vi "Main.vi"() -> ()   [LabVIEW 2023]
uses:
  SubVIs/Control 1.ctl
  SubVIs/CorrelationSwitchControlType.ctl
  C:/Users/nanometa/Documents/TCSPC_Git_Repo/Source/Thorlabs.MotionControl.Controls.dll
  Thorlabs.MotionControl.Controls.dll
  Drivers/BH TCSPC/Examples/Example_Controls/UserInput.ctl
  Drivers/BH TCSPC/SPC_Wrappers/SPC_Controls/ADCResolution.ctl
  <vilib>/Utility/error.llb/DialogType.ctl
  SubVIs/MeasurementType.ctl
  <vilib>/DAQmx/read.llb/DAQmx Read (Counter DBL 1Chan 1Samp).vi
  <vilib>/DAQmx/write.llb/DAQmx Write (Digital 1D Bool 1Chan 1Samp).vi
  <vilib>/DAQmx/create/channels.llb/DAQmx Create Channel (CI-Count Edges).vi
  <vilib>/DAQmx/miscellaneous.llb/DAQmx Fill In Error Info.vi
  <vilib>/DAQmx/create/channels.llb/DAQmx Create Channel (DO-Digital Output).vi
  <vilib>/Utility/file.llb/Write Delimited Spreadsheet (I64).vi
  C:/Users/nanometa/Documents/TCSPC_Git_Repo/Source/ThorLabs.MotionControl.KCube.DCServoCLI.dll
  ThorLabs.MotionControl.KCube.DCServoCLI.dll
  C:/Users/nanometa/Documents/TCSPC_Git_Repo/Source/Thorlabs.MotionControl.FilterFlipperCLI.dll
  Thorlabs.MotionControl.FilterFlipperCLI.dll
  <instrlib>/Thorlabs_FWxC/Thorlabs_FWxC.lvlib
  <vilib>/Analysis/NI_AALBase.lvlib
panel:
  out "lifetime output":u16[][](array[numeric])=[[0], [0], [0], [0], [0], [0], [0], [0], [0], [0], [0], [0], [0], [0], [0], [0], [0], [0], [0], [0], [0], [0], [0], [0], [0], [0], [0], [0], [0], [0], [0], [0], [0], [0], [0], [0], [0], [0], [0], [0], [0], [0], [0], [0], [0], [0], [0], [0], [0], [0], [0], [0], [0], [0], [0], [0], [0], [0], [0], [0], [0], [0], [0], [0], [0], [0], [0], [0], [0], [0], [0], [0], [0], [0], [0], [0], [0], [0], [0], [0], [0], [0], [0], [0], [0], [0], [0], [0], [0], [0], [0], [0], [0], [0], [0], [0], [0], [0], [0], [0], [0], [0], [0], [0], [0], [0], [0], [0], [0], [0], [0], [0], [0], [0], [0], [0], [0], [0], [0], [0], [0], [0], [0], [0], [0], [0], [0], [0], [6], [5], [5], [6], [7], [4], [3], [7], [7], [9], [3], [3], [6], [7], [4], [4], [3], [5], [3], [4], [7], [7], [6], [4], [8], [4], [3], [4], [3], [3], [3], [6], [3], [2], [8], [5], [6], [3], [4], [2], [2], [5], [7], [5], [8], [4], [6], [1], [2], [3], [3], [4], [6], [7], [5], [1], [4], [4], [4], [6], [3], [8], [7], [1], [5], [4], [4], [1], [6], [5], [1], [4], [1], [5], [6], [6], [3], [7], [2], [6], [1], [2], [5], [3], [5], [5], [3], [3], [3], [4], [9], [5], [5], [8], [6], [6], [7], [4], [4], [5], [6], [1], [6], [4], [8], [5], [5], [2], [4], [7], [6], [3], [3], [6], [1], [5], [6], [5], [2], [6], [3], [1], [4], [5], [6], [6], [5], [6], [7], [6], [5], [4], [6], [4], [5], [9], [3], [5], [4], [6], [4], [4], [3], [6], [10], [6], [3], [5], [7], [6], [3], [3], [7], [1], [5], [2], [0], [4], [6], [6], [3], [5], [3], [4], [4], [5], [1], [5], [4], [2], [3], [4], [6], [9], [7], [2], [4], [8], [1], [6], [2], [6], [4], [2], [4], [3], [5], [2], [3], [4], [3], [4], [3], [4], [3], [6], [4], [7], [1], [2], [3], [11], [8], [5], [6], [4], [3], [4], [6], [7], [6], [16], [19], [29], [35], [23], [43], [50], [62], [82], [82], [87], [123], [147], [191], [268], [319], [471], [763], [954], [1441], [2098], [2594], [3370], [3864], [4458], [4550], [4405], [3863], [3514], [2773], [2350], [1769], [1507], [1267], [1044], [879], [868], [787], [694], [634], [605], [569], [567], [565], [551], [457], [504], [464], [486], [476], [461], [401], [443], [420], [400], [382], [384], [415], [405], [363], [352], [334], [352], [325], [329], [353], [331], [311], [338], [327], [313], [310], [308], [282], [295], [277], [271], [298], [259], [267], [277], [303], [249], [241], [270], [246], [264], [284], [247], [270], [220], [214], [241], [221], [257], [232], [225], [222], [260], [202], [215], [211], [184], [197], [183], [188], [198], [203], [201], [199], [187], [174], [177], [172], [184], [172], [172], [184], [186], [160], [174], [161], [182], [140], [153], [175], [141], [151], [140], [151], [142], [136], [130], [152], [125], [138], [122], [151], [131], [117], [134], [110], [140], [114], [122], [127], [126], [116], [112], [129], [113], [111], [107], [117], [116], [114], [140], [117], [117], [99], [110], [117], [82], [109], [95], [92], [90], [99], [105], [96], [72], [102], [101], [97], [88], [95], [83], [90], [97], [77], [102], [72], [96], [76], [101], [82], [96], [83], [71], [80], [83], [96], [81], [72], [81], [64], [75], [81], [68], [67], [82], [62], [72], [68], [72], [79], [53], [65], [69], [53], [66], [74], [54], [60], [69], [56], [52], [58], [52], [57], [72], [45], [59], [62], [48], [51], [64], [57], [45], [45], [46], [55], [44], [43], [42], [51], [44], [42], [44], [53], [52], [44], [52], [52], [45], [53], [35], [38], [31], [44], [41], [47], [41], [36], [49], [43], [35], [40], [45], [35], [39], [47], [36], [44], [36], [38], [38], [40], [48], [38], [28], [36], [36], [32], [34], [32], [50], [35], [27], [43], [42], [35], [36], [38], [49], [28], [37], [34], [33], [27], [31], [36], [20], [28], [33], [32], [29], [40], [33], [31], [37], [42], [22], [29], [32], [34], [30], [29], [25], [27], [33], [25], [34], [35], [30], [36], [17], [22], [22], [16], [28], [25], [24], [24], [29], [19], [18], [28], [35], [17], [23], [18], [28], [23], [23], [23], [30], [28], [13], [26], [18], [26], [26], [28], [24], [22], [27], [18], [29], [20], [26], [29], [31], [25], [28], [21], [23], [11], [15], [19], [15], [23], [12], [16], [18], [23], [26], [18], [12], [17], [25], [21], [24], [18], [31], [13], [18], [25], [13], [23], [18], [15], [23], [15], [16], [18], [20], [10], [22], [12], [23], [22], [21], [14], [15], [17], [11], [20], [14], [19], [13], [6], [14], [14], [13], [17], [8], [7], [8], [23], [21], [12], [18], [14], [17], [10], [15], [13], [13], [18], [17], [10], [13], [14], [24], [18], [16], [21], [13], [13], [13], [11], [10], [13], [15], [11], [11], [8], [13], [12], [6], [13], [9], [12], [9], [18], [14], [11], [19], [17], [19], [9], [12], [16], [13], [11], [8], [12], [10], [16], [13], [18], [10], [15], [9], [15], [14], [14], [11], [11], [14], [15], [11], [14], [8], [9], [15], [10], [11], [11], [3], [6], [6], [8], [13], [13], [11], [11], [11], [14], [9], [15], [2], [15], [15], [7], [8], [8], [12], [6], [9], [11], [9], [12], [8], [9], [16], [8], [16], [6], [8], [14], [14], [9], [4], [16], [11], [14], [10], [16], [13], [8], [12], [3], [16], [9], [6], [10], [14], [6], [8], [8], [13], [8], [9], [15], [5], [8], [8], [12], [6], [8], [10], [9], [13], [9], [6], [7], [11], [9], [7], [9], [10], [8], [6], [8], [14], [8], [7], [15], [8], [10], [8], [5], [8], [7], [8], [5], [4], [14], [10], [8], [9], [3], [5], [9], [10], [6], [2], [10], [5], [6], [12], [9], [8], [14], [4], [3], [10], [9], [10], [6], [13], [6], [11], [8], [4], [6], [4], [5], [14], [9], [5], [5], [7], [12], [7], [10], [9], [7], [11], [4], [5], [8], [5], [7], [14], [9], [3], [4], [4], [5], [7], [2], [6], [4], [2], [13], [9], [10], [6], [11], [7], [6], [5], [7], [14], [8], [5], [6], [12], [11], [6], [5], [7], [7], [5], [8], [6], [10], [3], [6], [10], [8], [6], [10], [8], [6], [6], [7], [8], [5], [4], [9], [8], [4], [9], [5], [8], [7], [5], [6], [4], [6], [8], [5], [8], [13], [6], [10], [7], [6], [9], [8], [8], [3], [7], [8], [9], [7], [4], [8], [4], [6], [8], [13], [4], [8], [8], [9], [1], [4], [11], [9], [5], [5], [9], [6], [5], [8], [8], [3], [10], [3], [9], [3], [5], [4], [2], [9], [6], [12], [5], [14], [11], [3], [8], [7], [4], [6], [5], [8], [8], [7], [3], [9], [3], [6], [8], [6], [3], [6], [6], [5], [11], [6], [7], [6], [5], [4], [3], [8], [4], [1], [3], [11], [7], [3], [4], [4], [8], [8], [4], [4], [4], [3], [7], [5], [3], [8], [5], [11], [10], [8], [4], [2], [4], [4], [7], [10], [2], [5], [8], [8], [8], [4], [6], [2], [5], [5], [7], [4], [8], [10], [6], [3], [5], [5], [6], [7], [5], [5], [8], [8], [9], [9], [5], [6], [9], [5], [4], [5], [6], [8], [6], [6], [4], [7], [6], [12], [12], [10], [5], [11], [6], [9], [5], [6], [7], [7], [9], [6], [5], [7], [6], [12], [5], [5], [6], [6], [5], [3], [6], [8], [8], [5], [5], [2], [4], [8], [3], [4], [6], [4], [3], [9], [3], [6], [9], [11], [6], [2], [6], [5], [3], [12], [6], [8], [6], [5], [3], [3], [4], [3], [7], [6], [4], [4], [4], [4], [5], [4], [6], [5], [9], [3], [3], [4], [5], [1], [6], [5], [5], [4], [3], [2], [13], [10], [4], [3], [4], [4], [6], [4], [4], [2], [5], [3], [9], [1], [5], [11], [6], [6], [2], [8], [2], [6], [7], [8], [5], [7], [11], [8], [4], [4], [8], [11], [1], [2], [6], [3], [3], [5], [5], [9], [4], [5], [9], [6], [10], [4], [2], [6], [5], [2], [2], [3], [8], [6], [3], [5], [5], [8], [2], [2], [4], [2], [4], [4], [4], [8], [4], [2], [9], [2], [5], [3], [4], [12], [1], [5], [4], [6], [3], [4], [4], [6], [6], [6], [4], [5], [7], [7], [4], [1], [10], [6], [7], [3], [5], [4], [9], [2], [5], [6], [10], [5], [8], [7], [5], [5], [4], [7], [6], [4], [7], [1], [11], [6], [5], [6], [5], [7], [2], [3], [3], [5], [2], [9], [5], [4], [7], [1], [6], [6], [6], [8], [5], [6], [6], [4], [3], [8], [4], [1], [7], [6], [4], [8], [6], [7], [7], [7], [4], [4], [5], [5], [8], [3], [3], [6], [5], [7], [3], [3], [1], [7], [3], [7], [5], [5], [3], [7], [5], [3], [3], [7], [5], [7], [6], [5], [4], [5], [4], [8], [7], [4], [9], [3], [2], [5], [6], [4], [11], [5], [2], [4], [6], [3], [9], [3], [5], [11], [3], [5], [6], [6], [6], [6], [5], [4], [9], [8], [0], [4], [4], [5], [4], [1], [5], [5], [2], [5], [6], [5], [5], [3], [6], [5], [8], [6], [4], [1], [5], [7], [6], [3], [3], [3], [8], [3], [1], [6], [2], [4], [6], [4], [5], [4], [3], [9], [6], [6], [6], [8], [6], [4], [0], [5], [7], [8], [3], [4], [4], [5], [8], [6], [12], [3], [10], [5], [7], [2], [6], [4], [6], [2], [1], [4], [3], [2], [6], [6], [9], [7], [3], [1], [2], [5], [8], [4], [3], [3], [3], [5], [3], [4], [5], [8], [7], [6], [5], [5], [6], [6], [2], [5], [10], [4], [5], [4], [5], [13], [4], [4], [5], [10], [5], [4], [1], [9], [3], [1], [3], [9], [4], [6], [8], [6], [3], [4], [9], [7], [0], [6], [4], [7], [4], [7], [7], [2], [5], [3], [3], [6], [3], [2], [7], [2], [5], [6], [3], [2], [4], [2], [3], [3], [2], [4], [3], [4], [5], [7], [3], [4], [5], [7], [5], [5], [4], [5], [9], [2], [8], [6], [12], [7], [4], [4], [7], [15], [2], [5], [6], [5], [8], [1], [4], [5], [8], [6], [5], [3], [5], [3], [5], [8], [2], [9], [8], [3], [6], [5], [5], [5], [6], [4], [3], [2], [5], [5], [7], [4], [6], [10], [10], [3], [3], [0], [3], [3], [3], [2], [9], [3], [9], [7], [12], [8], [7], [7], [2], [2], [6], [2], [5], [4], [2], [2], [3], [2], [6], [7], [5], [1], [5], [4], [5], [4], [5], [7], [4], [5], [4], [4], [4], [6], [4], [1], [4], [3], [5], [5], [4], [8], [1], [5], [4], [3], [4], [6], [8], [7], [11], [6], [4], [4], [5], [5], [13], [5], [2], [5], [9], [3], [2], [3], [6], [2], [2], [6], [5], [4], [1], [8], [6], [2], [0], [5], [4], [5], [2], [5], [2], [6], [7], [0], [2], [5], [2], [6], [2], [4], [4], [7], [6], [8], [2], [7], [2], [4], [3], [5], [3], [7], [5], [7], [6], [5], [10], [5], [3], [6], [6], [6], [3], [7], [3], [9], [8], [3], [5], [6], [3], [4], [4], [5], [3], [4], [6], [6], [3], [6], [5], [9], [5], [5], [2], [5], [4], [4], [4], [6], [4], [1], [3], [3], [4], [7], [6], [0], [3], [5], [5], [3], [4], [7], [2], [3], [8], [5], [5], [1], [4], [5], [7], [4], [5], [3], [4], [4], [7], [7], [6], [3], [8], [8], [3], [4], [6], [1], [6], [4], [8], [5], [2], [6], [6], [8], [5], [5], [6], [1], [3], [5], [2], [5], [4], [5], [5], [2], [4], [5], [3], [4], [5], [8], [6], [3], [5], [7], [5], [5], [3], [5], [5], [9], [3], [9], [5], [11], [3], [9], [9], [3], [2], [5], [4], [2], [5], [5], [7], [2], [2], [2], [10], [6], [4], [3], [4], [5], [6], [3], [10], [6], [2], [7], [3], [9], [7], [5], [2], [5], [5], [3], [3], [6], [4], [1], [4], [4], [6], [4], [4], [4], [2], [8], [5], [5], [7], [6], [2], [4], [1], [4], [4], [6], [7], [4], [2], [4], [7], [4], [2], [4], [6], [4], [1], [3], [4], [2], [4], [3], [4], [5], [6], [5], [4], [2], [7], [5], [4], [4], [2], [6], [2], [5], [4], [4], [5], [6], [5], [6], [6], [5], [1], [6], [7], [6], [4], [10], [6], [4], [5], [7], [7], [6], [4], [3], [6], [1], [5], [5], [3], [2], [5], [4], [5], [6], [4], [3], [5], [4], [5], [5], [7], [4], [4], [5], [4], [7], [5], [8], [10], [4], [7], [3], [4], [3], [2], [7], [6], [3], [3], [5], [2], [4], [6], [6], [3], [3], [5], [5], [3], [3], [5], [5], [4], [2], [6], [3], [5], [5], [5], [3], [1], [5], [3], [3], [7], [5], [8], [5], [3], [3], [6], [5], [11], [6], [7], [9], [3], [8], [3], [9], [8], [3], [7], [7], [3], [6], [6], [6], [6], [6], [3], [5], [5], [6], [10], [9], [4], [6], [4], [7], [3], [2], [2], [8], [4], [5], [1], [4], [3], [6], [6], [2], [7], [3], [8], [5], [7], [5], [6], [4], [9], [5], [3], [7], [5], [1], [0], [6], [6], [7], [5], [1], [3], [8], [4], [4], [6], [8], [3], [5], [4], [5], [2], [7], [6], [4], [4], [5], [3], [3], [4], [3], [4], [6], [5], [1], [1], [9], [7], [3], [5], [4], [3], [3], [7], [6], [6], [1], [2], [3], [6], [4], [4], [4], [2], [4], [5], [7], [1], [6], [3], [8], [7], [5], [2], [3], [4], [6], [6], [5], [4], [9], [5], [5], [4], [8], [5], [6], [2], [1], [10], [5], [3], [5], [2], [5], [2], [2], [4], [6], [2], [7], [3], [1], [8], [8], [4], [7], [5], [9], [3], [8], [3], [3], [6], [6], [4], [4], [2], [3], [4], [5], [9], [12], [2], [2], [5], [11], [8], [5], [4], [3], [2], [4], [8], [7], [3], [2], [3], [4], [1], [2], [4], [3], [3], [3], [6], [2], [2], [4], [5], [4], [11], [5], [3], [1], [4], [6], [5], [4], [6], [7], [6], [10], [5], [7], [1], [8], [2], [7], [3], [7], [5], [6], [5], [5], [7], [3], [7], [3], [8], [2], [7], [4], [5], [6], [8], [3], [5], [5], [2], [6], [2], [2], [4], [1], [4], [7], [5], [4], [5], [1], [7], [3], [4], [7], [6], [3], [5], [4], [9], [4], [6], [3], [0], [3], [9], [3], [4], [3], [3], [3], [2], [4], [5], [3], [3], [5], [2], [1], [7], [4], [8], [2], [5], [2], [5], [4], [4], [4], [4], [7], [5], [5], [5], [4], [3], [6], [2], [3], [9], [6], [7], [6], [2], [2], [1], [8], [2], [3], [4], [3], [2], [4], [1], [2], [5], [2], [2], [9], [2], [6], [6], [4], [5], [6], [4], [4], [3], [4], [4], [2], [1], [2], [3], [2], [2], [8], [6], [2], [5], [3], [4], [5], [3], [4], [7], [3], [8], [5], [6], [4], [5], [2], [5], [5], [5], [5], [4], [5], [5], [6], [3], [7], [5], [5], [7], [7], [7], [4], [3], [2], [6], [7], [4], [1], [8], [2], [1], [5], [5], [4], [7], [9], [4], [4], [5], [6], [1], [5], [4], [3], [7], [7], [7], [5], [6], [4], [3], [9], [7], [6], [7], [4], [5], [6], [0], [5], [4], [2], [3], [4], [0], [4], [3], [7], [6], [6], [3], [8], [3], [9], [2], [2], [5], [5], [3], [6], [3], [5], [5], [6], [7], [4], [4], [1], [2], [6], [7], [4], [3], [4], [4], [3], [11], [1], [3], [5], [5], [8], [7], [5], [5], [4], [3], [3], [6], [2], [4], [4], [7], [1], [3], [6], [3], [5], [4], [1], [6], [3], [1], [4], [5], [6], [2], [3], [5], [3], [7], [6], [5], [3], [3], [2], [5], [5], [0], [2], [2], [5], [5], [3], [6], [3], [4], [8], [4], [3], [3], [0], [4], [6], [2], [2], [5], [2], [6], [5], [6], [6], [4], [7], [5], [4], [2], [6], [6], [3], [4], [4], [2], [4], [3], [2], [3], [6], [5], [2], [4], [6], [3], [5], [5], [1], [3], [3], [5], [3], [3], [4], [4], [7], [7], [6], [7], [4], [8], [3], [3], [2], [5], [7], [8], [4], [2], [5], [9], [6], [9], [4], [7], [6], [5], [5], [4], [2], [6], [6], [4], [2], [3], [5], [9], [9], [3], [6], [3], [2], [1], [8], [5], [0], [6], [3], [5], [5], [4], [4], [5], [7], [5], [5], [2], [5], [2], [8], [6], [5], [3], [3], [4], [2], [3], [7], [6], [4], [5], [2], [3], [2], [7], [4], [5], [7], [8], [4], [5], [6], [4], [3], [4], [4], [7], [6], [1], [3], [4], [3], [4], [3], [6], [2], [7], [6], [3], [3], [4], [6], [5], [3], [8], [4], [3], [3], [4], [4], [6], [0], [3], [9], [4], [1], [2], [4], [4], [5], [8], [4], [3], [7], [3], [7], [6], [4], [6], [6], [6], [4], [10], [5], [6], [4], [5], [9], [4], [4], [10], [5], [3], [4], [6], [1], [5], [9], [4], [4], [5], [3], [3], [5], [6], [4], [7], [4], [6], [2], [3], [4], [2], [2], [3], [6], [3], [6], [5], [8], [3], [4], [5], [1], [5], [5], [3], [2], [3], [1], [7], [1], [3], [7], [6], [7], [8], [6], [6], [3], [4], [3], [5], [4], [8], [3], [2], [3], [0], [5], [7], [1], [2], [2], [3], [3], [4], [2], [7], [5], [7], [6], [4], [4], [5], [5], [7], [3], [5], [4], [4], [5], [3], [3], [5], [3], [7], [3], [6], [2], [4], [8], [7], [8], [2], [7], [4], [5], [2], [7], [1], [5], [6], [2], [5], [6], [4], [9], [6], [6], [5], [6], [2], [1], [5], [9], [5], [7], [1], [6], [2], [1], [6], [2], [7], [5], [3], [3], [5], [5], [1], [5], [9], [4], [3], [5], [3], [6], [5], [2], [2], [4], [3], [4], [6], [5], [2], [5], [9], [6], [4], [9], [5], [6], [4], [3], [6], [5], [3], [4], [5], [4], [3], [3], [6], [4], [5], [4], [5], [5], [4], [7], [7], [2], [4], [1], [4], [3], [2], [7], [4], [6], [5], [3], [8], [1], [2], [7], [3], [4], [4], [7], [4], [4], [5], [6], [3], [5], [3], [4], [3], [2], [5], [2], [7], [7], [4], [7], [4], [3], [4], [4], [7], [3], [5], [2], [4], [3], [8], [2], [6], [3], [3], [5], [6], [3], [5], [0], [4], [4], [4], [3], [6], [8], [4], [2], [6], [6], [1], [3], [4], [1], [4], [6], [6], [6], [2], [4], [4], [8], [8], [2], [5], [3], [3], [2], [3], [3], [1], [2], [1], [2], [4], [5], [7], [6], [8], [3], [4], [5], [1], [5], [2], [7], [2], [2], [7], [5], [9], [2], [4], [2], [7], [6], [4], [3], [4], [4], [4], [6], [5], [1], [1], [3], [4], [7], [6], [9], [7], [3], [4], [1], [5], [7], [7], [5], [6], [3], [6], [6], [6], [6], [3], [3], [3], [4], [3], [4], [6], [6], [5], [5], [3], [6], [7], [4], [5], [5], [4], [3], [5], [5], [2], [1], [4], [2], [2], [4], [5], [5], [3], [4], [4], [3], [2], [6], [1], [4], [5], [6], [2], [5], [4], [9], [7], [3], [6], [7], [5], [4], [4], [4], [1], [7], [1], [3], [5], [3], [2], [3], [3], [7], [4], [3], [5], [8], [0], [3], [3], [9], [8], [7], [4], [7], [8], [4], [6], [6], [2], [5], [3], [3], [6], [2], [6], [7], [7], [2], [6], [4], [5], [2], [8], [3], [5], [3], [5], [3], [2], [4], [5], [6], [2], [3], [4], [1], [1], [6], [5], [3], [6], [10], [5], [4], [5], [3], [8], [6], [4], [1], [2], [4], [3], [4], [4], [3], [5], [6], [6], [2], [5], [6], [3], [8], [5], [4], [6], [5], [5], [4], [5], [4], [2], [3], [7], [2], [6], [5], [7], [6], [3], [6], [8], [6], [5], [8], [6], [5], [7], [5], [3], [2], [2], [4], [2], [6], [7], [5], [3], [3], [4], [6], [7], [7], [5], [7], [5], [6], [4], [4], [3], [5], [7], [2], [2], [3], [1], [3], [8], [1], [5], [7], [6], [2], [5], [4], [7], [4], [2], [1], [3], [6], [4], [5], [7], [2], [7], [7], [2], [4], [5], [7], [7], [5], [2], [2], [5], [6], [4], [6], [2], [5], [0], [2], [9], [2], [2], [5], [3], [5], [7], [2], [4], [1], [3], [5], [4], [4], [7], [4], [3], [3], [4], [3], [4], [3], [5], [3], [1], [9], [5], [14], [2], [3], [5], [8], [5], [2], [3], [6], [4], [4], [7], [6], [2], [5], [3], [5], [6], [3], [7], [3], [4], [1], [4], [8], [4], [4], [4], [7], [4], [3], [5], [5], [5], [3], [5], [4], [4], [6], [3], [3], [6], [7], [6], [4], [2], [7], [6], [4], [6], [3], [2], [4], [5], [3], [3], [3], [9], [4], [6], [5], [3], [4], [5], [6], [5], [3], [4], [3], [6], [5], [5], [4], [3], [6], [5], [5], [5], [5], [2], [4], [9], [5], [7], [9], [6], [4], [4], [5], [6], [5], [8], [7], [5], [10], [2], [3], [3], [1], [6], [5], [3], [2], [1], [4], [5], [5], [4], [6], [7], [3], [4], [7], [6], [4], [2], [5], [5], [5], [9], [4], [6], [2], [4], [6], [4], [7], [4], [4], [3], [3], [7], [6], [4], [1], [1], [6], [6], [5], [5], [5], [6], [4], [7], [4], [5], [4], [5], [5], [5], [3], [3], [5], [3], [4], [7], [7], [4], [5], [0], [1], [4], [5], [4], [5], [8], [1], [5], [5], [9], [3], [5], [5], [4], [4], [4], [4], [7], [4], [8], [2], [1], [4], [2], [3], [8], [2], [5], [2], [7], [5], [5], [1], [4], [1], [5], [5], [4], [10], [4], [5], [5], [8], [5], [3], [5], [2], [2], [7], [3], [3], [3], [2], [5], [8], [3], [5], [5], [4], [5], [3], [5], [2], [4], [7], [3], [4], [6], [4], [3], [6], [7], [9], [3], [4], [6], [4], [4], [1], [10], [4], [3], [6], [10], [4], [5], [5], [4], [6], [6], [6], [4], [4], [4], [6], [7], [8], [3], [4], [6], [5], [5], [1], [2], [3], [5], [3], [4], [3], [4], [5], [11], [8], [7], [7], [6], [3], [4], [9], [3], [4], [4], [1], [4], [2], [3], [2], [2], [7], [4], [3], [6], [6], [2], [6], [5], [3], [6], [5], [4], [3], [5], [2], [6], [3], [3], [2], [6], [2], [6], [6], [2], [1], [1], [2], [4], [6], [8], [5], [3], [4], [7], [4], [12], [3], [4], [3], [3], [3], [5], [4], [5], [1], [6], [7], [7], [5], [3], [3], [6], [6], [3], [6], [4], [6], [2], [4], [5], [8], [3], [5], [7], [4], [2], [3], [2], [4], [2], [6], [4], [7], [3], [3], [3], [2], [2], [5], [4], [6], [2], [4], [3], [4], [7], [6], [5], [6], [5], [5], [3], [5], [5], [4], [7], [7], [6], [3], [4], [5], [2], [6], [2], [7], [2], [5], [7], [2], [1], [7], [2], [6], [9], [0], [3], [4], [6], [6], [4], [4], [7], [4], [4], [6], [8], [7], [4], [5], [3], [4], [6], [3], [5], [5], [5], [3], [5], [6], [5], [4], [6], [3], [4], [4], [3], [6], [6], [10], [4], [3], [3], [4], [5], [6], [4], [4], [5], [6], [13], [6], [6], [6], [7], [4], [4], [6], [5], [4], [1], [5], [8], [1], [4], [8], [4], [4], [2], [5], [3], [3], [7], [1], [6], [6], [1], [4], [6], [3], [4], [2], [4], [6], [4], [4], [2], [7], [7], [5], [5], [6], [5], [6], [5], [7], [6], [5], [5], [4], [6], [7], [7], [7], [2], [5], [4], [2], [5], [5], [5], [6], [8], [2], [4], [1], [8], [7], [7], [2], [8], [4], [5], [6], [3], [4], [5], [2], [5], [1], [3], [4], [5], [3], [3], [4], [9], [4], [5], [5], [4], [2], [5], [3], [6], [3], [4], [7], [3], [6], [6], [6], [1], [6], [4], [3], [6], [9], [2], [4], [7], [2], [8], [4], [2], [8], [5], [4], [1], [5], [1], [5], [6], [7], [4], [5], [5], [5], [4], [4], [4], [3], [1], [5], [4], [3], [5], [5], [2], [4], [7], [1], [3], [4], [0], [1], [6], [6], [5], [9], [4], [5], [2], [2], [7], [3], [5], [3], [3], [3], [4], [7], [7], [5], [11], [3], [5], [3], [5], [3], [4], [3], [4], [7], [5], [2], [6], [7], [3], [3], [2], [6], [6], [7], [5], [1], [10], [4], [7], [3], [2], [4], [4], [7], [5], [5], [3], [7], [3], [4], [4], [1], [8], [5], [6], [5], [2], [5], [6], [5], [3], [5], [5], [4], [4], [8], [4], [2], [4], [7], [5], [4], [2], [4], [5], [5], [6], [3], [6], [7], [7], [5], [8], [3], [5], [5], [7], [11], [5], [1], [10], [3], [3], [4], [7], [5], [8], [9], [7], [0], [0], [0], [0], [0], [0], [0], [0], [0], [0], [0], [0], [0], [0], [0], [0], [0], [0], [0], [0], [0], [0], [0], [0], [0], [0], [0], [0], [0], [0], [0], [0], [0], [0], [0], [0], [0], [0], [0], [0], [0], [0], [0], [0], [0], [0], [0], [0], [0], [0], [0], [0], [0], [0], [0], [0], [0], [0], [0], [0], [0], [0], [0], [0], [0], [0], [0], [0], [0], [0], [0], [0], [0], [0], [0], [0], [0], [0], [0], [0], [0], [0], [0], [0], [0], [0], [0], [0], [0], [0], [0], [0], [0], [0], [0], [0], [0], [0], [0], [0], [0], [0], [0], [0], [0], [0], [0], [0], [0], [0], [0], [0], [0], [0], [0], [0], [0], [0], [0], [0], [0], [0], [0], [0], [0], [0], [0], [0]] caption="Output Array"
  out "Filter Wheel Init Error":errorcluster
  in  "SLOC Laser":bool
  in  "Rotating Laser Power Filter":refnum<k24>(container)
  in  "FilterFlipperControl 2":refnum<k24>(container)
  in  "FilterFlipperControl":refnum<k24>(container)
  out "Xstored":dbl=51.85
  out "Ystored":dbl=45.85
  out "drift vect.":dbl[](array[numeric])
  out "Zstored":dbl=48.40147356000009 format="%.3g"
  out "Saturation Init":dbl[][](array[numeric])
  out "Scriptable Controls (label text)":string="# of bins\n# of Steps\n3D Line Graph\nA-frequency\nA-velocity\nAbs. Move\nActual Coincidences\nAlign Scan\nAlign XY Mesh\nAlign XY range\nAlignment Graph\nAlignment limits\nAnalog Input\nArea #\nAS Duration (msec)\nAUTO XY SCAN\nBoxcar Width\nBS \nBuffered MapCorr\nBuffered Map\nBuffering\ncent\nChoose QC Config\nClear emitters\nCoincidences\nControls\nCorrect map\nCorrection type\nCorrelation measurement\nCount Direction 2\nCount Direction\nCounters 2\nCounters\nCurent DLL mode\nCurrent MapCorr\nCurrent Map\nCurrent mode value\nCW g2 Cutoff\nCW g2\nDisplay time (s)\nDLL_path\ndown\nDraw emitters\ndrift vect.\neast\nEDC Enable\nEdge\nEdge 2\nEmitter #\nEMITTER REPORT\nEMITTER RUNTHROUGH\nEmpty memory\nenable\nError MG17 Spectrometer\nError MG17\nerror out\nExtension\nFine Align\nFirgelli Position (mm)\nFirgelliSetupOutput\ng2 Button\ng2 config 2\ng2 config pulsed\nGetNewLoc\nGS Frequency\nHelp me find emitters!\nIdentification\nIni file name\nInitial Count\nInitSLOCLaserCluster\nInt. Time (microsec)\nIntegration time (ms)\nIntensities\nIntensity Graph\nIntensity\nIntensity limits\nlampOn\nlampOn 2\nLaser power\nlifetime Button\nlifetime config long\nlifetime config short\nLogging mode\nLower thr\nlowerbright\nMap centers\nMap Switch\nMax Radius\nMax velocity\nMax. dir. changes\nMeasure On PDMs\nMesh\nMG17MotorSpectrometer\nMG17Motor\nMin Radius\nMirror Movement\nMirror Movement 2\nML\nMotion\nN Integrations\nNano AS Data\nNanoCube tracking\nNemitters\nNext emitter\nNLC Enable\nnorth\nNumber of used modules\nOutput Array lifetime 2\nOutput Array lifetime\nOutput Array pulsed 2\nOutput Array pulsed to file\nOutput Array pulsed\nOutput Array\nPath to conf file\nPDM 1 on/off\nPDM 2 on/off\nPDM1 counts\nPDM1 trace\nPDM1+PDM2\nPDM2 counts\nPDM2 trace\nPick candidates\nPosition\npulsed g2 Cutoff\nPulsed on/off\nQC error out\nRabi Contrast\nReceived String\nRecord stab\nRerun g2/lifetim/Sat.\nRMS Cutoff\nRun Lifetime\nRun Pulsed g2\nRun Saturation\nRun T1\nS/N\nSatOutput Array\nSaturation Array 2\nSaturation Array\nScan Frequency\nScan Termination\nScan Type\nScan Velocity\nScans to Average\nScriptable Controls (label text)\nSerial Number:\nSLOC Laser\nsouth\nSPC error\nSPC module info\nSPC_rates\nSPCdata\nSPCM counts\nSPCM trace\nSpectrometer Name:\nSpectrum Array\nSpectrum Button\nSpectrum\nSpeed factor\nStabilityRMS\nstart path\nstaturation Button\nstop\nString To Send\nT1 Array\nT1 Button\nT1 Firgell Position\nT1 Measure Cluster\nTable rate\nTAC range\nTCSPCcluster\nTraceData\nTraceDataStab\nTracking\nTrigger Period (s) 2\nUpper thr\nupperbright\nup\nVISA resource name\nVISA resource name out \nWaveform Graph 2\nWaveform Graph\nwest\nWrite Alignment map to file\nWrite g2 to file\nWrite lifetime to file\nWrite PL map to file\nWrite sat. to file\nWrite spectrum to file\nWrite T1 to file\nWrite to file\nWvlgth\nX Scan Center\nX Scan Range\nX-frequency\nXstored\nXY Graph\nX\nXY Scan\nY Scan Center\nY Scan Range\nY-velocity\nYstored\nY\nZ Mesh\nZ range\nZ-frequency\nZ-velocity\nZstored\nZX range\nZ\n\r\n"
  in  "N Integrations":i32=1 min=1 max=65000000
  in  "enable":i16 min=0 max=1 step=1
  in  "lampOn 2":i32 min=0 max=1 step=1
  in  "lampOn":i32 min=0 max=1 step=1
  in  "NLC Enable":i32 min=0 max=1 step=1
  in  "EDC Enable":i32 min=0 max=1 step=1
  out "Spectrometer Name:":string="QE65000"
  out "Serial Number:":string="QEB1140"
  in  "Scans to Average":i32=1 min=1 max=50 step=1
  in  "Boxcar Width":i32=1 min=0 max=50 step=1
  out "NanoCube tracking":cluster{dbl[], dbl[]}(graph)={[49.99295798, 50.00121664, 50.00152345, 49.99750134, 49.99873124, 50.008933, 49.9950786, 49.99353926, 49.9973082, 50.00564734, 50.00756751], [49.99961646, 49.99920959, 50.00021441, 49.99994716, 49.99854077, 50.00032286, 49.99990099, 49.99988771, 50.00065782, 49.99944116, 49.99927217]} caption="Input XY bulls-eye"
  out "Alignment Graph":dbl[][](graph)
  in  "Alignment limits":dbl[](array[numeric])=[0.0, 0.1]
  out "spectrum output":dbl[][](array[numeric])=[[298.5515419, 2193.0], [299.3478420176174, 2191.6666666666665], [300.14408067453877, 2182.6666666666665], [300.94025784086847, 2177.0], [301.7363734867104, 2171.3333333333335], [302.5324275821688, 2170.6666666666665], [303.32842009734765, 2173.6666666666665], [304.1243510023511, 2174.0], [304.92022026728324, 2177.3333333333335], [305.7160278622481, 2180.3333333333335], [306.51177375735, 2181.3333333333335], [307.3074579226929, 2190.0], [308.10308032838077, 2190.6666666666665], [308.8986409445179, 2196.3333333333335], [309.6941397412084, 2191.6666666666665], [310.48957668855627, 2194.6666666666665], [311.2849517566656, 2203.3333333333335], [312.08026491564056, 2191.6666666666665], [312.87551613558526, 2185.0], [313.67070538660363, 2178.3333333333335], [314.46583263880007, 2190.0], [315.2608978622784, 2195.3333333333335], [316.0559010271428, 2189.6666666666665], [316.8508421034975, 2183.3333333333335], [317.6457210614464, 2179.0], [318.4405378710938, 2180.0], [319.2352925025436, 2188.6666666666665], [320.02998492590007, 2194.0], [320.82461511126724, 2192.6666666666665], [321.61918302874915, 2191.0], [322.41368864845003, 2186.6666666666665], [323.2081319404739, 2189.0], [324.00251287492483, 2189.0], [324.796831421907, 2193.0], [325.5910875515244, 2194.6666666666665], [326.38528123388124, 2197.0], [327.1794124390816, 2199.3333333333335], [327.97348113722956, 2195.0], [328.7674872984293, 2192.6666666666665], [329.56143089278464, 2191.0], [330.3553118904, 2192.3333333333335], [331.1491302613794, 2194.3333333333335], [331.9428859758268, 2192.0], [332.73657900384643, 2213.0], [333.53020931554244, 2214.3333333333335], [334.32377688101883, 2201.6666666666665], [335.1172816703796, 2183.3333333333335], [335.91072365372906, 2194.3333333333335], [336.7041028011712, 2208.0], [337.49741908281015, 2199.6666666666665], [338.29067246875, 2190.3333333333335], [339.0838629290949, 2182.0], [339.87699043394883, 2188.0], [340.67005495341596, 2182.3333333333335], [341.46305645760043, 2188.3333333333335], [342.2559949166062, 2186.3333333333335], [343.0488703005376, 2189.6666666666665], [343.8416825794986, 2193.3333333333335], [344.63443172359325, 2205.6666666666665], [345.42711770292567, 2198.0], [346.2197404876, 2200.0], [347.0123000477204, 2181.3333333333335], [347.80479635339077, 2179.3333333333335], [348.5972293747154, 2179.3333333333335], [349.3895990817984, 2181.0], [350.1819054447438, 2191.0], [350.9741484336556, 2178.3333333333335], [351.7663280186381, 2178.6666666666665], [352.5584441697952, 2171.3333333333335], [353.3504968572311, 2175.6666666666665], [354.14248605105007, 2179.6666666666665], [354.93441172135584, 2179.6666666666665], [355.72627383825284, 2184.3333333333335], [356.51807237184494, 2182.6666666666665], [357.3098072922364, 2181.3333333333335], [358.10147856953125, 2190.6666666666665], [358.8930861738336, 2195.3333333333335], [359.6846300752476, 2199.3333333333335], [360.47611024387726, 2194.3333333333335], [361.26752664982666, 2195.3333333333335], [362.0588792632, 2193.6666666666665], [362.8501680541014, 2185.0], [363.64139299263485, 2177.6666666666665], [364.4325540489045, 2176.6666666666665], [365.22365119301446, 2171.6666666666665], [366.0146843950688, 2180.6666666666665], [366.8056536251716, 2184.6666666666665], [367.59655885342704, 2191.3333333333335], [368.3874000499392, 2185.6666666666665], [369.17817718481217, 2192.0], [369.96889022815003, 2195.0], [370.7595391500569, 2203.6666666666665], [371.55012392063685, 2198.6666666666665], [372.3406445099939, 2197.6666666666665], [373.1311008882325, 2191.0], [373.92149302545624, 2184.3333333333335], [374.7118208917696, 2180.6666666666665], [375.5020844572766, 2182.0], [376.29228369208124, 2187.3333333333335], [377.0824185662877, 2185.6666666666665], [377.87248905, 2183.0], [378.66249511332234, 2183.6666666666665], [379.4524367263588, 2184.6666666666665], [380.2423138592135, 2187.3333333333335], [381.0321264819905, 2185.6666666666665], [381.8218745647938, 2192.0], [382.61155807772764, 2192.6666666666665], [383.4011769908961, 2198.3333333333335], [384.1907312744032, 2185.3333333333335], [384.98022089835314, 2186.6666666666665], [385.76964583285, 2183.0], [386.5590060479979, 2196.6666666666665], [387.3483015139008, 2191.6666666666665], [388.137532200663, 2197.0], [388.9266980783884, 2202.0], [389.71579911718123, 2208.0], [390.5048352871456, 2196.0], [391.2938065583856, 2189.0], [392.08271290100527, 2191.0], [392.8715542851087, 2198.3333333333335], [393.66033068080003, 2195.0], [394.44904205818335, 2192.6666666666665], [395.2376883873628, 2196.6666666666665], [396.0262696384425, 2196.3333333333335], [396.81478578152644, 2188.0], [397.6032367867188, 2176.3333333333335], [398.3916226241236, 2185.3333333333335], [399.1799432638451, 2189.3333333333335], [399.9681986759872, 2196.6666666666665], [400.75638883065415, 2184.3333333333335], [401.54451369795004, 2184.6666666666665], [402.33257324797887, 2180.0], [403.1205674508448, 2179.6666666666665], [403.90849627665193, 2181.3333333333335], [404.69635969550444, 2182.3333333333335], [405.4841576775063, 2190.0], [406.27189019276165, 2189.0], [407.05955721137457, 2192.6666666666665], [407.8471587034492, 2190.0], [408.6346946390897, 2196.0], [409.4221649884, 2204.0], [410.20956972148434, 2213.3333333333335], [410.9969088084468, 2206.3333333333335], [411.7841822193915, 2203.3333333333335], [412.5713899244225, 2191.6666666666665], [413.35853189364383, 2193.0], [414.1456080971596, 2185.3333333333335], [414.93261850507406, 2187.6666666666665], [415.7195630874912, 2188.3333333333335], [416.5064418145152, 2193.3333333333335], [417.29325465625004, 2192.0], [418.08000158279987, 2188.3333333333335], [418.8666825642688, 2185.6666666666665], [419.65329757076097, 2198.0], [420.4398465723804, 2201.6666666666665], [421.2263295392313, 2207.0], [422.0127464414176, 2192.3333333333335], [422.7990972490436, 2186.3333333333335], [423.58538193221324, 2177.3333333333335], [424.37160046103065, 2183.0], [425.1577528056, 2191.6666666666665], [425.9438389360253, 2193.3333333333335], [426.7298588224108, 2201.6666666666665], [427.5158124348605, 2203.3333333333335], [428.3016997434784, 2203.0], [429.0875207183688, 2197.3333333333335], [429.8732753296356, 2187.6666666666665], [430.6589635473831, 2187.6666666666665], [431.4445853417152, 2182.0], [432.23014068273613, 2191.3333333333335], [433.01562954055004, 2195.6666666666665], [433.8010518852609, 2195.3333333333335], [434.58640768697285, 2195.3333333333335], [435.37169691579, 2201.3333333333335], [436.15691954181636, 2207.6666666666665], [436.9420755351562, 2200.6666666666665], [437.7271648659136, 2185.6666666666665], [438.5121875041926, 2183.6666666666665], [439.29714342009726, 2185.0], [440.0820325837317, 2193.0], [440.86685496520005, 2190.3333333333335], [441.65161053460633, 2192.3333333333335], [442.43629926205483, 2187.6666666666665], [443.2209211176495, 2186.3333333333335], [444.00547607149446, 2181.3333333333335], [444.7899640936938, 2179.3333333333335], [445.5743851543516, 2178.0], [446.35873922357206, 2190.3333333333335], [447.1430262714592, 2195.6666666666665], [447.92724626811713, 2196.3333333333335], [448.7113991836501, 2190.6666666666665], [449.4954849881619, 2195.6666666666665], [450.27950365175684, 2196.6666666666665], [451.063455144539, 2194.0], [451.84733943661234, 2198.6666666666665], [452.6311564980812, 2204.3333333333335], [453.4149062990496, 2204.0], [454.1985888096216, 2190.6666666666665], [454.9822039999013, 2179.3333333333335], [455.7657518399927, 2176.6666666666665], [456.5492323, 2193.0], [457.33264535002735, 2195.3333333333335], [458.1159909601788, 2204.6666666666665], [458.89926910055846, 2194.6666666666665], [459.6824797412704, 2195.6666666666665], [460.46562285241885, 2186.6666666666665], [461.24869840410764, 2186.0], [462.03170636644103, 2193.6666666666665], [462.8146467095232, 2200.0], [463.59751940345814, 2199.3333333333335], [464.38032441835, 2198.3333333333335], [465.1630617243029, 2191.3333333333335], [465.94573129142077, 2201.6666666666665], [466.72833308980796, 2201.3333333333335], [467.5108670895684, 2202.6666666666665], [468.2933332608062, 2197.3333333333335], [469.07573157362566, 2225.6666666666665], [469.8580619981306, 2230.0], [470.6403245044252, 2221.0], [471.4225190626136, 2193.0], [472.2046456428, 2194.0], [472.9867042150883, 2205.0], [473.76869474958283, 2200.6666666666665], [474.5506172163875, 2200.3333333333335], [475.33247158560647, 2192.6666666666665], [476.1142578273438, 2203.3333333333335], [476.8959759117036, 2206.3333333333335], [477.6776258087901, 2211.3333333333335], [478.45920748870725, 2202.6666666666665], [479.24072092155916, 2196.0], [480.02216607745004, 2186.6666666666665], [480.80354292648394, 2193.6666666666665], [481.5848514387648, 2194.6666666666665], [482.366091584397, 2198.6666666666665], [483.14726333348443, 2185.0], [483.9283666561313, 2183.3333333333335], [484.7094015224416, 2179.3333333333335], [485.4903679025196, 2188.0], [486.27126576646924, 2196.6666666666665], [487.0520950843947, 2203.0], [487.8328558264, 2205.6666666666665], [488.61354796258934, 2204.3333333333335], [489.3941714630668, 2205.6666666666665], [490.1747262979365, 2201.6666666666665], [490.95521243730246, 2191.3333333333335], [491.7356298512688, 2234.0], [492.51597850993966, 2278.6666666666665], [493.29625838341906, 2286.6666666666665], [494.07646944181124, 2237.0], [494.85661165522015, 2193.6666666666665], [495.63668499375, 2191.6666666666665], [496.4166894275049, 2197.6666666666665], [497.1966249265888, 2198.6666666666665], [497.976491461106, 2203.6666666666665], [498.7562890011604, 2209.0], [499.5360175168563, 2204.0], [500.31567697829763, 2203.6666666666665], [501.09526735558865, 2202.0], [501.8747886188333, 2202.6666666666665], [502.6542407381357, 2205.0], [503.43362368360005, 2194.3333333333335], [504.2129374253304, 2192.0], [504.9921819334308, 2180.6666666666665], [505.7713571780055, 2192.3333333333335], [506.55046312915846, 2195.0], [507.3294997569938, 2204.0], [508.1084670316156, 2195.6666666666665], [508.887364923128, 2197.0], [509.6661934016352, 2201.3333333333335], [510.44495243724117, 2199.0], [511.22364200005006, 2198.0], [512.0022620601659, 2193.6666666666665], [512.7808125876928, 2191.3333333333335], [513.5592935527351, 2196.3333333333335], [514.3377049253965, 2187.6666666666665], [515.1160466757813, 2197.3333333333335], [515.8943187739936, 2197.3333333333335], [516.6725211901376, 2285.3333333333335], [517.4506538943173, 2281.3333333333335], [518.2287168566367, 2278.6666666666665], [519.0067100472002, 2204.0], [519.7846334361113, 2205.0], [520.5624869934747, 2201.3333333333335], [521.3402706893945, 2200.3333333333335], [522.1179844939745, 2199.0], [522.8956283773188, 2202.6666666666665], [523.6732023095316, 2205.3333333333335], [524.450706260717, 2210.0], [525.2281402009792, 2209.6666666666665], [526.0055041004222, 2212.0], [526.7827979291501, 2211.3333333333335], [527.5600216572669, 2211.0], [528.3371752548769, 2197.6666666666665], [529.1142586920839, 2201.6666666666665], [529.8912719389924, 2198.6666666666665], [530.6682149657063, 2200.6666666666665], [531.4450877423296, 2199.0], [532.2218902389666, 2201.0], [532.9986224257212, 2196.6666666666665], [533.7752842726977, 2193.6666666666665], [534.55187575, 2192.0], [535.3283968277323, 2193.0], [536.1048474759988, 2196.0], [536.8812276649035, 2201.0], [537.6575373645504, 2201.0], [538.4337765450438, 2198.0], [539.2099451764877, 2206.0], [539.986043228986, 2212.0], [540.7620706726432, 2211.3333333333335], [541.5380274775631, 2201.0], [542.31391361385, 2197.3333333333335], [543.089729051608, 2195.6666666666665], [543.8654737609407, 2198.3333333333335], [544.6411477119531, 2198.0], [545.4167508747485, 2197.3333333333335], [546.1922832194313, 2197.3333333333335], [546.9677447161057, 2200.0], [547.7431353348757, 2199.6666666666665], [548.5184550458453, 2203.6666666666665], [549.2937038191186, 2198.6666666666665], [550.0688816248002, 2207.0], [550.8439884329933, 2199.6666666666665], [551.6190242138028, 2196.3333333333335], [552.3939889373326, 2194.3333333333335], [553.1688825736865, 2201.0], [553.9437050929689, 2209.0], [554.7184564652836, 2202.6666666666665], [555.4931366607352, 2193.3333333333335], [556.2677456494272, 2192.6666666666665], [557.0422834014643, 2193.6666666666665], [557.8167498869501, 2200.0], [558.5911450759888, 2203.0], [559.3654689386848, 2204.6666666666665], [560.139721445142, 2200.0], [560.9139025654645, 2193.3333333333335], [561.6880122697563, 2192.0], [562.4620505281216, 2192.6666666666665], [563.2360173106646, 2200.6666666666665], [564.0099125874892, 2198.0], [564.7837363286998, 2203.6666666666665], [565.5574885044, 2207.0], [566.3311690846944, 2211.0], [567.1047780396868, 2208.6666666666665], [567.8783153394814, 2202.3333333333335], [568.6517809541824, 2211.6666666666665], [569.4251748538937, 2208.3333333333335], [570.1984970087196, 2205.6666666666665], [570.971747388764, 2199.3333333333335], [571.7449259641312, 2202.3333333333335], [572.5180327049252, 2212.3333333333335], [573.2910675812501, 2218.0], [574.0640305632099, 2216.6666666666665], [574.8369216209087, 2204.3333333333335], [575.6097407244511, 2190.0], [576.3824878439405, 2195.0], [577.1551629494812, 2195.6666666666665], [577.9277660111777, 2199.6666666666665], [578.7002969991337, 2195.0], [579.4727558834533, 2202.0], [580.2451426342407, 2198.3333333333335], [581.0174572216001, 2197.3333333333335], [581.7896996156353, 2193.6666666666665], [582.5618697864509, 2206.0], [583.3339677041505, 2209.0], [584.1059933388384, 2207.3333333333335], [584.8779466606188, 2194.3333333333335], [585.6498276395955, 2190.6666666666665], [586.4216362458732, 2193.0], [587.1933724495552, 2202.6666666666665], [587.9650362207462, 2205.6666666666665], [588.7366275295501, 2203.3333333333335], [589.5081463460708, 2198.6666666666665], [590.279592640413, 2198.0], [591.0509663826799, 2193.3333333333335], [591.8222675429765, 2192.6666666666665], [592.5934960914062, 2183.3333333333335], [593.3646519980737, 2185.0], [594.1357352330825, 2180.0], [594.9067457665371, 2187.6666666666665], [595.6776835685417, 2182.0], [596.4485486092, 2184.0], [597.2193408586164, 2185.6666666666665], [597.9900602868948, 2192.0], [598.7607068641395, 2191.6666666666665], [599.5312805604545, 2197.0], [600.3017813459437, 2200.3333333333335], [601.0722091907118, 2205.3333333333335], [601.8425640648621, 2197.6666666666665], [602.6128459384993, 2198.6666666666665], [603.3830547817272, 2196.6666666666665], [604.1531905646501, 2200.3333333333335], [604.9232532573719, 2196.3333333333335], [605.6932428299967, 2197.3333333333335], [606.4631592526291, 2197.3333333333335], [607.2330024953724, 2205.6666666666665], [608.0027725283313, 2210.3333333333335], [608.7724693216097, 2197.6666666666665], [609.5420928453116, 2185.6666666666665], [610.3116430695412, 2177.3333333333335], [611.0811199644025, 2188.3333333333335], [611.8505235000001, 2185.0], [612.6198536464374, 2193.3333333333335], [613.3891103738188, 2195.3333333333335], [614.1582936522485, 2207.3333333333335], [614.9274034518304, 2205.0], [615.6964397426689, 2199.6666666666665], [616.4654024948676, 2188.3333333333335], [617.2342916785311, 2187.0], [618.0031072637632, 2184.3333333333335], [618.7718492206682, 2184.0], [619.5405175193501, 2184.6666666666665], [620.3091121299128, 2187.6666666666665], [621.077633022461, 2196.0], [621.846080167098, 2187.6666666666665], [622.6144535339284, 2184.3333333333335], [623.3827530930562, 2181.6666666666665], [624.1509788145856, 2188.0], [624.9191306686206, 2190.0], [625.6872086252652, 2187.3333333333335], [626.4552126546238, 2189.3333333333335], [627.2231427268, 2191.3333333333335], [627.9909988118984, 2199.3333333333335], [628.7587808800229, 2199.6666666666665], [629.5264889012775, 2198.0], [630.2941228457665, 2187.3333333333335], [631.0616826835937, 2183.0], [631.8291683848637, 2180.6666666666665], [632.59657991968, 2185.3333333333335], [633.3639172581472, 2185.0], [634.1311803703693, 2188.6666666666665], [634.8983692264501, 2189.0], [635.665483796494, 2187.6666666666665], [636.4325240506048, 2188.0], [637.199489958887, 2206.0], [637.9663814914444, 2201.6666666666665], [638.7331986183813, 2196.6666666666665], [639.4999413098017, 2173.6666666666665], [640.2666095358096, 2181.0], [641.0332032665093, 2178.0], [641.7997224720046, 2185.0], [642.5661671224001, 2187.0], [643.3325371877994, 2191.6666666666665], [644.0988326383069, 2196.0], [644.8650534440266, 2204.3333333333335], [645.6311995750624, 2209.0], [646.3972710015189, 2204.6666666666665], [647.1632676934995, 2190.0], [647.9291896211092, 2186.3333333333335], [648.6950367544512, 2177.0], [649.4608090636302, 2178.3333333333335], [650.22650651875, 2181.6666666666665], [650.9921290899148, 2184.6666666666665], [651.7576767472289, 2181.3333333333335], [652.5231494607959, 2183.6666666666665], [653.2885472007204, 2191.3333333333335], [654.0538699371062, 2199.3333333333335], [654.8191176400576, 2197.6666666666665], [655.5842902796786, 2188.0], [656.3493878260731, 2179.6666666666665], [657.1144102493457, 2170.6666666666665], [657.8793575195999, 2173.6666666666665], [658.6442296069403, 2182.0], [659.4090264814707, 2183.6666666666665], [660.1737481132955, 2185.0], [660.9383944725186, 2191.6666666666665], [661.7029655292437, 2202.0], [662.4674612535757, 2200.0], [663.231881615618, 2192.6666666666665], [663.9962265854753, 2191.3333333333335], [664.7604961332512, 2243.3333333333335], [665.5246902290501, 2235.3333333333335], [666.288808842976, 2228.6666666666665], [667.0528519451328, 2181.0], [667.8168195056251, 2184.3333333333335], [668.5807114945563, 2186.3333333333335], [669.3445278820312, 2184.3333333333335], [670.1082686381536, 2179.0], [670.8719337330276, 2181.6666666666665], [671.6355231367572, 2185.0], [672.3990368194467, 2194.0], [673.1624747512001, 2188.6666666666665], [673.9258369021214, 2186.3333333333335], [674.6891232423148, 2190.0], [675.4523337418844, 2200.0], [676.2154683709343, 2208.6666666666665], [676.9785270995689, 2203.6666666666665], [677.7415098978915, 2196.6666666666665], [678.5044167360072, 2188.0], [679.2672475840193, 2186.6666666666665], [680.0300024120321, 2188.0], [680.7926811901501, 2202.6666666666665], [681.5552838884768, 2209.3333333333335], [682.3178104771168, 2203.6666666666665], [683.0802609261739, 2193.6666666666665], [683.8426352057525, 2185.0], [684.6049332859562, 2189.3333333333335], [685.3671551368897, 2181.6666666666665], [686.1293007286566, 2191.0], [686.8913700313611, 2194.6666666666665], [687.6533630151077, 2197.6666666666665], [688.41527965, 2185.0], [689.1771199061424, 2183.0], [689.9388837536388, 2189.3333333333335], [690.7005711625935, 2197.6666666666665], [691.4621821031104, 2191.6666666666665], [692.2237165452938, 2194.6666666666665], [692.9851744592477, 2188.0], [693.7465558150761, 2190.3333333333335], [694.5078605828832, 2181.0], [695.2690887327732, 2182.6666666666665], [696.03024023485, 2180.0], [696.7913150592179, 2180.3333333333335], [697.5523131759808, 2190.6666666666665], [698.3132345552431, 2196.0], [699.0740791671084, 2196.0], [699.8348469816813, 2194.6666666666665], [700.5955379690657, 2193.6666666666665], [701.3561520993655, 2195.6666666666665], [702.1166893426853, 2189.3333333333335], [702.8771496691286, 2191.3333333333335], [703.6375330488002, 2192.6666666666665], [704.3978394518033, 2192.6666666666665], [705.1580688482429, 2194.0], [705.9182212082226, 2188.6666666666665], [706.6782965018463, 2190.0], [707.4382946992189, 2180.3333333333335], [708.1982157704435, 2183.0], [708.958059685625, 2187.6666666666665], [709.7178264148672, 2204.6666666666665], [710.4775159282742, 2201.3333333333335], [711.23712819595, 2199.6666666666665], [711.9966631879988, 2191.6666666666665], [712.756120874525, 2198.6666666666665], [713.515501225632, 2193.0], [714.2748042114245, 2194.0], [715.0340298020063, 2194.6666666666665], [715.7931779674816, 2199.6666666666665], [716.5522486779546, 2208.3333333333335], [717.3112419035292, 2205.6666666666665], [718.0701576143098, 2210.3333333333335], [718.8289957804, 2199.0], [719.5877563719043, 2197.3333333333335], [720.3464393589269, 2187.3333333333335], [721.1050447115715, 2188.3333333333335], [721.8635723999424, 2184.3333333333335], [722.6220223941436, 2191.3333333333335], [723.3803946642797, 2188.3333333333335], [724.1386891804541, 2193.0], [724.8969059127712, 2189.0], [725.6550448313352, 2196.6666666666665], [726.41310590625, 2202.6666666666665], [727.17108910762, 2199.3333333333335], [727.9289944055488, 2200.6666666666665], [728.686821770141, 2192.0], [729.4445711715005, 2198.6666666666665], [730.2022425797313, 2198.3333333333335], [730.9598359649376, 2197.3333333333335], [731.7173512972234, 2186.0], [732.4747885466933, 2179.0], [733.2321476834506, 2182.6666666666665], [733.9894286776001, 2192.0], [734.7466314992454, 2201.6666666666665], [735.5037561184909, 2194.0], [736.2608025054404, 2194.0], [737.0177706301984, 2189.3333333333335], [737.7746604628688, 2202.6666666666665], [738.5314719735555, 2201.0], [739.288205132363, 2199.0], [740.0448599093952, 2198.6666666666665], [740.8014362747563, 2204.6666666666665], [741.55793419855, 2201.6666666666665], [742.3143536508808, 2196.6666666666665], [743.0706946018529, 2191.3333333333335], [743.8269570215699, 2186.3333333333335], [744.5831408801364, 2189.0], [745.3392461476562, 2185.0], [746.0952727942337, 2182.3333333333335], [746.8512207899727, 2184.6666666666665], [747.6070901049771, 2190.6666666666665], [748.3628807093518, 2188.6666666666665], [749.1185925732, 2184.0], [749.8742256666263, 2181.0], [750.6297799597348, 2188.3333333333335], [751.3852554226295, 2189.6666666666665], [752.1406520254145, 2193.3333333333335], [752.8959697381938, 2196.3333333333335], [753.6512085310717, 2192.6666666666665], [754.4063683741521, 2193.0], [755.1614492375393, 2196.6666666666665], [755.9164510913372, 2201.3333333333335], [756.6713739056502, 2199.6666666666665], [757.426217650582, 2196.6666666666665], [758.1809822962367, 2190.0], [758.9356678127191, 2184.3333333333335], [759.6902741701324, 2176.6666666666665], [760.4448013385813, 2187.0], [761.1992492881697, 2201.6666666666665], [761.9536179890015, 2207.3333333333335], [762.7079074111813, 2194.3333333333335], [763.4621175248127, 2188.0], [764.2162483000001, 2184.0], [764.9702997068473, 2196.3333333333335], [765.7242717154588, 2192.3333333333335], [766.4781642959385, 2193.3333333333335], [767.2319774183903, 2189.6666666666665], [767.9857110529189, 2190.0], [768.7393651696276, 2199.0], [769.4929397386211, 2192.6666666666665], [770.2464347300032, 2198.6666666666665], [770.9998501138782, 2191.3333333333335], [771.7531858603501, 2196.0], [772.5064419395229, 2185.0], [773.2596183215009, 2189.6666666666665], [774.012714976388, 2186.0], [774.7657318742885, 2188.3333333333335], [775.5186689853062, 2184.0], [776.2715262795457, 2186.6666666666665], [777.0243037271106, 2195.3333333333335], [777.7770012981052, 2190.3333333333335], [778.5296189626338, 2193.6666666666665], [779.2821566908, 2189.6666666666665], [780.0346144527084, 2198.6666666666665], [780.7869922184628, 2204.3333333333335], [781.5392899581675, 2203.0], [782.2915076419265, 2207.0], [783.0436452398437, 2191.3333333333335], [783.7957027220237, 2185.6666666666665], [784.5476800585701, 2183.3333333333335], [785.2995772195873, 2187.6666666666665], [786.0513941751792, 2192.0], [786.8031308954501, 2191.6666666666665], [787.554787350504, 2197.3333333333335], [788.3063635104448, 2192.6666666666665], [789.0578593453771, 2184.6666666666665], [789.8092748254044, 2189.0], [790.5606099206314, 2200.6666666666665], [791.3118646011617, 2200.6666666666665], [792.0630388370995, 2187.0], [792.8141325985493, 2176.0], [793.5651458556147, 2183.0], [794.3160785784, 2189.6666666666665], [795.0669307370093, 2192.0], [795.8177023015468, 2185.3333333333335], [796.5683932421165, 2176.3333333333335], [797.3190035288223, 2177.3333333333335], [798.0695331317688, 2186.6666666666665], [798.8199820210596, 2205.3333333333335], [799.5703501667992, 2203.0], [800.3206375390912, 2200.0], [801.0708441080401, 2195.3333333333335], [801.8209698437502, 2192.3333333333335], [802.5710147163248, 2188.6666666666665], [803.3209786958689, 2199.0], [804.0708617524859, 2208.3333333333335], [804.8206638562805, 2200.6666666666665], [805.5703849773563, 2183.6666666666665], [806.3200250858176, 2184.3333333333335], [807.0695841517686, 2198.0], [807.8190621453132, 2204.3333333333335], [808.5684590365557, 2204.6666666666665], [809.3177747956, 2203.0], [810.0670093925504, 2193.0], [810.8161627975109, 2189.0], [811.5652349805855, 2181.0], [812.3142259118785, 2185.3333333333335], [813.0631355614937, 2191.6666666666665], [813.8119638995357, 2191.6666666666665], [814.560710896108, 2196.3333333333335], [815.3093765213154, 2181.3333333333335], [816.0579607452612, 2189.0], [816.8064635380499, 2191.3333333333335], [817.554884869786, 2204.3333333333335], [818.3032247105727, 2196.6666666666665], [819.0514830305151, 2191.0], [819.7996597997164, 2187.6666666666665], [820.5477549882812, 2192.0], [821.2957685663137, 2194.0], [822.0437005039175, 2197.0], [822.7915507711972, 2202.0], [823.5393193382566, 2205.3333333333335], [824.2870061752002, 2197.3333333333335], [825.0346112521314, 2191.6666666666665], [825.7821345391546, 2180.0], [826.5295760063746, 2186.3333333333335], [827.2769356238944, 2190.0], [828.0242133618189, 2211.0], [828.7714091902516, 2203.0], [829.5185230792971, 2205.6666666666665], [830.2655549990593, 2185.0], [831.0125049196421, 2195.0], [831.7593728111501, 2189.6666666666665], [832.5061586436868, 2199.6666666666665], [833.2528623873569, 2201.3333333333335], [833.999484012264, 2202.0], [834.7460234885126, 2197.6666666666665], [835.4924807862062, 2186.6666666666665], [836.2388558754495, 2183.3333333333335], [836.9851487263467, 2181.6666666666665], [837.7313593090012, 2181.6666666666665], [838.4774875935178, 2182.0], [839.22353355, 2180.3333333333335], [839.9694971485525, 2186.0], [840.7153783592788, 2186.6666666666665], [841.4611771522834, 2186.6666666666665], [842.2068934976704, 2191.6666666666665], [842.9525273655438, 2190.3333333333335], [843.6980787260077, 2193.0], [844.443547549166, 2183.3333333333335], [845.1889338051234, 2190.3333333333335], [845.9342374639832, 2247.3333333333335], [846.6794584958499, 2249.3333333333335], [847.424596870828, 2255.0], [848.1696525590207, 2206.6666666666665], [848.914625530533, 2204.6666666666665], [849.6595157554684, 2194.6666666666665], [850.4043232039312, 2186.6666666666665], [851.1490478460256, 2182.3333333333335], [851.8936896518555, 2185.3333333333335], [852.6382485915252, 2180.0], [853.3827246351387, 2205.0], [854.1271177528001, 2203.3333333333335], [854.8714279146134, 2221.3333333333335], [855.6156550906827, 2206.3333333333335], [856.3597992511125, 2205.3333333333335], [857.1038603660063, 2212.6666666666665], [857.8478384054689, 2215.6666666666665], [858.5917333396037, 2220.6666666666665], [859.3355451385152, 2209.0], [860.0792737723073, 2205.6666666666665], [860.8229192110841, 2194.6666666666665], [861.5664814249501, 2182.0], [862.3099603840088, 2177.6666666666665], [863.053356058365, 2180.6666666666665], [863.7966684181221, 2183.3333333333335], [864.5398974333846, 2183.6666666666665], [865.2830430742563, 2264.0], [866.0261053108416, 2294.6666666666665], [866.7690841132446, 2293.0], [867.5119794515691, 2213.3333333333335], [868.2547912959197, 2188.3333333333335], [868.9975196164, 2198.3333333333335], [869.7401643831145, 2198.6666666666665], [870.4827255661668, 2195.6666666666665], [871.2252031356614, 2190.0], [871.9675970617026, 2191.0], [872.7099073143937, 2184.0], [873.4521338638398, 2186.3333333333335], [874.1942766801441, 2181.3333333333335], [874.9363357334113, 2183.3333333333335], [875.6783109937453, 2190.3333333333335], [876.42020243125, 2197.6666666666665], [877.16201001603, 2209.6666666666665], [877.9037337181887, 2199.6666666666665], [878.6453735078311, 2192.3333333333335], [879.3869293550605, 2185.3333333333335], [880.1284012299813, 2192.6666666666665], [880.8697891026977, 2200.3333333333335], [881.6110929433135, 2194.3333333333335], [882.3523127219332, 2193.3333333333335], [883.0934484086607, 2190.6666666666665], [883.8344999736001, 2193.3333333333335], [884.5754673868554, 2190.6666666666665], [885.3163506185307, 2191.0], [886.0571496387305, 2202.0], [886.7978644175583, 2196.6666666666665], [887.5384949251188, 2199.3333333333335], [888.2790411315157, 2191.0], [889.0195030068533, 2195.3333333333335], [889.7598805212352, 2190.6666666666665], [890.5001736447662, 2192.0], [891.24038234755, 2195.6666666666665], [891.9805065996908, 2197.6666666666665], [892.7205463712929, 2203.3333333333335], [893.4605016324599, 2191.6666666666665], [894.2003723532965, 2186.6666666666665], [894.9401585039062, 2184.0], [895.6798600543935, 2191.3333333333335], [896.4194769748627, 2202.3333333333335], [897.1590092354171, 2197.3333333333335], [897.8984568061618, 2191.0], [898.6378196572, 2189.3333333333335], [899.3770977586365, 2188.0], [900.1162910805749, 2186.0], [900.8553995931195, 2179.6666666666665], [901.5944232663745, 2183.0], [902.3333620704437, 2191.0], [903.0722159754317, 2199.6666666666665], [903.8109849514422, 2201.0], [904.5496689685791, 2195.6666666666665], [905.2882679969472, 2197.3333333333335], [906.0267820066499, 2194.6666666666665], [906.765210967792, 2200.3333333333335], [907.5035548504768, 2184.0], [908.2418136248091, 2188.3333333333335], [908.9799872608925, 2188.6666666666665], [909.7180757288312, 2196.0], [910.4560789987297, 2188.3333333333335], [911.1939970406916, 2185.6666666666665], [911.9318298248213, 2179.3333333333335], [912.6695773212227, 2179.6666666666665], [913.4072395000001, 2184.0], [914.1448163312574, 2187.0], [914.8823077850988, 2195.0], [915.6197138316285, 2187.0], [916.3570344409504, 2194.0], [917.0942695831689, 2189.0], [917.8314192283876, 2189.0], [918.5684833467112, 2184.0], [919.3054619082433, 2189.0], [920.042354883088, 2207.3333333333335], [920.7791622413501, 2207.0], [921.5158839531329, 2199.0], [922.2525199885409, 2186.3333333333335], [922.989070317678, 2178.6666666666665], [923.7255349106485, 2170.6666666666665], [924.4619137375563, 2173.6666666666665], [925.1982067685055, 2185.3333333333335], [925.9344139736006, 2198.0], [926.6705353229453, 2191.6666666666665], [927.4065707866438, 2193.6666666666665], [928.1425203348, 2192.0], [928.8783839375185, 2192.0], [929.6141615649029, 2192.3333333333335], [930.3498531870574, 2185.6666666666665], [931.0854587740864, 2191.3333333333335], [931.8209782960937, 2185.6666666666665], [932.5564117231837, 2194.3333333333335], [933.2917590254601, 2192.0], [934.0270201730272, 2192.0], [934.7621951359893, 2185.0], [935.49728388445, 2186.0], [936.2322863885139, 2191.6666666666665], [936.9672026182849, 2204.6666666666665], [937.7020325438671, 2200.6666666666665], [938.4367761353644, 2195.3333333333335], [939.1714333628812, 2187.3333333333335], [939.9060041965217, 2189.6666666666665], [940.6404886063896, 2189.3333333333335], [941.3748865625893, 2188.3333333333335], [942.1091980352247, 2189.0], [942.8434229944, 2189.0], [943.5775614102195, 2188.3333333333335], [944.3116132527867, 2184.6666666666665], [945.0455784922066, 2185.0], [945.7794570985824, 2185.3333333333335], [946.5132490420189, 2189.0], [947.2469542926196, 2188.0], [947.9805728204892, 2189.6666666666665], [948.7141045957313, 2185.6666666666665], [949.4475495884501, 2189.0], [950.1809077687501, 2185.0], [950.9141791067348, 2194.6666666666665], [951.6473635725089, 2191.3333333333335], [952.380461136176, 2192.3333333333335], [953.1134717678406, 2190.0], [953.8463954376062, 2193.6666666666665], [954.5792321155776, 2197.6666666666665], [955.3119817718587, 2197.0], [956.0446443765532, 2185.6666666666665], [956.7772198997658, 2183.6666666666665], [957.5097083116, 2187.6666666666665], [958.2421095821605, 2190.0], [958.9744236815509, 2191.3333333333335], [959.7066505798755, 2183.6666666666665], [960.4387902472386, 2196.0], [961.1708426537438, 2188.6666666666665], [961.9028077694957, 2186.6666666666665], [962.6346855645982, 2182.6666666666665], [963.3664760091551, 2186.6666666666665], [964.0981790732712, 2183.3333333333335], [964.82979472705, 2184.6666666666665], [965.561322940596, 2189.0], [966.2927636840128, 2192.0], [967.0241169274051, 2193.0], [967.7553826408764, 2192.0], [968.4865607945311, 2189.6666666666665], [969.2176513584737, 2186.3333333333335], [969.9486543028075, 2181.6666666666665], [970.6795695976374, 2183.3333333333335], [971.4103972130666, 2187.6666666666665], [972.1411371192002, 2192.6666666666665], [972.8717892861414, 2194.6666666666665], [973.6023536839948, 2191.3333333333335], [974.3328302828646, 2192.0], [975.0632190528544, 2190.0], [975.7935199640689, 2192.6666666666665], [976.5237329866115, 2197.6666666666665], [977.2538580905872, 2205.0], [977.9838952460993, 2199.3333333333335], [978.7138444232521, 2197.0], [979.4437055921501, 2194.3333333333335], [980.1734787228969, 2195.6666666666665], [980.9031637855969, 2192.3333333333335], [981.632760750354, 2191.3333333333335], [982.3622695872725, 2200.3333333333335], [983.0916902664563, 2195.0], [983.8210227580096, 2196.0], [984.5502670320366, 2195.0], [985.2794230586412, 2203.6666666666665], [986.0084908079278, 2210.3333333333335], [986.7374702500001, 2203.0], [987.4663613549623, 2201.0], [988.195164092919, 2188.6666666666665], [988.9238784339734, 2186.6666666666665], [989.6525043482305, 2176.3333333333335], [990.3810418057938, 2178.6666666666665], [991.1094907767678, 2181.3333333333335], [991.8378512312561, 2192.0], [992.5661231393632, 2201.6666666666665], [993.2943064711933, 2196.3333333333335], [994.02240119685, 2191.0], [994.750407286438, 2183.6666666666665], [995.4783247100609, 2192.6666666666665], [996.2061534378231, 2206.3333333333335], [996.9338934398285, 2211.0], [997.6615446861813, 2206.0], [998.3891071469857, 2196.6666666666665], [999.1165807923455, 2193.3333333333335], [999.8439655923653, 2207.6666666666665], [1000.5712615171487, 2204.3333333333335], [1001.2984685368001, 2203.0], [1002.0255866214234, 2188.3333333333335], [1002.7526157411228, 2187.6666666666665], [1003.4795558660026, 2193.3333333333335], [1004.2064069661665, 2191.3333333333335], [1004.9331690117189, 2196.6666666666665], [1005.6598419727636, 2200.3333333333335], [1006.3864258194052, 2203.3333333333335], [1007.1129205217472, 2198.6666666666665], [1007.8393260498941, 2189.6666666666665], [1008.5656423739501, 2194.3333333333335], [1009.2918694640189, 2199.0], [1010.0180072902049, 2198.0], [1010.744055822612, 2201.3333333333335], [1011.4700150313446, 2200.3333333333335], [1012.1958848865063, 2205.0], [1012.9216653582016, 2198.3333333333335], [1013.6473564165346, 2194.0], [1014.3729580316093, 2187.0], [1015.0984701735298, 2189.0], [1015.8238928124, 2196.0], [1016.5492259183244, 2207.3333333333335], [1017.2744694614069, 2211.0], [1017.9996234117515, 2209.3333333333335], [1018.7246877394625, 2202.0], [1019.4496624146437, 2197.0], [1020.1745474073997, 2201.6666666666665], [1020.8993426878341, 2200.6666666666665], [1021.6240482260512, 2207.3333333333335], [1022.3486639921551, 2201.0], [1023.0731899562501, 2227.3333333333335], [1023.7976260884399, 2220.3333333333335], [1024.5219723588289, 2223.0], [1025.2462287375213, 2189.3333333333335], [1025.9703951946203, 2188.6666666666665], [1026.6944717002311, 2179.3333333333335], [1027.4184582244577, 2189.6666666666665], [1028.1423547374036, 2187.3333333333335], [1028.8661612091732, 2198.3333333333335], [1029.5898776098707, 2194.0], [1030.3135039096003, 2201.6666666666665], [1031.0370400784655, 2197.6666666666665], [1031.7604860865708, 2200.6666666666665], [1032.4838419040204, 2195.0], [1033.2071075009185, 2194.0], [1033.930282847369, 2192.3333333333335], [1034.6533679134757, 2200.0], [1035.3763626693433, 2204.3333333333335], [1036.0992670850753, 2199.3333333333335], [1036.8220811307763, 2187.3333333333335], [1037.54480477655, 2181.6666666666665], [1038.2674379925008, 2187.3333333333335], [1038.989980748733, 2190.6666666666665], [1039.7124330153501, 2189.3333333333335], [1040.4347947624565, 2188.6666666666665], [1041.1570659601564, 2227.6666666666665], [1041.8792465785536, 2235.0], [1042.6013365877527, 2241.6666666666665], [1043.3233359578574, 2204.3333333333335], [1044.0452446589718, 2196.0], [1044.7670626612, 2202.0], [1045.4887899346463, 2202.3333333333335], [1046.210426449415, 2204.3333333333335], [1046.9319721756096, 2190.6666666666665], [1047.6534270833345, 2184.6666666666665], [1048.374791142694, 2178.6666666666665], [1049.0960643237918, 2182.3333333333335], [1049.817246596732, 2193.6666666666665], [1050.5383379316193, 2197.6666666666665], [1051.2593382985572, 2199.0], [1051.98024766765, 2189.0], [1052.701066009002, 2192.6666666666665], [1053.4217932927168, 2192.3333333333335], [1054.142429488899, 2198.0], [1054.8629745676524, 2196.6666666666665], [1055.5834284990813, 2191.6666666666665], [1056.3037912532898, 2184.3333333333335], [1057.0240628003817, 2177.3333333333335], [1057.7442431104614, 2177.0], [1058.4643321536328, 2184.6666666666665], [1059.1843299000002, 2187.6666666666665], [1059.9042363196675, 2194.3333333333335], [1060.6240513827388, 2197.3333333333335], [1061.3437750593187, 2199.3333333333335], [1062.0634073195104, 2195.6666666666665], [1062.7829481334188, 2191.0], [1063.5023974711476, 2190.6666666666665], [1064.221755302801, 2195.3333333333335], [1064.9410215984833, 2198.6666666666665], [1065.660196328298, 2206.3333333333335], [1066.37927946235, 2201.0], [1067.0982709707428, 2199.3333333333335], [1067.817170823581, 2194.3333333333335], [1068.535978990968, 2190.0], [1069.2546954430086, 2188.6666666666665], [1069.9733201498063, 2190.3333333333335], [1070.6918530814655, 2193.3333333333335], [1071.4102942080906, 2190.0], [1072.1286434997853, 2185.6666666666665], [1072.846900926654, 2184.0], [1073.5650664588002, 2186.3333333333335], [1074.2831400663283, 2193.6666666666665], [1075.0011217193428, 2197.0], [1075.7190113879476, 2190.3333333333335], [1076.4368090422465, 2178.3333333333335], [1077.1545146523438, 2162.6666666666665], [1077.8721281883438, 2158.0], [1078.5896496203502, 2169.6666666666665], [1079.3070789184671, 2182.6666666666665], [1080.0244160527993, 2200.3333333333335], [1080.74166099345, 2197.3333333333335], [1081.4588137105238, 2200.6666666666665], [1082.1758741741248, 2195.6666666666665], [1082.892842354357, 2197.6666666666665], [1083.6097182213246, 2199.0], [1084.3265017451313, 2194.6666666666665], [1085.0431928958817, 2183.0], [1085.7597916436796, 2183.6666666666665], [1086.4762979586292, 2190.6666666666665], [1087.1927118108347, 2184.3333333333335], [1087.9090331704003, 2165.6666666666665], [1088.6252620074295, 2146.3333333333335], [1089.341398292027, 2147.3333333333335], [1090.0574419942966, 2151.0]]
  out "pulsed g2 output":u16[][](array[numeric])=[[0], [0], [0], [0], [0], [0], [0], [0], [0], [0], [0], [0], [0], [0], [0], [0], [0], [0], [0], [0], [0], [0], [0], [0], [0], [0], [0], [0], [0], [0], [0], [0], [1], [0], [0], [1], [0], [0], [1], [0], [1], [1], [5], [23], [4], [4], [2], [0], [1], [0], [0], [0], [0], [0], [1], [0], [1], [0], [0], [0], [0], [0], [0], [0], [1], [0], [1], [0], [0], [0], [0], [0], [0], [1], [0], [1], [0], [0], [0], [0], [0], [0], [1], [2], [12], [28], [8], [2], [0], [0], [1], [0], [0], [0], [0], [0], [0], [0], [0], [0], [0], [0], [1], [0], [1], [0], [0], [0], [0], [0], [0], [0], [0], [0], [0], [1], [0], [0], [0], [0], [0], [0], [3], [0], [0], [4], [16], [19], [6], [3], [0], [0], [0], [0], [0], [0], [1], [1], [1], [0], [0], [0], [0], [0], [0], [0], [1], [0], [1], [0], [0], [0], [0], [0], [0], [0], [0], [0], [1], [0], [0], [0], [0], [0], [2], [3], [1], [7], [22], [4], [0], [1], [1], [0], [1], [0], [0], [0], [0], [1], [1], [0], [0], [0], [0], [0], [0], [0], [0], [0], [0], [1], [2], [0], [0], [0], [1], [0], [0], [0], [0], [0], [0], [0], [0], [0], [1], [0], [0], [14], [19], [7], [4], [0], [0], [0], [0], [1], [0], [1], [0], [0], [0], [0], [0], [0], [0], [0], [0], [0], [0], [0], [0], [0], [0], [0], [1], [1], [0], [0], [1], [0], [0], [0], [0], [0], [0], [1], [1], [1], [3], [18], [14], [4], [2], [0], [1], [0], [0], [0], [1], [0], [0], [0], [0], [1], [0], [0], [0], [0], [0], [0], [0], [0], [0], [0], [0], [0], [1], [0], [0], [0], [0], [0], [0], [0], [0], [0], [0], [0], [1], [0], [5], [23], [11], [2], [0], [0], [0], [0], [0], [0], [0], [0], [0], [1], [0], [1], [0], [0], [0], [1], [0], [0], [1], [0], [0], [0], [0], [0], [0], [0], [0], [0], [0], [0], [0], [0], [0], [0], [0], [0], [1], [1], [14], [13], [5], [1], [0], [1], [0], [0], [0], [0], [0], [0], [0], [0], [0], [0], [0], [0], [0], [0], [0], [0], [0], [0], [0], [0], [0], [0], [0], [0], [0], [0], [0], [0], [2], [1], [1], [0], [0], [1], [2], [4], [21], [11], [4], [3], [0], [0], [0], [0], [0], [0], [0], [0], [0], [0], [0], [0], [0], [0], [0], [1], [1], [0], [0], [0], [2], [0], [0], [0], [1], [0], [0], [0], [0], [1], [0], [0], [0], [0], [0], [0], [1], [5], [26], [8], [5], [0], [2], [0], [0], [1], [0], [0], [0], [0], [0], [0], [0], [0], [0], [0], [0], [0], [1], [0], [1], [0], [0], [0], [0], [0], [0], [0], [0], [0], [2], [0], [0], [0], [1], [0], [0], [1], [1], [11], [23], [8], [1], [0], [1], [0], [0], [0], [0], [1], [0], [0], [0], [0], [0], [0], [0], [0], [0], [0], [0], [1], [1], [1], [0], [0], [3], [0], [1], [1], [1], [0], [0], [0], [1], [1], [0], [0], [0], [1], [1], [9], [18], [5], [3], [0], [0], [0], [0], [0], [0], [0], [0], [0], [0], [0], [0], [1], [0], [0], [2], [2], [0], [0], [2], [0], [0], [0], [0], [0], [0], [0], [0], [0], [0], [0], [0], [0], [0], [0], [3], [3], [3], [17], [12], [4], [0], [1], [0], [0], [0], [0], [0], [0], [0], [0], [0], [0], [0], [0], [0], [1], [0], [0], [0], [0], [0], [0], [0], [0], [0], [1], [0], [0], [0], [0], [0], [0], [0], [0], [0], [0], [0], [1], [10], [23], [3], [2], [0], [0], [0], [1], [0], [0], [1], [1], [0], [0], [1], [0], [1], [0], [0], [0], [1], [0], [0], [0], [1], [1], [0], [0], [0], [0], [0], [0], [0], [0], [0], [0], [0], [0], [0], [1], [2], [2], [17], [20], [4], [3], [3], [0], [0], [0], [0], [0], [1], [0], [0], [0], [0], [0], [0], [0], [0], [0], [0], [0], [0], [0], [0], [0], [0], [1], [0], [0], [0], [1], [0], [0], [1], [1], [0], [0], [0], [2], [0], [3], [15], [15], [3], [0], [0], [0], [0], [0], [0], [0], [0], [0], [1], [0], [1], [0], [0], [1], [0], [0], [0], [0], [0], [1], [0], [0], [0], [0], [0], [0], [0], [0], [0], [0], [0], [1], [0], [0], [0], [0], [2], [4], [25], [10], [2], [0], [0], [0], [0], [0], [0], [0], [0], [0], [0], [0], [0], [0], [0], [1], [2], [0], [0], [0], [0], [0], [1], [0], [0], [0], [0], [0], [0], [0], [0], [0], [1], [0], [0], [0], [0], [1], [2], [9], [21], [6], [1], [0], [0], [0], [0], [0], [0], [0], [0], [0], [0], [0], [0], [2], [0], [0], [0], [0], [0], [0], [0], [0], [0], [0], [0], [0], [0], [0], [1], [0], [0], [0], [0], [0], [0], [1], [1], [2], [2], [17], [16], [7], [0], [0], [0], [1], [0], [0], [0], [0], [0], [0], [0], [0], [0], [0], [0], [0], [0], [0], [0], [0], [0], [0], [0], [0], [0], [0], [0], [0], [0], [0], [0], [0], [0], [0], [1], [0], [1], [0], [5], [15], [12], [5], [1], [0], [1], [1], [0], [0], [0], [1], [0], [0], [0], [0], [0], [0], [0], [0], [0], [0], [0], [1], [0], [0], [0], [1], [0], [1], [0], [0], [0], [0], [0], [0], [0], [0], [0], [0], [0], [2], [1], [18], [19], [3], [0], [1], [1], [0], [0], [0], [0], [0], [1], [0], [1], [0], [0], [0], [0], [0], [0], [0], [0], [0], [0], [1], [0], [0], [0], [0], [0], [0], [0], [0], [0], [0], [0], [0], [0], [0], [0], [2], [5], [20], [5], [3], [2], [1], [0], [0], [1], [0], [0], [0], [0], [0], [0], [0], [1], [0], [0], [0], [0], [0], [0], [0], [0], [1], [0], [0], [0], [0], [0], [0], [0], [0], [0], [0], [0], [1], [0], [1], [0], [3], [5], [17], [11], [2], [0], [0], [0], [0], [1], [1], [0], [0], [0], [0], [0], [1], [0], [0], [0], [0], [0], [0], [0], [0], [0], [0], [0], [0], [1], [0], [0], [0], [0], [0], [0], [0], [0], [0], [0], [0], [0], [0], [0], [0], [0], [0], [0], [0], [0], [0], [0], [0], [0], [0], [0], [0], [0], [0], [0], [0], [0], [0], [0], [0], [3], [0], [1], [4], [3], [0], [1], [3], [1], [0], [0], [1], [2], [2], [4], [4], [1], [2], [2], [1], [1], [3], [1], [3], [2], [3], [3], [2], [4], [0], [4], [1], [3], [0], [3], [0], [2], [1], [1], [1], [0], [1], [0], [1], [3], [2], [0], [2], [3], [1], [1], [2], [2], [4], [3], [3], [3], [3], [3], [4], [3], [2], [0], [0], [3], [2], [2], [1], [0], [3], [1], [1], [1], [0], [2], [0], [2], [1], [2], [3], [2], [2], [1], [1], [1], [1], [2], [1], [1], [1], [3], [0], [1], [0], [3], [2], [0], [5], [0], [0], [1], [0], [3], [1], [2], [4], [0], [2], [5], [0], [1], [3], [1], [0], [0], [1], [2], [2], [1], [2], [2], [0], [1], [1], [1], [1], [0], [0], [2], [2], [0], [1], [1], [1], [2], [3], [1], [1], [1], [0], [0], [1], [1], [3], [1], [0], [1], [1], [2], [5], [2], [0], [2], [2], [0], [3], [1], [0], [0], [0], [0], [0], [1], [4], [0], [3], [1], [0], [1], [1], [1], [1], [1], [1], [0], [0], [1], [1], [2], [0], [1], [2], [0], [1], [0], [0], [3], [1], [1], [1], [0], [1], [2], [2], [1], [0], [2], [1], [3], [0], [3], [2], [0], [1], [1], [3], [0], [3], [3], [1], [2], [3], [0], [0], [1], [2], [0], [2], [0], [2], [1], [0], [0], [0], [0], [0], [4], [3], [2], [1], [0], [1], [1], [4], [1], [0], [0], [1], [0], [2], [4], [0], [0], [3], [1], [1], [2], [1], [1], [2], [2], [4], [0], [2], [2], [2], [3], [0], [1], [2], [0], [4], [1], [0], [0], [2], [2], [4], [1], [0], [2], [0], [1], [0], [0], [3], [3], [1], [0], [1], [0], [2], [0], [1], [0], [2], [0], [2], [2], [0], [2], [0], [5], [1], [2], [2], [0], [0], [0], [0], [2], [1], [3], [1], [0], [0], [0], [0], [1], [1], [1], [0], [1], [3], [3], [0], [2], [1], [1], [1], [1], [2], [5], [0], [1], [1], [2], [3], [2], [0], [3], [0], [2], [3], [1], [0], [1], [1], [3], [2], [0], [0], [4], [1], [0], [1], [1], [0], [0], [2], [0], [0], [0], [4], [2], [0], [1], [0], [1], [1], [1], [2], [1], [2], [1], [0], [1], [1], [1], [0], [0], [1], [0], [1], [0], [2], [2], [1], [1], [3], [2], [0], [1], [2], [1], [5], [1], [0], [1], [1], [1], [0], [0], [1], [1], [2], [1], [1], [2], [3], [2], [4], [4], [0], [0], [0], [1], [1], [2], [3], [2], [1], [1], [1], [2], [1], [1], [0], [1], [3], [1], [1], [1], [0], [0], [0], [0], [2], [0], [1], [3], [0], [0], [1], [0], [3], [0], [1], [1], [1], [2], [0], [0], [1], [1], [1], [0], [3], [0], [0], [1], [2], [2], [0], [0], [0], [2], [0], [2], [6], [0], [1], [1], [0], [0], [2], [1], [2], [2], [0], [1], [3], [2], [2], [0], [1], [1], [0], [2], [2], [1], [0], [0], [0], [0], [4], [2], [2], [2], [2], [1], [1], [4], [1], [1], [2], [2], [0], [2], [1], [3], [1], [1], [1], [0], [1], [0], [0], [3], [1], [2], [1], [0], [1], [1], [0], [1], [2], [1], [1], [1], [1], [0], [1], [0], [1], [0], [1], [3], [2], [1], [0], [2], [2], [0], [0], [1], [2], [2], [3], [1], [2], [3], [1], [1], [5], [0], [0], [1], [0], [1], [0], [1], [1], [0], [0], [3], [2], [2], [0], [1], [1], [2], [0], [1], [2], [2], [0], [2], [1], [3], [1], [0], [2], [1], [0], [0], [2], [0], [0], [0], [0], [0], [0], [1], [3], [0], [2], [2], [1], [1], [2], [0], [1], [1], [1], [1], [1], [2], [0], [1], [2], [2], [1], [1], [2], [0], [1], [1], [1], [2], [0], [1], [0], [0], [1], [2], [1], [4], [0], [1], [0], [0], [2], [1], [2], [0], [0], [1], [1], [3], [1], [0], [1], [1], [3], [2], [0], [0], [0], [0], [6], [0], [1], [1], [0], [0], [1], [1], [0], [1], [1], [1], [0], [0], [0], [2], [1], [1], [1], [1], [1], [3], [0], [1], [0], [1], [3], [2], [1], [1], [1], [1], [1], [1], [2], [0], [1], [0], [0], [0], [0], [1], [1], [0], [0], [1], [3], [1], [2], [2], [1], [1], [1], [1], [1], [2], [1], [2], [0], [2], [2], [2], [2], [2], [2], [0], [0], [4], [0], [0], [2], [0], [3], [0], [1], [1], [0], [1], [2], [1], [2], [0], [0], [0], [1], [2], [0], [0], [1], [1], [1], [0], [1], [3], [2], [2], [0], [2], [0], [1], [1], [2], [0], [0], [2], [1], [1], [1], [0], [2], [1], [0], [4], [0], [0], [1], [3], [1], [0], [1], [0], [0], [2], [1], [1], [0], [2], [1], [1], [0], [1], [1], [0], [1], [1], [1], [0], [0], [1], [0], [1], [0], [0], [1], [0], [1], [0], [1], [1], [3], [4], [0], [1], [2], [2], [0], [0], [0], [2], [1], [2], [1], [1], [3], [2], [1], [0], [1], [2], [1], [2], [2], [1], [1], [4], [3], [1], [1], [0], [0], [1], [0], [2], [0], [1], [3], [3], [1], [2], [2], [2], [0], [0], [0], [2], [1], [0], [1], [2], [1], [2], [2], [3], [0], [1], [1], [3], [2], [0], [0], [0], [0], [2], [0], [3], [0], [2], [0], [0], [3], [0], [0], [1], [2], [1], [0], [0], [3], [0], [0], [1], [1], [1], [1], [0], [0], [4], [0], [2], [0], [0], [0], [1], [0], [0], [1], [2], [1], [0], [0], [0], [2], [1], [0], [0], [0], [0], [0], [0], [0], [0], [0], [1], [2], [0], [0], [0], [0], [1], [1], [1], [1], [2], [1], [0], [0], [1], [1], [3], [0], [0], [1], [1], [0], [3], [0], [1], [0], [3], [1], [2], [1], [2], [0], [1], [1], [0], [1], [1], [0], [2], [1], [1], [0], [2], [0], [1], [0], [1], [1], [1], [1], [0], [1], [0], [1], [0], [2], [1], [0], [1], [1], [0], [1], [0], [0], [2], [2], [2], [0], [2], [2], [1], [0], [2], [1], [0], [2], [2], [1], [0], [2], [0], [1], [1], [0], [0], [2], [0], [1], [1], [0], [1], [0], [0], [1], [2], [2], [1], [2], [1], [0], [1], [0], [0], [2], [0], [1], [2], [1], [0], [0], [0], [2], [2], [1], [1], [1], [1], [2], [2], [1], [1], [1], [0], [0], [2], [0], [0], [1], [0], [1], [1], [0], [0], [0], [1], [1], [2], [0], [1], [2], [0], [3], [2], [2], [0], [0], [2], [1], [2], [0], [0], [1], [2], [2], [1], [2], [0], [0], [0], [0], [1], [2], [1], [0], [2], [1], [0], [1], [3], [1], [2], [2], [0], [0], [1], [1], [1], [1], [1], [2], [1], [0], [1], [4], [0], [3], [0], [0], [3], [0], [1], [0], [2], [1], [1], [0], [0], [1], [1], [1], [2], [0], [1], [1], [0], [1], [1], [0], [1], [1], [2], [0], [2], [1], [0], [1], [1], [0], [1], [0], [1], [1], [0], [4], [0], [1], [1], [1], [0], [2], [1], [0], [1], [2], [2], [0], [1], [1], [1], [1], [1], [1], [0], [0], [2], [0], [0], [0], [1], [1], [1], [0], [0], [0], [0], [3], [0], [1], [1], [0], [2], [3], [2], [1], [2], [1], [0], [1], [2], [0], [0], [1], [2], [1], [1], [0], [1], [3], [2], [1], [0], [1], [2], [2], [1], [1], [0], [2], [0], [0], [2], [3], [3], [3], [3], [0], [0], [0], [2], [0], [0], [1], [1], [0], [2], [0], [0], [3], [2], [0], [0], [4], [4], [0], [0], [4], [1], [2], [0], [2], [2], [0], [0], [0], [0], [0], [2], [0], [3], [1], [0], [1], [3], [1], [0], [1], [1], [0], [0], [0], [2], [0], [0], [2], [0], [1], [1], [1], [2], [1], [3], [4], [2], [0], [1], [1], [0], [1], [0], [2], [3], [1], [1], [1], [3], [2], [0], [0], [0], [1], [1], [2], [2], [2], [2], [0], [1], [2], [0], [0], [0], [1], [2], [0], [0], [0], [1], [1], [0], [0], [3], [0], [4], [1], [2], [0], [2], [1], [2], [1], [0], [0], [1], [0], [1], [2], [2], [1], [2], [0], [0], [1], [0], [0], [0], [0], [0], [0], [1], [1], [1], [0], [3], [1], [1], [1], [1], [1], [1], [1], [0], [0], [0], [0], [1], [0], [1], [0], [0], [1], [2], [0], [1], [2], [0], [2], [0], [1], [0], [0], [2], [0], [1], [0], [0], [0], [0], [0], [0], [0], [1], [0], [0], [0], [3], [2], [6], [0], [2], [1], [0], [1], [0], [3], [0], [2], [0], [1], [2], [1], [0], [2], [2], [1], [0], [0], [1], [1], [1], [1], [0], [2], [2], [0], [0], [2], [1], [2], [1], [0], [1], [0], [0], [2], [1], [1], [2], [1], [3], [0], [0], [0], [1], [0], [0], [0], [2], [2], [1], [1], [3], [1], [0], [0], [1], [1], [2], [1], [1], [0], [0], [1], [0], [0], [2], [0], [1], [0], [0], [0], [2], [1], [0], [0], [1], [3], [1], [1], [1], [0], [0], [1], [0], [0], [1], [1], [0], [0], [1], [0], [1], [1], [2], [0], [0], [3], [2], [2], [0], [1], [0], [3], [1], [2], [0], [0], [0], [1], [0], [1], [0], [1], [1], [0], [2], [0], [2], [1], [0], [1], [0], [1], [2], [1], [1], [2], [0], [0], [2], [0], [0], [0], [0], [3], [2], [1], [1], [1], [0], [0], [1], [2], [0], [1], [2], [0], [1], [2], [0], [3], [2], [1], [2], [1], [0], [1], [0], [0], [1], [0], [1], [1], [0], [1], [0], [1], [0], [1], [0], [0], [1], [0], [1], [1], [2], [1], [0], [1], [0], [1], [0], [0], [6], [0], [0], [0], [1], [0], [1], [1], [1], [1], [0], [1], [1], [0], [0], [1], [0], [2], [0], [1], [0], [2], [0], [0], [0], [1], [1], [2], [2], [1], [1], [0], [2], [0], [1], [2], [0], [0], [1], [1], [0], [0], [0], [1], [1], [1], [1], [0], [1], [0], [1], [0], [0], [0], [1], [0], [0], [1], [0], [2], [2], [1], [1], [2], [1], [1], [0], [3], [1], [2], [2], [1], [0], [0], [3], [0], [1], [3], [4], [1], [0], [1], [0], [1], [1], [0], [0], [3], [1], [0], [5], [1], [2], [1], [1], [2], [1], [0], [0], [1], [1], [0], [1], [1], [1], [1], [1], [0], [3], [1], [1], [0], [0], [0], [1], [3], [0], [2], [0], [0], [1], [0], [1], [0], [3], [0], [1], [3], [0], [1], [1], [4], [2], [0], [1], [1], [3], [3], [0], [0], [1], [2], [1], [2], [0], [2], [0], [0], [1], [2], [1], [3], [1], [1], [2], [3], [1], [0], [2], [1], [1], [4], [1], [0], [2], [0], [0], [0], [1], [3], [1], [0], [0], [0], [0], [0], [1], [2], [1], [1], [1], [1], [1], [1], [1], [0], [1], [1], [3], [1], [3], [0], [0], [1], [0], [1], [1], [1], [3], [1], [3], [0], [2], [1], [1], [0], [0], [0], [0], [0], [1], [1], [2], [2], [1], [1], [0], [1], [1], [0], [1], [1], [1], [0], [2], [1], [0], [0], [0], [1], [1], [1], [0], [1], [0], [0], [1], [0], [3], [3], [0], [1], [0], [0], [0], [1], [2], [1], [1], [1], [1], [1], [1], [2], [0], [0], [3], [0], [2], [2], [1], [1], [2], [5], [1], [1], [2], [0], [1], [2], [2], [1], [0], [0], [2], [2], [1], [0], [0], [1], [1], [0], [0], [4], [1], [2], [0], [2], [1], [3], [1], [1], [0], [0], [0], [1], [2], [1], [2], [4], [0], [2], [1], [0], [3], [1], [1], [0], [3], [1], [1], [0], [1], [0], [1], [0], [0], [2], [0], [1], [0], [0], [1], [0], [0], [3], [0], [0], [0], [0], [1], [1], [0], [0], [4], [2], [0], [1], [0], [2], [1], [1], [1], [1], [1], [1], [1], [2], [0], [0], [0], [3], [2], [0], [1], [0], [0], [1], [1], [0], [2], [0], [1], [1], [2], [1], [1], [2], [4], [0], [0], [2], [0], [1], [4], [0], [1], [0], [1], [1], [1], [1], [1], [0], [2], [0], [2], [0], [0], [0], [1], [0], [1], [0], [1], [0], [0], [0], [0], [0], [1], [0], [1], [1], [0], [0], [1], [2], [1], [0], [0], [1], [1], [2], [0], [0], [2], [3], [1], [0], [1], [0], [0], [3], [1], [0], [1], [3], [0], [1], [1], [1], [0], [0], [0], [0], [2], [1], [1], [0], [0], [0], [1], [0], [2], [2], [0], [1], [1], [1], [1], [2], [0], [1], [0], [0], [0], [0], [1], [0], [3], [2], [2], [0], [1], [1], [0], [0], [0], [2], [1], [1], [2], [1], [2], [0], [2], [0], [0], [3], [1], [1], [1], [2], [1], [0], [1], [2], [0], [0], [0], [0], [0], [1], [2], [0], [0], [0], [0], [1], [0], [0], [2], [0], [0], [0], [0], [1], [0], [2], [3], [1], [1], [1], [2], [1], [5], [1], [2], [1], [0], [0], [1], [0], [2], [2], [0], [1], [0], [1], [0], [0], [1], [0], [0], [1], [0], [1], [1], [3], [0], [0], [2], [2], [0], [0], [1], [0], [0], [1], [1], [0], [1], [1], [2], [1], [0], [0], [1], [2], [1], [0], [0], [1], [1], [2], [0], [2], [0], [1], [1], [1], [0], [2], [0], [2], [0], [0], [0], [1], [0], [0], [1], [0], [0], [1], [2], [0], [0], [0], [0], [2], [0], [2], [0], [0], [0], [0], [1], [1], [0], [1], [2], [0], [2], [1], [1], [1], [0], [2], [0], [0], [1], [1], [1], [0], [1], [0], [2], [1], [1], [1], [1], [1], [3], [2], [2], [2], [0], [0], [0], [2], [0], [2], [2], [0], [1], [0], [2], [1], [0], [2], [0], [3], [0], [3], [0], [0], [1], [1], [1], [0], [1], [2], [1], [0], [1], [0], [1], [0], [1], [3], [0], [0], [0], [0], [0], [2], [2], [1], [0], [0], [0], [2], [0], [0], [0], [1], [1], [0], [2], [1], [2], [1], [2], [1], [2], [0], [1], [1], [0], [0], [0], [0], [1], [2], [0], [1], [1], [1], [0], [0], [2], [1], [1], [1], [0], [0], [2], [0], [0], [1], [1], [1], [1], [0], [1], [0], [1], [1], [0], [1], [0], [0], [0], [2], [0], [0], [2], [0], [0], [0], [0], [1], [0], [1], [0], [2], [0], [0], [0], [2], [0], [2], [0], [0], [1], [0], [0], [2], [3], [1], [0], [0], [0], [1], [1], [0], [0], [0], [0], [3], [2], [0], [1], [0], [1], [0], [0], [1], [0], [1], [2], [0], [0], [0], [0], [3], [0], [1], [0], [0], [0], [1], [0], [0], [1], [2], [1], [0], [0], [0], [0], [1], [1], [3], [1], [0], [0], [2], [2], [1], [1], [0], [1], [4], [1], [0], [2], [0], [1], [0], [1], [0], [0], [1], [0], [1], [0], [0], [1], [0], [1], [0], [2], [3], [0], [0], [1], [1], [1], [0], [1], [0], [0], [2], [0], [1], [0], [0], [1], [0], [0], [0], [0], [1], [1], [0], [1], [1], [0], [2], [3], [0], [0], [3], [2], [1], [0], [1], [1], [2], [1], [1], [0], [2], [1], [4], [0], [1], [1], [0], [0], [2], [0], [1], [0], [1], [1], [1], [1], [0], [1], [0], [1], [0], [0], [4], [1], [3], [2], [0], [0], [0], [0], [0], [2], [0], [1], [1], [1], [3], [0], [2], [0], [2], [1], [1], [3], [1], [2], [0], [2], [3], [1], [1], [2], [0], [1], [0], [0], [2], [0], [1], [0], [1], [0], [0], [0], [1], [1], [2], [0], [0], [3], [3], [2], [0], [2], [1], [0], [0], [2], [0], [1], [3], [1], [0], [2], [0], [2], [0], [1], [1], [2], [0], [1], [3], [0], [1], [0], [2], [0], [1], [1], [1], [1], [2], [1], [0], [3], [1], [2], [5], [2], [0], [1], [1], [0], [0], [0], [0], [0], [1], [0], [0], [0], [2], [0], [0], [1], [2], [2], [1], [2], [1], [0], [2], [0], [1], [0], [0], [3], [2], [0], [1], [0], [2], [0], [3], [1], [1], [0], [0], [1], [1], [1], [2], [2], [1], [2], [3], [1], [2], [3], [1], [0], [3], [1], [2], [1], [1], [1], [1], [0], [1], [1], [1], [0], [0], [2], [1], [0], [0], [2], [1], [1], [0], [0], [0], [1], [1], [3], [0], [2], [0], [0], [2], [3], [0], [2], [1], [1], [2], [2], [0], [0], [0], [0], [2], [0], [0], [0], [0], [0], [2], [2], [0], [0], [1], [0], [2], [3], [0], [2], [1], [1], [1], [1], [2], [0], [1], [1], [2], [1], [0], [1], [2], [1], [1], [2], [1], [3], [1], [1], [2], [0], [1], [1], [2], [0], [1], [1], [0], [1], [2], [0], [0], [1], [0], [0], [0], [0], [0], [1], [0], [2], [2], [2], [1], [0], [0], [1], [0], [1], [1], [2], [1], [0], [1], [0], [2], [0], [1], [3], [2], [3], [0], [2], [0], [2], [1], [1], [1], [2], [1], [0], [0], [0], [2], [3], [0], [0], [0], [0], [0], [1], [2], [0], [0], [2], [2], [2], [2], [1], [0], [0], [0], [2], [1], [2], [1], [1], [0], [0], [2], [1], [0], [3], [2], [0], [0], [0], [0], [1], [0], [3], [0], [1], [2], [0], [0], [0], [1], [2], [0], [1], [2], [0], [0], [2], [1], [1], [1], [1], [2], [0], [1], [4], [1], [1], [0], [0], [0], [0], [2], [0], [1], [0], [2], [1], [2], [0], [1], [2], [1], [0], [0], [1], [0], [0], [1], [0], [0], [2], [2], [1], [2], [2], [0], [0], [0], [0], [0], [2], [2], [0], [1], [2], [1], [0], [1], [1], [0], [1], [2], [2], [1], [2], [1], [3], [0], [2], [1], [1], [1], [1], [1], [0], [0], [2], [0], [1], [0], [2], [1], [0], [1], [3], [1], [1], [1], [1], [3], [1], [0], [0], [1], [2], [1], [2], [1], [1], [1], [0], [3], [1], [0], [1], [0], [2], [1], [2], [0], [1], [0], [2], [1], [0], [1], [0], [2], [2], [0], [2], [0], [2], [0], [3], [0], [2], [1], [0], [1], [0], [1], [1], [2], [0], [0], [0], [2], [0], [1], [2], [2], [1], [1], [0], [0], [0], [3], [0], [3], [0], [1], [0], [1], [2], [1], [1], [0], [0], [1], [3], [1], [0], [1], [0], [0], [1], [2], [0], [1], [1], [1], [0], [2], [2], [1], [1], [1], [1], [0], [1], [1], [2], [1], [0], [0], [0], [0], [0], [0], [0], [0], [0], [0], [0], [0], [0], [0], [0], [0], [0], [0], [0], [0], [0], [0], [0], [0], [0], [0], [0], [0], [0], [0], [0], [0], [0], [0], [0], [0], [0], [0], [0], [0], [0], [0], [0], [0], [0], [0], [0], [0], [0], [0], [0], [0], [0], [0], [0], [0], [0], [0], [0], [0], [0], [0], [0], [0], [0], [0], [0], [0], [0], [0], [0], [0], [0], [0], [0], [0], [0], [0], [0], [0], [0], [0], [0], [0], [0], [0], [0], [0], [0], [0], [0], [0], [0], [0], [0], [0], [0], [0], [0], [0], [0], [0], [0], [0], [0], [0], [0], [0], [0], [0], [0], [0], [0], [0], [0], [0], [0], [0], [0], [0], [0], [0], [0], [0], [0], [0], [0], [0], [0]] caption="Output Array"
  out "TraceDataStab":dbl[][](array[numeric])
  out "# of Steps":i64=5
  out "TraceData":dbl[][](array[numeric])
  in  "Controls":enum32{"Operation", "Parameters", "Setup"}(tab)
  in  "Clear Last Select Point":bool
  in  "Clear Last Filter Position":bool
  out "ADC Resolution [exponent]":T1=10 items=["-1"=-1, "1"=0, "4"=2, "16"=4, "64"=6, "256"=8, "1024"=10, "4096"=12]
  in  "Counter Int time (ms)":T2=100
  in  "Power Meter Int Time (ms)":u32=300
  in  "ctr2":tag="Dev3/ctr2"
  in  "ctr1":tag="Dev3/ctr1"
  out "NI USB-6341 ctr1 Initalization Error":errorcluster
  out "NI USB-6341 ct2 Initalization Error":errorcluster
  in  "ctr0":tag="Dev3/ctr0"
  out "Attenuator Error Out":errorcluster
  out "Filter wheel ID":string
  out "Power Meter COM Ports":string[](array[string])
  out "Flip Motor (Spectrometer) Initialization Error":errorcluster
  out "Flip Motor (Det) Initialization Error":errorcluster
  out "Power Meter Initalization Error":errorcluster caption="error out" {"code" format="%.0x"}
  out "NI USB-6341 ctr0 Initalization Error":errorcluster
  out "Rotation attenuator Initialization Error":errorcluster
  out "NI-USB 6526 Initialization Error":errorcluster
  in  "Filter Configuraton":u16(ring) items=["550 LP", "590 LP", "633 LP", "750 BP (missing)", "850 LP", "None"]
  in  "Min power":bool
  in  "Mirror Configuraton":u16(ring) items=["Spectrometer", "SPCM", "PDMS"]
  in  "Wavelength":dbl=532.0
  out "Saturation Array":dbl[][](array[numeric])=[[1455.9916, 234680.0], [1472.1560000000002, 280400.0], [1132.38475, 190980.0], [37.0804763, 116460.0], [16.538525500000002, 9010.0], [7.547880900000001, 4680.0], [4.952824799999999, 2870.0], [2.5077224900000004, 2140.0], [1.22270078, 1120.0], [0.656095286, 880.0], [9.517986800000001, 750.0], [6741.6808200000005, 185850.0], [6797.00042, 560640.0], [6740.60352, 585290.0], [6833.27274, 536370.0], [6759.937239999999, 530110.0], [6659.60911, 587330.0], [6633.4184, 584510.0], [6605.0009199999995, 596330.0], [6648.2028199999995, 589580.0], [6185.36891, 571350.0], [0.511186732, 550.0], [0.511247814, 1730.0], [0.515731195, 390.0], [0.515676182, 430.0], [0.515566261, 500.0], [0.51405144, 550.0], [0.5262248669999999, 480.0], [0.593377323, 500.0], [0.647287389, 490.0], [0.665856023, 560.0], [0.677583543, 800.0], [0.68986694, 540.0], [0.70512498, 700.0], [0.71768935, 610.0], [0.7217329, 680.0], [0.73452323, 1310.0], [0.76364057, 940.0], [0.77294931, 570.0], [0.77351127, 750.0], [0.8590612799999999, 720.0], [1.03936623, 720.0], [1.1000684799999998, 1070.0], [1.1943714300000001, 740.0], [1.22601136, 1000.0], [1.24475106, 870.0], [1.2496863399999998, 1050.0], [1.2436821599999999, 840.0], [1.59823279, 1240.0], [1.9418438199999999, 1600.0], [2.53862945, 1330.0], [2.96582986, 1840.0], [3.1734563700000002, 2110.0], [3.2214781900000005, 2070.0], [3.33114929, 1940.0], [3.38079595, 2370.0], [3.50932246, 1960.0], [3.81024406, 2460.0], [3.8589376000000004, 2140.0], [3.8588218199999993, 2700.0], [3.8309442500000004, 2080.0], [4.07525608, 2290.0], [5.31388046, 2630.0], [5.76290512, 3340.0], [7.0907816, 3680.0], [10.0290582, 4840.0], [10.7187472, 4760.0], [11.0151188, 4680.0], [11.7129446, 4710.0], [12.222438899999998, 5340.0], [12.519934, 5120.0], [13.1213803, 5710.0], [13.359242400000001, 6260.0], [14.860863499999999, 6460.0], [18.877713399999998, 6510.0], [20.0740939, 7160.0], [21.085736, 6680.0], [21.9301502, 7450.0], [22.400882, 7650.0], [24.0245733, 8250.0], [25.5491376, 9570.0], [25.2947289, 7920.0], [24.9260375, 9220.0], [25.1921733, 8850.0], [38.3423824, 12110.0], [39.1157739, 11160.0], [38.389618399999996, 12720.0], [37.3949702, 12050.0], [37.8927416, 12080.0], [37.8671069, 10420.0], [38.7255988, 12410.0], [40.878367600000004, 10750.0], [41.9340005, 11860.0], [45.9134277, 14570.0], [46.150556200000004, 19850.0], [46.48418110000001, 13180.0], [47.70362659999999, 17520.0], [59.7791768, 15840.0], [68.7891225, 18630.0], [83.33834599999999, 22550.0], [117.08323899999999, 26850.0], [138.106087, 30950.0], [133.954317, 29490.0], [140.860909, 30080.0], [145.44810700000002, 32830.0], [151.565834, 32660.0], [158.99844099999999, 33000.0], [162.066408, 36420.0], [162.044358, 36310.0], [169.234667, 37130.0], [204.94297600000002, 39610.0], [265.021337, 47580.0], [260.20314600000006, 52650.0], [257.091807, 47950.0], [261.115792, 48880.0], [274.047655, 50510.0], [288.012466, 53270.0], [289.892659, 55110.0], [293.272056, 53670.0], [310.369423, 60220.0], [400.66583199999997, 68110.0], [447.878375, 88820.0], [439.00912999999997, 95160.0], [449.24273100000005, 80120.0], [472.442019, 78470.0], [494.045419, 81180.0], [495.132092, 80950.0], [497.648375, 83630.0], [508.320554, 80790.0], [654.6428559999999, 96220.0], [728.5613300000001, 113430.0], [744.19163, 110310.0], [787.1007900000001, 117120.0], [820.62869, 118930.0], [808.22532, 120770.0], [819.27692, 124080.0], [836.5707699999999, 119940.0], [897.07702, 123640.0], [1102.58666, 142160.0], [1205.79368, 155130.0], [1284.67248, 164870.0], [1290.66448, 171850.0], [1406.65224, 194870.0], [1480.35825, 191940.0], [1722.38759, 213440.0], [1865.8108, 227240.0], [1893.08987, 221870.0], [1909.7304800000002, 218510.0], [2068.2971399999997, 233260.0], [2582.28194, 277970.0], [3436.9528200000004, 328380.0], [3897.95196, 381120.0], [4513.89267, 434570.0], [4742.28839, 443470.0], [5117.27118, 465350.0], [5362.627130000001, 510830.0], [5443.36982, 490160.0], [5423.272959999999, 500930.0], [5326.58546, 503620.0], [5317.36149, 503680.0], [5295.75543, 515460.0], [5323.308690000001, 509020.0], [5349.63303, 497140.0], [5362.144759999999, 497440.0], [5363.18335, 486120.0], [5344.46612, 489250.0], [5404.26929, 490350.0], [5417.96507, 508820.0], [5360.72026, 503630.0], [5316.52541, 490470.0], [5417.673309999999, 480340.0], [5431.53121, 492440.0], [5371.67792, 498730.0], [5445.159720000001, 504820.0], [5431.78384, 525340.0], [5480.051219999999, 526270.0], [5426.330489999999, 512170.0], [5385.468620000001, 502900.0], [5402.68148, 519290.0], [5462.21004, 494820.0], [5520.24571, 485030.0], [5545.59418, 484040.0], [5500.2947300000005, 480560.0], [5459.9825, 476810.0], [5486.5321699999995, 505330.0], [5465.16691, 500580.0], [5463.38268, 503450.0], [5483.597699999999, 500210.0], [5512.71105, 509410.0]]
  in  "Restore center":bool
  in  "Last Scan Y":dbl=50.0 format="%.3g"
  in  "Last Scan X":dbl=50.0 format="%.3g"
  in  "HOME":bool
  in  "Tab Control":T3(tab)=enum."Lifetime"
  in  "Stop Auto Spectrum":bool
  out "Spectrum":cluster{"Y":dbl[], "Y":dbl[]}[](graph)
  in  "Measure spectrum":bool
  in  "Write spectrum to file":bool caption="Write to file"
  in  "Auto Spectrum":bool
  in  "Spectrum Integration Time (s)":i32=10 min=10 max=240000000
  out "g2 time remaining":sgl(knob) caption="Time Remaining" scale=0.0..10.0
  in  "Auto g2":bool
  in  "Measure g2":bool
  in  "Write g2 to file":bool caption="Write to file"
  in  "g2 abort":bool
  in  "g2 settings":T4={"tac_range"=50.0, "tac_gain"=1, "tac_offset"=10.0, "tac_limit_high"=97.0, "tac_limit_low"=3.0, "collect_time"=5.0, "sync_threshold"=-50.980392, "sync_zc_level"=-5.2913384, "sync_freq_div"=1, "cfd_limit_low"=-50.980392, "cfd_zc_level"=-5.2999988} {"sync_freq_div" items=["1"=1, "2"=2, "4"=4]; "cfd_zc_level" min=-96 max=96 step=0.1 format="%#_3g"; "cfd_limit_low" min=-500 max=0 step=0.1 format="%#_3g"; "sync_zc_level" min=-96 max=96 step=0.1 format="%#_3g"; "sync_threshold" min=-500 max=-20 step=0.1 format="%#_3g"; "tac_limit_low" format="%.3g"; "tac_limit_high" min=0 max=100 step=0.1 format="%.3g"; "collect_time" min=1e-07 max=100000 step=0.001; "tac_offset" min=0 max=100 step=0.1 format="%.4g"; "tac_gain" min=1 max=15 step=1; "tac_range" format="%^#_6g"}
  out "g2 data":u16[](graph)=[0, 0, 0, 0, 0, 0, 0, 0, 0, 0, 0, 0, 0, 0, 0, 0, 0, 0, 0, 0, 0, 0, 0, 0, 0, 0, 0, 0, 0, 0, 0, 0, 188, 173, 204, 201, 179, 193, 203, 205, 169, 197, 158, 200, 219, 211, 198, 192, 189, 216, 199, 199, 200, 193, 198, 203, 194, 190, 180, 188, 209, 176, 189, 198, 215, 185, 173, 178, 215, 209, 193, 225, 210, 196, 196, 188, 211, 212, 193, 184, 208, 191, 198, 199, 187, 189, 179, 214, 192, 195, 194, 197, 168, 197, 179, 200, 175, 174, 189, 185, 191, 190, 174, 190, 210, 192, 201, 193, 192, 201, 170, 198, 198, 174, 171, 183, 195, 204, 172, 188, 206, 189, 197, 226, 200, 179, 218, 199, 189, 208, 194, 186, 176, 176, 205, 189, 205, 201, 189, 185, 196, 176, 169, 182, 215, 195, 194, 218, 194, 190, 213, 222, 184, 205, 202, 186, 193, 189, 191, 221, 184, 199, 191, 215, 194, 192, 207, 182, 188, 182, 198, 174, 173, 177, 190, 218, 205, 218, 154, 185, 174, 180, 191, 184, 188, 184, 173, 183, 195, 199, 179, 206, 192, 171, 206, 179, 208, 172, 194, 182, 185, 203, 167, 198, 180, 204, 197, 178, 194, 181, 182, 195, 181, 196, 185, 174, 205, 204, 193, 195, 215, 213, 194, 204, 178, 182, 190, 178, 196, 181, 201, 192, 180, 194, 214, 174, 194, 189, 185, 222, 195, 198, 209, 187, 209, 200, 196, 201, 229, 191, 202, 191, 212, 200, 185, 196, 203, 222, 209, 160, 178, 177, 198, 197, 192, 207, 188, 194, 182, 201, 190, 190, 200, 184, 216, 184, 193, 163, 173, 195, 176, 196, 194, 221, 176, 196, 215, 185, 207, 181, 177, 192, 219, 189, 195, 205, 197, 191, 187, 199, 202, 181, 200, 202, 204, 177, 179, 195, 208, 194, 184, 180, 188, 211, 183, 221, 198, 181, 179, 178, 166, 203, 181, 172, 171, 181, 184, 198, 175, 215, 191, 190, 193, 187, 190, 163, 192, 194, 207, 206, 221, 184, 184, 155, 176, 182, 176, 182, 200, 178, 181, 186, 201, 204, 178, 196, 184, 215, 178, 200, 181, 192, 177, 183, 188, 171, 169, 189, 195, 199, 188, 187, 183, 171, 197, 188, 176, 189, 209, 203, 181, 183, 185, 164, 186, 214, 187, 182, 199, 187, 213, 190, 202, 170, 172, 201, 189, 168, 170, 206, 175, 176, 185, 191, 165, 205, 173, 198, 177, 171, 183, 176, 173, 164, 189, 187, 187, 164, 195, 166, 158, 157, 190, 162, 163, 181, 157, 174, 170, 142, 177, 180, 150, 173, 170, 163, 151, 175, 168, 164, 154, 157, 180, 168, 172, 161, 154, 147, 142, 175, 178, 169, 181, 133, 157, 160, 151, 154, 160, 158, 142, 154, 166, 160, 166, 154, 149, 137, 131, 143, 161, 158, 132, 150, 134, 164, 163, 133, 143, 131, 148, 140, 157, 147, 122, 126, 152, 141, 131, 150, 144, 146, 122, 128, 125, 145, 133, 109, 138, 136, 117, 122, 100, 101, 112, 111, 120, 112, 106, 106, 99, 129, 97, 111, 101, 99, 90, 78, 94, 91, 105, 88, 98, 100, 102, 96, 85, 58, 81, 82, 74, 80, 76, 80, 65, 85, 70, 96, 84, 102, 88, 90, 88, 85, 96, 94, 89, 101, 112, 98, 107, 92, 98, 123, 112, 115, 116, 105, 118, 94, 106, 115, 106, 99, 108, 128, 130, 119, 129, 118, 131, 134, 140, 119, 133, 145, 124, 123, 143, 139, 119, 159, 144, 133, 134, 145, 162, 141, 160, 142, 138, 140, 143, 131, 162, 153, 167, 155, 152, 157, 155, 138, 150, 174, 184, 158, 128, 163, 176, 167, 156, 161, 161, 166, 165, 171, 176, 182, 172, 148, 157, 167, 157, 177, 183, 146, 163, 162, 174, 165, 168, 161, 149, 174, 152, 178, 174, 191, 177, 164, 172, 177, 180, 164, 173, 171, 188, 203, 193, 174, 177, 164, 179, 196, 187, 169, 204, 172, 182, 177, 181, 159, 180, 191, 194, 203, 180, 156, 161, 187, 179, 182, 188, 212, 184, 185, 161, 163, 205, 199, 192, 177, 164, 201, 202, 181, 179, 170, 185, 185, 186, 180, 183, 207, 167, 195, 188, 187, 177, 172, 178, 204, 172, 196, 169, 182, 193, 193, 195, 193, 189, 181, 187, 191, 182, 178, 184, 195, 181, 192, 176, 149, 189, 197, 165, 184, 199, 169, 177, 173, 202, 183, 169, 197, 203, 184, 191, 166, 157, 176, 188, 183, 172, 217, 211, 188, 183, 178, 178, 182, 179, 175, 172, 184, 197, 187, 162, 172, 192, 178, 184, 180, 187, 177, 206, 174, 190, 208, 195, 188, 201, 187, 176, 197, 203, 207, 191, 224, 194, 198, 193, 191, 199, 192, 189, 192, 177, 204, 208, 192, 213, 193, 198, 185, 155, 202, 190, 200, 193, 171, 170, 165, 171, 202, 191, 170, 192, 190, 226, 231, 183, 192, 189, 197, 192, 180, 183, 199, 188, 169, 158, 199, 189, 182, 168, 175, 214, 184, 173, 182, 194, 180, 190, 195, 186, 170, 171, 206, 199, 190, 188, 174, 188, 185, 208, 200, 203, 184, 184, 192, 176, 193, 165, 189, 178, 163, 199, 191, 181, 188, 195, 175, 203, 202, 186, 198, 182, 207, 191, 213, 194, 183, 186, 182, 204, 196, 193, 190, 209, 187, 179, 225, 174, 221, 193, 189, 199, 209, 210, 190, 218, 202, 192, 207, 185, 199, 210, 209, 202, 190, 203, 197, 216, 180, 208, 217, 186, 190, 183, 200, 181, 194, 218, 184, 178, 188, 150, 202, 200, 169, 162, 185, 204, 186, 204, 192, 176, 187, 211, 217, 208, 190, 195, 167, 206, 173, 215, 198, 172, 208, 182, 191, 178, 195, 196, 186, 171, 195, 188, 182, 179, 197, 186, 200, 208, 176, 195, 180, 192, 214, 206, 192, 207, 201, 172, 205, 219, 197, 176, 202, 177, 164, 189, 204, 206, 169, 191, 188, 179, 193, 198, 181, 179, 236, 188, 193, 215, 203, 209, 198, 199, 182, 0, 0, 0, 0, 0, 0, 0, 0, 0, 0, 0, 0, 0, 0, 0, 0, 0, 0, 0, 0, 0, 0, 0, 0, 0, 0, 0, 0, 0, 0, 0, 0]
  in  "Auto lifetime":bool
  in  "Write lifetime to file":bool caption="Write to file"
  in  "Meaure lifetime":bool
  out "lifetime data":u16[](graph)=[0, 0, 0, 0, 0, 0, 0, 0, 0, 0, 0, 0, 0, 0, 0, 0, 0, 0, 0, 0, 0, 0, 0, 0, 0, 0, 0, 0, 0, 0, 0, 0, 64, 48, 63, 72, 64, 56, 55, 57, 57, 67, 49, 49, 59, 60, 56, 58, 63, 54, 59, 43, 55, 53, 61, 58, 69, 59, 69, 55, 56, 67, 54, 59, 55, 57, 51, 53, 57, 64, 67, 69, 38, 65, 66, 48, 64, 49, 42, 39, 55, 60, 71, 59, 58, 60, 56, 57, 47, 54, 66, 53, 73, 68, 63, 45, 55, 53, 58, 57, 53, 60, 53, 47, 76, 45, 54, 58, 58, 57, 57, 71, 63, 51, 58, 52, 55, 65, 64, 51, 66, 57, 59, 64, 53, 65, 49, 61, 60, 54, 52, 73, 57, 48, 68, 97, 214, 796, 1523, 2126, 2428, 2565, 2617, 2716, 2678, 2807, 2743, 2712, 2789, 2747, 2850, 2684, 2717, 2570, 2508, 2600, 2497, 2458, 2349, 2456, 2292, 2281, 2247, 2241, 2223, 2139, 2199, 2178, 2147, 2048, 2072, 2090, 1991, 1912, 1880, 1814, 1870, 1914, 1861, 1750, 1765, 1773, 1656, 1700, 1710, 1637, 1589, 1633, 1606, 1640, 1585, 1528, 1510, 1532, 1475, 1448, 1479, 1428, 1432, 1449, 1336, 1328, 1344, 1289, 1253, 1291, 1273, 1296, 1213, 1223, 1192, 1180, 1162, 1159, 1112, 1157, 1120, 1093, 1075, 1070, 1077, 1066, 1068, 1062, 1013, 983, 942, 1015, 956, 930, 969, 952, 857, 920, 929, 887, 874, 839, 832, 859, 866, 889, 839, 785, 758, 790, 795, 789, 724, 770, 787, 737, 693, 711, 752, 746, 771, 697, 671, 618, 725, 680, 628, 627, 657, 644, 602, 622, 611, 585, 588, 581, 569, 602, 613, 577, 527, 563, 555, 564, 529, 515, 555, 530, 533, 522, 460, 483, 532, 507, 531, 528, 479, 536, 475, 461, 458, 468, 420, 434, 444, 433, 373, 441, 448, 432, 405, 429, 391, 388, 390, 371, 400, 410, 383, 383, 359, 364, 378, 366, 398, 357, 341, 346, 336, 328, 341, 343, 322, 315, 329, 325, 304, 310, 279, 336, 304, 300, 301, 295, 303, 298, 305, 280, 296, 251, 289, 284, 272, 274, 276, 242, 252, 274, 286, 259, 275, 256, 261, 279, 242, 267, 236, 234, 211, 268, 248, 226, 218, 210, 214, 216, 222, 218, 217, 224, 205, 218, 223, 216, 219, 194, 207, 199, 225, 204, 206, 201, 176, 188, 193, 172, 215, 209, 177, 189, 195, 201, 198, 189, 171, 169, 175, 163, 192, 176, 179, 166, 174, 179, 172, 165, 151, 166, 157, 168, 158, 171, 116, 149, 151, 158, 204, 167, 166, 128, 151, 170, 151, 116, 148, 149, 161, 126, 147, 137, 134, 160, 134, 153, 140, 138, 140, 128, 140, 122, 120, 127, 139, 113, 122, 125, 143, 126, 120, 131, 116, 141, 137, 121, 139, 116, 130, 106, 132, 111, 136, 119, 108, 128, 133, 137, 108, 123, 126, 110, 112, 122, 106, 123, 131, 126, 121, 114, 128, 104, 122, 108, 110, 107, 97, 113, 99, 85, 113, 124, 98, 102, 124, 103, 98, 96, 101, 97, 107, 94, 103, 88, 82, 95, 102, 78, 99, 104, 92, 89, 99, 89, 117, 97, 90, 108, 89, 104, 89, 109, 104, 90, 79, 80, 84, 112, 92, 91, 107, 86, 91, 84, 95, 110, 79, 87, 103, 86, 98, 103, 94, 79, 88, 94, 95, 93, 101, 76, 76, 74, 83, 84, 68, 77, 82, 86, 82, 81, 77, 82, 98, 82, 99, 83, 88, 87, 57, 75, 70, 77, 79, 81, 77, 85, 105, 73, 90, 90, 89, 92, 84, 76, 90, 85, 80, 74, 78, 81, 85, 86, 77, 69, 78, 80, 70, 84, 81, 78, 81, 89, 89, 76, 69, 75, 75, 87, 76, 78, 80, 65, 72, 85, 79, 70, 75, 86, 75, 67, 73, 77, 67, 81, 67, 81, 76, 65, 61, 63, 62, 92, 87, 79, 76, 68, 69, 84, 63, 74, 66, 66, 75, 83, 62, 76, 72, 73, 71, 69, 62, 71, 78, 75, 66, 61, 65, 64, 73, 67, 73, 54, 72, 77, 66, 79, 61, 72, 86, 75, 72, 88, 62, 91, 70, 71, 64, 80, 72, 75, 69, 66, 78, 65, 68, 57, 65, 73, 55, 61, 55, 65, 74, 81, 64, 62, 76, 41, 71, 64, 72, 76, 69, 69, 63, 63, 72, 79, 63, 70, 77, 83, 58, 67, 69, 54, 63, 63, 63, 56, 77, 66, 75, 59, 70, 53, 72, 60, 65, 62, 67, 69, 65, 70, 74, 59, 71, 62, 58, 75, 65, 63, 54, 70, 62, 60, 51, 55, 61, 64, 72, 62, 65, 68, 63, 52, 64, 50, 78, 56, 71, 76, 62, 68, 58, 67, 66, 53, 62, 65, 47, 59, 61, 74, 76, 60, 74, 61, 63, 74, 76, 65, 58, 67, 69, 60, 63, 78, 59, 56, 69, 69, 66, 65, 71, 63, 49, 68, 54, 65, 63, 65, 63, 64, 53, 57, 67, 72, 44, 45, 67, 73, 72, 65, 55, 65, 55, 64, 70, 59, 54, 77, 55, 52, 70, 65, 61, 69, 55, 68, 67, 62, 52, 63, 56, 61, 58, 58, 67, 46, 60, 71, 72, 58, 58, 53, 63, 69, 56, 64, 68, 64, 69, 49, 62, 67, 78, 52, 58, 70, 57, 60, 72, 55, 66, 62, 54, 49, 64, 68, 60, 64, 72, 56, 63, 64, 58, 48, 63, 58, 54, 66, 70, 57, 63, 57, 61, 47, 57, 68, 62, 60, 63, 57, 66, 70, 62, 59, 58, 48, 47, 61, 69, 61, 54, 50, 55, 71, 51, 58, 60, 60, 51, 72, 56, 72, 67, 62, 56, 53, 52, 62, 65, 63, 62, 66, 57, 63, 58, 68, 74, 57, 66, 63, 66, 60, 49, 60, 74, 49, 43, 56, 64, 48, 60, 42, 64, 81, 63, 62, 59, 50, 67, 63, 65, 65, 55, 49, 67, 57, 56, 64, 70, 53, 53, 61, 56, 56, 61, 64, 64, 59, 51, 63, 55, 57, 68, 41, 57, 58, 63, 55, 69, 53, 52, 62, 51, 65, 0, 0, 0, 0, 0, 0, 0, 0, 0, 0, 0, 0, 0, 0, 0, 0, 0, 0, 0, 0, 0, 0, 0, 0, 0, 0, 0, 0, 0, 0, 0, 0]
  in  "Lifetime settings":T4={"tac_range"=50.033573, "tac_gain"=4, "tac_offset"=6.0, "tac_limit_high"=97.0, "tac_limit_low"=3.0, "collect_time"=5.0, "sync_threshold"=-50.980392, "sync_zc_level"=-5.2913384, "sync_freq_div"=1, "cfd_limit_low"=-50.980392, "cfd_zc_level"=-5.2999988} {"sync_freq_div" items=["1"=1, "2"=2, "4"=4]; "cfd_zc_level" min=-96 max=96 step=0.1 format="%#_3g"; "cfd_limit_low" min=-500 max=0 step=0.1 format="%#_3g"; "sync_zc_level" min=-96 max=96 step=0.1 format="%#_3g"; "sync_threshold" min=-500 max=-20 step=0.1 format="%#_3g"; "tac_limit_low" format="%.3g"; "tac_limit_high" min=0 max=100 step=0.1 format="%.3g"; "collect_time" min=1e-07 max=100000 step=0.001; "tac_offset" min=0 max=100 step=0.1 format="%.4g"; "tac_gain" min=1 max=15 step=1; "tac_range" format="%^#_6g"}
  in  "Lifetime abort":bool
  out "Lifetime time remaining":sgl(knob) caption="Time Remaining" scale=0.0..30.000001907348633
  in  "Auto Saturation":bool
  in  "Measure saturation":bool
  out "All Detector Counts":dbl[][](graph)
  in  "Record counts":bool
  in  "Write stability to file":bool caption="Write to file"
  in  "Empty memory":bool
  in  "Saturation Start Angle":dbl=10.0
  in  "Saturation Sweep Speed (deg/s)":dbl=10.0
  in  "Saturation End Angle":dbl=210.0
  in  "Measure counts on PDMs?":bool=TRUE
  in  "Scan area override":bool
  in  "Autoscan Spectrum Time (s)":i32=30 min=10 max=240000000
  in  "lifetime window":bool
  in  "Stop Autoscan":bool
  in  "g2":bool
  in  "Spectrum":bool
  in  "Lifetime Auto Scan Settings":T4={"tac_range"=50.0, "tac_gain"=4, "tac_offset"=6.0, "tac_limit_high"=97.0, "tac_limit_low"=3.0, "collect_time"=5.0, "sync_threshold"=-51.0, "sync_zc_level"=-5.2913384, "sync_freq_div"=1, "cfd_limit_low"=-51.0, "cfd_zc_level"=-5.2999988} {"sync_freq_div" items=["1"=1, "2"=2, "4"=4]; "cfd_zc_level" min=-96 max=96 step=0.1 format="%#_3g"; "cfd_limit_low" min=-500 max=0 step=0.1 format="%#_3g"; "sync_zc_level" min=-96 max=96 step=0.1 format="%#_3g"; "sync_threshold" min=-500 max=-20 step=0.1 format="%#_3g"; "tac_limit_low" format="%.3g"; "tac_limit_high" min=0 max=100 step=0.1 format="%.3g"; "collect_time" min=1e-07 max=100000 step=0.001; "tac_offset" min=0 max=100 step=0.1 format="%.4g"; "tac_gain" min=1 max=15 step=1; "tac_range" format="%^#_6g"}
  in  "g2 Auto Scan Settings":T4={"tac_range"=50.0, "tac_gain"=1, "tac_offset"=6.0, "tac_limit_high"=97.0, "tac_limit_low"=3.0, "collect_time"=30.000002, "sync_threshold"=-51.0, "sync_zc_level"=-5.2913384, "sync_freq_div"=1, "cfd_limit_low"=-51.0, "cfd_zc_level"=-5.2999988} {"sync_freq_div" items=["1"=1, "2"=2, "4"=4]; "cfd_zc_level" min=-96 max=96 step=0.1 format="%#_3g"; "cfd_limit_low" min=-500 max=0 step=0.1 format="%#_3g"; "sync_zc_level" min=-96 max=96 step=0.1 format="%#_3g"; "sync_threshold" min=-500 max=-20 step=0.1 format="%#_3g"; "tac_limit_low" format="%.3g"; "tac_limit_high" min=0 max=100 step=0.1 format="%.3g"; "collect_time" min=1e-07 max=100000 step=0.001; "tac_offset" min=0 max=100 step=0.1 format="%.4g"; "tac_gain" min=1 max=15 step=1; "tac_range" format="%^#_6g"}
  in  "g2 window":bool=TRUE
  out "StabilityRMS":dbl=0.4585852277827532
  in  "Tracking":bool
  in  "Align Scan":bool
  in  "Z range":dbl=1.0
  in  "Z Mesh":dbl=0.003
  in  "ZX range":dbl=0.006
  in  "Z-velocity":dbl=0.5 format="%#_13g"
  in  "Z-frequency":dbl=0.5 format="%#_13g"
  in  "A-velocity":dbl=2.0 format="%#_13g"
  in  "A-frequency":dbl=2.0 format="%#_13g"
  in  "Emitter #":i32
  in  "Next emitter":bool
  in  "Align XY range":dbl=1.0
  in  "Align XY Mesh":dbl=0.01
  in  "EMITTER RUNTHROUGH":bool
  out "# of Emitters":i32=47
  out "Area #":i16=5050
  in  "AUTO XY SCAN":bool
  in  "RMS Cutoff":dbl=10000.0
  in  "Fine Align":bool
  out "Autoscan Status":string
  in  "Upper Counts Theshold":dbl=8000000.0
  in  "Lower Counts Threshold":dbl=40000.0
  in  "Autoscan Stability Time (s)":dbl=10.0 caption="Delay Time (s)"
  in  "Lifetime":bool
  in  "Saturation":bool
  in  "GetNewLoc":bool
  in  "Lower contrast threshold":dbl=0.2
  in  "Correct map":bool=TRUE
  in  "Correction type":i16(slide) scale=0.0..1.0
  in  "Upper contrast threshold":dbl=1000000.0
  in  "Write Alignment map to file":bool
  in  "Map Switch":bool=TRUE
  in  "Draw emitters":bool
  in  "Help me find emitters!":bool=TRUE
  in  "Pick candidates":bool
  in  "Laser Shutter":bool
  in  "Correlation measurement":T5 items=["Lifetime (80 MHz, 12.5 ns)", "Lifetime (20 MHz, 50 ns)", "g2 (50 ns)", "g2 (300 ns)"]
  in  "Multiplier":dbl=3.2
  out "Laser power (uW)":dbl=0.32650840600000003 format="%#_5g"
  out "PDM2 counts":i32=730
  out "SPCM trace":dbl(graph)
  out "PDM1 trace":dbl(graph)=20.0
  out "PDM2 trace":dbl(graph)
  in  "Y-velocity":dbl=1.0 format="%#_13g"
  in  "X-frequency":dbl=1.0 format="%#_13g"
  in  "Buffering":bool
  in  "Clear emitters":bool
  in  "PL scan contrast limits":dbl[](array[numeric])=[0.0, 0.001]
  in  "Write PL map to file":bool
  in  "down":bool
  in  "up":bool
  in  "north":bool
  in  "south":bool
  in  "west":bool
  in  "east":bool
  out "Intensity":dbl=52.84858823
  in  "Y Range":dbl=10.0
  in  "XY Scan":bool
  in  "Y Center":dbl=50.0 format="%.3g"
  in  "X Center":dbl=50.0 format="%.3g"
  in  "Abs. Move":bool
  in  "Z":dbl=50.00135028 format="%.3g"
  in  "Y":dbl=49.98837873 format="%.3g"
  in  "X":dbl=50.00616648 format="%.3g"
  out "Position":dbl[](array[numeric])=[49.99295798, 49.99961646, 48.40159384] format="%.6f"
  out "Motion":bool=TRUE
  in  "X Range":dbl=10.0
  out "Intensity Graph":dbl[][](graph)
  in  "Mesh":dbl=0.2
  in  "stop":bool
  out "PDM1 counts":i32=20
  out "SPCM counts":i32
  in  "PDM 2 on/off":bool=TRUE
  in  "PDM 1 on/off":bool=TRUE
  in  "Clear auto spectra positions":bool
  in  "Filter Positions":dbl[](array[numeric])
  in  "Measurement Save Path":path
  in  "Filename Note":string
  out "User Selected Measurement Points":dbl[][](array[numeric])
  out "Current Angle":sgl
  in  "Set power":bool
  in  "Move to":dbl
  out "Filter wheel position":i32
  out "Resource Name":string
  out "Serial Number":string
  out "Laser Pwr Save Var":dbl
  in  "Default 70x70um scan":dbl[][](array[numeric])=[[50.0, 50.0], [50.0, 40.0], [60.0, 40.0], [60.0, 50.0], [60.0, 60.0], [50.0, 60.0], [40.0, 60.0], [40.0, 50.0], [40.0, 40.0], [40.0, 30.0], [50.0, 30.0], [60.0, 30.0], [70.0, 30.0], [70.0, 40.0], [70.0, 50.0], [70.0, 60.0], [70.0, 70.0], [60.0, 70.0], [50.0, 70.0], [40.0, 70.0], [30.0, 70.0], [30.0, 60.0], [30.0, 50.0], [30.0, 40.0], [30.0, 30.0], [30.0, 20.0], [40.0, 20.0], [50.0, 20.0], [60.0, 20.0], [70.0, 20.0], [80.0, 20.0], [80.0, 30.0], [80.0, 40.0], [80.0, 50.0], [80.0, 60.0], [80.0, 70.0], [80.0, 80.0], [70.0, 80.0], [60.0, 80.0], [50.0, 80.0], [40.0, 80.0], [30.0, 80.0], [20.0, 80.0]]
  out "cent":i32[][](array[numeric])=[[193, 6], [84, 9], [125, 13], [137, 17], [32, 22], [163, 22], [123, 25], [36, 29], [14, 30], [119, 40], [32, 41], [132, 54], [8, 55], [33, 57], [191, 57], [139, 59], [88, 73], [36, 80], [26, 83], [115, 85], [177, 89], [22, 90], [141, 105], [132, 109], [161, 109], [180, 116], [39, 125], [63, 126], [153, 129], [173, 129], [26, 136], [162, 136], [73, 139], [134, 140], [127, 153], [96, 155], [145, 155], [79, 157], [29, 163], [96, 164], [50, 166], [119, 169], [150, 176], [22, 184], [182, 185], [189, 188], [75, 190]]
  out "deleted portion":dbl[](array[numeric])
  out "Buffered MapCorr":dbl[][](array[numeric])
  out "Current MapCorr":dbl[][](array[numeric])
  out "Buffered Map":dbl[][](array[numeric])=[[0.40084199999999726, 0.0009999999999976694, 0.0009999999999976694, 0.0009999999999976694, 0.0009999999999976694, 0.0009999999999976694, 0.0009999999999976694, 0.0009999999999976694, 0.0009999999999976694, 0.0009999999999976694, 0.0009999999999976694, 0.0009999999999976694, 0.0009999999999976694, 0.0009999999999976694, 0.0009999999999976694, 0.0009999999999976694, 0.0009999999999976694, 0.0009999999999976694, 0.0009999999999976694, 0.0009999999999976694, 0.0009999999999976694, 0.0009999999999976694, 0.0009999999999976694, 0.0009999999999976694, 0.0009999999999976694, 0.0009999999999976694, 0.0009999999999976694, 0.0009999999999976694, 0.0009999999999976694, 0.0009999999999976694, 0.0009999999999976694, 0.0009999999999976694, 0.0009999999999976694, 0.0009999999999976694, 0.0009999999999976694, 0.0009999999999976694, 0.0009999999999976694, 0.0009999999999976694, 0.0009999999999976694, 0.0009999999999976694, 0.0009999999999976694, 0.0009999999999976694, 0.0009999999999976694, 0.0009999999999976694, 0.0009999999999976694, 0.0009999999999976694, 0.0009999999999976694, 0.0009999999999976694, 0.0009999999999976694, 0.0009999999999976694, 0.0009999999999976694, 0.0009999999999976694, 0.0009999999999976694, 0.0009999999999976694, 0.0009999999999976694, 0.0009999999999976694, 0.0009999999999976694, 0.0009999999999976694, 0.0009999999999976694, 0.0009999999999976694, 0.0009999999999976694, 0.0009999999999976694, 0.0009999999999976694, 0.0009999999999976694, 0.0009999999999976694, 0.0009999999999976694, 0.0009999999999976694, 0.0009999999999976694, 0.0009999999999976694, 0.0009999999999976694, 0.0009999999999976694, 0.0009999999999976694, 0.0009999999999976694, 0.0009999999999976694, 0.0009999999999976694, 0.0009999999999976694, 0.0009999999999976694, 0.0009999999999976694, 0.0009999999999976694, 0.0009999999999976694, 0.0009999999999976694, 0.0009999999999976694, 0.0009999999999976694, 0.0009999999999976694, 0.0009999999999976694, 0.0009999999999976694, 0.0009999999999976694, 0.0009999999999976694, 0.0009999999999976694, 0.0009999999999976694, 0.0009999999999976694, 0.0009999999999976694, 0.0009999999999976694, 0.0009999999999976694, 0.0009999999999976694, 0.0009999999999976694, 0.0009999999999976694, 0.0009999999999976694, 0.0009999999999976694, 0.0009999999999976694], [0.39584799999999376, 0.0009999999999976694, 0.0009999999999976694, 0.0009999999999976694, 0.0009999999999976694, 0.0009999999999976694, 0.0009999999999976694, 0.0009999999999976694, 0.0009999999999976694, 0.0009999999999976694, 0.0009999999999976694, 0.0009999999999976694, 0.0009999999999976694, 0.0009999999999976694, 0.0009999999999976694, 0.0009999999999976694, 0.0009999999999976694, 0.0009999999999976694, 0.0009999999999976694, 0.0009999999999976694, 0.0009999999999976694, 0.0009999999999976694, 0.0009999999999976694, 0.0009999999999976694, 0.0009999999999976694, 0.0009999999999976694, 0.0009999999999976694, 0.0009999999999976694, 0.0009999999999976694, 0.0009999999999976694, 0.0009999999999976694, 0.0009999999999976694, 0.0009999999999976694, 0.0009999999999976694, 0.0009999999999976694, 0.0009999999999976694, 0.0009999999999976694, 0.0009999999999976694, 0.0009999999999976694, 0.0009999999999976694, 0.0009999999999976694, 0.0009999999999976694, 0.0009999999999976694, 0.0009999999999976694, 0.0009999999999976694, 0.0009999999999976694, 0.0009999999999976694, 0.0009999999999976694, 0.0009999999999976694, 0.0009999999999976694, 0.0009999999999976694, 0.0009999999999976694, 0.0009999999999976694, 0.0009999999999976694, 0.0009999999999976694, 0.0009999999999976694, 0.0009999999999976694, 0.0009999999999976694, 0.0009999999999976694, 0.0009999999999976694, 0.0009999999999976694, 0.0009999999999976694, 0.0009999999999976694, 0.0009999999999976694, 0.0009999999999976694, 0.0009999999999976694, 0.0009999999999976694, 0.0009999999999976694, 0.0009999999999976694, 0.0009999999999976694, 0.0009999999999976694, 0.0009999999999976694, 0.0009999999999976694, 0.0009999999999976694, 0.0009999999999976694, 0.0009999999999976694, 0.0009999999999976694, 0.0009999999999976694, 0.0009999999999976694, 0.0009999999999976694, 0.0009999999999976694, 0.0009999999999976694, 0.0009999999999976694, 0.0009999999999976694, 0.0009999999999976694, 0.0009999999999976694, 0.0009999999999976694, 0.0009999999999976694, 0.0009999999999976694, 0.0009999999999976694, 0.0009999999999976694, 0.0009999999999976694, 0.0009999999999976694, 0.0009999999999976694, 0.0009999999999976694, 0.0009999999999976694, 0.0009999999999976694, 0.0009999999999976694, 0.0009999999999976694, 0.0009999999999976694], [0.3941149999999993, 0.0009999999999976694, 0.0009999999999976694, 0.0009999999999976694, 0.0009999999999976694, 0.0009999999999976694, 0.0009999999999976694, 0.0009999999999976694, 0.0009999999999976694, 0.0009999999999976694, 0.0009999999999976694, 0.0009999999999976694, 0.0009999999999976694, 0.0009999999999976694, 0.0009999999999976694, 0.0009999999999976694, 0.0009999999999976694, 0.0009999999999976694, 0.0009999999999976694, 0.0009999999999976694, 0.0009999999999976694, 0.0009999999999976694, 0.0009999999999976694, 0.0009999999999976694, 0.0009999999999976694, 0.0009999999999976694, 0.0009999999999976694, 0.0009999999999976694, 0.0009999999999976694, 0.0009999999999976694, 0.0009999999999976694, 0.0009999999999976694, 0.0009999999999976694, 0.0009999999999976694, 0.0009999999999976694, 0.0009999999999976694, 0.0009999999999976694, 0.0009999999999976694, 0.0009999999999976694, 0.0009999999999976694, 0.0009999999999976694, 0.0009999999999976694, 0.0009999999999976694, 0.0009999999999976694, 0.0009999999999976694, 0.0009999999999976694, 0.0009999999999976694, 0.0009999999999976694, 0.0009999999999976694, 0.0009999999999976694, 0.0009999999999976694, 0.0009999999999976694, 0.0009999999999976694, 0.0009999999999976694, 0.0009999999999976694, 0.0009999999999976694, 0.0009999999999976694, 0.0009999999999976694, 0.0009999999999976694, 0.0009999999999976694, 0.0009999999999976694, 0.0009999999999976694, 0.0009999999999976694, 0.0009999999999976694, 0.0009999999999976694, 0.0009999999999976694, 0.0009999999999976694, 0.0009999999999976694, 0.0009999999999976694, 0.0009999999999976694, 0.0009999999999976694, 0.0009999999999976694, 0.0009999999999976694, 0.0009999999999976694, 0.0009999999999976694, 0.0009999999999976694, 0.0009999999999976694, 0.0009999999999976694, 0.0009999999999976694, 0.0009999999999976694, 0.0009999999999976694, 0.0009999999999976694, 0.0009999999999976694, 0.0009999999999976694, 0.0009999999999976694, 0.0009999999999976694, 0.0009999999999976694, 0.0009999999999976694, 0.0009999999999976694, 0.0009999999999976694, 0.0009999999999976694, 0.0009999999999976694, 0.0009999999999976694, 0.0009999999999976694, 0.0009999999999976694, 0.0009999999999976694, 0.0009999999999976694, 0.0009999999999976694, 0.0009999999999976694, 0.0009999999999976694], [0.40012899999999973, 0.0009999999999976694, 0.0009999999999976694, 0.0009999999999976694, 0.0009999999999976694, 0.0009999999999976694, 0.0009999999999976694, 0.0009999999999976694, 0.0009999999999976694, 0.0009999999999976694, 0.0009999999999976694, 0.0009999999999976694, 0.0009999999999976694, 0.0009999999999976694, 0.0009999999999976694, 0.0009999999999976694, 0.0009999999999976694, 0.0009999999999976694, 0.0009999999999976694, 0.0009999999999976694, 0.0009999999999976694, 0.0009999999999976694, 0.0009999999999976694, 0.0009999999999976694, 0.0009999999999976694, 0.0009999999999976694, 0.0009999999999976694, 0.0009999999999976694, 0.0009999999999976694, 0.0009999999999976694, 0.0009999999999976694, 0.0009999999999976694, 0.0009999999999976694, 0.0009999999999976694, 0.0009999999999976694, 0.0009999999999976694, 0.0009999999999976694, 0.0009999999999976694, 0.0009999999999976694, 0.0009999999999976694, 0.0009999999999976694, 0.0009999999999976694, 0.0009999999999976694, 0.0009999999999976694, 0.0009999999999976694, 0.0009999999999976694, 0.0009999999999976694, 0.0009999999999976694, 0.0009999999999976694, 0.0009999999999976694, 0.0009999999999976694, 0.0009999999999976694, 0.0009999999999976694, 0.0009999999999976694, 0.0009999999999976694, 0.0009999999999976694, 0.0009999999999976694, 0.0009999999999976694, 0.0009999999999976694, 0.0009999999999976694, 0.0009999999999976694, 0.0009999999999976694, 0.0009999999999976694, 0.0009999999999976694, 0.0009999999999976694, 0.0009999999999976694, 0.0009999999999976694, 0.0009999999999976694, 0.0009999999999976694, 0.0009999999999976694, 0.0009999999999976694, 0.0009999999999976694, 0.0009999999999976694, 0.0009999999999976694, 0.0009999999999976694, 0.0009999999999976694, 0.0009999999999976694, 0.0009999999999976694, 0.0009999999999976694, 0.0009999999999976694, 0.0009999999999976694, 0.0009999999999976694, 0.0009999999999976694, 0.0009999999999976694, 0.0009999999999976694, 0.0009999999999976694, 0.0009999999999976694, 0.0009999999999976694, 0.0009999999999976694, 0.0009999999999976694, 0.0009999999999976694, 0.0009999999999976694, 0.0009999999999976694, 0.0009999999999976694, 0.0009999999999976694, 0.0009999999999976694, 0.0009999999999976694, 0.0009999999999976694, 0.0009999999999976694, 0.0009999999999976694], [0.38820399999999466, 0.0009999999999976694, 0.0009999999999976694, 0.0009999999999976694, 0.0009999999999976694, 0.0009999999999976694, 0.0009999999999976694, 0.0009999999999976694, 0.0009999999999976694, 0.0009999999999976694, 0.0009999999999976694, 0.0009999999999976694, 0.0009999999999976694, 0.0009999999999976694, 0.0009999999999976694, 0.0009999999999976694, 0.0009999999999976694, 0.0009999999999976694, 0.0009999999999976694, 0.0009999999999976694, 0.0009999999999976694, 0.0009999999999976694, 0.0009999999999976694, 0.0009999999999976694, 0.0009999999999976694, 0.0009999999999976694, 0.0009999999999976694, 0.0009999999999976694, 0.0009999999999976694, 0.0009999999999976694, 0.0009999999999976694, 0.0009999999999976694, 0.0009999999999976694, 0.0009999999999976694, 0.0009999999999976694, 0.0009999999999976694, 0.0009999999999976694, 0.0009999999999976694, 0.0009999999999976694, 0.0009999999999976694, 0.0009999999999976694, 0.0009999999999976694, 0.0009999999999976694, 0.0009999999999976694, 0.0009999999999976694, 0.0009999999999976694, 0.0009999999999976694, 0.0009999999999976694, 0.0009999999999976694, 0.0009999999999976694, 0.0009999999999976694, 0.0009999999999976694, 0.0009999999999976694, 0.0009999999999976694, 0.0009999999999976694, 0.0009999999999976694, 0.0009999999999976694, 0.0009999999999976694, 0.0009999999999976694, 0.0009999999999976694, 0.0009999999999976694, 0.0009999999999976694, 0.0009999999999976694, 0.0009999999999976694, 0.0009999999999976694, 0.0009999999999976694, 0.0009999999999976694, 0.0009999999999976694, 0.0009999999999976694, 0.0009999999999976694, 0.0009999999999976694, 0.0009999999999976694, 0.0009999999999976694, 0.0009999999999976694, 0.0009999999999976694, 0.0009999999999976694, 0.0009999999999976694, 0.0009999999999976694, 0.0009999999999976694, 0.0009999999999976694, 0.0009999999999976694, 0.0009999999999976694, 0.0009999999999976694, 0.0009999999999976694, 0.0009999999999976694, 0.0009999999999976694, 0.0009999999999976694, 0.0009999999999976694, 0.0009999999999976694, 0.0009999999999976694, 0.0009999999999976694, 0.0009999999999976694, 0.0009999999999976694, 0.0009999999999976694, 0.0009999999999976694, 0.0009999999999976694, 0.0009999999999976694, 0.0009999999999976694, 0.0009999999999976694, 0.0009999999999976694], [0.3995169999999959, 0.0009999999999976694, 0.0009999999999976694, 0.0009999999999976694, 0.0009999999999976694, 0.0009999999999976694, 0.0009999999999976694, 0.0009999999999976694, 0.0009999999999976694, 0.0009999999999976694, 0.0009999999999976694, 0.0009999999999976694, 0.0009999999999976694, 0.0009999999999976694, 0.0009999999999976694, 0.0009999999999976694, 0.0009999999999976694, 0.0009999999999976694, 0.0009999999999976694, 0.0009999999999976694, 0.0009999999999976694, 0.0009999999999976694, 0.0009999999999976694, 0.0009999999999976694, 0.0009999999999976694, 0.0009999999999976694, 0.0009999999999976694, 0.0009999999999976694, 0.0009999999999976694, 0.0009999999999976694, 0.0009999999999976694, 0.0009999999999976694, 0.0009999999999976694, 0.0009999999999976694, 0.0009999999999976694, 0.0009999999999976694, 0.0009999999999976694, 0.0009999999999976694, 0.0009999999999976694, 0.0009999999999976694, 0.0009999999999976694, 0.0009999999999976694, 0.0009999999999976694, 0.0009999999999976694, 0.0009999999999976694, 0.0009999999999976694, 0.0009999999999976694, 0.0009999999999976694, 0.0009999999999976694, 0.0009999999999976694, 0.0009999999999976694, 0.0009999999999976694, 0.0009999999999976694, 0.0009999999999976694, 0.0009999999999976694, 0.0009999999999976694, 0.0009999999999976694, 0.0009999999999976694, 0.0009999999999976694, 0.0009999999999976694, 0.0009999999999976694, 0.0009999999999976694, 0.0009999999999976694, 0.0009999999999976694, 0.0009999999999976694, 0.0009999999999976694, 0.0009999999999976694, 0.0009999999999976694, 0.0009999999999976694, 0.0009999999999976694, 0.0009999999999976694, 0.0009999999999976694, 0.0009999999999976694, 0.0009999999999976694, 0.0009999999999976694, 0.0009999999999976694, 0.0009999999999976694, 0.0009999999999976694, 0.0009999999999976694, 0.0009999999999976694, 0.0009999999999976694, 0.0009999999999976694, 0.0009999999999976694, 0.0009999999999976694, 0.0009999999999976694, 0.0009999999999976694, 0.0009999999999976694, 0.0009999999999976694, 0.0009999999999976694, 0.0009999999999976694, 0.0009999999999976694, 0.0009999999999976694, 0.0009999999999976694, 0.0009999999999976694, 0.0009999999999976694, 0.0009999999999976694, 0.0009999999999976694, 0.0009999999999976694, 0.0009999999999976694, 0.0009999999999976694], [0.3968670000000003, 0.39177099999999854, 0.0009999999999976694, 0.0009999999999976694, 0.0009999999999976694, 0.0009999999999976694, 0.0009999999999976694, 0.0009999999999976694, 0.0009999999999976694, 0.3975809999999953, 0.3952369999999945, 0.0009999999999976694, 0.0009999999999976694, 0.40002699999999436, 0.0009999999999976694, 0.0009999999999976694, 0.0009999999999976694, 0.397987999999998, 0.0009999999999976694, 0.0009999999999976694, 0.0009999999999976694, 0.0009999999999976694, 0.38147699999999674, 0.0009999999999976694, 0.0009999999999976694, 0.4033899999999946, 0.0009999999999976694, 0.0009999999999976694, 0.0009999999999976694, 0.0009999999999976694, 0.4291759999999982, 0.0009999999999976694, 0.0009999999999976694, 0.0009999999999976694, 0.0009999999999976694, 0.0009999999999976694, 0.3899369999999962, 0.40237099999999515, 0.0009999999999976694, 0.0009999999999976694, 0.392280999999997, 0.40349199999999996, 0.0009999999999976694, 0.0009999999999976694, 0.0009999999999976694, 0.0009999999999976694, 0.40614199999999556, 0.0009999999999976694, 0.4003329999999963, 0.3972750000000005, 0.0009999999999976694, 0.0009999999999976694, 0.0009999999999976694, 0.0009999999999976694, 0.0009999999999976694, 0.0009999999999976694, 0.3952369999999945, 0.39747899999999703, 0.0009999999999976694, 0.0009999999999976694, 0.0009999999999976694, 0.3926889999999972, 0.0009999999999976694, 0.0009999999999976694, 0.40053599999999534, 0.39972099999999955, 0.0009999999999976694, 0.0009999999999976694, 0.40002699999999436, 0.0009999999999976694, 0.0009999999999976694, 0.3983959999999982, 0.39941499999999763, 0.39859999999999474, 0.0009999999999976694, 0.0009999999999976694, 0.0009999999999976694, 0.0009999999999976694, 0.0009999999999976694, 0.3956439999999972, 0.0009999999999976694, 0.0009999999999976694, 0.0009999999999976694, 0.3983959999999982, 0.3967649999999949, 0.0009999999999976694, 0.3963579999999993, 0.39737699999999876, 0.0009999999999976694, 0.0009999999999976694, 0.0009999999999976694, 0.39788599999999974, 0.0009999999999976694, 0.0009999999999976694, 0.0009999999999976694, 0.0009999999999976694, 0.0009999999999976694, 0.0009999999999976694, 0.3938099999999949, 0.3968670000000003], [0.3952369999999945, 0.3948289999999943, 0.400739999999999, 0.39788599999999974, 0.39747899999999703, 0.39737699999999876, 0.3960519999999974, 0.39513499999999624, 0.39289199999999624, 0.39819199999999455, 0.39707099999999684, 0.39707099999999684, 0.4030839999999998, 0.3982939999999999, 0.4028809999999936, 0.3988039999999984, 0.4057339999999954, 0.3990079999999949, 0.40685599999999766, 0.39788599999999974, 0.400230999999998, 0.40206500000000034, 0.3948289999999943, 0.39554199999999895, 0.40124999999999744, 0.39625599999999395, 0.3968670000000003, 0.3999249999999961, 0.3915669999999949, 0.39972099999999955, 0.3956439999999972, 0.39319799999999816, 0.39859999999999474, 0.39442099999999414, 0.40043399999999707, 0.4030839999999998, 0.3956439999999972, 0.3938099999999949, 0.3929939999999945, 0.42071699999999623, 0.40767100000000056, 0.39890599999999665, 0.36843099999999396, 0.409403999999995, 0.3988039999999984, 0.3960519999999974, 0.3948289999999943, 0.400739999999999, 0.3957459999999955, 0.400739999999999, 0.397987999999998, 0.3957459999999955, 0.3961539999999957, 0.39747899999999703, 0.3969689999999986, 0.3980899999999963, 0.3967649999999949, 0.40012899999999973, 0.3945229999999995, 0.3961539999999957, 0.4021669999999986, 0.3983959999999982, 0.39890599999999665, 0.39594999999999914, 0.4033899999999946, 0.40012899999999973, 0.404408999999994, 0.3967649999999949, 0.389528999999996, 0.401453999999994, 0.39737699999999876, 0.3995169999999959, 0.3967649999999949, 0.3987020000000001, 0.4003329999999963, 0.3960519999999974, 0.3998229999999978, 0.39788599999999974, 0.39656199999999586, 0.39849799999999647, 0.39972099999999955, 0.3868790000000004, 0.39177099999999854, 0.39656199999999586, 0.3954400000000007, 0.3910579999999939, 0.4017589999999984, 0.38259799999999444, 0.400739999999999, 0.4032879999999963, 0.41154399999999924, 0.39890599999999665, 0.3990079999999949, 0.39890599999999665, 0.4025749999999988, 0.3972750000000005, 0.39554199999999895, 0.3976830000000007, 0.39707099999999684, 0.40155599999999936], [0.40053599999999534, 0.4055309999999963, 0.4009439999999955, 0.3998229999999978, 0.40084199999999726, 0.40532699999999977, 0.39584799999999376, 0.41235899999999504, 0.400739999999999, 0.3960519999999974, 0.3919749999999951, 0.39788599999999974, 0.3949309999999997, 0.4074669999999969, 0.4067539999999994, 0.3960519999999974, 0.3972750000000005, 0.39819199999999455, 0.39778499999999894, 0.3945229999999995, 0.4090980000000002, 0.3996189999999942, 0.40695699999999846, 0.40349199999999996, 0.40165799999999763, 0.40155599999999936, 0.3975809999999953, 0.39849799999999647, 0.39442099999999414, 0.40797699999999537, 0.40767100000000056, 0.39737699999999876, 0.39778499999999894, 0.39289199999999624, 0.399210999999994, 0.39207700000000045, 0.39360599999999835, 0.3982939999999999, 0.3980899999999963, 0.3972750000000005, 0.39666299999999666, 0.3925869999999989, 0.39707099999999684, 0.39391200000000026, 0.3976830000000007, 0.3971729999999951, 0.39747899999999703, 0.4033899999999946, 0.3982939999999999, 0.39941499999999763, 0.4345779999999948, 0.3929939999999945, 0.39972099999999955, 0.3972750000000005, 0.3871849999999952, 0.40532699999999977, 0.39584799999999376, 0.4307049999999961, 0.39707099999999684, 0.4048169999999942, 0.397987999999998, 0.39747899999999703, 0.39513499999999624, 0.39747899999999703, 0.39788599999999974, 0.40685599999999766, 0.39503299999999797, 0.3957459999999955, 0.4018609999999967, 0.3918729999999968, 0.39207700000000045, 0.4075689999999952, 0.3998229999999978, 0.4045109999999994, 0.38789799999999985, 0.39401299999999395, 0.39859999999999474, 0.4075689999999952, 0.3968670000000003, 0.3999249999999961, 0.3953379999999953, 0.39594999999999914, 0.399210999999994, 0.3892229999999941, 0.401453999999994, 0.40124999999999744, 0.3952369999999945, 0.3948289999999943, 0.3925869999999989, 0.3996189999999942, 0.3967649999999949, 0.39941499999999763, 0.4057339999999954, 0.40614199999999556, 0.3899369999999962, 0.41184999999999405, 0.3996189999999942, 0.39747899999999703, 0.400230999999998, 0.43518899999999405], [0.3892229999999941, 0.40349199999999996, 0.3988039999999984, 0.40624399999999383, 0.39431899999999587, 0.39666299999999666, 0.39319799999999816, 0.39126199999999756, 0.39319799999999816, 0.401453999999994, 0.39931299999999936, 0.3969689999999986, 0.39931299999999936, 0.3960519999999974, 0.3954400000000007, 0.4052249999999944, 0.3960519999999974, 0.400739999999999, 0.39890599999999665, 0.397987999999998, 0.4003329999999963, 0.392280999999997, 0.40624399999999383, 0.399210999999994, 0.3948289999999943, 0.40002699999999436, 0.3949309999999997, 0.39941499999999763, 0.40155599999999936, 0.3960519999999974, 0.3995169999999959, 0.43202999999999747, 0.39584799999999376, 0.3964599999999976, 0.4009439999999955, 0.3967649999999949, 0.39431899999999587, 0.39972099999999955, 0.4013519999999957, 0.40124999999999744, 0.4009439999999955, 0.3941149999999993, 0.39584799999999376, 0.40043399999999707, 0.4083839999999981, 0.3999249999999961, 0.39656199999999586, 0.4009439999999955, 0.40532699999999977, 0.39778499999999894, 0.39747899999999703, 0.4048169999999942, 0.39513499999999624, 0.39941499999999763, 0.39207700000000045, 0.3915669999999949, 0.409912999999996, 0.3935040000000001, 0.4033899999999946, 0.401453999999994, 0.40165799999999763, 0.3914649999999966, 0.3781139999999965, 0.3982939999999999, 0.3991100000000003, 0.40043399999999707, 0.3896309999999943, 0.39656199999999586, 0.40053599999999534, 0.3963579999999993, 0.39472699999999605, 0.3980899999999963, 0.3942169999999976, 0.4040019999999984, 0.4010459999999938, 0.39666299999999666, 0.3903439999999989, 0.40155599999999936, 0.4006379999999936, 0.4017589999999984, 0.39737699999999876, 0.4036959999999965, 0.3982939999999999, 0.4017589999999984, 0.3952369999999945, 0.40542899999999804, 0.3988039999999984, 0.40206500000000034, 0.40379799999999477, 0.3911599999999993, 0.39778499999999894, 0.3971729999999951, 0.39737699999999876, 0.3998229999999978, 0.4052249999999944, 0.3946249999999978, 0.3999249999999961, 0.41032099999999616, 0.41235899999999504, 0.39238299999999526], [0.40155599999999936, 0.3960519999999974, 0.39788599999999974, 0.4028809999999936, 0.39737699999999876, 0.3996189999999942, 0.40542899999999804, 0.4402860000000004, 0.3956439999999972, 0.4154169999999979, 0.39890599999999665, 0.3963579999999993, 0.37444499999999437, 0.40390000000000015, 0.39737699999999876, 0.39503299999999797, 0.4049189999999996, 0.39442099999999414, 0.39849799999999647, 0.39656199999999586, 0.40277899999999534, 0.39849799999999647, 0.4010459999999938, 0.38973299999999966, 0.3964599999999976, 0.3961539999999957, 0.3969689999999986, 0.39584799999999376, 0.40359399999999823, 0.39656199999999586, 0.40797699999999537, 0.40053599999999534, 0.39849799999999647, 0.3972750000000005, 0.38942699999999775, 0.3983959999999982, 0.3884079999999983, 0.3960519999999974, 0.3963579999999993, 0.4009439999999955, 0.3991100000000003, 0.39554199999999895, 0.39747899999999703, 0.3946249999999978, 0.3960519999999974, 0.39890599999999665, 0.4018609999999967, 0.3969689999999986, 0.3971729999999951, 0.4021669999999986, 0.3975809999999953, 0.3926889999999972, 0.39085399999999737, 0.38983499999999793, 0.39177099999999854, 0.39513499999999624, 0.3956439999999972, 0.39554199999999895, 0.40012899999999973, 0.40542899999999804, 0.40084199999999726, 0.39360599999999835, 0.4125629999999987, 0.3960519999999974, 0.39329999999999643, 0.3929939999999945, 0.39941499999999763, 0.3957459999999955, 0.399210999999994, 0.39625599999999395, 0.3957459999999955, 0.3949309999999997, 0.3948289999999943, 0.4116459999999975, 0.40012899999999973, 0.39238299999999526, 0.39707099999999684, 0.39778499999999894, 0.392280999999997, 0.397987999999998, 0.3930959999999999, 0.40084199999999726, 0.40919999999999845, 0.3919749999999951, 0.3915669999999949, 0.3913639999999958, 0.4010459999999938, 0.40114799999999917, 0.392280999999997, 0.3914649999999966, 0.4139899999999983, 0.392280999999997, 0.3971729999999951, 0.3967649999999949, 0.4032879999999963, 0.3968670000000003, 0.40053599999999534, 0.3956439999999972, 0.3957459999999955, 0.3942169999999976], [0.39584799999999376, 0.39360599999999835, 0.40124999999999744, 0.39656199999999586, 0.3975809999999953, 0.39747899999999703, 0.3935040000000001, 0.3899369999999962, 0.39666299999999666, 0.3953379999999953, 0.39737699999999876, 0.3877959999999945, 0.3888159999999985, 0.392280999999997, 0.3988039999999984, 0.40277899999999534, 0.4025749999999988, 0.4074669999999969, 0.397987999999998, 0.39594999999999914, 0.39554199999999895, 0.37954099999999613, 0.3998229999999978, 0.39391200000000026, 0.3988039999999984, 0.39788599999999974, 0.40277899999999534, 0.3956439999999972, 0.40277899999999534, 0.4006379999999936, 0.3957459999999955, 0.3942169999999976, 0.4021669999999986, 0.3896309999999943, 0.39931299999999936, 0.40430699999999575, 0.39656199999999586, 0.4013519999999957, 0.3975809999999953, 0.39941499999999763, 0.3906499999999937, 0.3957459999999955, 0.397987999999998, 0.3869809999999987, 0.3968670000000003, 0.40124999999999744, 0.39472699999999605, 0.39859999999999474, 0.39054799999999545, 0.39931299999999936, 0.39625599999999395, 0.39747899999999703, 0.39819199999999455, 0.3941149999999993, 0.4067539999999994, 0.4036959999999965, 0.3968670000000003, 0.3995169999999959, 0.38647100000000023, 0.4009439999999955, 0.39329999999999643, 0.39126199999999756, 0.3996189999999942, 0.41307299999999714, 0.3988039999999984, 0.39513499999999624, 0.39177099999999854, 0.399210999999994, 0.3980899999999963, 0.39401299999999395, 0.3980899999999963, 0.4025749999999988, 0.400230999999998, 0.40053599999999534, 0.3991100000000003, 0.3896309999999943, 0.3990079999999949, 0.40084199999999726, 0.3983959999999982, 0.399210999999994, 0.3942169999999976, 0.3964599999999976, 0.3963579999999993, 0.4040019999999984, 0.40318599999999805, 0.4018609999999967, 0.3961539999999957, 0.4006379999999936, 0.3982939999999999, 0.3926889999999972, 0.3968670000000003, 0.40053599999999534, 0.3900389999999945, 0.3949309999999997, 0.3968670000000003, 0.3980899999999963, 0.39625599999999395, 0.3937079999999966, 0.39859999999999474, 0.38749099999999714], [0.3964599999999976, 0.3982939999999999, 0.39594999999999914, 0.39442099999999414, 0.41562099999999447, 0.4030839999999998, 0.39819199999999455, 0.3987020000000001, 0.39289199999999624, 0.41643599999999736, 0.3967649999999949, 0.399210999999994, 0.4040019999999984, 0.3824959999999962, 0.3998229999999978, 0.3980899999999963, 0.399210999999994, 0.3835160000000002, 0.4055309999999963, 0.4006379999999936, 0.3980899999999963, 0.3969689999999986, 0.4022689999999969, 0.3957459999999955, 0.3876939999999962, 0.397987999999998, 0.3961539999999957, 0.3914649999999966, 0.4049189999999996, 0.40084199999999726, 0.40002699999999436, 0.39778499999999894, 0.39625599999999395, 0.400230999999998, 0.40084199999999726, 0.3980899999999963, 0.3987020000000001, 0.39013999999999527, 0.3904459999999972, 0.3969689999999986, 0.39166900000000027, 0.39788599999999974, 0.39819199999999455, 0.3971729999999951, 0.39859999999999474, 0.3904459999999972, 0.3949309999999997, 0.400230999999998, 0.4010459999999938, 0.40084199999999726, 0.39737699999999876, 0.40817999999999444, 0.3996189999999942, 0.4022689999999969, 0.39625599999999395, 0.3935040000000001, 0.3996189999999942, 0.3980899999999963, 0.39431899999999587, 0.3972750000000005, 0.39972099999999955, 0.40124999999999744, 0.3913639999999958, 0.4083839999999981, 0.39085399999999737, 0.4060399999999973, 0.39472699999999605, 0.3967649999999949, 0.40206500000000034, 0.40705899999999673, 0.4028809999999936, 0.39238299999999526, 0.40359399999999823, 0.3926889999999972, 0.3995169999999959, 0.40053599999999534, 0.3995169999999959, 0.3946249999999978, 0.39707099999999684, 0.3826999999999998, 0.40206500000000034, 0.39594999999999914, 0.3969689999999986, 0.3952369999999945, 0.40124999999999744, 0.3954400000000007, 0.3967649999999949, 0.39931299999999936, 0.3960519999999974, 0.3968670000000003, 0.4056319999999971, 0.38942699999999775, 0.3941149999999993, 0.40124999999999744, 0.3980899999999963, 0.3930959999999999, 0.3982939999999999, 0.39737699999999876, 0.3942169999999976, 0.400230999999998], [0.3946249999999978, 0.4024730000000005, 0.39849799999999647, 0.3999249999999961, 0.400230999999998, 0.44395499999999544, 0.39594999999999914, 0.3956439999999972, 0.3995169999999959, 0.39972099999999955, 0.3982939999999999, 0.4013519999999957, 0.4018609999999967, 0.3988039999999984, 0.3961539999999957, 0.3983959999999982, 0.3889169999999993, 0.3960519999999974, 0.40614199999999556, 0.3980899999999963, 0.3949309999999997, 0.4105249999999998, 0.4017589999999984, 0.39329999999999643, 0.3941149999999993, 0.39707099999999684, 0.4003329999999963, 0.3935040000000001, 0.39024200000000064, 0.39329999999999643, 0.3942169999999976, 0.4036959999999965, 0.39329999999999643, 0.4028809999999936, 0.39941499999999763, 0.42214399999999586, 0.39859999999999474, 0.400230999999998, 0.40165799999999763, 0.4018609999999967, 0.4028809999999936, 0.39248500000000064, 0.40043399999999707, 0.40237099999999515, 0.40390000000000015, 0.400230999999998, 0.4036959999999965, 0.4209209999999999, 0.39819199999999455, 0.3926889999999972, 0.4060399999999973, 0.40084199999999726, 0.3934019999999947, 0.39391200000000026, 0.3892229999999941, 0.3949309999999997, 0.40654999999999575, 0.3998229999999978, 0.3968670000000003, 0.3963579999999993, 0.40053599999999534, 0.39747899999999703, 0.3930959999999999, 0.405937999999999, 0.40155599999999936, 0.3910579999999939, 0.39126199999999756, 0.3889169999999993, 0.4003329999999963, 0.392789999999998, 0.40807899999999364, 0.38942699999999775, 0.40012899999999973, 0.4006379999999936, 0.3971729999999951, 0.4208189999999945, 0.4018609999999967, 0.3968670000000003, 0.40084199999999726, 0.39166900000000027, 0.4021669999999986, 0.40043399999999707, 0.4030839999999998, 0.4045109999999994, 0.40002699999999436, 0.3963579999999993, 0.39707099999999684, 0.3911599999999993, 0.39472699999999605, 0.39788599999999974, 0.39554199999999895, 0.3972750000000005, 0.3918729999999968, 0.44589099999999604, 0.39166900000000027, 0.400230999999998, 0.40420599999999496, 0.40012899999999973, 0.40114799999999917, 0.3957459999999955], [0.0009999999999976694, 0.40736499999999864, 0.40430699999999575, 0.0009999999999976694, 0.0009999999999976694, 0.0009999999999976694, 0.0009999999999976694, 0.4013519999999957, 0.0009999999999976694, 0.0009999999999976694, 0.40502099999999785, 0.3910579999999939, 0.39442099999999414, 0.0009999999999976694, 0.0009999999999976694, 0.4399799999999985, 0.39778499999999894, 0.3945229999999995, 0.3948289999999943, 0.0009999999999976694, 0.0009999999999976694, 0.0009999999999976694, 0.0009999999999976694, 0.397987999999998, 0.39238299999999526, 0.0009999999999976694, 0.39656199999999586, 0.3995169999999959, 0.0009999999999976694, 0.0009999999999976694, 0.3956439999999972, 0.3990079999999949, 0.0009999999999976694, 0.0009999999999976694, 0.4033899999999946, 0.0009999999999976694, 0.0009999999999976694, 0.0009999999999976694, 0.40461299999999767, 0.3948289999999943, 0.3982939999999999, 0.0009999999999976694, 0.39503299999999797, 0.3953379999999953, 0.0009999999999976694, 0.0009999999999976694, 0.3996189999999942, 0.40043399999999707, 0.0009999999999976694, 0.39972099999999955, 0.397987999999998, 0.41001499999999425, 0.3982939999999999, 0.3964599999999976, 0.3946249999999978, 0.40237099999999515, 0.4067539999999994, 0.39941499999999763, 0.0009999999999976694, 0.0009999999999976694, 0.0009999999999976694, 0.3987020000000001, 0.3935040000000001, 0.0009999999999976694, 0.0009999999999976694, 0.4021669999999986, 0.4366159999999937, 0.3982939999999999, 0.0009999999999976694, 0.3998229999999978, 0.0009999999999976694, 0.3976830000000007, 0.4022689999999969, 0.3968670000000003, 0.0009999999999976694, 0.0009999999999976694, 0.0009999999999976694, 0.4006379999999936, 0.40277899999999534, 0.38066199999999384, 0.39238299999999526, 0.39360599999999835, 0.0009999999999976694, 0.0009999999999976694, 0.3942169999999976, 0.0009999999999976694, 0.0009999999999976694, 0.0009999999999976694, 0.0009999999999976694, 0.39289199999999624, 0.0009999999999976694, 0.40053599999999534, 0.3930959999999999, 0.39941499999999763, 0.0009999999999976694, 0.39166900000000027, 0.39931299999999936, 0.3982939999999999, 0.0009999999999976694, 0.3893249999999995], [0.0009999999999976694, 0.0009999999999976694, 0.0009999999999976694, 0.0009999999999976694, 0.0009999999999976694, 0.0009999999999976694, 0.0009999999999976694, 0.0009999999999976694, 0.0009999999999976694, 0.0009999999999976694, 0.0009999999999976694, 0.0009999999999976694, 0.0009999999999976694, 0.0009999999999976694, 0.0009999999999976694, 0.0009999999999976694, 0.0009999999999976694, 0.0009999999999976694, 0.0009999999999976694, 0.0009999999999976694, 0.0009999999999976694, 0.0009999999999976694, 0.0009999999999976694, 0.0009999999999976694, 0.0009999999999976694, 0.0009999999999976694, 0.0009999999999976694, 0.0009999999999976694, 0.0009999999999976694, 0.0009999999999976694, 0.0009999999999976694, 0.0009999999999976694, 0.0009999999999976694, 0.0009999999999976694, 0.0009999999999976694, 0.0009999999999976694, 0.0009999999999976694, 0.0009999999999976694, 0.0009999999999976694, 0.0009999999999976694, 0.0009999999999976694, 0.0009999999999976694, 0.0009999999999976694, 0.0009999999999976694, 0.0009999999999976694, 0.0009999999999976694, 0.0009999999999976694, 0.0009999999999976694, 0.0009999999999976694, 0.0009999999999976694, 0.0009999999999976694, 0.0009999999999976694, 0.0009999999999976694, 0.0009999999999976694, 0.0009999999999976694, 0.0009999999999976694, 0.0009999999999976694, 0.0009999999999976694, 0.0009999999999976694, 0.0009999999999976694, 0.0009999999999976694, 0.0009999999999976694, 0.0009999999999976694, 0.0009999999999976694, 0.0009999999999976694, 0.0009999999999976694, 0.0009999999999976694, 0.0009999999999976694, 0.0009999999999976694, 0.0009999999999976694, 0.0009999999999976694, 0.0009999999999976694, 0.0009999999999976694, 0.0009999999999976694, 0.0009999999999976694, 0.0009999999999976694, 0.0009999999999976694, 0.0009999999999976694, 0.0009999999999976694, 0.0009999999999976694, 0.0009999999999976694, 0.0009999999999976694, 0.0009999999999976694, 0.0009999999999976694, 0.0009999999999976694, 0.0009999999999976694, 0.0009999999999976694, 0.0009999999999976694, 0.0009999999999976694, 0.0009999999999976694, 0.0009999999999976694, 0.0009999999999976694, 0.0009999999999976694, 0.0009999999999976694, 0.0009999999999976694, 0.0009999999999976694, 0.0009999999999976694, 0.0009999999999976694, 0.0009999999999976694, 0.0009999999999976694], [0.0009999999999976694, 0.0009999999999976694, 0.0009999999999976694, 0.0009999999999976694, 0.0009999999999976694, 0.0009999999999976694, 0.0009999999999976694, 0.0009999999999976694, 0.0009999999999976694, 0.0009999999999976694, 0.0009999999999976694, 0.0009999999999976694, 0.0009999999999976694, 0.0009999999999976694, 0.0009999999999976694, 0.0009999999999976694, 0.0009999999999976694, 0.0009999999999976694, 0.0009999999999976694, 0.0009999999999976694, 0.0009999999999976694, 0.0009999999999976694, 0.0009999999999976694, 0.0009999999999976694, 0.0009999999999976694, 0.0009999999999976694, 0.0009999999999976694, 0.0009999999999976694, 0.0009999999999976694, 0.0009999999999976694, 0.0009999999999976694, 0.0009999999999976694, 0.0009999999999976694, 0.0009999999999976694, 0.0009999999999976694, 0.0009999999999976694, 0.0009999999999976694, 0.0009999999999976694, 0.0009999999999976694, 0.0009999999999976694, 0.0009999999999976694, 0.0009999999999976694, 0.0009999999999976694, 0.0009999999999976694, 0.0009999999999976694, 0.0009999999999976694, 0.0009999999999976694, 0.0009999999999976694, 0.0009999999999976694, 0.0009999999999976694, 0.0009999999999976694, 0.0009999999999976694, 0.0009999999999976694, 0.0009999999999976694, 0.0009999999999976694, 0.0009999999999976694, 0.0009999999999976694, 0.0009999999999976694, 0.0009999999999976694, 0.0009999999999976694, 0.0009999999999976694, 0.0009999999999976694, 0.0009999999999976694, 0.0009999999999976694, 0.0009999999999976694, 0.0009999999999976694, 0.0009999999999976694, 0.0009999999999976694, 0.0009999999999976694, 0.0009999999999976694, 0.0009999999999976694, 0.0009999999999976694, 0.0009999999999976694, 0.0009999999999976694, 0.0009999999999976694, 0.0009999999999976694, 0.0009999999999976694, 0.0009999999999976694, 0.0009999999999976694, 0.0009999999999976694, 0.0009999999999976694, 0.0009999999999976694, 0.0009999999999976694, 0.0009999999999976694, 0.0009999999999976694, 0.0009999999999976694, 0.0009999999999976694, 0.0009999999999976694, 0.0009999999999976694, 0.0009999999999976694, 0.0009999999999976694, 0.0009999999999976694, 0.0009999999999976694, 0.0009999999999976694, 0.0009999999999976694, 0.0009999999999976694, 0.0009999999999976694, 0.0009999999999976694, 0.0009999999999976694, 0.0009999999999976694], [0.0009999999999976694, 0.0009999999999976694, 0.0009999999999976694, 0.0009999999999976694, 0.0009999999999976694, 0.0009999999999976694, 0.0009999999999976694, 0.0009999999999976694, 0.0009999999999976694, 0.0009999999999976694, 0.0009999999999976694, 0.0009999999999976694, 0.0009999999999976694, 0.0009999999999976694, 0.0009999999999976694, 0.0009999999999976694, 0.0009999999999976694, 0.0009999999999976694, 0.0009999999999976694, 0.0009999999999976694, 0.0009999999999976694, 0.0009999999999976694, 0.0009999999999976694, 0.0009999999999976694, 0.0009999999999976694, 0.0009999999999976694, 0.0009999999999976694, 0.0009999999999976694, 0.0009999999999976694, 0.0009999999999976694, 0.0009999999999976694, 0.0009999999999976694, 0.0009999999999976694, 0.0009999999999976694, 0.0009999999999976694, 0.0009999999999976694, 0.0009999999999976694, 0.0009999999999976694, 0.0009999999999976694, 0.0009999999999976694, 0.0009999999999976694, 0.0009999999999976694, 0.0009999999999976694, 0.0009999999999976694, 0.0009999999999976694, 0.0009999999999976694, 0.0009999999999976694, 0.0009999999999976694, 0.0009999999999976694, 0.0009999999999976694, 0.0009999999999976694, 0.0009999999999976694, 0.0009999999999976694, 0.0009999999999976694, 0.0009999999999976694, 0.0009999999999976694, 0.0009999999999976694, 0.0009999999999976694, 0.0009999999999976694, 0.0009999999999976694, 0.0009999999999976694, 0.0009999999999976694, 0.0009999999999976694, 0.0009999999999976694, 0.0009999999999976694, 0.0009999999999976694, 0.0009999999999976694, 0.0009999999999976694, 0.0009999999999976694, 0.0009999999999976694, 0.0009999999999976694, 0.0009999999999976694, 0.0009999999999976694, 0.0009999999999976694, 0.0009999999999976694, 0.0009999999999976694, 0.0009999999999976694, 0.0009999999999976694, 0.0009999999999976694, 0.0009999999999976694, 0.0009999999999976694, 0.0009999999999976694, 0.0009999999999976694, 0.0009999999999976694, 0.0009999999999976694, 0.0009999999999976694, 0.0009999999999976694, 0.0009999999999976694, 0.0009999999999976694, 0.0009999999999976694, 0.0009999999999976694, 0.0009999999999976694, 0.0009999999999976694, 0.0009999999999976694, 0.0009999999999976694, 0.0009999999999976694, 0.0009999999999976694, 0.0009999999999976694, 0.0009999999999976694, 0.0009999999999976694], [0.0009999999999976694, 0.0009999999999976694, 0.0009999999999976694, 0.0009999999999976694, 0.0009999999999976694, 0.0009999999999976694, 0.0009999999999976694, 0.0009999999999976694, 0.0009999999999976694, 0.0009999999999976694, 0.0009999999999976694, 0.0009999999999976694, 0.0009999999999976694, 0.0009999999999976694, 0.0009999999999976694, 0.0009999999999976694, 0.0009999999999976694, 0.0009999999999976694, 0.0009999999999976694, 0.0009999999999976694, 0.0009999999999976694, 0.0009999999999976694, 0.0009999999999976694, 0.0009999999999976694, 0.0009999999999976694, 0.0009999999999976694, 0.0009999999999976694, 0.0009999999999976694, 0.0009999999999976694, 0.0009999999999976694, 0.0009999999999976694, 0.0009999999999976694, 0.0009999999999976694, 0.0009999999999976694, 0.0009999999999976694, 0.0009999999999976694, 0.0009999999999976694, 0.0009999999999976694, 0.0009999999999976694, 0.0009999999999976694, 0.0009999999999976694, 0.0009999999999976694, 0.0009999999999976694, 0.0009999999999976694, 0.0009999999999976694, 0.0009999999999976694, 0.0009999999999976694, 0.0009999999999976694, 0.0009999999999976694, 0.0009999999999976694, 0.0009999999999976694, 0.0009999999999976694, 0.0009999999999976694, 0.0009999999999976694, 0.0009999999999976694, 0.0009999999999976694, 0.0009999999999976694, 0.0009999999999976694, 0.0009999999999976694, 0.0009999999999976694, 0.0009999999999976694, 0.0009999999999976694, 0.0009999999999976694, 0.0009999999999976694, 0.0009999999999976694, 0.0009999999999976694, 0.0009999999999976694, 0.0009999999999976694, 0.0009999999999976694, 0.0009999999999976694, 0.0009999999999976694, 0.0009999999999976694, 0.0009999999999976694, 0.0009999999999976694, 0.0009999999999976694, 0.0009999999999976694, 0.0009999999999976694, 0.0009999999999976694, 0.0009999999999976694, 0.0009999999999976694, 0.0009999999999976694, 0.0009999999999976694, 0.0009999999999976694, 0.0009999999999976694, 0.0009999999999976694, 0.0009999999999976694, 0.0009999999999976694, 0.0009999999999976694, 0.0009999999999976694, 0.0009999999999976694, 0.0009999999999976694, 0.0009999999999976694, 0.0009999999999976694, 0.0009999999999976694, 0.0009999999999976694, 0.0009999999999976694, 0.0009999999999976694, 0.0009999999999976694, 0.0009999999999976694, 0.0009999999999976694], [0.0009999999999976694, 0.0009999999999976694, 0.0009999999999976694, 0.0009999999999976694, 0.0009999999999976694, 0.0009999999999976694, 0.0009999999999976694, 0.0009999999999976694, 0.0009999999999976694, 0.0009999999999976694, 0.0009999999999976694, 0.0009999999999976694, 0.0009999999999976694, 0.0009999999999976694, 0.0009999999999976694, 0.0009999999999976694, 0.0009999999999976694, 0.0009999999999976694, 0.0009999999999976694, 0.0009999999999976694, 0.0009999999999976694, 0.0009999999999976694, 0.0009999999999976694, 0.0009999999999976694, 0.0009999999999976694, 0.0009999999999976694, 0.0009999999999976694, 0.0009999999999976694, 0.0009999999999976694, 0.0009999999999976694, 0.0009999999999976694, 0.0009999999999976694, 0.0009999999999976694, 0.0009999999999976694, 0.0009999999999976694, 0.0009999999999976694, 0.0009999999999976694, 0.0009999999999976694, 0.0009999999999976694, 0.0009999999999976694, 0.0009999999999976694, 0.0009999999999976694, 0.0009999999999976694, 0.0009999999999976694, 0.0009999999999976694, 0.0009999999999976694, 0.0009999999999976694, 0.0009999999999976694, 0.0009999999999976694, 0.0009999999999976694, 0.0009999999999976694, 0.0009999999999976694, 0.0009999999999976694, 0.0009999999999976694, 0.0009999999999976694, 0.0009999999999976694, 0.0009999999999976694, 0.0009999999999976694, 0.0009999999999976694, 0.0009999999999976694, 0.0009999999999976694, 0.0009999999999976694, 0.0009999999999976694, 0.0009999999999976694, 0.0009999999999976694, 0.0009999999999976694, 0.0009999999999976694, 0.0009999999999976694, 0.0009999999999976694, 0.0009999999999976694, 0.0009999999999976694, 0.0009999999999976694, 0.0009999999999976694, 0.0009999999999976694, 0.0009999999999976694, 0.0009999999999976694, 0.0009999999999976694, 0.0009999999999976694, 0.0009999999999976694, 0.0009999999999976694, 0.0009999999999976694, 0.0009999999999976694, 0.0009999999999976694, 0.0009999999999976694, 0.0009999999999976694, 0.0009999999999976694, 0.0009999999999976694, 0.0009999999999976694, 0.0009999999999976694, 0.0009999999999976694, 0.0009999999999976694, 0.0009999999999976694, 0.0009999999999976694, 0.0009999999999976694, 0.0009999999999976694, 0.0009999999999976694, 0.0009999999999976694, 0.0009999999999976694, 0.0009999999999976694, 0.0009999999999976694]]
  out "Current Map":dbl[][](array[numeric])
  in  "Scan Termination":T6(ring)=enum."Center of scan"
  in  "Scan Type":enum16{"Sinusoidal", "Spiral"}(ring)
  in  "Scan Velocity":dbl=0.1910828025477707
  in  "Analog Input":i32=4 min=1 max=5 step=1
  in  "Scan Frequency":dbl=0.9554140127388535
  in  "Table rate":i32=5
  out "Nano AS Data":dbl[][](array[numeric])
  in  "Speed factor":dbl=1.0
  in  "Max velocity":dbl=3.0
  in  "Min Radius":dbl=0.1
  in  "Max Radius":dbl=1.0
  in  "GS Frequency":dbl=2.5
  in  "Max. dir. changes":i32=50
  in  "ML":dbl=0.1
  out "AS Duration (msec)":u32=62855
  out "Received String":string=">>SPA? 1 0x0E000200\r\n1 0xe000200=4.999999874e-005"
  in  "String To Send":string
  out "Identification":string="(c)2015-2018 Physik Instrumente (PI) GmbH & Co. KG, E-712.3CDA, 117006756, 14.10.12.05"
  out "S/N":string="117006756"
  in  "Logging mode":bool
  out "Path to conf file":path=path "C:/Users/brk1273pc1/PI QC Workstation_Brandon_v4.vi"
  # "PHOTON COUNTING"
  # "Quantum Emitter Measurement Station"
  # "Stage Position"
  # "X\nY\nZ"
  # "Scanning"
  # "on"
  # "off"
  # "Mirror Configuration"
  # "Laser Power"
  # "Filter Configuration"
  # "Initialization Errors"
  # "TAC / Time Range"
  # "CFD"
  # "(start)"
  # "SYNC"
  # "(stop)"
  # "range"
  # "gain"
  # "threshold(LL)"
  # "offset"
  # "limit high"
  # "limit low"
  # "zero cross(ZC)"
  # "Collection Time"
  # "TAC / Time Range"
  # "CFD"
  # "(start)"
  # "SYNC"
  # "(stop)"
  # "range"
  # "gain"
  # "threshold(LL)"
  # "offset"
  # "limit high"
  # "limit low"
  # "zero cross(ZC)"
  # "Collection Time"
  # "Saturation Set saturation start angle as an angle that corresponds to a very low laser power. Set end angle as maximum power you wish to measure. Select end angle such that it's greater than start angle because the rotation direction is fixed. Press \"measure saturation\" to begin the measurement. Saturation will prompt you to save it automatically.\n\nAutosaturation will take saturation measurements at the selected points saved in memory (right column) and save them automatically. Be sure to set your save path (top right). \n\nStability is measured by pressing \"record counts\", you can pause/resume the measurment with this button. \"Write to file\" will save the data displayed. Clear memory is used to clear the data to start another measurment.\n\nThe counts written to memory are from all the detectors summed up, it does not matter if you measure on PDMs or SPCM."
  # "Measurements to run:"
  # "Auto Emitter Analysis"
  # "Alignment Scan"
  # "MAP CONTROLS"
  # "buffer"
  # "current"
  # "TAC / Time Range"
  # "CFD"
  # "(start)"
  # "SYNC"
  # "(stop)"
  # "range"
  # "gain"
  # "threshold(LL)"
  # "offset"
  # "limit high"
  # "limit low"
  # "zero cross(ZC)"
  # "Collection Time"
  # "TAC / Time Range"
  # "CFD"
  # "(start)"
  # "SYNC"
  # "(stop)"
  # "range"
  # "gain"
  # "threshold(LL)"
  # "offset"
  # "limit high"
  # "limit low"
  # "zero cross(ZC)"
  # "Collection Time"
  # "Areal Scan Parameters"
  # "Gradient Search Parameters"
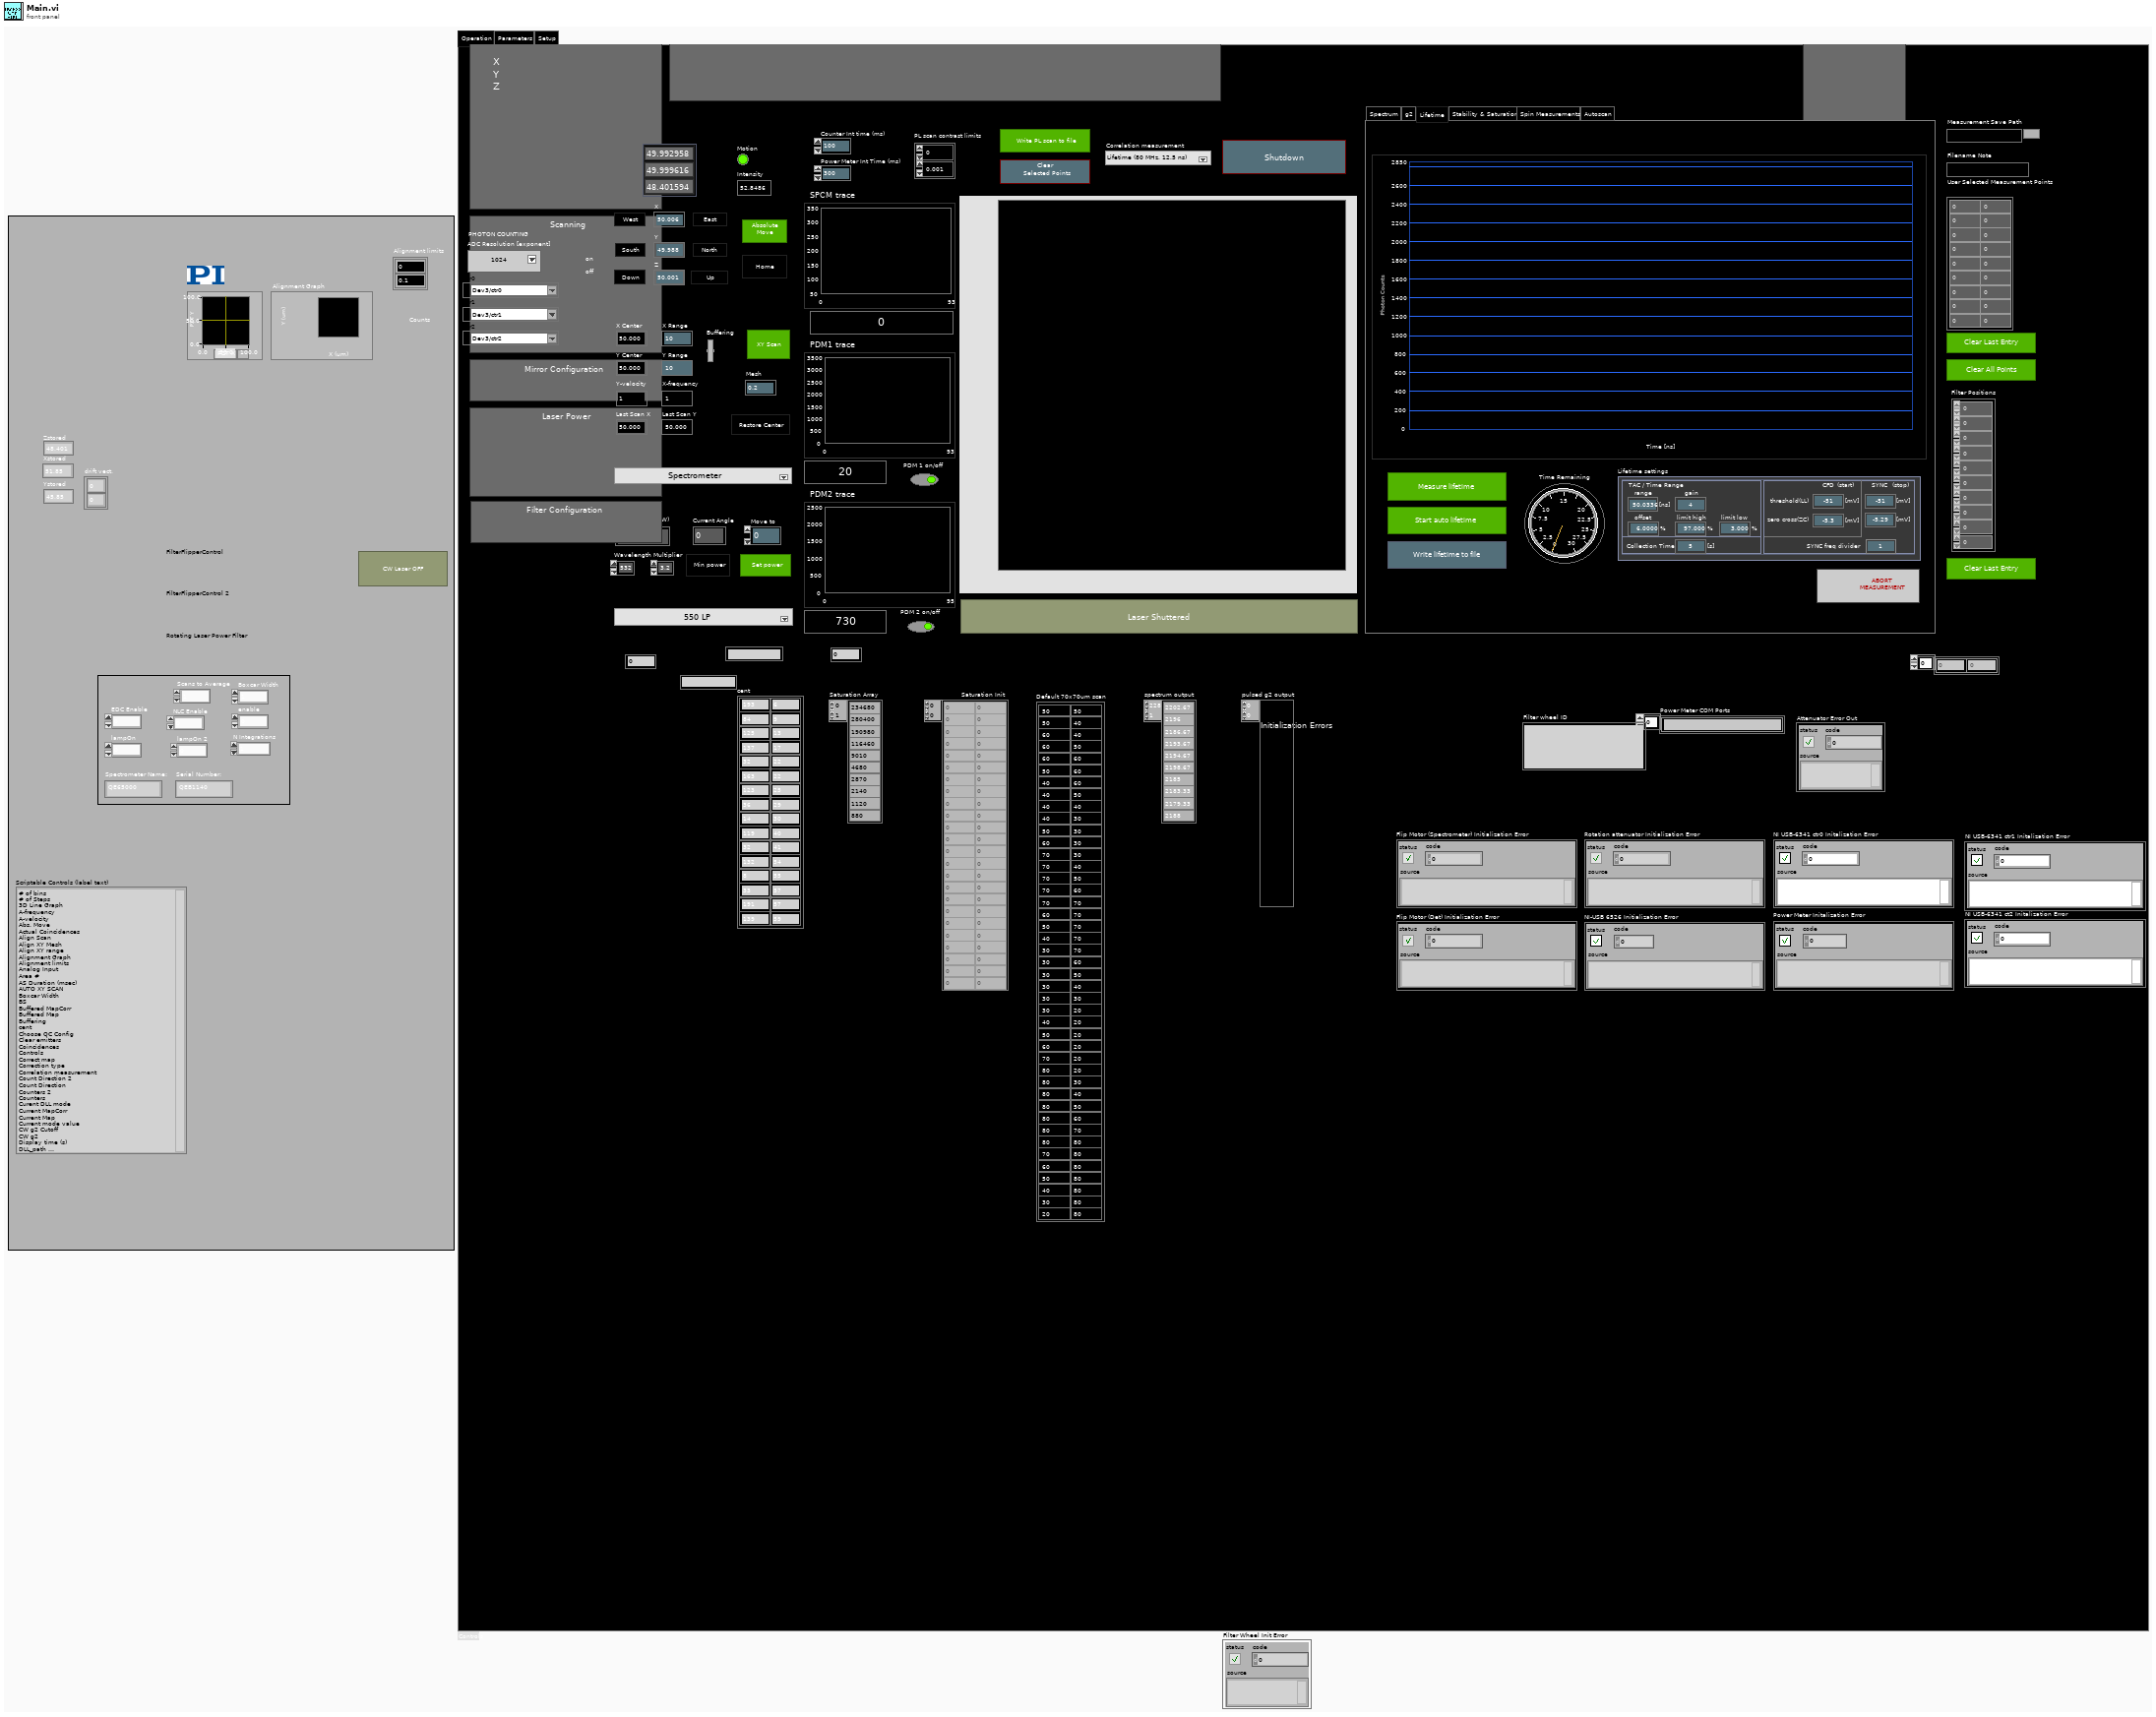
[diagram p1: front panel]
types:
  T1 = typedef "ADCResolution.ctl" = i16
  T2 = typedef "Control 1.ctl" = u32
  T3 = enum32{"Spectrum", "g2", "Lifetime", "Stability & Saturation", "Spin Measurements", "Autoscan"}
  T4 = typedef "UserInput.ctl" = cluster{"tac_range":sgl, "tac_gain":i16, "tac_offset":sgl, "tac_limit_high":sgl, "tac_limit_low":sgl, "collect_time":sgl, "sync_threshold":sgl, "sync_zc_level":sgl, "sync_freq_div":i16, "cfd_limit_low":sgl, "cfd_zc_level":sgl}
  T5 = typedef "CorrelationSwitchControlType.ctl" = u16
  T6 = enum16{"Maximum", "End Position", "Center of scan"}
  T7 = typedef "DialogType.ctl" = u16
  T8 = enum8{"Enabled", "Disabled", "Disabled and Grayed Out"}
  T9 = enum16{"Turn off when wheel is idle to eliminate stray light", "Remain active"}
  T10 = typedef "ConfigMem.ctl" = cluster{"Max Block No":i32, "Blocks Per Frame":i32, "Frames Per Page":i32, "Maxpage":i32, "Block Length":i32}
  T11 = cluster{"SPCMemConfig":T10, "DLL Path":path, "Module No":i16, "Page":i32}
  T12 = typedef "MeasurementType.ctl" = enum16{"PL Map", "Spectrum", "Lifetime", "g2", "Stability", "Saturation"}
  T13 = cluster{"Width":u16, "Style":enum32{"Solid", "Dash", "Dot", "DashDot", "DashDotDot"}}
  T14 = enum16{"Maximum", "End Position", "Center of scan", ""}
  T15 = cluster{"System no.":i32, "Xoffset":dbl, "Yoffset":dbl, "Array":dbl[][], "Mesh":dbl, "cent":i32[][], "Numeric":i32}
  T16 = cluster{"Measurement Save Path":path, "Autoscan Emitter Position":dbl[], "Current Angle":sgl, "Filename Note":string}
  T17 = typedef "imagedata.ctl" = cluster{"image type":i32, "image depth":i32, "image":u8[], "mask":u8[], "colors":u32[], "Rectangle":cluster{"left":i16, "top":i16, "right":i16, "bottom":i16}}
  T18 = typedef "LVPoint32TypeDef.ctl" = cluster{"Horizontal":i32, "Vertical":i32}
  T19 = typedef "LVRectTypeDef.ctl" = cluster{"Left":i16, "Top":i16, "Right":i16, "Bottom":i16}
  T20 = cluster{"task out":refnum<k21>, "task out":refnum<k21>, "task out":refnum<k21>}
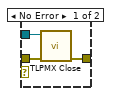
[diagram p2: hidden frame]
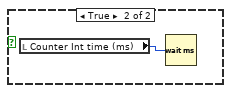
[diagram p3: hidden frame]
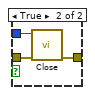
[diagram p4: hidden frame]
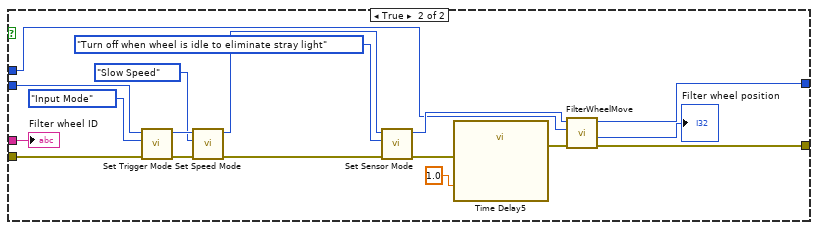
[diagram p5: hidden frame]
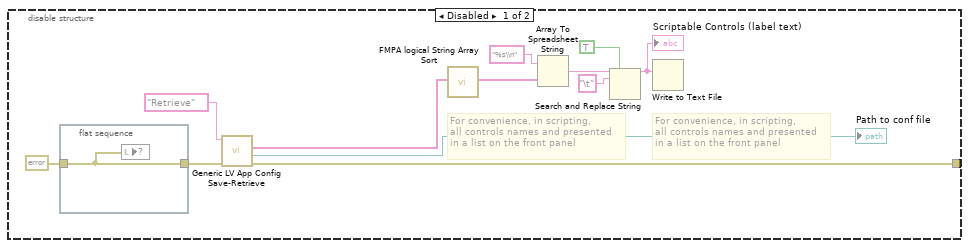
[diagram p6: hidden frame]
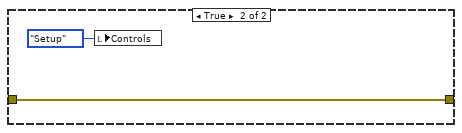
[diagram p7: hidden frame]
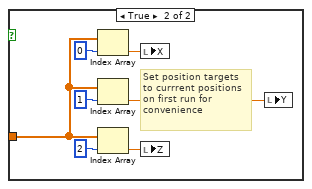
[diagram p11: hidden frame]
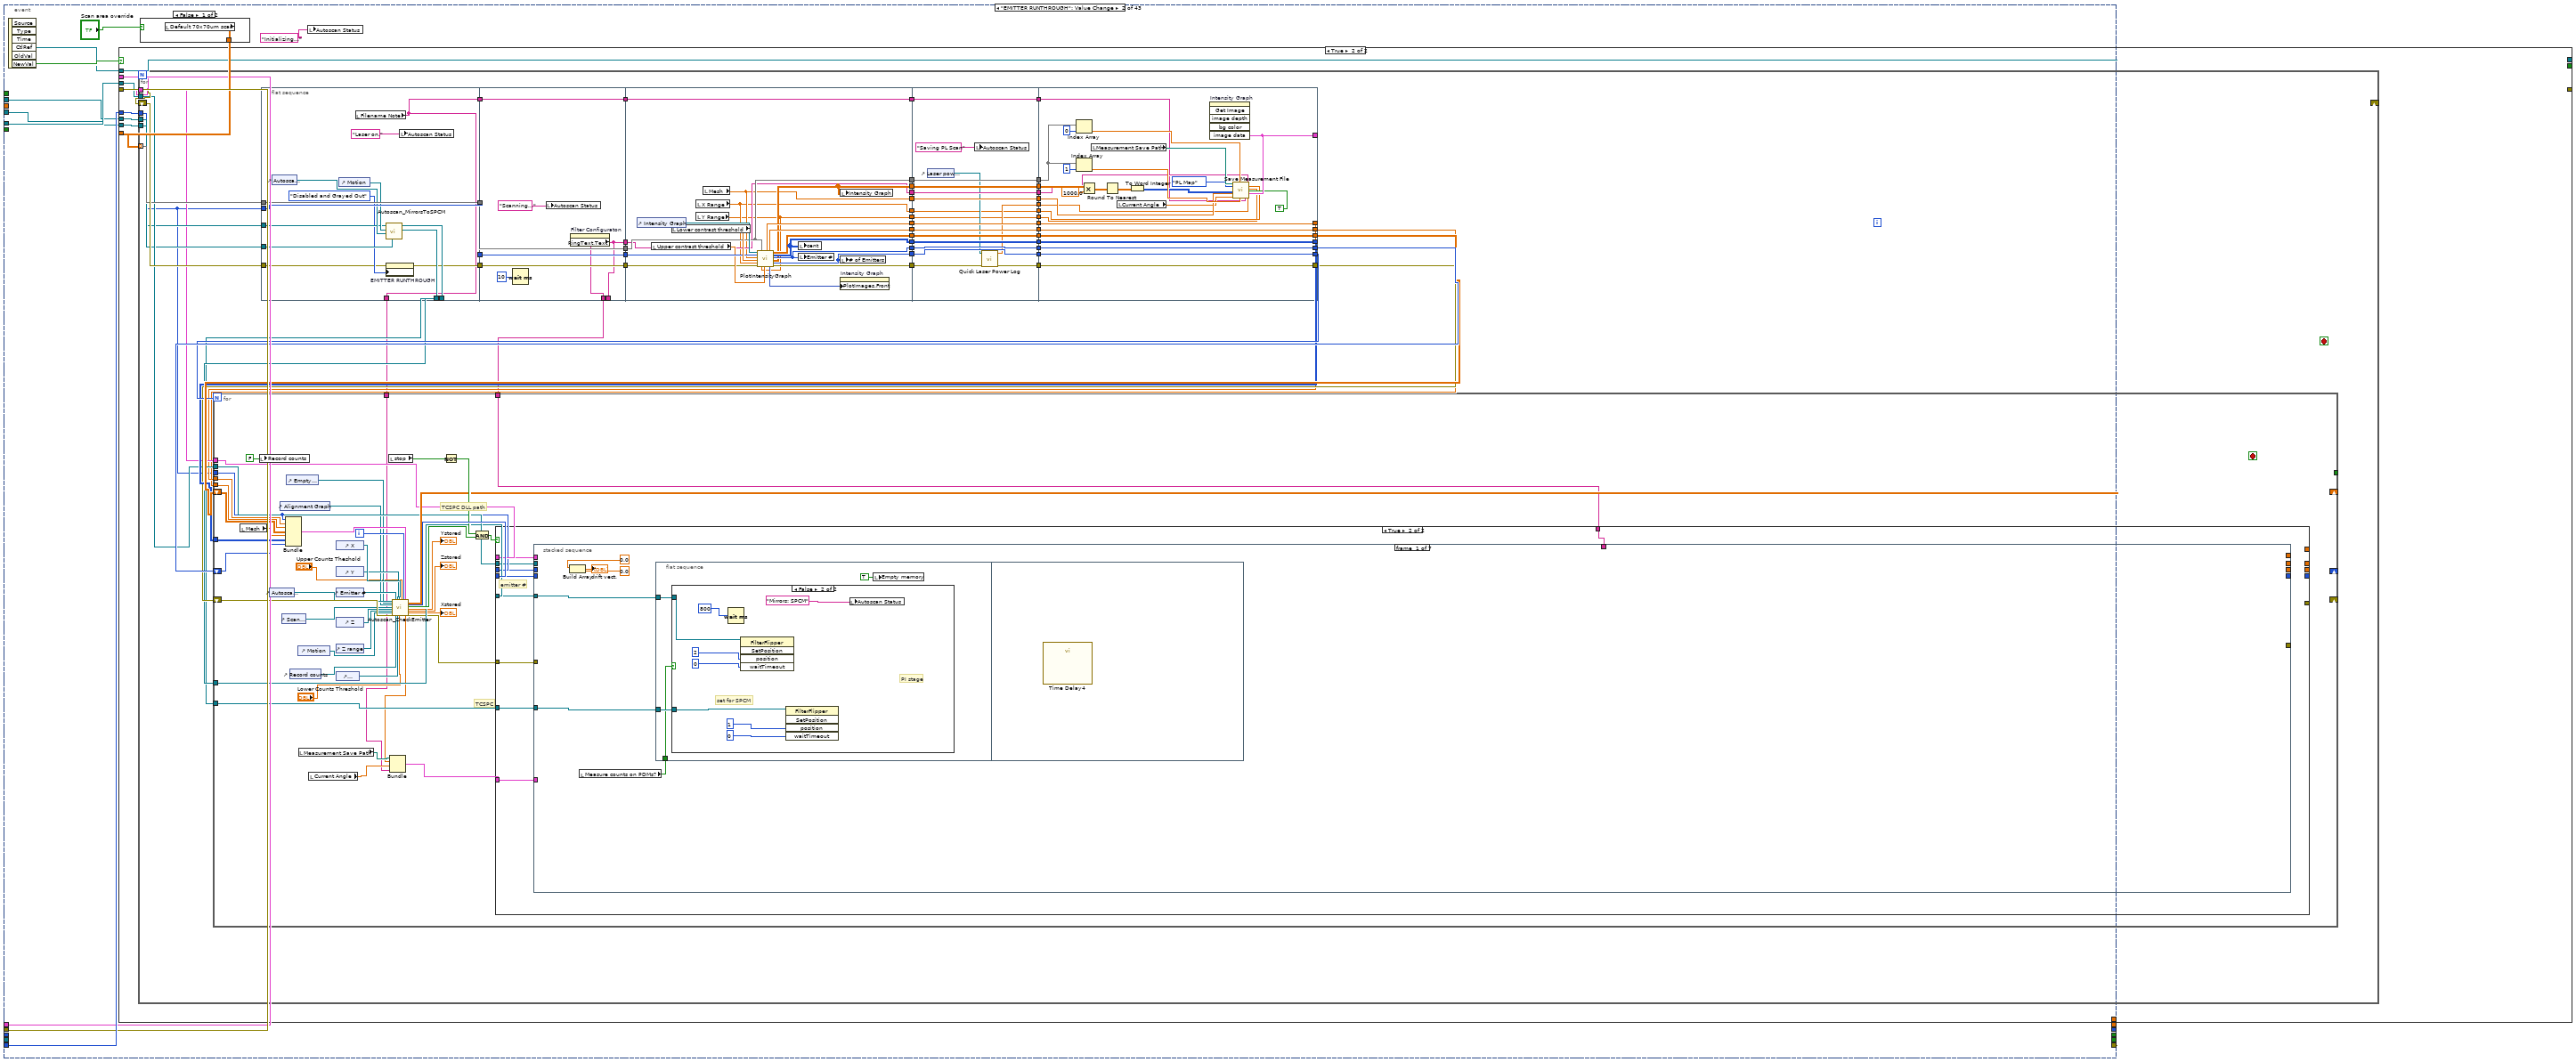
[diagram p12: hidden frame]
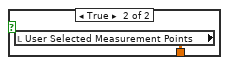
[diagram p13: hidden frame]
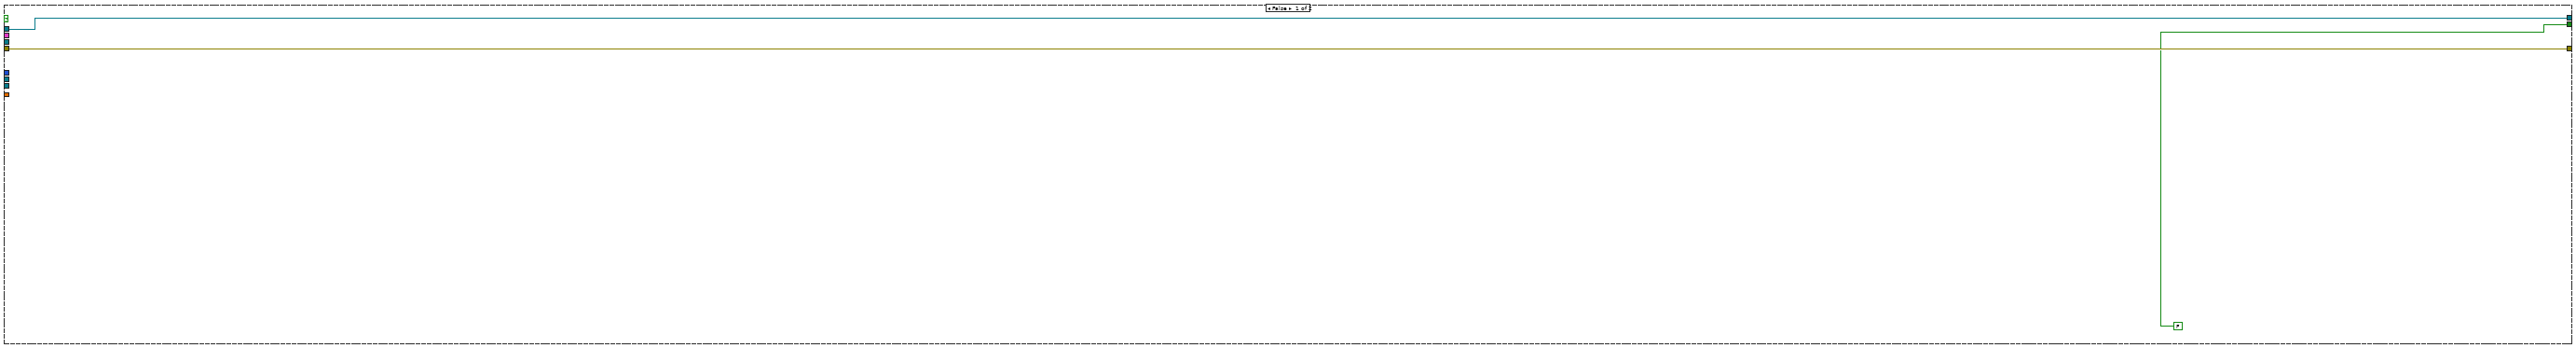
[diagram p14: hidden frame]
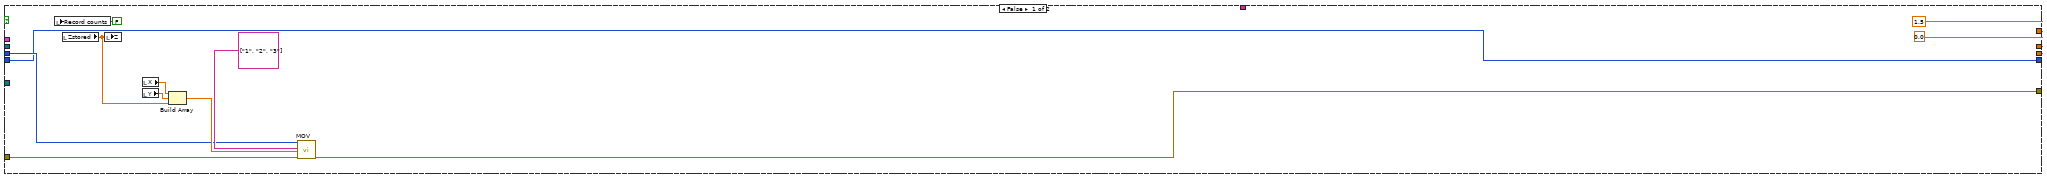
[diagram p15: hidden frame]
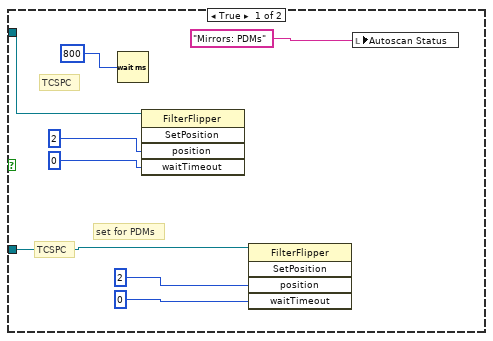
[diagram p16: hidden frame]
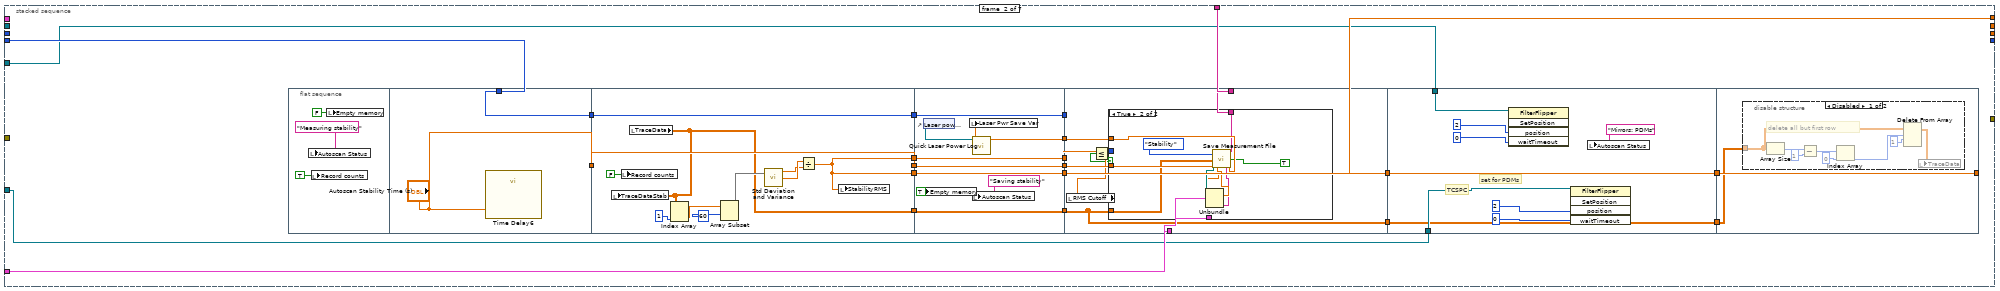
[diagram p17: hidden frame]
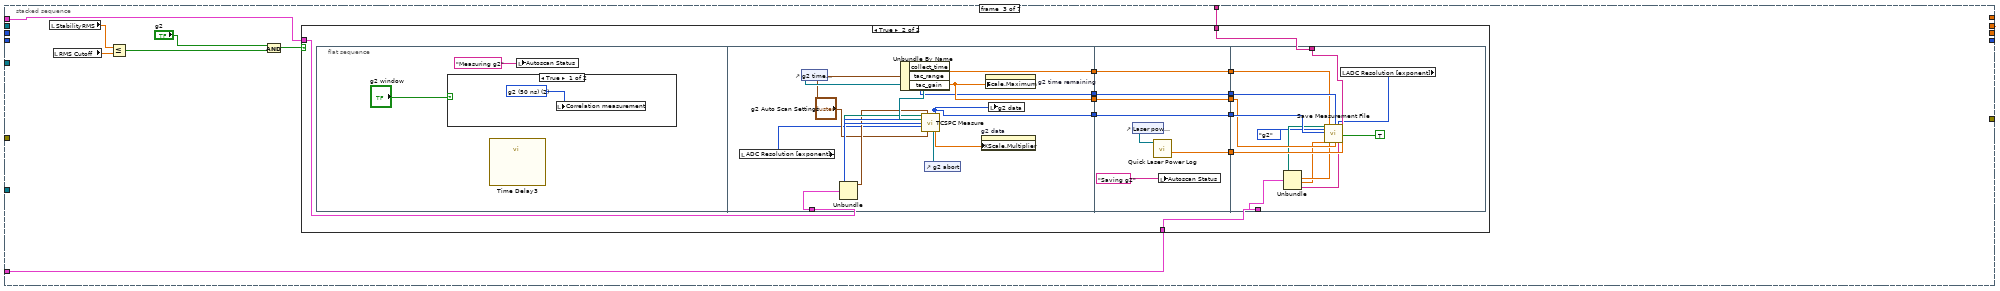
[diagram p20: hidden frame]
diagram:
  w42 = T7 3 items=["no dialog", "OK message", "continue or stop message", "OK message + warnings", "continue/stop + warnings"] ("type of dialog (OK msg:1)")
  (unwired) FALSE  # Nano GS active?
  w60 = T7 0 items=["no dialog", "OK message", "continue or stop message", "OK message + warnings", "continue/stop + warnings"] ("type of dialog (OK msg:1)")
  # "check this"
  # "If the device doesn't initialize then ignore"
  # "On termination, stop logging (if it's on), stop\nall fast alignment processes, and if there's an\nerror situation, show the Setup pane with\nits error indicator."
  n1 = disable-structure shown="Enabled" {
    disable-tunnel: [w69 _] -> w12
    frame Disabled {
      # "For convenience, in scripting,\nall controls names and presented\nin a list on the front panel"
      # "For convenience, in scripting,\nall controls names and presented\nin a list on the front panel"
      n2 = flat-sequence {
        tunnel: errorcluster {"status"=FALSE, "code"=0, "source"=""} ("error in") -> [w79]
        tunnel: [w79] -> w70
        frame #0 {
          n3 = local write item#-1(w79) -> ()
        }
      }
      n4 = call "Generic LV App Config Save-Retrieve.vi"("error in"=w70, "Save/Retrieve"="Retrieve") -> ("error out"=w69:errorcluster, "Path to conf file"=→"Path to conf file":path, "Calling VI's Controls"=w76:string[])  [unwired: 5 in, 2 out]
      n5 = call "FMPA logical String Array Sort.vi"("Unsorted List"=w76) -> ("Sorted List"=w71:string[])  [unwired: 18 in]
      n6 = Array To Spreadsheet String(array=w71, 3:"%s\\n" ("format string")) -> (spreadsheet string=w74:string)  [unwired: 1 in]
      n7 = Search and Replace String(replace all?=TRUE ("replace all? (F)"), input string=w74, search string="\t") -> (result string=w67:string)  [unwired: 5 in, 3 out]
      "Scriptable Controls (label text)" <- w67
      n8 = Write to Text File(text=w67) -> ()  [unwired: 3 in, 3 out]
    }
    frame Enabled {
      # "Retrieve all  control settings from the .conf file if it exists.\n\nThe .conf file is created in the user's home directory on\nevery non-error conclusion of this VI.  It is not written\nif an error condition exists or if the LabVIEW halt button\nis pressed."
    }
  }
  n9 = flat-sequence {
    tunnel: w12 -> [w80]
    tunnel: [w80] -> w11
    frame #0 {
      w81 = FALSE ("Abs. Move")
      # "Variable Initialiation"
      n10 = flat-sequence {
        frame #0 {
          # "Brandon's Auto Measurements"
        }
      }
      n11 = flat-sequence {
        frame #0 {
          # "Scan variables"
        }
      }
      n12 = flat-sequence {
        frame #0 {
          # "Alignment variables"
        }
      }
      n13 = flat-sequence {
        frame #0 {
          n14 = Initialize Array(0.0 ("element"), 1 ("dimension size"), 2 ("dimension size")) -> (→"TraceData" →"TraceDataStab":dbl[][])
          n15 = local write "Empty memory"(FALSE ("Empty memory")) -> ()
          n16 = local write "EMITTER RUNTHROUGH"(FALSE ("EMITTER RUNTHROUGH")) -> ()
        }
      }
      n17 = local write "Controls"(enum32{"Operation", "Parameters", "Setup"}."Operation" ("Controls")) -> ()
      n18 = flat-sequence {
        frame #0 {
        }
      }
      n19 = flat-sequence {
        frame #0 {
          w91 = T8."Enabled" ("Disabled")
          n20 = property on="stop" class="Bool (strict)"("Value"=FALSE ("stop")) -> (error out=w95:errorcluster)  [unwired: 2 in, 1 out]
          n21 = property on="Meaure lifetime" class="Bool (strict)"(error in=w95, "DisabledEnum"=w91) -> (error out=w94:errorcluster)  [unwired: 1 in, 1 out]
          n22 = property on="Measure g2" class="Bool (strict)"(error in=w94, "DisabledEnum"=w91) -> (error out=w93:errorcluster)  [unwired: 1 in, 1 out]
          n23 = property on="Measure spectrum" class="Bool (strict)"(error in=w93, "DisabledEnum"=w91) -> (error out=w92:errorcluster)  [unwired: 1 in, 1 out]
          n24 = property on="Measure saturation" class="Bool (strict)"(error in=w92, "DisabledEnum"=w91) -> (error out=w90:errorcluster)  [unwired: 1 in, 1 out]
          n25 = property on="EMITTER RUNTHROUGH" class="Bool (strict)"(error in=w90, "DisabledEnum"=w91) -> (error out=w89:errorcluster)  [unwired: 1 in, 1 out]
          n26 = property on="Stop Autoscan" class="Bool (strict)"(error in=w89, "DisabledEnum"=w91) -> ()  [unwired: 1 in, 2 out]
        }
      }
      n27 = local write "XY Scan"(w81) -> ()
      n28 = local write "stop"(w81) -> ()
      n29 = local write "Write PL map to file"(w81) -> ()
      n30 = local write "Write Alignment map to file"(w81) -> ()
      n31 = local write "Laser Shutter"(w81) -> ()
      n32 = local write "Abs. Move"(w81) -> ()
      n33 = flat-sequence {
        frame #0 {
          # "Spectrometer Variables"
        }
      }
      n34 = Build Array("west", "east", "south", "north", "down", "up") -> ()  [unwired: 1 out]
    }
  }
  n35 = flat-sequence {
    tunnel: [w105] -> w51
    tunnel: [w106] -> w38
    tunnel: [w103] -> w49
    frame #0 {
      # "Filter Wheel Initalization"
      n36 = call <instrlib>:"List COM port.vi"() -> ("error out"=w110:errorcluster, "COM Ports"=w113:string[])  [unwired: 10 in]
      "Power Meter COM Ports" <- w113
      n37 = Reverse 1D Array(array=w113) -> (reversed array=w112:string[])
      n38 = Index Array(array=w112) -> (element=w111:string)  [unwired: 1 in]
      n39 = call <instrlib>:"Open.vi"("error in (no error)"=w110, "Serial Port"=w111) -> ("error out"=w114:errorcluster, "hdl out"=w115:i32, "Connected?"=w103:bool)  [unwired: 7 in]
      n40 = call <instrlib>:"Get ID.vi"("error in (no error)"=w114, "hdl in"=w115) -> ("error out"=w107:errorcluster, "ID"=w109:string, "hdl out"=w108:i32)  [unwired: 7 in]
      n41 = case shown="False" w103 {
        tunnel: w109 -> [_ w135]
        tunnel: w108 -> [w117 w128]
        tunnel: w107 -> [w116 w127]
        tunnel: [w116 w125] -> w106
        tunnel: [w117 w124] -> w105
        tunnel: "Filter Configuraton" -> [_ w123]
        frame False {
          # "If the device never connects just ignore it"
        }
        frame True {
          n42 = call <instrlib>:"Set Trigger Mode.vi"("error in (no error)"=w127, "Set Trigger Mode"=enum16{"Input Mode", "Output Mode"}."Input Mode", "hdl in"=w128) -> ("error out"=w132:errorcluster, "hdl out"=w134:i32)  [unwired: 7 in]
          n43 = call <instrlib>:"Set Speed Mode.vi"("error in (no error)"=w132, "Set Speed Mode"=enum16{"Slow Speed", "High Speed"}."Slow Speed", "hdl in"=w134) -> ("error out"=w131:errorcluster, "hdl out"=w133:i32)  [unwired: 7 in]
          n44 = call <instrlib>:"Set Sensor Mode.vi"("error in (no error)"=w131, "Set Sensor Mode"=T9."Turn off when wheel is idle to eliminate stray light", "hdl in"=w133) -> ("error out"=w122:errorcluster, "hdl out"=w126:i32)  [unwired: 7 in]
          n45 = call "Time Delay5"("error in (no error)"=w122, "Delay Time (s)"=1.0) -> ("error out"=w121:errorcluster)  [unwired: 9 in]
          n46 = call "FilterWheelMove.vi"("error in (no error)"=w121, "Filter Configuraton"=w123, "hdl in"=w126) -> ("error out"=w125:errorcluster, "Get Position"=→"Filter wheel position":i32, "hdl out"=w124:i32)  [unwired: 6 in]
          "Filter wheel ID" <- w135
        }
      }
    }
  }
  n47 = flat-sequence {
    tunnel: [w136] -> w47
    frame #0 {
      # "DAQmx is NI 6525 device"
      # "NI USB-6525 (I/O Relay device) Initialization"
      n48 = Build Array(tag "Dev2/port0/line0" ("lines"), tag "Dev2/port0/line2" ("lines"), tag "Dev2/port0/line3" ("element"), tag "Dev2/port0/line4" ("element"), tag "Dev2/port0/line5" ("element"), tag "Dev2/port0/line7" ("lines"), tag "Dev2/port0/line6" ("lines")) -> (w145:tag[])
      n49 = call <vilib>:"DAQmx Flatten Channel String.vi"("names in"=w145) -> ("names out"=w143:string, "error out"=w147:errorcluster)  [unwired: 13 in]
      n50 = call-poly <vilib>:"DAQmx Create Virtual Channel.vi"("lines"=w143, "error in"=w147) -> ("task out"=w149:refnum<k21>, "error out"=w148:errorcluster)  [unwired: 12 in]
      n51 = call <vilib>:"DAQmx Start Task.vi"("task/channels in"=w149, "error in"=w148) -> ("task out"=w136:refnum<k21>, "error out"=→"NI-USB 6526 Initialization Error":errorcluster)  [unwired: 12 in]
    }
  }
  n52 = flat-sequence {
    tunnel: [w152] -> w56
    tunnel: [w152] -> w15
    tunnel: [w151] -> w14
    tunnel: w11 -> [w150]
    frame #0 {
      w154 = TRUE  # Parameter no. format  (Decimal: FALSE)
      w161 = TRUE  # Stop wave generator output (if any)
      w160 = FALSE  # Move to middle?
      w162 = 20000  # Timeout
      w164 = FALSE  # Perform autozero?
      w165 = TRUE  # Change servo status to ON?
      w152 = 1  # System no.
      w163 = u16 2 items=["RS232", "TCP/IP", "USB"] ("Interface")
      w174 = string[] ["1", "2", "3"] ("Routinename")
      # "Re-enable"
      # "PI Piezo Stage Initialization"
      n53 = call "Set logging mode.vi"("Logging mode"="Logging mode", "File dialog?"=TRUE, "error in"=w150) -> ("error out"=w171:errorcluster)  [unwired: 16 in]
      n54 = call "E712_Configuration_Setup.vi"("System no."=w152, "USB settings"=cluster{"S/N":string, "USB Search?":bool} {"S/N"="117006756", "USB Search?"=FALSE}, "Change servo status to ON?"=w165, "Perform autozero?"=w164, "error in"=w171, "Interface"=w163, "Timeout"=w162, "Stop wave generator\noutput (if any)"=w161, "Move to middle?"=w160) -> ("Identification"=→"Identification":string, "USB: S/N out"=→"S/N":string, "error out"=w169:errorcluster)  [unwired: 6 in, 2 out]
      n55 = call "CCL.vi"("System no."=w152, "Command level"=1, "Password"="advanced", "error in"=w169) -> ("error out"=w170:errorcluster)  [unwired: 14 in, 1 out]
      n56 = call "SPA.vi"("System no."=w152, "Axis to set"=string[] ["1"], "Parameter value"=dbl[] [3.0], "error in"=w170, "Parameter no. format \n(Decimal: FALSE)"=w154, "Parameter number (hex)"=u32[] [369099520]) -> ("error out"=w151:errorcluster)  [unwired: 12 in, 1 out]
      n57 = call "FRP?.vi"("System no."=w152, "Routines to query"=w174, "error in"=w151) -> ("error out"=w173:errorcluster)  [unwired: 15 in, 1 out]
      n58 = call "FRP.vi"("System no."=w152, "Routinename"=w174, "Option"=i32[] [0, 0], "error in"=w173) -> ("error out"=w176:errorcluster)  [unwired: 15 in]
      n59 = call "ERR?.vi"("System no."=w152, "error in"=w176) -> ()  [unwired: 16 in, 2 out]
    }
  }
  n60 = flat-sequence {
    tunnel: [w178] -> w18
    frame #0 {
      w177 = T1 10 items=["-1"=-1, "1"=0, "4"=2, "16"=4, "64"=6, "256"=8, "1024"=10, "4096"=12] ("ADC Resolution [exponent]")
      # "B&H TCSPC Initialization"
      n61 = call "TCSPC Initialize.vi"("ADC Resolution [exponent]"=w177) -> ("Page"=w179:i32, "Module No"=w180:i16, "DLL Path"=w181:path, "SPCMemConfig"=w182:T10)  [unwired: 5 in, 2 out]
      n62 = Bundle "B&H"("SPCMemConfig"=w182, "DLL Path"=w181, "Module No"=w180, "Page"=w179) -> (w178:T11)  [unwired: 1 in]
      "ADC Resolution [exponent]" <- w177
    }
  }
  n63 = call "FDG.vi"("System no."=w15, "Routinename"="2" ("String"), "Axis settings"=cluster{"Scan axis":string, "Step axis":string} {"Scan axis"="1", "Step axis"="2"}, "error in"=w14) -> ("error out"=w13:errorcluster)  [unwired: 15 in]
  n64 = Initialize Array(FALSE, 6) -> (w52:bool[])
  n65 = while {
    shift-right: [w200] -> _
    shift-left: _ -> [w198]
    tunnel: w56 -> [w199]
    shift-right: [w189] -> w22
    shift-left: w13 -> [w197]
    tunnel: w4 -> [w196]
    tunnel: w54 -> [w195]
    tunnel: w53 -> [w194]
    shift-right: [w191] -> _
    shift-left: w52 -> [w192]
    tunnel: w51 -> [w190]
    tunnel: [w187] -> w50
    tunnel: w49 -> [w186]
    tunnel: w47 -> [w185]
    tunnel: w18 -> [w183]
    stop <- w188 stop-if-true
    # "Attenuator ref"
    # "State Machine"
    n66 = Wait (ms)(milliseconds to wait=u32 100) -> ()  [unwired: 1 out]
    n67 = event shown="[19] \"Min power\": Mouse Down" {
      selector: _ -> [_ _ _ _ _ _ _ _ _ _ _ _ _ _ _ _ _ _ _ _ _ _ _ _ _ _ _ _ _ _ _ _ _ _ _ _ _ _ _ _ _ _ _]
      dyn-events: _ -> [_ _ _ _ _ _ _ _ _ _ _ _ _ _ _ _ _ _ _ _ _ _ _ _ _ _ _ _ _ _ _ _ _ _ _ _ _ _ _ _ _ _ _]
      timeout: 0 -> [_ _ _ _ _ _ _ _ _ _ _ _ _ _ _ _ _ _ _ _ _ _ _ _ _ _ _ _ _ _ _ _ _ _ _ _ _ _ _ _ _ _ _]
      tunnel: [w203 _ _ _ _ _ _ _ _ _ _ _ _ _ _ _ _ _ _ _ _ _ _ _ _ _ _ _ _ _ _ _ _ _ _ _ _ _ _ _ _ _ _] -> w200
      tunnel: w199 -> [w209 w249 w923 _ _ _ _ _ _ _ _ _ _ w1325 w1417 w1509 w1630 _ _ _ _ _ _ _ _ _ _ _ w1854 _ w1916 w2013 _ _ w2040 _ _ _ w2116 w2134 w2150 w2177 _]
      tunnel: w198 -> [_ _ _ _ _ _ _ _ _ _ _ _ _ _ _ _ _ _ _ _ _ _ _ _ w1819 _ _ _ _ _ _ _ _ _ _ _ _ _ _ _ _ _ _]
      tunnel: [_ _ _ _ _ _ _ _ _ _ _ _ _ _ _ _ _ _ _ _ _ _ _ _ w1819 _ _ _ _ _ _ _ _ _ _ _ _ _ _ _ _ _ _] -> _
      tunnel: w197 -> [w202 w248 w925 w951 w1049 w1091 w1124 w1153 w1200 w1271 w1287 w1297 w1320 w1326 w1418 w1510 w1631 w1724 w1747 w1761 w1764 w1768 w1795 w1798 w1814 w1840 _ _ w1857 w1909 w1915 w2015 w2028 w2031 w2047 w2084 w2095 w2098 w2118 w2136 w2152 w2176 w2269]
      tunnel: [w205 w244 w924 w952 w1050 w1088 w1121 w1156 w1199 w1271 w1287 w1297 w1320 w1327 w1419 w1511 w1632 w1724 w1746 w1761 w1764 w1769 w1795 w1798 w1805 w1840 _ _ w1856 w1909 w1912 w2014 w2028 w2031 w2047 w2084 w2095 w2096 w2117 w2135 w2151 w2172 w2269] -> w189
      tunnel: w196 -> [_ w242 _ _ _ _ _ _ w1197 _ _ _ _ w1323 w1415 w1506 w1629 _ _ w1763 w1767 _ _ _ _ _ _ _ _ _ _ _ _ _ _ _ _ _ _ _ _ _ _]
      tunnel: w195 -> [_ w240 _ _ _ _ _ w1154 _ _ _ _ _ _ _ w1508 _ w1727 _ _ _ _ _ _ _ _ _ _ _ _ _ _ _ _ _ _ _ _ _ _ _ _ _]
      tunnel: w194 -> [_ w241 _ _ _ _ _ w1155 _ _ _ _ _ _ _ w1507 _ w1726 _ _ _ _ _ _ _ _ _ _ _ _ _ _ _ _ _ _ _ _ _ _ _ _ _]
      tunnel: w185 -> [_ _ _ w956 w1054 _ _ _ _ _ _ _ _ _ _ _ _ _ _ _ _ _ _ _ _ _ _ _ _ _ _ _ _ _ _ _ _ _ _ _ _ _ _]
      tunnel: w192 -> [_ _ _ w954 w1052 _ _ _ _ _ _ _ _ _ _ _ _ _ _ _ _ _ _ _ _ _ _ _ _ _ _ _ _ _ _ _ _ _ _ _ _ _ _]
      tunnel: [_ _ _ w953 w1051 _ _ _ _ _ _ _ _ _ _ _ _ _ _ _ _ _ _ _ _ _ _ _ _ _ _ _ _ _ _ _ _ _ _ _ _ _ _] -> w191
      tunnel: w190 -> [_ _ _ _ _ _ _ _ _ _ _ _ _ _ _ _ _ _ w1751 _ _ _ _ _ _ _ _ _ _ _ _ _ _ _ _ _ _ _ _ _ _ _ _]
      tunnel: [_ _ _ _ _ _ _ _ _ _ _ _ _ _ _ _ _ _ w1749 _ _ _ _ _ _ _ _ _ _ _ _ _ _ _ _ _ _ _ _ _ _ _ _] -> w187
      tunnel: w186 -> [_ _ _ _ _ _ _ _ _ _ _ _ _ _ _ _ _ _ w1748 _ _ _ _ _ _ _ _ _ _ _ _ _ _ _ _ _ _ _ _ _ _ _ _]
      tunnel: [_ _ _ _ _ _ _ _ _ _ _ _ _ _ _ _ _ _ _ _ _ _ _ _ _ _ _ _ _ _ _ _ _ _ _ _ _ _ _ _ _ _ "stop"] -> w184
      tunnel: w183 -> [_ w237 _ _ _ w1090 w1123 _ _ _ _ _ _ w1324 w1416 _ _ _ _ _ _ _ _ _ _ _ _ _ _ _ _ _ _ _ _ _ _ _ _ _ _ _ _]
      event Timeout {
        # "Update positions and\npower indicators on the\nfront panel."
        # "This subVI provides a \"contrail\" for the dither bulls-eye"
        # "Check if piezo motion is underway,\neither from a commanded move\nor the gradient search."
        n68 = event-data() -> ()  [unwired: 1 in, 3 out]
        n69 = call "POS?.vi"("System no."=w209, "All axes?"=TRUE, "error in"=w202) -> ("Position"=w203:dbl[], "error out"=w210:errorcluster)  [unwired: 2 in, 13 out]
        n70 = local read "Analog Input"() -> (w208:i32)
        n71 = call "TCI?.vi"("System no."=w209, "Board"=w208, "error in"=w210) -> ("Calculated analog value"=→"Intensity":dbl, "error out"=w207:errorcluster)  [unwired: 15 in]
        n72 = First Call?() -> (First Call?: T/F=w214:bool)
        n73 = local write "Position"(w203) -> ()
        n74 = Index Array(array=w203, index=0) -> (element=w217:dbl)
        n75 = Index Array(array=w203, index=1) -> (element=w216:dbl)
        n76 = call "#5.vi"("System no."=w209, "error in"=w207) -> ("Axis moving?"=w228:bool[], "error out"=w223:errorcluster)  [unwired: 16 out]
        n77 = call "FRP?.vi"("System no."=w209, "Routines to query"=string[] ["2"], "error in"=w223) -> ("Status"=w224:i32[], "error out"=w205:errorcluster)  [unwired: 15 in]
        n78 = Equal?(x=w224, y=2) -> (x = y?=w226:bool[])
        n79 = case shown="False" w214 {
          tunnel: w203 -> [_ w232]
          frame False {
          }
          frame True {
            # "Set position targets\nto currrent positions\non first run for \nconvenience"
            n80 = Index Array(array=w232, index=0) -> (element=w230:dbl)
            n81 = Index Array(array=w232, index=1) -> (element=w229:dbl)
            n82 = Index Array(array=w232, index=2) -> (element=w231:dbl)
            n83 = local write "X"(w230) -> ()
            n84 = local write "Z"(w231) -> ()
            n85 = local write "Y"(w229) -> ()
          }
        }
        n86 = Build Array(w217, w216) -> (w215:dbl[])
        n87 = Or Array Elements(Boolean array=w226) -> (logical OR=w204:bool)
        n88 = Or Array Elements(Boolean array=w228) -> (logical OR=w221:bool)
        n89 = call "FMPA Feed Bullseye.vi"("Perfect circle XY bulls-eye"=cluster{dbl[], dbl[]} {[], []}, "Perfect circle?"=FALSE, "Init?"=w214, "POS array"=w215) -> ("Input XY bulls-eye"=w211:cluster{dbl[], dbl[]})  [unwired: 7 in]
        n90 = local write "NanoCube tracking"(w211) -> ()
        n91 = Or(x=w221, y=w204) -> (x .or. y?=→"Motion":bool)
      }
      event "EMITTER RUNTHROUGH": Value Change {
        n92 = event-data() -> ("CtlRef"=w246:refnum<vi>, "NewVal"=w247:bool)  [unwired: 1 in, 4 out]
        n93 = case shown="False" "Scan area override" {
          tunnel: [w250 w251] -> w245
          frame False {
            n94 = local read "Default 70x70um scan"() -> (w250:dbl[][])
          }
          frame True {
            n95 = local read "User Selected Measurement Points"() -> (w251:dbl[][])
          }
        }
        n96 = case shown="True" w247 {
          tunnel: [w254 w256] -> w244
          tunnel: w248 -> [w254 w264]
          tunnel: w249 -> [_ w263]
          tunnel: w246 -> [w253 w265]
          tunnel: [w253 w265] -> w243
          tunnel: w245 -> [_ w257]
          tunnel: w242 -> [_ w262]
          tunnel: w241 -> [_ w261]
          tunnel: w240 -> [_ w260]
          tunnel: [FALSE ("Value") FALSE ("Value")] -> w238
          tunnel: w237 -> [_ w258]
          frame False {
          }
          frame True {
            n97 = for {
              tunnel: w263 -> [w305]
              tunnel: w257 -> [w321] mode=indexing
              shift-right: [w303] -> w255
              shift-left: w264 -> [w323]
              tunnel: w262 -> [w320]
              tunnel: w261 -> [w319]
              tunnel: w260 -> [w318]
              tunnel: w258 -> [w309]
              stop <- w308 stop-if-true
              n98 = for {
                N: w325 -> [_]
                tunnel: w324 -> [w441]
                tunnel: w305 -> [w446]
                shift-right: [w460] -> _
                shift-left: w327 -> [w419]
                shift-right: [w417] -> w303
                shift-left: w322 -> [w450]
                shift-right: [w454] -> _
                shift-left: w326 -> [w443]
                tunnel: w307 -> [w445]
                tunnel: w306 -> [w444]
                tunnel: w320 -> [w453]
                tunnel: w313 -> [w452]
                tunnel: w310 -> [w451]
                tunnel: w309 -> [w448]
                tunnel: ["Stop Autoscan"] -> w308
                tunnel: w304 -> [w421]
                tunnel: w270 -> [w414]
                i -> [w440]
                stop <- "Stop Autoscan" stop-if-true
                # "TCSPC"
                # "TCSPC DLL path"
                n99 = local read "Mesh"() -> (w442:dbl)
                n100 = local write "Record counts"(FALSE ("Record stab")) -> ()
                n101 = control-ref of="Autoscan Status"() -> (w438:refnum<vi>)
                n102 = control-ref of="Alignment Graph"() -> (w433:refnum<vi>)
                n103 = control-ref of="Scan Termination"() -> (w432:refnum<vi>)
                n104 = Bundle("System no."=w446, "Xoffset"=w445, "Yoffset"=w444, "Array"=w443, "Mesh"=w442, "cent"=w441, "Numeric"=w419) -> (w439:T15)  [unwired: 1 in]
                n105 = control-ref of="Empty memory"() -> (w434:refnum<vi>)
                n106 = control-ref of="Record counts"() -> (w428:refnum<vi>)
                n107 = control-ref of="Motion"() -> (w429:refnum<vi>)
                n108 = local read "Measurement Save Path"() -> (w420:path)
                n109 = local read "Current Angle"() -> (w415:sgl)
                n110 = control-ref of="X"() -> (w437:refnum<vi>)
                n111 = control-ref of="Y"() -> (w436:refnum<vi>)
                n112 = control-ref of="Emitter #"() -> (w435:refnum<vi>)
                n113 = control-ref of="Z"() -> (w431:refnum<vi>)
                n114 = control-ref of="Z range"() -> (w430:refnum<vi>)
                n115 = control-ref of="TraceData"() -> (w425:refnum<vi>)
                n116 = local read "stop"() -> (w458:bool)
                n117 = call "Autoscan_CheckEmitter.vi"("String in"=w438, "reference 5"=w434, "IntGraph Refnum"=w433, "reference 6"=w432, "reference 7"=w431, "reference 8"=w430, "reference 9"=w429, "error in (no error)"=w450, "reference 4"=w435, "reference 10"=w428, "reference 3"=w436, "reference 11"=w425, "reference in"=w437, "lowerbright"="Lower Counts Threshold", "upperbright"="Upper Counts Theshold", "Numeric in"=w440, "Cluster"=w439) -> ("Autoscan Emitter Position"=w418:dbl[], "Array"=w454:dbl[][], "Emitter # out"=w459:i32, "Boolean"=w457:bool, "Ystored"=→"Ystored":dbl, "Zstored"=→"Zstored":dbl, "Xstored"=→"Xstored":dbl, "error out"=w449:errorcluster)  [unwired: 2 in, 1 out]
                n118 = Bundle("Measurement Save Path"=w420, "Autoscan Emitter Position"=w418, "Current Angle"=w415, "Filename Note"=w414) -> (w416:T16)  [unwired: 1 in]
                n119 = Not(x=w458) -> (.not. x?=w456:bool)
                n120 = And(x=w456, y=w457) -> (x .and. y?=w455:bool)
                n121 = case shown="True" w455 {
                  tunnel: w449 -> [w472 w486]
                  tunnel: w446 -> [w471 w485]
                  tunnel: w459 -> [w467 w488]
                  tunnel: [w467 w487] -> w461
                  tunnel: w453 -> [_ w484]
                  tunnel: w452 -> [_ w475]
                  tunnel: w451 -> [_ w483]
                  tunnel: [w465 w482] -> w417
                  tunnel: [0.0 w479] -> _
                  tunnel: [w463 w480] -> _
                  tunnel: [w463 w481] -> _
                  tunnel: w448 -> [_ w478]
                  tunnel: w421 -> [_ w477]
                  tunnel: w416 -> [_ w476]
                  frame False {
                    w463 = 1.5
                    n122 = local write "Record counts"(FALSE ("Record stab")) -> ()
                    n123 = local read "Zstored"() -> (w468:dbl)
                    n124 = local write "Z"(w468) -> ()
                    n125 = local read "X"() -> (w470:dbl)
                    n126 = local read "Y"() -> (w469:dbl)
                    n127 = Build Array(w470, w469, w468) -> (w473:dbl[])
                    n128 = call "MOV.vi"("System no."=w471, "Axes to move"=string[] ["1", "2", "3"], "Position values"=w473, "error in"=w472) -> ("error out"=w465:errorcluster)  [unwired: 1 in, 14 out]
                  }
                  frame True {
                    # "emitter #"
                    n129 = stacked-sequence {
                      seq-local: [w491 _ _ _ _ _ _] -> [_ _ _ _ _ w811 w909]
                      tunnel: w486 -> [w491 _ _ _ _ _ _]
                      tunnel: w488 -> [_ w528 _ _ _ _ w910]
                      tunnel: [_ _ _ _ _ _ w910] -> w487
                      tunnel: w485 -> [_ _ _ _ _ w821 _]
                      tunnel: w484 -> [_ _ _ _ _ w814 _]
                      tunnel: w475 -> [w493 w521 _ _ w728 w813 w906]
                      tunnel: w483 -> [w492 w520 _ _ w727 w812 w905]
                      tunnel: [_ _ _ _ _ w808 _] -> w482
                      tunnel: [0.0 _ _ _ _ _ _] -> w481
                      tunnel: [_ _ 0.0 ("CW g2") _ _ _ _] -> w480
                      tunnel: [_ w539 _ _ _ _ _] -> w479
                      tunnel: w478 -> [_ _ w612 w667 _ _ _]
                      tunnel: w477 -> [_ w524 w605 w665 _ w809 w907]
                      tunnel: w476 -> [_ w523 w606 w666 w723 w810 w908]
                      tunnel: [_ _ _ _ _ _ w908] -> _
                      tunnel: [_ _ _ _ _ _ w907] -> _
                      frame #0 {
                        (unwired) 0.0 ("element")
                        # "PI stage"
                        n130 = Build Array(0.0 ("element"), 0.0 ("element")) -> (→"drift vect.":dbl[])
                        n131 = local read "Measure counts on PDMs?"() -> (w489:bool)
                        n132 = flat-sequence {
                          tunnel: w493 -> [w500]
                          tunnel: w492 -> [w499]
                          tunnel: w489 -> [w498]
                          frame #0 {
                            # "PI stage"
                            n133 = case shown="False" w498 {
                              tunnel: w500 -> [w503 w511]
                              tunnel: w499 -> [w502 w510]
                              frame True {
                                # "TCSPC"
                                # "TCSPC"
                                # "set for PDMs"
                                n134 = Wait (ms)(milliseconds to wait=u32 800) -> ()  [unwired: 1 out]
                                n135 = invoke class="FilterFlipper" method="SetPosition"(reference=w503, "position"=u32 2, "waitTimeout"=0) -> ()  [unwired: 2 in, 5 out]
                                n136 = invoke class="FilterFlipper" method="SetPosition"(reference=w502, "position"=u32 2, "waitTimeout"=0) -> ()  [unwired: 2 in, 5 out]
                                n137 = local write "Autoscan Status"("Mirrors: PDMs") -> ()
                              }
                              frame False {
                                # "set for SPCM"
                                n138 = Wait (ms)(milliseconds to wait=u32 800) -> ()  [unwired: 1 out]
                                n139 = invoke class="FilterFlipper" method="SetPosition"(reference=w511, "position"=u32 2, "waitTimeout"=0) -> ()  [unwired: 2 in, 5 out]
                                n140 = invoke class="FilterFlipper" method="SetPosition"(reference=w510, "position"=u32 1, "waitTimeout"=0) -> ()  [unwired: 2 in, 5 out]
                                n141 = local write "Autoscan Status"("Mirrors: SPCM") -> ()
                              }
                            }
                            n142 = local write "Empty memory"(TRUE ("Empty memory")) -> ()
                          }
                          frame #1 {
                            n143 = call "Time Delay4"() -> ()  [unwired: 11 in, 1 out]
                          }
                        }
                      }
                      frame #1 {
                        n144 = flat-sequence {
                          tunnel: ["Autoscan Stability Time (s)"] -> w538
                          tunnel: w528 -> [w543]
                          tunnel: [w543] -> w527
                          tunnel: [w547] -> w537
                          tunnel: w538 -> [w548]
                          tunnel: [w548] -> w535
                          tunnel: [w547] -> w532
                          tunnel: [w546] -> w530
                          tunnel: w527 -> [w545]
                          tunnel: [w545] -> w526
                          tunnel: w537 -> [w564]
                          tunnel: [w564] -> w536
                          tunnel: w535 -> [w563]
                          tunnel: [w563] -> w534
                          tunnel: [w561] -> w533
                          tunnel: w532 -> [w560]
                          tunnel: [w560] -> w531
                          tunnel: w530 -> [w559]
                          tunnel: [w559] -> w529
                          tunnel: w526 -> [w558]
                          tunnel: [w558] -> w525
                          tunnel: w536 -> [w574]
                          tunnel: w534 -> [w573]
                          tunnel: w533 -> [w572]
                          tunnel: w531 -> [w571]
                          tunnel: w529 -> [w565]
                          tunnel: w525 -> [w568]
                          tunnel: w524 -> [w567]
                          tunnel: w523 -> [w566]
                          tunnel: [w574] -> w522
                          tunnel: [w565] -> w517
                          tunnel: w522 -> [w594]
                          tunnel: w521 -> [w589]
                          tunnel: w520 -> [w588]
                          tunnel: [w594] -> w519
                          tunnel: [w586] -> w518
                          tunnel: w517 -> [w586]
                          tunnel: [w596] -> w539
                          tunnel: w519 -> [w596]
                          tunnel: w518 -> [w595]
                          frame #0 {
                            n145 = local write "Autoscan Status"("Measuring stability" ("Autoscan Status")) -> ()
                            n146 = local write "Record counts"(TRUE ("Record stab")) -> ()
                            n147 = local write "Empty memory"(FALSE ("Empty memory")) -> ()
                          }
                          frame #1 {
                            n148 = call "Time Delay6"("Delay Time (s)"="Autoscan Stability Time (s)") -> ()  [unwired: 10 in, 1 out]
                          }
                          frame #2 {
                            n149 = local write "Record counts"(FALSE ("Record stab")) -> ()
                            n150 = local read "TraceData"() -> (w546:dbl[][])
                            n151 = local write "TraceDataStab"(w546) -> ()
                            n152 = Index Array(array=w546, index (col)=1) -> (element=w552:dbl[])  [unwired: 1 in]
                            n153 = Array Subset(array=w552, index=60) -> (w553:dbl[])  [unwired: 1 in]
                            n154 = call <vilib>:"Std Deviation and Variance.vi"("X"=w553) -> ("mean"=w554:dbl, "standard deviation"=w555:dbl)  [unwired: 1 in, 1 out]
                            n155 = Divide(x=w555, y=w554) -> (x/y=w547:dbl)
                            n156 = local write "StabilityRMS"(w547) -> ()
                          }
                          frame #3 {
                            n157 = local write "Empty memory"(TRUE ("Empty memory")) -> ()
                            n158 = control-ref of="Laser power (uW)"() -> (w562:refnum<vi>)
                            n159 = call "Quick Laser Power Log.vi"("Digital in"=w562) -> ("Numeric"=w561:dbl)  [unwired: 9 in, 1 out]
                            n160 = local write "Laser Pwr Save Var"(w561) -> ()
                            n161 = local write "Autoscan Status"("Saving stability" ("Current Measurement")) -> ()
                          }
                          frame #4 {
                            n162 = local read "RMS Cutoff"() -> (w570:dbl)
                            n163 = Less Or Equal?(x=w571, y=w570) -> (x <= y?=w569:bool)
                            n164 = case shown="True" w569 {
                              tunnel: w573 -> [_ w585]
                              tunnel: w572 -> [_ w584]
                              tunnel: w565 -> [_ w583]
                              tunnel: w568 -> [_ _]
                              tunnel: w567 -> [_ w581]
                              tunnel: w566 -> [_ w579]
                              frame False {
                              }
                              frame True {
                                n165 = Unbundle(w579) -> ("Measurement Save Path"=w578:path, "Autoscan Emitter Position"=w577:dbl[], "Current Angle"=w576:sgl, "Filename Note"=w575:string)
                                n166 = call "Save Measurement File.vi"("Measurement Save Path"=w578, "Measurement Type"=MeasurementType."Stability", "Data in (if 2D)"=w583, "ND angle"=w576, "Position"=w577, "integration time"=w585, "Filename Note"=w575, "Filter"=w581, "Prevent Save Dialog Prompt?"=TRUE, "laser power"=w584) -> ()  [unwired: 10 in]
                              }
                            }
                          }
                          frame #5 {
                            # "TCSPC"
                            # "set for PDMs"
                            n167 = invoke class="FilterFlipper" method="SetPosition"(reference=w589, "position"=u32 2, "waitTimeout"=0) -> ()  [unwired: 2 in, 5 out]
                            n168 = invoke class="FilterFlipper" method="SetPosition"(reference=w588, "position"=u32 2, "waitTimeout"=0) -> ()  [unwired: 2 in, 5 out]
                            n169 = local write "Autoscan Status"("Mirrors: PDMs" ("Current Measurement")) -> ()
                          }
                          frame #6 {
                            n170 = disable-structure shown="Disabled" {
                              disable-tunnel: w595 -> [w598 _]
                              frame Disabled {
                                # "delete all but first row"
                                n171 = Array Size(array=w598) -> (size(s)=w604:i32[])
                                n172 = Subtract(x=w604, y=1) -> (x-y=w602:i32[])
                                n173 = Index Array(array=w602, index=0) -> (element=w600:i32)
                                n174 = Delete From Array(array=w598, length=w600, index (row)=1) -> (array with subset deleted=w597:dbl[][])  [unwired: 1 in, 1 out]
                                n175 = local write "TraceData"(w597) -> ()
                              }
                              frame Enabled {
                              }
                            }
                          }
                        }
                      }
                      frame #2 {
                        # "PI Stage"
                        # "TCSPC"
                        n176 = local read "StabilityRMS"() -> (w609:dbl)
                        n177 = local read "RMS Cutoff"() -> (w608:dbl)
                        n178 = Less Or Equal?(x=w609, y=w608) -> (x <= y?=w610:bool)
                        n179 = And(x="g2", y=w610) -> (x .and. y?=w607:bool)
                        n180 = case shown="True" w607 {
                          tunnel: w612 -> [_ w625]
                          tunnel: w606 -> [_ w624]
                          tunnel: w605 -> [_ w623]
                          frame False {
                          }
                          frame True {
                            n181 = flat-sequence {
                              tunnel: w625 -> [w637]
                              tunnel: [w633] -> w622
                              tunnel: [w632] -> w620
                              tunnel: [w631] -> w618
                              tunnel: [w630] -> w616
                              tunnel: w622 -> [w650]
                              tunnel: [w650] -> w621
                              tunnel: w620 -> [w649]
                              tunnel: [w649] -> w619
                              tunnel: w618 -> [w648]
                              tunnel: [w648] -> w617
                              tunnel: w616 -> [w647]
                              tunnel: [w647] -> w615
                              tunnel: [w645] -> w614
                              tunnel: w624 -> [w664]
                              tunnel: w621 -> [w663]
                              tunnel: w619 -> [w662]
                              tunnel: w623 -> [w661]
                              tunnel: w617 -> [w660]
                              tunnel: w615 -> [w659]
                              tunnel: w614 -> [w658]
                              frame #0 {
                                n182 = case shown="True" "g2 window" {
                                frame True {
                                w628 = T5 2 items=["Lifetime (80 MHz, 12.5 ns)", "Lifetime (20 MHz, 50 ns)", "g2 (50 ns)", "g2 (300 ns)"] ("Correlation measurement")
                                n183 = local write "Correlation measurement"(w628) -> ()
                                }
                                frame False {
                                w629 = T5 3 items=["Lifetime (80 MHz, 12.5 ns)", "Lifetime (20 MHz, 50 ns)", "g2 (50 ns)", "g2 (300 ns)"] ("Correlation measurement")
                                # "Adjust shutter here"
                                n184 = local write "Correlation measurement"(w629) -> ()
                                }
                                }
                                n185 = call "Time Delay3"() -> ()  [unwired: 11 in, 1 out]
                                n186 = local write "Autoscan Status"("Measuring g2") -> ()
                              }
                              frame #1 {
                                n187 = local read "ADC Resolution [exponent]"() -> (w634:T1)
                                n188 = control-ref of="g2 time remaining"() -> (w642:refnum<vi>)
                                n189 = Unbundle(w637) -> ("SPCMemConfig"=w638:T10, "DLL Path"=w639:path, "Module No"=w640:i16, "Page"=w641:i32)
                                n190 = Unbundle By Name("g2 Auto Scan Settings") -> ("collect_time"=w632:sgl, "tac_range"=w630:sgl, "tac_gain"=w631:i16)
                                n191 = control-ref of="g2 abort"() -> (w643:refnum<vi>)
                                n192 = call "TCSPC Measure.vi"("DLL Path"=w639, "SPC Memory Config"=w638, "Module No"=w640, "Timer Refnum"=w642, "Page"=w641, "ADC Resolution (exponent)"=w634, "Abort Refnum"=w643, "User Input"="g2 Auto Scan Settings") -> ("Data"=w633:u16[], "x-scale multiplier"=w635:dbl)  [unwired: 4 in, 2 out]
                                n193 = property on="g2 data" class="WFGraph (strict)"("XScale.Multiplier"=w635) -> ()  [unwired: 2 in, 2 out]
                                n194 = property on="g2 time remaining" class="Knob (strict)"("Scale.Maximum"=w632) -> ()  [unwired: 2 in, 2 out]
                                n195 = local write "g2 data"(w633) -> ()
                              }
                              frame #2 {
                                n196 = control-ref of="Laser power (uW)"() -> (w646:refnum<vi>)
                                n197 = call "Quick Laser Power Log.vi"("Digital in"=w646) -> ("Numeric"=w645:dbl)  [unwired: 9 in, 1 out]
                                n198 = local write "Autoscan Status"("Saving g2") -> ()
                              }
                              frame #3 {
                                n199 = Unbundle(w664) -> ("Measurement Save Path"=w657:path, "Autoscan Emitter Position"=w656:dbl[], "Current Angle"=w655:sgl, "Filename Note"=w651:string)
                                n200 = local read "ADC Resolution [exponent]"() -> (w652:T1)
                                n201 = call "Save Measurement File.vi"("Measurement Save Path"=w657, "Measurement Type"=MeasurementType."g2", "Data in (if 1D)"=w663, "ND angle"=w655, "tac"=w659, "Position"=w656, "gain"=w660, "integration time"=w662, "bins"=w652, "Filename Note"=w651, "Filter"=w661, "Prevent Save Dialog Prompt?"=TRUE, "laser power"=w658) -> ()  [unwired: 7 in]
                              }
                            }
                          }
                        }
                      }
                      frame #3 {
                        # "Measure Lifetime"
                        n202 = local read "StabilityRMS"() -> (w671:dbl)
                        n203 = local read "RMS Cutoff"() -> (w670:dbl)
                        n204 = local read "Lifetime"() -> (w668:bool)
                        n205 = Less Or Equal?(x=w671, y=w670) -> (x <= y?=w672:bool)
                        n206 = And(x=w668, y=w672) -> (x .and. y?=w669:bool)
                        n207 = case shown="True" w669 {
                          tunnel: w667 -> [_ w684]
                          tunnel: w666 -> [_ w682]
                          tunnel: w665 -> [_ w681]
                          frame False {
                          }
                          frame True {
                            n208 = flat-sequence {
                              tunnel: w684 -> [w696]
                              tunnel: [w692] -> w679
                              tunnel: [w691] -> w678
                              tunnel: [w690] -> w676
                              tunnel: [w689] -> w674
                              tunnel: [w707] -> w683
                              tunnel: [w706] -> w680
                              tunnel: w679 -> [w706]
                              tunnel: w678 -> [w705]
                              tunnel: [w705] -> w677
                              tunnel: w676 -> [w704]
                              tunnel: [w704] -> w675
                              tunnel: w674 -> [w703]
                              tunnel: [w703] -> w673
                              tunnel: w683 -> [w722]
                              tunnel: w682 -> [w721]
                              tunnel: w681 -> [w717]
                              tunnel: w680 -> [w715]
                              tunnel: w677 -> [w714]
                              tunnel: w675 -> [w712]
                              tunnel: w673 -> [w711]
                              frame #0 {
                                n209 = call "Time Delay8"() -> ()  [unwired: 11 in, 1 out]
                                n210 = case shown="True" "lifetime window" {
                                frame False {
                                w687 = T5 1 items=["Lifetime (80 MHz, 12.5 ns)", "Lifetime (20 MHz, 50 ns)", "g2 (50 ns)", "g2 (300 ns)"] ("Correlation measurement")
                                n211 = local write "Correlation measurement"(w687) -> ()
                                }
                                frame True {
                                w688 = T5 1 items=["Lifetime (80 MHz, 12.5 ns)", "Lifetime (20 MHz, 50 ns)", "g2 (50 ns)", "g2 (300 ns)"] ("Correlation measurement")
                                n212 = local write "Correlation measurement"(w688) -> ()
                                }
                                }
                                n213 = local write "Autoscan Status"("Measuring lifetime") -> ()
                              }
                              frame #1 {
                                n214 = local read "ADC Resolution [exponent]"() -> (w693:T1)
                                n215 = Unbundle By Name(w696) -> ("SPCMemConfig"=w699:T10, "DLL Path"=w700:path, "Module No"=w701:i16, "Page"=w702:i32)
                                n216 = control-ref of="Lifetime time remaining"() -> (w698:refnum<vi>)
                                n217 = Unbundle By Name("Lifetime Auto Scan Settings") -> ("collect_time"=w689:sgl, "tac_range"=w692:sgl, "tac_gain"=w691:i16)
                                n218 = control-ref of="Lifetime abort"() -> (w697:refnum<vi>)
                                n219 = call "TCSPC Measure.vi"("DLL Path"=w700, "SPC Memory Config"=w699, "Module No"=w701, "Timer Refnum"=w698, "Page"=w702, "ADC Resolution (exponent)"=w693, "Abort Refnum"=w697, "User Input"="Lifetime Auto Scan Settings") -> ("Data"=w690:u16[], "x-scale multiplier"=w694:dbl)  [unwired: 4 in, 2 out]
                                n220 = property on="Lifetime time remaining" class="Knob (strict)"("Scale.Maximum"=w689) -> ()  [unwired: 2 in, 2 out]
                                n221 = local write "lifetime data"(w690) -> ()
                                n222 = property on="lifetime data" class="WFGraph (strict)"("XScale.Multiplier"=w694) -> ()  [unwired: 2 in, 2 out]
                              }
                              frame #2 {
                                n223 = control-ref of="Laser power (uW)"() -> (w708:refnum<vi>)
                                n224 = call "Quick Laser Power Log.vi"("Digital in"=w708) -> ("Numeric"=w707:dbl)  [unwired: 9 in, 1 out]
                              }
                              frame #3 {
                                n225 = local read "ADC Resolution [exponent]"() -> (w716:T1)
                                n226 = Unbundle(w721) -> ("Measurement Save Path"=w720:path, "Autoscan Emitter Position"=w719:dbl[], "Current Angle"=w718:sgl, "Filename Note"=w709:string)
                                n227 = call "Save Measurement File.vi"("Measurement Save Path"=w720, "Measurement Type"=MeasurementType."Lifetime", "Data in (if 1D)"=w712, "ND angle"=w718, "tac"=w715, "Position"=w719, "gain"=w714, "integration time"=w711, "bins"=w716, "Filename Note"=w709, "Filter"=w717, "Prevent Save Dialog Prompt?"=TRUE, "laser power"=w722) -> ()  [unwired: 7 in]
                              }
                            }
                          }
                        }
                      }
                      frame #4 {
                        n228 = local read "StabilityRMS"() -> (w730:dbl)
                        n229 = local read "RMS Cutoff"() -> (w729:dbl)
                        n230 = Less Or Equal?(x=w730, y=w729) -> (x <= y?=w725:bool)
                        n231 = And(x="Spectrum", y=w725) -> (x .and. y?=w724:bool)
                        n232 = case shown="True" w724 {
                          tunnel: w728 -> [_ w755]
                          tunnel: w727 -> [_ w754]
                          tunnel: w723 -> [_ w734]
                          frame False {
                          }
                          frame True {
                            n233 = flat-sequence {
                              tunnel: w755 -> [w779]
                              tunnel: w754 -> [w778]
                              tunnel: [w781] -> w753
                              tunnel: [w780] -> w752
                              tunnel: w753 -> [w790]
                              tunnel: w752 -> [w789]
                              tunnel: [w790] -> w751
                              tunnel: [w789] -> w750
                              tunnel: [w806] -> w756
                              tunnel: [w807] -> w757
                              tunnel: w751 -> [w807]
                              tunnel: w750 -> [w806]
                              tunnel: w749 -> [w805]
                              tunnel: w748 -> [w804]
                              tunnel: w747 -> [w803]
                              tunnel: w746 -> [w802]
                              tunnel: w745 -> [w801]
                              tunnel: w744 -> [w800]
                              tunnel: w743 -> [w799]
                              tunnel: w742 -> [w798]
                              tunnel: 0 -> [w797]
                              tunnel: w740 -> [w796]
                              tunnel: [w795] -> w739
                              tunnel: [w794] -> w738
                              tunnel: [w793] -> w737
                              tunnel: [w792] -> w732
                              tunnel: [w791] -> w736
                              frame #0 {
                                # "set for spectrometer"
                                n234 = invoke class="FilterFlipper" method="SetPosition"(reference=w779, "position"=u32 1, "waitTimeout"=0) -> (reference out=w781:refnum<k24>)  [unwired: 2 in, 4 out]
                                n235 = invoke class="FilterFlipper" method="SetPosition"(reference=w778, "position"=u32 1, "waitTimeout"=0) -> (reference out=w780:refnum<k24>)  [unwired: 2 in, 4 out]
                                n236 = Wait (ms)(milliseconds to wait=1500) -> ()  [unwired: 1 out]
                                n237 = local write "Autoscan Status"("Mirrors: Spectrometer") -> ()
                              }
                              frame #1 {
                                n238 = local write "Autoscan Status"("Measuring Spectrum...") -> ()
                                n239 = Wait (ms)(milliseconds to wait=10) -> ()  [unwired: 1 out]
                              }
                              frame #2 {
                                n240 = call "OceanOpticsRecordSpectra.vi"("Boxcar Width"=w805, "Scans to Average"=w804, "EDC Enable"=w803, "NLC Enable"=w802, "lampOn"=w801, "N Integrations"=w800, "Int. Time (microsec)"=w799, "lampOn 2"=w798, "Spectrometer Index"=w797, "enable"=w796) -> ("getName"=w795:string, "getSerialNumber"=w794:string, "XY Graph"=w793:cluster{"Y":dbl[], "Y":dbl[]}[], "Array"=w792:dbl[][], "error out"=w791:errorcluster)  [unwired: 5 in]
                              }
                            }
                            n241 = local read "Scans to Average"() -> (w748:i32)
                            n242 = local read "N Integrations"() -> (w744:i32)
                            n243 = local read "Boxcar Width"() -> (w749:i32)
                            n244 = local read "EDC Enable"() -> (w747:i32)
                            n245 = local read "NLC Enable"() -> (w746:i32)
                            n246 = Multiply(x="Autoscan Spectrum Time (s)", y=1000000) -> (x*y=w743:i32)
                            n247 = local read "lampOn 2"() -> (w742:i32)
                            n248 = local read "lampOn"() -> (w745:i32)
                            n249 = local read "enable"() -> (w740:i16)
                            n250 = flat-sequence {
                              tunnel: w736 -> [w761]
                              tunnel: w757 -> [_]
                              tunnel: w756 -> [_]
                              tunnel: [w760] -> w735
                              tunnel: [w759] -> w731
                              tunnel: [w776] -> _
                              tunnel: w735 -> [w776]
                              tunnel: w734 -> [w774]
                              tunnel: "Autoscan Spectrum Time (s)" -> [w775]
                              tunnel: w732 -> [w773]
                              tunnel: w731 -> [w772]
                              frame #0 {
                                # "set for PDMs"
                                n251 = control-ref of="Laser power (uW)"() -> (w762:refnum<vi>)
                                n252 = Wait (ms)(milliseconds to wait=1000) -> ()  [unwired: 1 out]
                                n253 = call "Quick Laser Power Log.vi"("error in (no error)"=w761, "Digital in"=w762) -> ("error out"=w760:errorcluster, "Numeric"=w759:dbl)  [unwired: 8 in]
                              }
                              frame #1 {
                                n254 = local write "Autoscan Status"("Saving spectrum") -> ()
                                n255 = local write "Empty memory"(TRUE ("Empty memory")) -> ()
                                n256 = Unbundle(w774) -> ("Measurement Save Path"=w768:path, "Autoscan Emitter Position"=w771:dbl[], "Current Angle"=w770:sgl, "Filename Note"=w765:string)
                                n257 = call "Save Measurement File.vi"("Measurement Save Path"=w768, "Measurement Type"=MeasurementType."Spectrum", "Data in (if 2D)"=w773, "ND angle"=w770, "Position"=w771, "integration time"=w775, "Filename Note"=w765, "Prevent Save Dialog Prompt?"=TRUE, "laser power"=w772) -> ()  [unwired: 11 in]
                              }
                            }
                            n258 = local write "Spectrometer Name:"(w739) -> ()
                            n259 = local write "Serial Number:"(w738) -> ()
                            n260 = local write "Spectrum"(w737) -> ()
                            n261 = local write "spectrum output"(w732) -> ()
                          }
                        }
                      }
                      frame #5 {
                        n262 = local read "StabilityRMS"() -> (w818:dbl)
                        n263 = local read "RMS Cutoff"() -> (w817:dbl)
                        n264 = local read "Saturation"() -> (w819:bool)
                        n265 = local read "Scan Termination"() -> (w820:T6)
                        n266 = Less Or Equal?(x=w818, y=w817) -> (x <= y?=w816:bool)
                        n267 = And(x=w819, y=w816) -> (x .and. y?=w815:bool)
                        n268 = case shown="True" w815 {
                          tunnel: [w822 w844] -> w808
                          tunnel: w821 -> [_ w829]
                          tunnel: w820 -> [_ w828]
                          tunnel: w814 -> [_ w831]
                          tunnel: w813 -> [_ w827]
                          tunnel: w812 -> [_ w826]
                          tunnel: w811 -> [w822 w825]
                          tunnel: w810 -> [_ w824]
                          tunnel: w809 -> [_ w823]
                          frame False {
                          }
                          frame True {
                            n269 = flat-sequence {
                              tunnel: [w848] -> w830
                              tunnel: w828 -> [_]
                              tunnel: w829 -> [_]
                              tunnel: w825 -> [w848]
                              tunnel: w826 -> [w846]
                              tunnel: w827 -> [w847]
                              tunnel: w830 -> [w865]
                              tunnel: [w870] -> w840
                              tunnel: [w869] -> w838
                              tunnel: [w868] -> w834
                              tunnel: w831 -> [w867]
                              tunnel: [w875] -> w841
                              tunnel: w840 -> [w875]
                              tunnel: [w874] -> w839
                              tunnel: w838 -> [w874]
                              tunnel: [w873] -> w835
                              tunnel: w834 -> [w873]
                              tunnel: [w885] -> w842
                              tunnel: w841 -> [w885]
                              tunnel: w839 -> [w884]
                              tunnel: [w883] -> w836
                              tunnel: w835 -> [w882]
                              tunnel: [w881] -> w832
                              tunnel: [w897] -> w843
                              tunnel: w842 -> [w897]
                              tunnel: [w896] -> w837
                              tunnel: w836 -> [w896]
                              tunnel: [w895] -> w833
                              tunnel: w832 -> [w895]
                              tunnel: w824 -> [w893]
                              tunnel: w823 -> [w888]
                              tunnel: [w899] -> w844
                              tunnel: w843 -> [w901]
                              tunnel: w837 -> [w902]
                              tunnel: w833 -> [w900]
                              frame #0 {
                                n270 = local read "Measure counts on PDMs?"() -> (w845:bool)
                                n271 = case shown="False" w845 {
                                tunnel: w847 -> [w850 w858]
                                tunnel: w846 -> [w849 w857]
                                frame False {
                                n272 = invoke class="FilterFlipper" method="SetPosition"(reference=w850, "position"=u32 2, "waitTimeout"=0) -> ()  [unwired: 2 in, 5 out]
                                n273 = invoke class="FilterFlipper" method="SetPosition"(reference=w849, "position"=u32 1, "waitTimeout"=0) -> ()  [unwired: 2 in, 5 out]
                                n274 = Wait (ms)(milliseconds to wait=u32 550) -> ()  [unwired: 1 out]
                                n275 = local write "Autoscan Status"("Mirrors: SPCM") -> ()
                                }
                                frame True {
                                n276 = invoke class="FilterFlipper" method="SetPosition"(reference=w858, "position"=u32 2, "waitTimeout"=0) -> ()  [unwired: 2 in, 5 out]
                                n277 = invoke class="FilterFlipper" method="SetPosition"(reference=w857, "position"=u32 2, "waitTimeout"=0) -> ()  [unwired: 2 in, 5 out]
                                n278 = Wait (ms)(milliseconds to wait=u32 550) -> ()  [unwired: 1 out]
                                n279 = local write "Autoscan Status"("Mirrors: PDMs") -> ()
                                }
                                }
                              }
                              frame #1 {
                                n280 = local read "Saturation Start Angle"() -> (w871:dbl)
                                n281 = local write "Autoscan Status"("Saturation Initialization") -> ()
                                n282 = call "Saturation Start Sequence.vi"("error in (no error)"=w865, "Saturation Start Angle"=w871, "Rotation stage refnum"=w867) -> ("error out"=w868:errorcluster, "Rotation stage refnum out"=w869:refnum<k24>, "return position"=w870:dbl)
                              }
                              frame #2 {
                                n283 = local write "Empty memory"(FALSE ("Empty memory")) -> ()
                                n284 = local write "Record counts"(TRUE) -> ()
                                n285 = Wait (ms)(milliseconds to wait=200) -> ()  [unwired: 1 out]
                              }
                              frame #3 {
                                n286 = local read "Saturation Sweep Speed (deg/s)"() -> (w879:dbl)
                                n287 = local read "Saturation End Angle"() -> (w880:dbl)
                                n288 = local write "Autoscan Status"("Saturation Measuring...") -> ()
                                n289 = call "Saturation Move Sequence.vi"("error in (no error)"=w882, "Saturation Sweep Speed"=w879, "Saturation End Angle"=w880, ".NET Refnum in"=w884) -> ("error out"=w881:errorcluster, "reference out"=w883:refnum<k24>)
                              }
                              frame #4 {
                                # "save the data"
                                n290 = local read "TraceData"() -> (w886:dbl[][])
                                n291 = Wait (ms)(milliseconds to wait=u32 50) -> ()  [unwired: 1 out]
                                n292 = Unbundle(w893) -> ("Measurement Save Path"=w892:path, "Autoscan Emitter Position"=w891:dbl[], "Filename Note"=w887:string)  [unwired: 1 out]
                                n293 = local write "Saturation Array"(w886) -> ()
                                n294 = call "Save Measurement File.vi"("Measurement Save Path"=w892, "Measurement Type"=MeasurementType."Saturation", "Data in (if 2D)"=w886, "Position"=w891, "Filename Note"=w887, "Filter"=w888, "Prevent Save Dialog Prompt?"=TRUE) -> ()  [unwired: 13 in]
                              }
                              frame #5 {
                                n295 = local write "Record counts"(FALSE ("Record counts")) -> ()
                                n296 = call "Saturation Return or End Sequence.vi"("error in (no error)"=w900, "return position"=w901, ".NET Refnum in"=w902) -> ("error out"=w899:errorcluster)  [unwired: 7 in, 1 out]
                                n297 = local write "Empty memory"(TRUE ("Empty memory")) -> ()
                                n298 = local write "Autoscan Status"("Saturation Done.") -> ()
                              }
                            }
                          }
                        }
                      }
                      frame #6 {
                        n299 = flat-sequence {
                          tunnel: w906 -> [w912]
                          tunnel: w905 -> [w911]
                          frame #0 {
                            # "set for SPCM"
                            n300 = Wait (ms)(milliseconds to wait=u32 1000 ("millisecond timer value")) -> ()  [unwired: 1 out]
                            n301 = local write "Empty memory"(FALSE ("Laser Shutter")) -> ()
                            n302 = local write "Autoscan Status"("Emitter complete. Mirrors to SPCM " ("Current Measurement")) -> ()
                            n303 = invoke class="FilterFlipper" method="SetPosition"(reference=w912, "position"=u32 2, "waitTimeout"=0) -> ()  [unwired: 2 in, 5 out]
                            n304 = invoke class="FilterFlipper" method="SetPosition"(reference=w911, "position"=u32 1, "waitTimeout"=0) -> ()  [unwired: 2 in, 5 out]
                          }
                        }
                        n305 = flat-sequence {
                          tunnel: w909 -> [w922]
                          tunnel: [w922] -> _
                          frame #0 {
                            n306 = Wait (ms)(milliseconds to wait=u32 400) -> ()  [unwired: 1 out]
                            n307 = local write "Autoscan Status"("Data saved.") -> ()
                          }
                        }
                      }
                    }
                  }
                }
                n308 = Increment(x=w461) -> (x+1=w460:i32)
              }
              n309 = flat-sequence {
                tunnel: [w340] -> w315
                tunnel: [w339] -> w314
                tunnel: [w336] -> w310
                tunnel: [w335] -> w313
                tunnel: w305 -> [w340]
                tunnel: w321 -> [w339]
                tunnel: w318 -> [w334]
                tunnel: w319 -> [w333]
                tunnel: w323 -> [w331]
                tunnel: [w330] -> w311
                tunnel: [w328] -> w271
                tunnel: [w328] -> w270
                tunnel: [w347] -> w317
                tunnel: [w346] -> w316
                tunnel: w315 -> [w347]
                tunnel: w314 -> [w346]
                tunnel: [w343] -> w312
                tunnel: w311 -> [w343]
                tunnel: [w342] -> w304
                tunnel: [w342] -> _
                tunnel: [w342] -> w302
                tunnel: [w341] -> w272
                tunnel: w271 -> [w341]
                tunnel: w317 -> [w361]
                tunnel: w316 -> [w354]
                tunnel: w312 -> [w356]
                tunnel: [w367] -> w301
                tunnel: [w366] -> w299
                tunnel: [w364] -> w297
                tunnel: [w355] -> w295
                tunnel: [w363] -> w293
                tunnel: [w362] -> w291
                tunnel: [w360] -> w289
                tunnel: [w354] -> w287
                tunnel: [w353] -> w285
                tunnel: [w352] -> w283
                tunnel: w302 -> [w352]
                tunnel: [w351] -> w281
                tunnel: [w350] -> w277
                tunnel: [w349] -> w275
                tunnel: [w348] -> w273
                tunnel: w272 -> [w348]
                tunnel: w301 -> [w385]
                tunnel: [w385] -> w300
                tunnel: w299 -> [w384]
                tunnel: [w384] -> w298
                tunnel: w297 -> [w383]
                tunnel: [w383] -> w296
                tunnel: w295 -> [w382]
                tunnel: [w382] -> w294
                tunnel: w293 -> [w381]
                tunnel: [w381] -> w292
                tunnel: w291 -> [w380]
                tunnel: [w380] -> w290
                tunnel: w289 -> [w373]
                tunnel: [w372] -> w288
                tunnel: w287 -> [w379]
                tunnel: [w379] -> w286
                tunnel: w285 -> [w378]
                tunnel: [w378] -> w284
                tunnel: w283 -> [w377]
                tunnel: [w377] -> w282
                tunnel: w281 -> [w376]
                tunnel: [w376] -> w280
                tunnel: [w374] -> w279
                tunnel: [w371] -> w278
                tunnel: w277 -> [w371]
                tunnel: [w370] -> w276
                tunnel: w275 -> [w370]
                tunnel: [w368] -> w274
                tunnel: w273 -> [w368]
                tunnel: [w407] -> w322
                tunnel: [w408] -> w306
                tunnel: [w409] -> w307
                tunnel: [w410] -> w324
                tunnel: [w411] -> w325
                tunnel: [w412] -> w326
                tunnel: [w413] -> w327
                tunnel: w300 -> [w413]
                tunnel: w298 -> [w412]
                tunnel: w296 -> [w411]
                tunnel: w294 -> [w410]
                tunnel: w292 -> [w409]
                tunnel: w290 -> [w408]
                tunnel: w288 -> [w407]
                tunnel: w286 -> [w404]
                tunnel: w284 -> [w401]
                tunnel: w282 -> [w387]
                tunnel: w280 -> [w394]
                tunnel: w279 -> [w392]
                tunnel: [w391] -> _
                tunnel: w278 -> [w389]
                tunnel: w276 -> [w388]
                tunnel: w274 -> [w386]
                frame #0 {
                  n310 = control-ref of="Autoscan Status"() -> (w338:refnum<vi>)
                  n311 = control-ref of="Motion"() -> (w337:refnum<vi>)
                  n312 = local read "Filename Note"() -> (w328:string)
                  n313 = call "Autoscan_MirrorsToSPCM.vi"("Device 4"=w333, "reference 3"=w338, "reference 2"=w337, ".NET Refnum in"=w334) -> ("Device"=w336:refnum<k24>, ".NET Refnum out"=w335:refnum<k24>)  [unwired: 6 in]
                  n314 = property on="EMITTER RUNTHROUGH" class="Bool (strict)"(error in=w331, "DisabledEnum"=T8."Disabled and Grayed Out" ("Disabled")) -> (error out=w330:errorcluster)  [unwired: 1 in, 1 out]
                  n315 = local write "Autoscan Status"("Laser on.") -> ()
                }
                frame #1 {
                  n316 = Wait (ms)(milliseconds to wait=u32 10) -> ()  [unwired: 1 out]
                  n317 = local write "Autoscan Status"("Scanning...") -> ()
                  n318 = property on="Filter Configuraton" class="Ring (strict)"() -> ("RingText.Text"=w342:string)  [unwired: 2 in, 2 out]
                }
                frame #2 {
                  n319 = control-ref of="Intensity Graph"() -> (w358:refnum<vi>)
                  n320 = local read "Upper contrast threshold"() -> (w359:dbl)
                  n321 = local read "Lower contrast threshold"() -> (w365:dbl)
                  n322 = local read "X Range"() -> (w350:dbl)
                  n323 = local read "Y Range"() -> (w349:dbl)
                  n324 = local read "Mesh"() -> (w351:dbl)
                  n325 = call "PlotIntensityGraph.vi"("IntensityGraph in"=w358, "System no."=w361, "Mesh"=w351, "Lower thr"=w365, "X Scan Range"=w350, "error in (no error)"=w356, "Map centers"=w354, "Y Scan Range"=w349, "Upper thr"=w359) -> ("Xoffset"=w363:dbl, "Yoffset"=w362:dbl, "Plot Images:Front"=w357:picture, "Array"=w366:dbl[][], "cent"=w355:i32[][], "Numeric"=w367:i32, "Intensity Graph"=w353:dbl[][], "Nemitters"=w364:i32, "error out"=w360:errorcluster)  [unwired: 2 in]
                  n326 = local write "cent"(w355) -> ()
                  n327 = local write "Emitter #"(w367) -> ()
                  n328 = local write "Intensity Graph"(w353) -> ()
                  n329 = local write "# of Emitters"(w364) -> ()
                  n330 = property on="Intensity Graph" class="IntGraph (strict)"("PlotImages.Front"=w357) -> ()  [unwired: 2 in, 2 out]
                }
                frame #3 {
                  n331 = control-ref of="Laser power (uW)"() -> (w375:refnum<vi>)
                  n332 = local write "Autoscan Status"("Saving PL Scan" ("Current Measurement")) -> ()
                  n333 = call "Quick Laser Power Log.vi"("error in (no error)"=w373, "Digital in"=w375) -> ("error out"=w372:errorcluster, "Numeric"=w374:dbl)  [unwired: 8 in]
                }
                frame #4 {
                  n334 = Index Array(array=w404, index=0) -> (element=w402:dbl)
                  n335 = Index Array(array=w404, index=1) -> (element=w403:dbl)
                  n336 = Multiply(x=w401, y=1000.0) -> (x*y=w399:dbl[][])
                  n337 = local read "Measurement Save Path"() -> (w396:path)
                  n338 = Round To Nearest(number=w399) -> (nearest integer value=w398:dbl[][])
                  n339 = local read "Current Angle"() -> (w393:sgl)
                  n340 = To Word Integer(number=w398) -> (16bit integer=w397:i16[][])
                  n341 = invoke on="Intensity Graph" class="IntGraph (strict)" method="Get Image"() -> ("image data"=w391:T17)  [unwired: 6 in, 5 out]
                  n342 = call "Save Measurement File.vi"("Measurement Save Path"=w396, "Measurement Type"=MeasurementType."PL Map", "Data in (if 2D)"=w397, "mesh"=w394, "ND angle"=w393, "x center"=w402, "y center"=w403, "Filename Note"=w386, "Filter"=w387, "x range"=w389, "y range"=w388, "Prevent Save Dialog Prompt?"=TRUE, "image data"=w391, "laser power"=w392) -> ()  [unwired: 6 in]
                }
              }
            }
            n343 = flat-sequence {
              tunnel: [w266] -> w256
              tunnel: w255 -> [w268]
              frame #0 {
                n344 = local write "Autoscan Status"("Autoscan exited." ("Current Measurement")) -> ()
                n345 = property on="EMITTER RUNTHROUGH" class="Bool (strict)"(error in=w268, "DisabledEnum"=T8."Enabled" ("Disabled")) -> (error out=w266:errorcluster)  [unwired: 1 in, 1 out]
              }
            }
          }
        }
        n346 = local write "Autoscan Status"("Initializing...") -> ()
        n347 = property class="Bool (strict)"(reference=w243, "Value"=w238) -> ()  [unwired: 1 in, 2 out]
      }
      event "AUTO XY SCAN": Value Change {
        n348 = event-data() -> ("CtlRef"=w928:refnum<vi>, "NewVal"=w929:bool)  [unwired: 1 in, 4 out]
        n349 = case shown="True" w929 {
          tunnel: w928 -> [w930 w946]
          tunnel: [w930 w946] -> w927
          tunnel: w925 -> [w931 w939]
          tunnel: [w931 w940] -> w924
          tunnel: w923 -> [_ w938]
          frame False {
          }
          frame True {
            n350 = flat-sequence {
              tunnel: w939 -> [w947]
              tunnel: [w947] -> w932
              frame #0 {
                n351 = local write "Motion"(TRUE ("Motion")) -> ()
              }
            }
            n352 = local read "Lower contrast threshold"() -> (w943:dbl)
            n353 = local read "X Range"() -> (w936:dbl)
            n354 = local read "Y Range"() -> (w935:dbl)
            n355 = local read "Mesh"() -> (w934:dbl)
            n356 = call "AUTOFLIM_AutoScan.vi"("X Scan Center"=55.0, "System#"=w938, "Mesh"=w934, "Y Scan Center"=55.0, "Lower Thr"=w943, "error in (no error)"=w932, "X Scan Range"=w936, "Y Scan Range"=w935) -> ("Intensity Graph"=w941:dbl[][], "Nemitters"=w942:i32, "cent"=w933:i32[][], "error out"=w940:errorcluster)  [unwired: 2 in, 2 out]
            n357 = local write "# of Emitters"(w942) -> ()
            n358 = local write "Intensity Graph"(w941) -> ()
            n359 = local write "cent"(w933) -> ()
            n360 = call "AUTOFLIM_Draw_emitters.vi"("Y Scan Range"=w935, "X Scan Range"=w936, "Mesh"=w934, "cent"=w933) -> ("Plot Images:Front"=w937:picture)  [unwired: 6 in, 1 out]
            n361 = property on="Intensity Graph" class="IntGraph (strict)"("PlotImages.Front"=w937) -> ()  [unwired: 2 in, 2 out]
          }
        }
        n362 = property class="Bool (strict)"(reference=w927, "Value"=FALSE) -> ()  [unwired: 1 in, 2 out]
      }
      event Value Change {
        n363 = event-data() -> ()  [unwired: 1 in, 5 out]
        n364 = case shown="0, Default" "Correlation measurement" {
          tunnel: [TRUE FALSE FALSE FALSE] -> w960
          tunnel: [FALSE FALSE FALSE TRUE] -> w961
          tunnel: [FALSE FALSE TRUE FALSE] -> w962
          tunnel: [FALSE TRUE FALSE FALSE] -> w963
          frame 0, Default {
            n365 = Bundle By Name(cluster=T4 {"tac_range"=50.033573, "tac_gain"=4, "tac_offset"=6.0, "tac_limit_high"=97.0, "tac_limit_low"=3.0, "collect_time"=5.0, "sync_threshold"=-50.980392, "sync_zc_level"=-5.2913384, "sync_freq_div"=1, "cfd_limit_low"=-50.980392, "cfd_zc_level"=-5.2999988} ("Lifetime settings"), "tac_range"=sgl 50.0, "tac_gain"=i16 4, "tac_offset"=sgl 6.0, "tac_limit_high"=sgl 97.0, "tac_limit_low"=sgl 3.0, "collect_time"=sgl 5.0, "sync_threshold"=sgl -51.0, "sync_zc_level"=sgl -5.3, "sync_freq_div"=i16 1, "cfd_limit_low"=sgl -51.0, "cfd_zc_level"=sgl -5.3) -> (w978:T4)
            n366 = local write "Lifetime settings"(w978) -> ()
          }
          frame 1 {
            n367 = Bundle By Name(cluster=T4 {"tac_range"=50.033573, "tac_gain"=4, "tac_offset"=6.0, "tac_limit_high"=97.0, "tac_limit_low"=3.0, "collect_time"=5.0, "sync_threshold"=-50.980392, "sync_zc_level"=-5.2913384, "sync_freq_div"=1, "cfd_limit_low"=-50.980392, "cfd_zc_level"=-5.2999988} ("Lifetime settings"), "tac_range"=sgl 50.0, "tac_gain"=i16 1, "tac_offset"=sgl 8.0, "tac_limit_high"=sgl 97.0, "tac_limit_low"=sgl 3.0, "collect_time"=sgl 5.0, "sync_threshold"=sgl -51.0, "sync_zc_level"=sgl -5.3, "sync_freq_div"=i16 1, "cfd_limit_low"=sgl -51.0, "cfd_zc_level"=sgl -5.3) -> (w993:T4)
            n368 = local write "Lifetime settings"(w993) -> ()
          }
          frame 2 {
            n369 = Bundle By Name(cluster=T4 {"tac_range"=50.033573, "tac_gain"=4, "tac_offset"=6.0, "tac_limit_high"=97.0, "tac_limit_low"=3.0, "collect_time"=5.0, "sync_threshold"=-50.980392, "sync_zc_level"=-5.2913384, "sync_freq_div"=1, "cfd_limit_low"=-50.980392, "cfd_zc_level"=-5.2999988} ("Lifetime settings"), "tac_range"=sgl 50.0, "tac_gain"=i16 1, "tac_offset"=sgl 6.0, "tac_limit_high"=sgl 97.0, "tac_limit_low"=sgl 3.0, "collect_time"=sgl 5.0, "sync_threshold"=sgl -51.0, "sync_zc_level"=sgl -5.3, "sync_freq_div"=i16 1, "cfd_limit_low"=sgl -51.0, "cfd_zc_level"=sgl -5.3) -> (w1010:T4)
            n370 = local write "g2 settings"(w1010) -> ()
          }
          frame 3 {
            n371 = Bundle By Name(cluster=T4 {"tac_range"=50.033573, "tac_gain"=4, "tac_offset"=6.0, "tac_limit_high"=97.0, "tac_limit_low"=3.0, "collect_time"=5.0, "sync_threshold"=-50.980392, "sync_zc_level"=-5.2913384, "sync_freq_div"=1, "cfd_limit_low"=-50.980392, "cfd_zc_level"=-5.2999988} ("Lifetime settings"), "tac_range"=sgl 300.0, "tac_gain"=i16 1, "tac_offset"=sgl 6.0, "tac_limit_high"=sgl 97.0, "tac_limit_low"=sgl 3.0, "collect_time"=sgl 5.0, "sync_threshold"=sgl -51.0, "sync_zc_level"=sgl -5.3, "sync_freq_div"=i16 1, "cfd_limit_low"=sgl -51.0, "cfd_zc_level"=sgl -5.3) -> (w1027:T4)
            n372 = local write "g2 settings"(w1027) -> ()
          }
        }
        n373 = local read "Laser Shutter"() -> (w950:bool)
        n374 = local read "Laser Shutter"() -> (w969:bool)
        n375 = Not(x=w969) -> ()  [unwired: 1 out]
        n376 = Not(x=w950) -> (.not. x?=w949:bool)
        n377 = Boolean Array To Number(Boolean array=w954) -> (number=w955:u32)
        n378 = Not(x="PDM 2 on/off") -> (.not. x?=w967:bool)
        n379 = Not(x="PDM 1 on/off") -> (.not. x?=w968:bool)
        n380 = Build Array(w967, w968, w963, w962, w961, w960, w949) -> (w964:bool[])
        n381 = Boolean Array To Number(Boolean array=w964) -> (number=w958:u32)
        n382 = Not Equal?(x=w955, y=w958) -> (x != y?=w959:bool)
        n383 = case shown="True" w959 {
          tunnel: [w971 w973] -> w953
          tunnel: w956 -> [_ w975]
          tunnel: [w970 w974] -> w952
          tunnel: w964 -> [w971 w973]
          tunnel: w951 -> [w970 w972]
          frame False {
          }
          frame True {
            n384 = call-poly <vilib>:"DAQmx Write.vi"("task/channels in"=w975, "data"=w973, "error in"=w972) -> ("error out"=w974:errorcluster)  [unwired: 10 in, 2 out]
          }
        }
      }
      event "PDM 1 on/off", "PDM 2 on/off", "Laser Shutter": Value Change {
        n385 = event-data() -> ()  [unwired: 1 in, 5 out]
        n386 = local read "Correlation measurement"() -> (w1048:T5)
        n387 = case shown="0, Default" w1048 {
          tunnel: [TRUE FALSE FALSE FALSE] -> w1057
          tunnel: [FALSE FALSE FALSE TRUE] -> w1058
          tunnel: [FALSE FALSE TRUE FALSE] -> w1059
          tunnel: [FALSE TRUE FALSE FALSE] -> w1060
          frame 0, Default {
          }
          frame 1 {
          }
          frame 2 {
          }
          frame 3 {
          }
        }
        n388 = local read "Laser Shutter"() -> (w1045:bool)
        n389 = local read "Laser Shutter"() -> (w1064:bool)
        n390 = Not(x=w1064) -> ()  [unwired: 1 out]
        n391 = Not(x=w1045) -> (.not. x?=w1044:bool)
        n392 = local read "PDM 1 on/off"() -> (w1047:bool)
        n393 = local read "PDM 2 on/off"() -> (w1046:bool)
        n394 = Boolean Array To Number(Boolean array=w1052) -> (number=w1053:u32)
        n395 = Not(x=w1047) -> (.not. x?=w1062:bool)
        n396 = Not(x=w1046) -> (.not. x?=w1063:bool)
        n397 = Build Array(w1062, w1063, w1060, w1059, w1058, w1057, w1044) -> (w1061:bool[])
        n398 = Boolean Array To Number(Boolean array=w1061) -> (number=w1055:u32)
        n399 = Not Equal?(x=w1053, y=w1055) -> (x != y?=w1056:bool)
        n400 = case shown="True" w1056 {
          tunnel: [w1066 w1068] -> w1051
          tunnel: w1054 -> [_ w1070]
          tunnel: [w1065 w1069] -> w1050
          tunnel: w1061 -> [w1066 w1068]
          tunnel: w1049 -> [w1065 w1067]
          frame False {
          }
          frame True {
            n401 = call-poly <vilib>:"DAQmx Write.vi"("task/channels in"=w1070, "data"=w1068, "error in"=w1067) -> ("error out"=w1069:errorcluster)  [unwired: 10 in, 2 out]
          }
        }
      }
      event "Measure g2": Value Change {
        n402 = event-data() -> ("NewVal"=w1092:bool)  [unwired: 1 in, 5 out]
        n403 = case shown="True" w1092 {
          tunnel: [w1098 w1112] -> w1089
          tunnel: w1091 -> [w1098 w1108]
          tunnel: w1090 -> [_ w1119]
          frame False {
          }
          frame True {
            n404 = local read "ADC Resolution [exponent]"() -> (w1099:T1)
            n405 = Unbundle By Name("g2 settings") -> ("collect_time"=w1105:sgl)
            n406 = property on="g2 time remaining" class="Knob (strict)"(error in=w1108, "Scale.Maximum"=w1105) -> (error out=w1107:errorcluster)  [unwired: 1 in, 1 out]
            n407 = property on="Measure g2" class="Bool (strict)"(error in=w1107, "DisabledEnum"=T8."Disabled and Grayed Out" ("Disabled")) -> (error out=w1113:errorcluster)  [unwired: 1 in, 1 out]
            n408 = control-ref of="g2 data"() -> (w1104:refnum<vi>)
            n409 = Unbundle(w1119) -> ("SPCMemConfig"=w1118:T10, "DLL Path"=w1117:path, "Module No"=w1116:i16, "Page"=w1115:i32)
            n410 = control-ref of="g2 time remaining"() -> (w1114:refnum<vi>)
            n411 = control-ref of="g2 abort"() -> (w1102:refnum<vi>)
            n412 = call "TCSPC Measure.vi"("DLL Path"=w1117, "SPC Memory Config"=w1118, "Module No"=w1116, "Timer Refnum"=w1114, "Page"=w1115, "ADC Resolution (exponent)"=w1099, "Abort Refnum"=w1102, "Error In"=w1113, "User Input"="g2 settings") -> ("Data"=→"g2 data":u16[], "x-scale multiplier"=w1103:dbl, "Error Out"=w1101:errorcluster)  [unwired: 3 in, 1 out]
            n413 = property class="WFGraph (strict)"(reference=w1104, error in=w1101, "XScale.Multiplier"=w1103) -> (error out=w1100:errorcluster)  [unwired: 1 out]
            n414 = property on="Measure g2" class="Bool (strict)"(error in=w1100, "DisabledEnum"=T8."Enabled" ("Disabled")) -> (error out=w1112:errorcluster)  [unwired: 1 in, 1 out]
          }
        }
        n415 = flat-sequence {
          tunnel: [w1095] -> w1087
          tunnel: w1089 -> [w1095]
          tunnel: [w1097] -> w1088
          tunnel: w1087 -> [w1097]
          frame #0 {
            n416 = control-ref of="Laser power (uW)"() -> (w1094:refnum<vi>)
            n417 = call "Quick Laser Power Log.vi"("Digital in"=w1094) -> ("Numeric"=w1093:dbl)  [unwired: 9 in, 1 out]
            n418 = local write "Laser Pwr Save Var"(w1093) -> ()
          }
          frame #1 {
            n419 = local write "g2 abort"(FALSE ("g2 abort")) -> ()
          }
        }
      }
      event "Meaure lifetime": Value Change {
        # "DAQmx task"
        n420 = event-data() -> ("NewVal"=w1125:bool)  [unwired: 1 in, 5 out]
        n421 = case shown="True" w1125 {
          tunnel: w1124 -> [w1131 w1141]
          tunnel: [w1131 w1146] -> w1122
          tunnel: w1123 -> [_ w1151]
          frame False {
          }
          frame True {
            n422 = local read "ADC Resolution [exponent]"() -> (w1132:T1)
            n423 = Unbundle By Name("Lifetime settings") -> ("collect_time"=w1138:sgl)
            n424 = property on="Lifetime time remaining" class="Knob (strict)"(error in=w1141, "Scale.Maximum"=w1138) -> (error out=w1140:errorcluster)  [unwired: 1 in, 1 out]
            n425 = property on="Meaure lifetime" class="Bool (strict)"(error in=w1140, "DisabledEnum"=T8."Disabled and Grayed Out" ("Disabled")) -> (error out=w1145:errorcluster)  [unwired: 1 in, 1 out]
            n426 = control-ref of="Lifetime time remaining"() -> (w1142:refnum<vi>)
            n427 = Unbundle(w1151) -> ("SPCMemConfig"=w1147:T10, "DLL Path"=w1150:path, "Module No"=w1149:i16, "Page"=w1148:i32)
            n428 = control-ref of="lifetime data"() -> (w1137:refnum<vi>)
            n429 = control-ref of="Lifetime abort"() -> (w1135:refnum<vi>)
            n430 = call "TCSPC Measure.vi"("DLL Path"=w1150, "SPC Memory Config"=w1147, "Module No"=w1149, "Timer Refnum"=w1142, "Page"=w1148, "ADC Resolution (exponent)"=w1132, "Abort Refnum"=w1135, "Error In"=w1145, "User Input"="Lifetime settings") -> ("Data"=→"lifetime data":u16[], "x-scale multiplier"=w1136:dbl, "Error Out"=w1134:errorcluster)  [unwired: 3 in, 1 out]
            n431 = property class="WFGraph (strict)"(reference=w1137, error in=w1134, "XScale.Multiplier"=w1136) -> (error out=w1133:errorcluster)  [unwired: 1 out]
            n432 = property on="Meaure lifetime" class="Bool (strict)"(error in=w1133, "DisabledEnum"=T8."Enabled" ("Disabled")) -> (error out=w1146:errorcluster)  [unwired: 1 in, 1 out]
          }
        }
        n433 = flat-sequence {
          tunnel: w1122 -> [w1128]
          tunnel: [w1128] -> w1120
          tunnel: [w1130] -> w1121
          tunnel: w1120 -> [w1130]
          frame #0 {
            n434 = control-ref of="Laser power (uW)"() -> (w1126:refnum<vi>)
            n435 = call "Quick Laser Power Log.vi"("Digital in"=w1126) -> ("Numeric"=→"Laser Pwr Save Var":dbl)  [unwired: 9 in, 1 out]
          }
          frame #1 {
            n436 = local write "Lifetime abort"(FALSE ("Lifetime abort")) -> ()
          }
        }
      }
      event "Measure spectrum": Value Change {
        n437 = event-data() -> ("NewVal"=w1157:bool)  [unwired: 1 in, 5 out]
        n438 = case shown="True" w1157 {
          tunnel: w1153 -> [w1158 w1172]
          tunnel: [w1158 w1161] -> w1156
          tunnel: w1155 -> [_ w1167]
          tunnel: w1154 -> [_ w1166]
          frame False {
          }
          frame True {
            n439 = flat-sequence {
              tunnel: [w1195] -> w1163
              tunnel: w1172 -> [w1195]
              tunnel: w1167 -> [w1190]
              tunnel: w1166 -> [w1189]
              frame #0 {
                n440 = invoke class="FilterFlipper" method="SetPosition"(reference=w1189, "position"=u32 1, "waitTimeout"=0) -> ()  [unwired: 2 in, 5 out]
                n441 = invoke class="FilterFlipper" method="SetPosition"(reference=w1190, "position"=u32 1, "waitTimeout"=0) -> ()  [unwired: 2 in, 5 out]
                n442 = Wait (ms)(milliseconds to wait=u32 550 ("millisecond timer value")) -> ()  [unwired: 1 out]
              }
            }
            n443 = local read "Spectrum Integration Time (s)"() -> (w1171:i32)
            n444 = property on="Measure spectrum" class="Bool (strict)"(error in=w1163, "DisabledEnum"=T8."Disabled and Grayed Out" ("Disabled")) -> (error out=w1162:errorcluster)  [unwired: 1 in, 1 out]
            n445 = local read "Scans to Average"() -> (w1181:i32)
            n446 = local read "N Integrations"() -> (w1178:i32)
            n447 = local read "Boxcar Width"() -> (w1182:i32)
            n448 = Multiply(x=w1171, y=1000000) -> (x*y=w1170:i32)
            n449 = local read "EDC Enable"() -> (w1175:i32)
            n450 = local read "NLC Enable"() -> (w1180:i32)
            n451 = local read "lampOn 2"() -> (w1179:i32)
            n452 = local read "lampOn"() -> (w1183:i32)
            n453 = Round To Nearest(number=w1170) -> (nearest integer value=w1169:i32)
            n454 = local read "enable"() -> (w1177:i16)
            n455 = call "OceanOpticsRecordSpectra.vi"("Boxcar Width"=w1182, "Scans to Average"=w1181, "EDC Enable"=w1175, "NLC Enable"=w1180, "error in (no error)"=w1162, "lampOn"=w1183, "N Integrations"=w1178, "Int. Time (microsec)"=w1169, "lampOn 2"=w1179, "Spectrometer Index"=0, "enable"=w1177) -> ("getName"=w1173:string, "getSerialNumber"=w1174:string, "XY Graph"=w1185:cluster{"Y":dbl[], "Y":dbl[]}[], "Array"=w1184:dbl[][], "error out"=w1160:errorcluster)  [unwired: 4 in]
            n456 = local write "Spectrometer Name:"(w1173) -> ()
            n457 = local write "Serial Number:"(w1174) -> ()
            n458 = local write "Spectrum"(w1185) -> ()
            n459 = local write "spectrum output"(w1184) -> ()
            n460 = flat-sequence {
              tunnel: w1160 -> [w1188]
              tunnel: [w1188] -> w1159
              frame #0 {
                n461 = control-ref of="Laser power (uW)"() -> (w1186:refnum<vi>)
                n462 = call "Quick Laser Power Log.vi"("Digital in"=w1186) -> ("Numeric"=w1187:dbl)  [unwired: 9 in, 1 out]
                n463 = local write "Laser Pwr Save Var"(w1187) -> ()
              }
            }
            n464 = property on="Measure spectrum" class="Bool (strict)"(error in=w1159, "DisabledEnum"=T8."Enabled" ("Disabled")) -> (error out=w1161:errorcluster)  [unwired: 1 in, 1 out]
          }
        }
      }
      event "Measure saturation": Value Change {
        n465 = event-data() -> ("NewVal"=w1198:bool)  [unwired: 1 in, 5 out]
        n466 = case shown="True" w1198 {
          tunnel: w1200 -> [w1201 w1221]
          tunnel: [w1201 w1219] -> w1199
          tunnel: w1197 -> [_ w1220]
          frame False {
          }
          frame True {
            n467 = flat-sequence {
              tunnel: w1221 -> [w1225]
              tunnel: w1220 -> [w1229]
              tunnel: [w1228] -> w1216
              tunnel: [w1227] -> w1214
              tunnel: [w1226] -> w1212
              tunnel: [w1232] -> w1217
              tunnel: w1216 -> [w1232]
              tunnel: [w1236] -> w1215
              tunnel: w1214 -> [w1236]
              tunnel: [w1235] -> w1213
              tunnel: w1212 -> [w1235]
              tunnel: [w1241] -> w1218
              tunnel: w1217 -> [w1241]
              tunnel: w1215 -> [w1240]
              tunnel: w1213 -> [w1239]
              tunnel: [w1238] -> w1211
              tunnel: [w1237] -> w1210
              tunnel: [w1252] -> w1209
              tunnel: w1218 -> [w1252]
              tunnel: w1211 -> [w1247]
              tunnel: [w1244] -> w1207
              tunnel: w1210 -> [w1244]
              tunnel: [w1247] -> w1204
              tunnel: [w1244] -> w1202
              tunnel: w1209 -> [w1258]
              tunnel: [w1258] -> w1208
              tunnel: w1207 -> [w1257]
              tunnel: [w1257] -> w1206
              tunnel: [w1254] -> w1205
              tunnel: w1204 -> [w1254]
              tunnel: [w1253] -> w1203
              tunnel: w1202 -> [w1253]
              tunnel: [w1262] -> w1219
              tunnel: w1208 -> [w1264]
              tunnel: w1206 -> [_]
              tunnel: w1205 -> [w1260]
              tunnel: w1203 -> [w1259]
              frame #0 {
                n468 = property on="Measure saturation" class="Bool (strict)"(error in=w1225, "DisabledEnum"=T8."Disabled and Grayed Out" ("Disabled")) -> (error out=w1224:errorcluster)  [unwired: 1 in, 1 out]
                n469 = call "Saturation Start Sequence.vi"("error in (no error)"=w1224, "Saturation Start Angle"="Saturation Start Angle", "Rotation stage refnum"=w1229) -> ("error out"=w1226:errorcluster, "Rotation stage refnum out"=w1227:refnum<k24>, "return position"=w1228:dbl)
                n470 = local write "Empty memory"(TRUE ("Empty memory")) -> ()
              }
              frame #1 {
                n471 = local write "Record counts"(TRUE ("Record stab")) -> ()
                n472 = Wait (ms)(milliseconds to wait=u32 200) -> ()  [unwired: 1 out]
                n473 = local write "Empty memory"(FALSE ("Empty memory")) -> ()
              }
              frame #2 {
                n474 = call "Saturation Move Sequence.vi"("error in (no error)"=w1239, "Saturation Sweep Speed"="Saturation Sweep Speed (deg/s)", "Saturation End Angle"="Saturation End Angle", ".NET Refnum in"=w1240) -> ("error out"=w1238:errorcluster, "reference out"=w1237:refnum<k24>)
              }
              frame #3 {
                n475 = local read "Measurement Save Path"() -> (w1251:path)
                n476 = local read "Filename Note"() -> (w1248:string)
                n477 = local read "TraceData"() -> (w1250:dbl[][])
                n478 = local read "Position"() -> (w1249:dbl[])
                n479 = property on="Filter Configuraton" class="Ring (strict)"() -> ("RingText.Text"=w1245:string)  [unwired: 2 in, 2 out]
                n480 = call "Save Measurement File.vi"("Measurement Save Path"=w1251, "Measurement Type"=MeasurementType."Saturation", "Data in (if 2D)"=w1250, "Position"=w1249, "Filename Note"=w1248, "Filter"=w1245) -> ()  [unwired: 14 in]
              }
              frame #4 {
                n481 = local write "Record counts"(FALSE ("Record stab")) -> ()
                n482 = Wait (ms)(milliseconds to wait=u32 200) -> ()  [unwired: 1 out]
              }
              frame #5 {
                n483 = call "Saturation Return or End Sequence.vi"("error in (no error)"=w1260, "return position"=w1264, ".NET Refnum in"=w1259) -> ("error out"=w1263:errorcluster)  [unwired: 7 in, 1 out]
                n484 = property on="Measure saturation" class="Bool (strict)"(error in=w1263, "DisabledEnum"=T8."Enabled" ("Disabled")) -> (error out=w1262:errorcluster)  [unwired: 1 in, 1 out]
              }
            }
          }
        }
      }
      event "Write g2 to file": Mouse Down {
        n485 = event-data() -> ()  [unwired: 1 in, 8 out]
        n486 = local read "g2 settings"() -> (w1276:T4)
        n487 = local read "Measurement Save Path"() -> (w1277:path)
        n488 = local read "Filename Note"() -> (w1272:string)
        n489 = local read "Current Angle"() -> (w1278:sgl)
        n490 = Unbundle By Name(w1276) -> ("tac_range"=w1275:sgl, "tac_gain"=w1274:i16, "collect_time"=w1273:sgl)
        n491 = local read "g2 data"() -> (w1269:u16[])
        n492 = local read "Position"() -> (w1270:dbl[])
        n493 = local read "ADC Resolution [exponent]"() -> (w1265:T1)
        n494 = local read "Laser Pwr Save Var"() -> (w1268:dbl)
        n495 = property on="Filter Configuraton" class="Ring (strict)"() -> ("RingText.Text"=w1267:string)  [unwired: 2 in, 2 out]
        n496 = call "Save Measurement File.vi"("Measurement Save Path"=w1277, "Measurement Type"=MeasurementType."g2", "Data in (if 1D)"=w1269, "ND angle"=w1278, "tac"=w1275, "Position"=w1270, "gain"=w1274, "integration time"=w1273, "bins"=w1265, "Filename Note"=w1272, "Filter"=w1267, "laser power"=w1268) -> ()  [unwired: 8 in]
      }
      event "Write lifetime to file": Mouse Down {
        (unwired) 0 ("laser power")
        n497 = event-data() -> ()  [unwired: 1 in, 8 out]
        n498 = local read "Lifetime settings"() -> (w1290:T4)
        n499 = local read "lifetime data"() -> (w1283:u16[])
        n500 = local read "Measurement Save Path"() -> (w1292:path)
        n501 = local read "Filename Note"() -> (w1291:string)
        n502 = local read "Current Angle"() -> (w1284:sgl)
        n503 = Unbundle By Name(w1290) -> ("tac_range"=w1289:sgl, "tac_gain"=w1288:i16, "collect_time"=w1285:sgl)
        n504 = local read "Position"() -> (w1286:dbl[])
        n505 = local read "ADC Resolution [exponent]"() -> (w1279:T1)
        n506 = local read "Laser Pwr Save Var"() -> (w1282:dbl)
        n507 = property on="Filter Configuraton" class="Ring (strict)"() -> ("RingText.Text"=w1281:string)  [unwired: 2 in, 2 out]
        n508 = call "Save Measurement File.vi"("Measurement Save Path"=w1292, "Measurement Type"=MeasurementType."Lifetime", "Data in (if 1D)"=w1283, "ND angle"=w1284, "tac"=w1289, "Position"=w1286, "gain"=w1288, "integration time"=w1285, "bins"=w1279, "Filename Note"=w1291, "Filter"=w1281, "laser power"=w1282) -> ()  [unwired: 8 in]
      }
      event "Write spectrum to file": Mouse Down {
        (unwired) 0 ("number")
        n509 = event-data() -> ()  [unwired: 1 in, 8 out]
        n510 = local read "Spectrum Integration Time (s)"() -> (w1299:i32)
        n511 = local read "Measurement Save Path"() -> (w1301:path)
        n512 = local read "spectrum output"() -> (w1302:dbl[][])
        n513 = local read "Current Angle"() -> (w1300:sgl)
        n514 = local read "Filename Note"() -> (w1298:string)
        n515 = local read "Position"() -> (w1296:dbl[])
        n516 = local read "Laser Pwr Save Var"() -> (w1295:dbl)
        n517 = property on="Filter Configuraton" class="Ring (strict)"() -> ("RingText.Text"=w1293:string)  [unwired: 2 in, 2 out]
        n518 = call "Save Measurement File.vi"("Measurement Save Path"=w1301, "Measurement Type"=MeasurementType."Spectrum", "Data in (if 2D)"=w1302, "ND angle"=w1300, "Position"=w1296, "integration time"=w1299, "Filename Note"=w1298, "Filter"=w1293, "laser power"=w1295) -> ()  [unwired: 11 in]
      }
      event "Write PL map to file": Mouse Down {
        n519 = event-data() -> ()  [unwired: 1 in, 8 out]
        n520 = local read "Mesh"() -> (w1303:dbl)
        n521 = local read "Intensity Graph"() -> (w1317:dbl[][])
        n522 = flat-sequence {
          tunnel: [w1321] -> w1306
          frame #0 {
            n523 = control-ref of="Laser power (uW)"() -> (w1322:refnum<vi>)
            n524 = call "Quick Laser Power Log.vi"("Digital in"=w1322) -> ("Numeric"=w1321:dbl)  [unwired: 9 in, 1 out]
          }
        }
        n525 = local read "Measurement Save Path"() -> (w1314:path)
        n526 = Multiply(x=w1317, y=1000.0) -> (x*y=w1316:dbl[][])
        n527 = property on="Filter Configuraton" class="Ring (strict)"() -> ("RingText.Text"=w1308:string)  [unwired: 2 in, 2 out]
        n528 = local read "Filename Note"() -> (w1309:string)
        n529 = local read "Current Angle"() -> (w1310:sgl)
        n530 = Round To Nearest(number=w1316) -> (nearest integer value=w1319:dbl[][])
        n531 = local read "X Center"() -> (w1305:dbl)
        n532 = local read "Y Center"() -> (w1304:dbl)
        n533 = To Word Integer(number=w1319) -> (16bit integer=w1313:i16[][])
        n534 = invoke on="Intensity Graph" class="IntGraph (strict)" method="Get Image"() -> ("image data"=w1312:T17)  [unwired: 6 in, 5 out]
        n535 = local read "X Range"() -> (w1311:dbl)
        n536 = local read "Y Range"() -> (w1307:dbl)
        n537 = call "Save Measurement File.vi"("Measurement Save Path"=w1314, "Measurement Type"=MeasurementType."PL Map", "Data in (if 2D)"=w1313, "mesh"=w1303, "ND angle"=w1310, "x center"=w1305, "y center"=w1304, "Filename Note"=w1309, "Filter"=w1308, "x range"=w1311, "y range"=w1307, "image data"=w1312, "laser power"=w1306) -> ()  [unwired: 7 in]
      }
      event "Auto g2": Value Change {
        n538 = event-data() -> ("NewVal"=w1328:bool)  [unwired: 1 in, 5 out]
        n539 = case shown="True" w1328 {
          tunnel: w1326 -> [w1329 w1333]
          tunnel: [w1329 w1334] -> w1327
          tunnel: w1325 -> [_ w1345]
          tunnel: w1324 -> [_ w1337]
          tunnel: w1323 -> [_ w1330]
          frame False {
          }
          frame True {
            n540 = local read "User Selected Measurement Points"() -> (w1340:dbl[][])
            n541 = property on="Auto lifetime" class="Bool (strict)"(error in=w1333, "DisabledEnum"=T8."Disabled and Grayed Out" ("Disabled")) -> (error out=w1332:errorcluster)  [unwired: 1 in, 1 out]
            n542 = local read "Filter Positions"() -> (w1339:dbl[])
            n543 = Array Size(array=w1340) -> (size(s)=w1346:i32[])
            n544 = local read "Measurement Save Path"() -> (w1338:path)
            n545 = Array Size(array=w1339) -> (size(s)=w1344:i32)
            n546 = Index Array(array=w1346, index=0) -> (element=w1343:i32)
            n547 = Round To Nearest(number=w1343) -> (nearest integer value=w1342:i32)
            n548 = Round To Nearest(number=w1344) -> (nearest integer value=w1341:i32)
            n549 = for {
              N: w1342 -> [_]
              shift-right: [w1357] -> w1335
              shift-left: w1332 -> [w1356]
              tunnel: w1340 -> [w1355] mode=indexing
              tunnel: w1339 -> [w1354]
              tunnel: w1345 -> [w1353]
              tunnel: w1341 -> [w1352]
              tunnel: w1338 -> [w1351]
              tunnel: w1337 -> [w1350]
              tunnel: w1330 -> [w1348]
              stop <- w1349 stop-if-true
              n550 = for {
                N: w1352 -> [_]
                tunnel: w1355 -> [w1364]
                tunnel: w1354 -> [w1363] mode=indexing
                tunnel: w1353 -> [w1362]
                shift-right: [w1366] -> w1357
                shift-left: w1356 -> [w1365]
                tunnel: w1351 -> [w1361]
                tunnel: w1350 -> [w1360]
                tunnel: [w1358] -> w1349
                tunnel: w1348 -> [w1359]
                stop <- w1358 stop-if-true
                n551 = stacked-sequence {
                  seq-local: [_ _ w1380 _ _] -> [_ _ _ _ w1414]
                  seq-local: [_ _ w1390 _ _] -> [_ _ _ _ w1410]
                  seq-local: [_ _ _ w1399 _] -> [_ _ _ _ w1406]
                  tunnel: [w1372 _ _ _ _] -> w1366
                  tunnel: w1365 -> [_ w1378 w1385 w1400 _]
                  tunnel: w1364 -> [_ w1373 _ _ w1412]
                  tunnel: w1363 -> [w1369 _ _ _ w1413]
                  tunnel: w1362 -> [_ w1376 _ _ _]
                  tunnel: w1361 -> [_ _ _ _ w1411]
                  tunnel: w1360 -> [_ _ w1397 _ _]
                  tunnel: w1359 -> [w1370 _ _ _ _]
                  frame #0 {
                    # "Move rotation attenuator angle"
                    n552 = invoke class="KCubeDCServo" method="MoveTo"(reference=w1370, "position"=w1369, "waitTimeout"=0) -> (error out=w1368:errorcluster)  [unwired: 2 in, 4 out]
                    n553 = call "Time Delay7"("error in (no error)"=w1368, "Delay Time (s)"=5.0) -> ("error out"=w1372:errorcluster)  [unwired: 9 in]
                  }
                  frame #1 {
                    w1374 = string[] ["1", "2"]
                    n554 = call "MOV.vi"("System no."=w1376, "Axes to move"=w1374, "Position values"=w1373, "error in"=w1378) -> ("error out"=w1377:errorcluster)  [unwired: 1 in, 14 out]
                    n555 = call "General wait for movement to stop.vi"("System no."=w1376, "Axes to wait for"=w1374, "Additional wait time, ms"=u32 200, "error in"=w1377) -> ()  [unwired: 4 in, 12 out]
                  }
                  frame #2 {
                    n556 = local read "ADC Resolution [exponent]"() -> (w1379:T1)
                    n557 = local read "g2 settings"() -> (w1390:T4)
                    n558 = Unbundle By Name(w1390) -> ("collect_time"=w1389:sgl)
                    n559 = property on="g2 time remaining" class="Knob (strict)"(error in=w1385, "Scale.Maximum"=w1389) -> (error out=w1388:errorcluster)  [unwired: 1 in, 1 out]
                    n560 = property on="Measure g2" class="Bool (strict)"(error in=w1388, "DisabledEnum"=T8."Disabled and Grayed Out" ("Disabled")) -> (error out=w1384:errorcluster)  [unwired: 1 in, 1 out]
                    n561 = Unbundle(w1397) -> ("SPCMemConfig"=w1393:T10, "DLL Path"=w1396:path, "Module No"=w1395:i16, "Page"=w1394:i32)
                    n562 = control-ref of="g2 time remaining"() -> (w1392:refnum<vi>)
                    n563 = control-ref of="g2 abort"() -> (w1381:refnum<vi>)
                    n564 = call "TCSPC Measure.vi"("DLL Path"=w1396, "SPC Memory Config"=w1393, "Module No"=w1395, "Timer Refnum"=w1392, "Page"=w1394, "ADC Resolution (exponent)"=w1379, "Abort Refnum"=w1381, "Error In"=w1384, "User Input"=w1390) -> ("Data"=w1380:u16[], "x-scale multiplier"=w1391:dbl, "Error Out"=w1383:errorcluster)  [unwired: 3 in, 1 out]
                    n565 = property on="g2 data" class="WFGraph (strict)"(error in=w1383, "XScale.Multiplier"=w1391) -> (error out=w1382:errorcluster)  [unwired: 1 in, 1 out]
                    n566 = local write "g2 data"(w1380) -> ()
                    n567 = property on="Measure g2" class="Bool (strict)"(error in=w1382, "DisabledEnum"=T8."Enabled" ("Disabled")) -> ()  [unwired: 1 in, 2 out]
                  }
                  frame #3 {
                    n568 = control-ref of="Laser power (uW)"() -> (w1398:refnum<vi>)
                    n569 = call "Quick Laser Power Log.vi"("error in (no error)"=w1400, "Digital in"=w1398) -> ("Numeric"=w1399:dbl)  [unwired: 8 in, 1 out]
                  }
                  frame #4 {
                    n570 = property on="Filter Configuraton" class="Ring (strict)"() -> ("RingText.Text"=w1403:string)  [unwired: 2 in, 2 out]
                    n571 = local read "ADC Resolution [exponent]"() -> (w1404:T1)
                    n572 = local read "Filename Note"() -> (w1407:string)
                    n573 = Unbundle By Name(w1410) -> ("tac_range"=w1409:sgl, "tac_gain"=w1408:i16, "collect_time"=w1402:sgl)
                    n574 = call "Save Measurement File.vi"("Measurement Save Path"=w1411, "Measurement Type"=MeasurementType."g2", "Data in (if 1D)"=w1414, "ND angle"=w1413, "tac"=w1409, "Position"=w1412, "gain"=w1408, "integration time"=w1402, "bins"=w1404, "Filename Note"=w1407, "Filter"=w1403, "Prevent Save Dialog Prompt?"=TRUE, "laser power"=w1406) -> ()  [unwired: 7 in]
                  }
                }
                n575 = local read "g2 abort"() -> (w1358:bool)
              }
            }
            n576 = property on="Auto lifetime" class="Bool (strict)"(error in=w1335, "DisabledEnum"=T8."Enabled" ("Disabled")) -> (error out=w1334:errorcluster)  [unwired: 1 in, 1 out]
          }
        }
      }
      event "Auto lifetime": Value Change {
        n577 = event-data() -> ("NewVal"=w1420:bool)  [unwired: 1 in, 5 out]
        n578 = case shown="True" w1420 {
          tunnel: w1418 -> [w1421 w1425]
          tunnel: [w1421 w1426] -> w1419
          tunnel: w1417 -> [_ w1437]
          tunnel: w1416 -> [_ w1429]
          tunnel: w1415 -> [_ w1422]
          frame False {
          }
          frame True {
            n579 = local read "User Selected Measurement Points"() -> (w1432:dbl[][])
            n580 = property on="Auto lifetime" class="Bool (strict)"(error in=w1425, "DisabledEnum"=T8."Disabled and Grayed Out" ("Disabled")) -> (error out=w1424:errorcluster)  [unwired: 1 in, 1 out]
            n581 = local read "Filter Positions"() -> (w1431:dbl[])
            n582 = Array Size(array=w1432) -> (size(s)=w1438:i32[])
            n583 = local read "Measurement Save Path"() -> (w1430:path)
            n584 = Array Size(array=w1431) -> (size(s)=w1436:i32)
            n585 = Index Array(array=w1438, index=0) -> (element=w1435:i32)
            n586 = Round To Nearest(number=w1435) -> (nearest integer value=w1434:i32)
            n587 = Round To Nearest(number=w1436) -> (nearest integer value=w1433:i32)
            n588 = for {
              N: w1434 -> [_]
              shift-right: [w1449] -> w1427
              shift-left: w1424 -> [w1448]
              tunnel: w1432 -> [w1447] mode=indexing
              tunnel: w1431 -> [w1446]
              tunnel: w1437 -> [w1445]
              tunnel: w1433 -> [w1444]
              tunnel: w1430 -> [w1443]
              tunnel: w1429 -> [w1442]
              tunnel: w1422 -> [w1440]
              stop <- w1441 stop-if-true
              n589 = for {
                N: w1444 -> [_]
                tunnel: w1447 -> [w1456]
                tunnel: w1446 -> [w1455] mode=indexing
                tunnel: w1445 -> [w1454]
                shift-right: [w1458] -> w1449
                shift-left: w1448 -> [w1457]
                tunnel: w1443 -> [w1453]
                tunnel: w1442 -> [w1452]
                tunnel: [w1450] -> w1441
                tunnel: w1440 -> [w1451]
                stop <- w1450 stop-if-true
                n590 = stacked-sequence {
                  seq-local: [_ _ w1472 _ _] -> [_ _ _ _ w1505]
                  seq-local: [_ _ w1481 _ _] -> [_ _ _ _ w1501]
                  seq-local: [_ _ _ w1490 _] -> [_ _ _ _ w1497]
                  tunnel: [w1464 _ _ _ _] -> w1458
                  tunnel: w1457 -> [_ w1470 w1479 _ _]
                  tunnel: w1456 -> [_ w1465 _ _ w1503]
                  tunnel: w1455 -> [w1461 _ _ _ w1504]
                  tunnel: w1454 -> [_ w1468 _ _ _]
                  tunnel: w1453 -> [_ _ _ _ w1502]
                  tunnel: w1452 -> [_ _ w1489 _ _]
                  tunnel: w1451 -> [w1462 _ _ _ _]
                  frame #0 {
                    # "Move rotation attenuator angle"
                    n591 = invoke class="KCubeDCServo" method="MoveTo"(reference=w1462, "position"=w1461, "waitTimeout"=0) -> (error out=w1460:errorcluster)  [unwired: 2 in, 4 out]
                    n592 = call "Time Delay2"("error in (no error)"=w1460, "Delay Time (s)"=5.0) -> ("error out"=w1464:errorcluster)  [unwired: 9 in]
                  }
                  frame #1 {
                    w1466 = string[] ["1", "2"]
                    n593 = call "MOV.vi"("System no."=w1468, "Axes to move"=w1466, "Position values"=w1465, "error in"=w1470) -> ("error out"=w1469:errorcluster)  [unwired: 1 in, 14 out]
                    n594 = call "General wait for movement to stop.vi"("System no."=w1468, "Axes to wait for"=w1466, "Additional wait time, ms"=u32 200, "error in"=w1469) -> ()  [unwired: 4 in, 12 out]
                  }
                  frame #2 {
                    n595 = local read "Lifetime settings"() -> (w1481:T4)
                    n596 = Unbundle By Name(w1481) -> ("collect_time"=w1480:sgl)
                    n597 = local read "ADC Resolution [exponent]"() -> (w1471:T1)
                    n598 = property on="Lifetime time remaining" class="Knob (strict)"(error in=w1479, "Scale.Maximum"=w1480) -> (error out=w1478:errorcluster)  [unwired: 1 in, 1 out]
                    n599 = property on="Meaure lifetime" class="Bool (strict)"(error in=w1478, "DisabledEnum"=T8."Disabled and Grayed Out" ("Disabled")) -> (error out=w1476:errorcluster)  [unwired: 1 in, 1 out]
                    n600 = control-ref of="Lifetime time remaining"() -> (w1483:refnum<vi>)
                    n601 = Unbundle(w1489) -> ("SPCMemConfig"=w1485:T10, "DLL Path"=w1488:path, "Module No"=w1487:i16, "Page"=w1486:i32)
                    n602 = control-ref of="Lifetime abort"() -> (w1484:refnum<vi>)
                    n603 = call "TCSPC Measure.vi"("DLL Path"=w1488, "SPC Memory Config"=w1485, "Module No"=w1487, "Timer Refnum"=w1483, "Page"=w1486, "ADC Resolution (exponent)"=w1471, "Abort Refnum"=w1484, "Error In"=w1476, "User Input"=w1481) -> ("Data"=w1472:u16[], "x-scale multiplier"=w1482:dbl, "Error Out"=w1475:errorcluster)  [unwired: 3 in, 1 out]
                    n604 = property on="lifetime data" class="WFGraph (strict)"(error in=w1475, "XScale.Multiplier"=w1482) -> (error out=w1474:errorcluster)  [unwired: 1 in, 1 out]
                    n605 = local write "lifetime data"(w1472) -> ()
                    n606 = property on="Meaure lifetime" class="Bool (strict)"(error in=w1474, "DisabledEnum"=T8."Enabled" ("Disabled")) -> ()  [unwired: 1 in, 2 out]
                  }
                  frame #3 {
                    n607 = control-ref of="Laser power (uW)"() -> (w1491:refnum<vi>)
                    n608 = call "Quick Laser Power Log.vi"("Digital in"=w1491) -> ("Numeric"=w1490:dbl)  [unwired: 9 in, 1 out]
                  }
                  frame #4 {
                    n609 = property on="Filter Configuraton" class="Ring (strict)"() -> ("RingText.Text"=w1494:string)  [unwired: 2 in, 2 out]
                    n610 = local read "Filename Note"() -> (w1498:string)
                    n611 = Unbundle By Name(w1501) -> ("tac_range"=w1500:sgl, "tac_gain"=w1499:i16, "collect_time"=w1496:sgl)
                    n612 = local read "ADC Resolution [exponent]"() -> (w1493:T1)
                    n613 = call "Save Measurement File.vi"("Measurement Save Path"=w1502, "Measurement Type"=MeasurementType."Lifetime", "Data in (if 1D)"=w1505, "ND angle"=w1504, "tac"=w1500, "Position"=w1503, "gain"=w1499, "integration time"=w1496, "bins"=w1493, "Filename Note"=w1498, "Filter"=w1494, "Prevent Save Dialog Prompt?"=TRUE, "laser power"=w1497) -> ()  [unwired: 7 in]
                  }
                }
                n614 = local read "Lifetime abort"() -> (w1450:bool)
              }
            }
            n615 = property on="Auto lifetime" class="Bool (strict)"(error in=w1427, "DisabledEnum"=T8."Enabled" ("Disabled")) -> (error out=w1426:errorcluster)  [unwired: 1 in, 1 out]
          }
        }
      }
      event "Auto Spectrum": Value Change {
        n616 = event-data() -> ("NewVal"=w1512:bool)  [unwired: 1 in, 5 out]
        n617 = case shown="True" w1512 {
          tunnel: w1510 -> [w1513 w1523]
          tunnel: [w1513 w1515] -> w1511
          tunnel: w1509 -> [_ w1535]
          tunnel: w1508 -> [_ w1521]
          tunnel: w1507 -> [_ w1520]
          tunnel: w1506 -> [_ w1514]
          frame False {
          }
          frame True {
            n618 = flat-sequence {
              tunnel: [w1547] -> w1522
              tunnel: w1523 -> [w1547]
              tunnel: w1521 -> [w1542]
              tunnel: w1520 -> [w1541]
              tunnel: [w1540] -> w1519
              tunnel: [w1539] -> w1518
              frame #0 {
                # "set for spectometer"
                n619 = invoke class="FilterFlipper" method="SetPosition"(reference=w1541, "position"=u32 1, "waitTimeout"=0) -> (reference out=w1540:refnum<k24>)  [unwired: 2 in, 4 out]
                n620 = invoke class="FilterFlipper" method="SetPosition"(reference=w1542, "position"=u32 1, "waitTimeout"=0) -> (reference out=w1539:refnum<k24>)  [unwired: 2 in, 4 out]
                n621 = Wait (ms)(milliseconds to wait=550) -> ()  [unwired: 1 out]
                n622 = property on="Auto Spectrum" class="Bool (strict)"("DisabledEnum"=T8."Disabled and Grayed Out" ("Disabled")) -> ()  [unwired: 2 in, 2 out]
              }
            }
            n623 = local read "User Selected Measurement Points"() -> (w1528:dbl[][])
            n624 = local read "Spectrum Integration Time (s)"() -> (w1526:i32)
            n625 = Array Size(array=w1528) -> (size(s)=w1536:i32[])
            n626 = local read "Filter Positions"() -> (w1525:dbl[])
            n627 = Multiply(x=w1526, y=1000000.0) -> (x*y=w1529:dbl)
            n628 = Array Size(array=w1525) -> (size(s)=w1534:i32)
            n629 = Index Array(array=w1536, index=0) -> (element=w1533:i32)
            n630 = Round To Nearest(number=w1533) -> (nearest integer value=w1532:i32)
            n631 = Round To Nearest(number=w1534) -> (nearest integer value=w1531:i32)
            n632 = Round To Nearest(number=w1529) -> (nearest integer value=w1527:dbl)
            n633 = local read "Measurement Save Path"() -> (w1524:path)
            n634 = for {
              N: w1532 -> [_]
              shift-right: [w1561] -> w1516
              shift-left: w1522 -> [w1560]
              tunnel: w1528 -> [w1559] mode=indexing
              tunnel: w1525 -> [w1558]
              tunnel: w1535 -> [w1557]
              tunnel: w1531 -> [w1556]
              tunnel: w1524 -> [w1555]
              tunnel: w1526 -> [w1554]
              tunnel: w1527 -> [w1553]
              tunnel: w1519 -> [w1551]
              tunnel: w1518 -> [w1550]
              tunnel: w1514 -> [w1549]
              stop <- w1552 stop-if-true
              n635 = for {
                N: w1556 -> [_]
                tunnel: w1559 -> [w1571]
                tunnel: w1558 -> [w1570] mode=indexing
                tunnel: w1557 -> [w1569]
                shift-right: [w1573] -> w1561
                shift-left: w1560 -> [w1572]
                tunnel: w1555 -> [w1568]
                tunnel: w1554 -> [w1567]
                tunnel: w1553 -> [w1566]
                shift-right: ["Stop Auto Spectrum"] -> w1552
                shift-left: _ -> [_]
                tunnel: w1551 -> [w1564]
                tunnel: w1550 -> [w1563]
                tunnel: w1549 -> [w1562]
                stop <- "Stop Auto Spectrum" stop-if-true
                n636 = stacked-sequence {
                  seq-local: [_ _ _ w1616 _] -> [_ _ _ _ w1623]
                  tunnel: [w1580 _ _ _ _] -> w1573
                  tunnel: w1572 -> [w1576 w1587 w1594 w1615 w1622]
                  tunnel: w1571 -> [_ w1581 _ _ w1626]
                  tunnel: w1570 -> [w1577 _ _ _ w1627]
                  tunnel: w1569 -> [_ w1585 _ _ _]
                  tunnel: [_ w1582 _ _ _] -> _
                  tunnel: [_ _ _ _ w1622] -> _
                  tunnel: [_ _ w1591 _ _] -> _
                  tunnel: w1568 -> [_ _ _ _ w1620]
                  tunnel: w1567 -> [_ _ _ _ w1625]
                  tunnel: w1566 -> [_ _ w1590 _ _]
                  tunnel: w1564 -> [_ _ w1589 _ _]
                  tunnel: w1563 -> [_ _ w1588 _ _]
                  tunnel: w1562 -> [w1578 _ _ _ _]
                  frame #0 {
                    # "Add rotation filter to minimum here"
                    n637 = invoke class="KCubeDCServo" method="MoveTo"(reference=w1578, error in=w1576, "position"=w1577, "waitTimeout"=0) -> (error out=w1575:errorcluster)  [unwired: 1 in, 4 out]
                    n638 = call "Time Delay"("error in (no error)"=w1575, "Delay Time (s)"=5.0) -> ("error out"=w1580:errorcluster)  [unwired: 9 in]
                  }
                  frame #1 {
                    w1583 = string[] ["1", "2"]
                    n639 = call "MOV.vi"("System no."=w1585, "Axes to move"=w1583, "Position values"=w1581, "error in"=w1587) -> ("error out"=w1586:errorcluster)  [unwired: 1 in, 14 out]
                    n640 = call "General wait for movement to stop.vi"("System no."=w1585, "Axes to wait for"=w1583, "Additional wait time, ms"=u32 200, "error in"=w1586) -> ("error out"=w1582:errorcluster)  [unwired: 4 in, 11 out]
                  }
                  frame #2 {
                    n641 = flat-sequence {
                      tunnel: [w1613] -> w1593
                      tunnel: w1594 -> [w1613]
                      tunnel: w1589 -> [w1608]
                      tunnel: w1588 -> [w1607]
                      frame #0 {
                        n642 = invoke class="FilterFlipper" method="SetPosition"(reference=w1608, "position"=u32 2, "waitTimeout"=0) -> ()  [unwired: 2 in, 5 out]
                        n643 = invoke class="FilterFlipper" method="SetPosition"(reference=w1607, "position"=u32 2, "waitTimeout"=0) -> ()  [unwired: 2 in, 5 out]
                        n644 = Wait (ms)(milliseconds to wait=u32 550 ("millisecond timer value")) -> ()  [unwired: 1 out]
                      }
                    }
                    n645 = local read "Scans to Average"() -> (w1603:i32)
                    n646 = local read "N Integrations"() -> (w1600:i32)
                    n647 = local read "Boxcar Width"() -> (w1604:i32)
                    n648 = local read "EDC Enable"() -> (w1597:i32)
                    n649 = local read "NLC Enable"() -> (w1602:i32)
                    n650 = local read "lampOn 2"() -> (w1601:i32)
                    n651 = local read "lampOn"() -> (w1605:i32)
                    n652 = local read "enable"() -> (w1599:i16)
                    n653 = call "OceanOpticsRecordSpectra.vi"("Boxcar Width"=w1604, "Scans to Average"=w1603, "EDC Enable"=w1597, "NLC Enable"=w1602, "error in (no error)"=w1593, "lampOn"=w1605, "N Integrations"=w1600, "Int. Time (microsec)"=w1590, "lampOn 2"=w1601, "Spectrometer Index"=0, "enable"=w1599) -> ("getName"=w1595:string, "getSerialNumber"=w1596:string, "XY Graph"=w1606:cluster{"Y":dbl[], "Y":dbl[]}[], "Array"=w1592:dbl[][], "error out"=w1591:errorcluster)  [unwired: 4 in]
                    n654 = local write "Spectrometer Name:"(w1595) -> ()
                    n655 = local write "Spectrum"(w1606) -> ()
                    n656 = local write "spectrum output"(w1592) -> ()
                    n657 = local write "Serial Number:"(w1596) -> ()
                  }
                  frame #3 {
                    n658 = control-ref of="Laser power (uW)"() -> (w1617:refnum<vi>)
                    n659 = call "Quick Laser Power Log.vi"("error in (no error)"=w1615, "Digital in"=w1617) -> ("Numeric"=w1616:dbl)  [unwired: 8 in, 1 out]
                  }
                  frame #4 {
                    n660 = property on="Filter Configuraton" class="Ring (strict)"() -> ("RingText.Text"=w1619:string)  [unwired: 2 in, 2 out]
                    n661 = local read "spectrum output"() -> (w1628:dbl[][])
                    n662 = local read "Filename Note"() -> (w1624:string)
                    n663 = call "Save Measurement File.vi"("Measurement Save Path"=w1620, "Measurement Type"=MeasurementType."Spectrum", "Data in (if 2D)"=w1628, "ND angle"=w1627, "Position"=w1626, "integration time"=w1625, "Filename Note"=w1624, "Filter"=w1619, "Prevent Save Dialog Prompt?"=TRUE, "laser power"=w1623) -> ()  [unwired: 10 in]
                  }
                }
              }
            }
            n664 = property on="Auto Spectrum" class="Bool (strict)"(error in=w1516, "DisabledEnum"=T8."Enabled" ("Disabled")) -> (error out=w1515:errorcluster)  [unwired: 1 in, 1 out]
          }
        }
      }
      event "Auto Saturation": Value Change {
        n665 = event-data() -> ("NewVal"=w1633:bool)  [unwired: 1 in, 5 out]
        n666 = case shown="True" w1633 {
          tunnel: w1631 -> [w1634 w1641]
          tunnel: [w1634 w1635] -> w1632
          tunnel: w1630 -> [_ w1647]
          tunnel: w1629 -> [_ w1640]
          frame False {
          }
          frame True {
            n667 = local read "User Selected Measurement Points"() -> (w1644:dbl[][])
            n668 = local read "Saturation Sweep Speed (deg/s)"() -> (w1638:dbl)
            n669 = local read "Measurement Save Path"() -> (w1642:path)
            n670 = local read "Saturation Start Angle"() -> (w1636:dbl)
            n671 = Array Size(array=w1644) -> (size(s)=w1648:i32[])
            n672 = local read "Saturation End Angle"() -> (w1639:dbl)
            n673 = local read "Filename Note"() -> (w1637:string)
            n674 = Index Array(array=w1648, index=0) -> (element=w1646:i32)
            n675 = Round To Nearest(number=w1646) -> (nearest integer value=w1645:i32)
            n676 = for {
              N: w1645 -> [_]
              tunnel: w1644 -> [w1660] mode=indexing
              tunnel: w1647 -> [w1659]
              tunnel: w1642 -> [w1658]
              tunnel: 1000000.0 ("y") -> [w1657]
              tunnel: w1641 -> [w1656]
              tunnel: w1640 -> [w1655]
              tunnel: w1636 -> [w1651]
              tunnel: w1639 -> [w1654]
              tunnel: w1638 -> [w1653]
              tunnel: w1637 -> [w1652]
              tunnel: [w1650] -> w1635
              n677 = stacked-sequence {
                tunnel: w1660 -> [w1661 w1677]
                tunnel: w1659 -> [w1667 _]
                tunnel: w1658 -> [_ w1680]
                tunnel: w1657 -> [_ _]
                tunnel: [w1663 _] -> _
                tunnel: w1656 -> [w1662 w1682]
                tunnel: w1655 -> [_ w1681]
                tunnel: w1651 -> [_ w1674]
                tunnel: w1654 -> [_ w1679]
                tunnel: w1653 -> [_ w1678]
                tunnel: w1652 -> [_ w1676]
                tunnel: [_ w1675] -> _
                tunnel: [_ w1673] -> _
                tunnel: w1651 -> [_ w1672]
                tunnel: [_ w1671] -> w1650
                frame #0 {
                  w1665 = string[] ["1", "2"]
                  n678 = call "MOV.vi"("System no."=w1667, "Axes to move"=w1665, "Position values"=w1661, "error in"=w1662) -> ("error out"=w1668:errorcluster)  [unwired: 1 in, 14 out]
                  n679 = call "General wait for movement to stop.vi"("System no."=w1667, "Axes to wait for"=w1665, "Additional wait time, ms"=u32 500, "error in"=w1668) -> ("error out"=w1664:errorcluster)  [unwired: 4 in, 11 out]
                  n680 = flat-sequence {
                    tunnel: w1664 -> [w1669]
                    tunnel: [w1669] -> w1663
                    frame #0 {
                      n681 = local write "SLOC Laser"(TRUE) -> ()
                    }
                  }
                }
                frame #1 {
                  n682 = flat-sequence {
                    tunnel: w1682 -> [w1693]
                    tunnel: w1681 -> [w1696]
                    tunnel: [w1695] -> w1690
                    tunnel: [w1694] -> w1689
                    tunnel: w1674 -> [w1692]
                    tunnel: [w1701] -> w1688
                    tunnel: w1690 -> [w1701]
                    tunnel: [w1700] -> w1687
                    tunnel: w1689 -> [w1700]
                    tunnel: w1688 -> [w1707]
                    tunnel: w1687 -> [w1706]
                    tunnel: [w1705] -> w1686
                    tunnel: [w1704] -> w1685
                    tunnel: w1679 -> [w1703]
                    tunnel: w1678 -> [w1702]
                    tunnel: [w1716] -> w1684
                    tunnel: w1686 -> [w1716]
                    tunnel: [w1717] -> w1683
                    tunnel: w1685 -> [w1717]
                    tunnel: w1680 -> [w1713]
                    tunnel: w1677 -> [w1712]
                    tunnel: w1676 -> [w1711]
                    tunnel: w1684 -> [w1723]
                    tunnel: w1683 -> [w1722]
                    tunnel: [w1723] -> w1675
                    tunnel: [w1722] -> w1673
                    tunnel: w1672 -> [w1719]
                    tunnel: [w1718] -> w1671
                    frame #0 {
                      n683 = call "Saturation Start Sequence.vi"("error in (no error)"=w1693, "Saturation Start Angle"=w1692, "Rotation stage refnum"=w1696) -> ("error out"=w1694:errorcluster, "Rotation stage refnum out"=w1695:refnum<k24>)  [unwired: 1 out]
                      n684 = local write "Empty memory"(TRUE ("Empty memory")) -> ()
                    }
                    frame #1 {
                      n685 = local write "Record counts"(TRUE ("Record stab")) -> ()
                      n686 = Wait (ms)(milliseconds to wait=u32 200) -> ()  [unwired: 1 out]
                      n687 = local write "Empty memory"(FALSE ("Empty memory")) -> ()
                    }
                    frame #2 {
                      n688 = call "Saturation Move Sequence.vi"("error in (no error)"=w1706, "Saturation Sweep Speed"=w1702, "Saturation End Angle"=w1703, ".NET Refnum in"=w1707) -> ("error out"=w1705:errorcluster, "reference out"=w1704:refnum<k24>)
                    }
                    frame #3 {
                      n689 = Wait (ms)(milliseconds to wait=u32 500) -> ()  [unwired: 1 out]
                      n690 = local read "TraceData"() -> (w1714:dbl[][])
                      n691 = property on="Mirror Configuraton" class="Ring (strict)"() -> ("RingText.Text"=w1709:string)  [unwired: 2 in, 2 out]
                      n692 = call "Save Measurement File.vi"("Measurement Save Path"=w1713, "Measurement Type"=MeasurementType."Saturation", "Data in (if 2D)"=w1714, "Position"=w1712, "Filename Note"=w1711, "Filter"=w1709, "Prevent Save Dialog Prompt?"=TRUE) -> ()  [unwired: 13 in]
                    }
                    frame #4 {
                      n693 = local write "Record counts"(FALSE ("Record stab")) -> ()
                      n694 = Wait (ms)(milliseconds to wait=u32 200) -> ()  [unwired: 1 out]
                      n695 = call "Saturation Return or End Sequence.vi"("return position"=w1719) -> ("error out"=w1718:errorcluster)  [unwired: 9 in, 1 out]
                    }
                  }
                }
              }
            }
          }
        }
      }
      event "Mirror Configuraton": Value Change {
        # "This NewVal might work might need to be replaced with the miriror configuration variable"
        n696 = event-data() -> ("NewVal"=w1725:u16)  [unwired: 1 in, 5 out]
        n697 = case shown="0, Default" w1725 {
          tunnel: w1727 -> [w1729 w1735 w1741]
          tunnel: w1726 -> [w1728 w1734 w1740]
          frame 0, Default {
            n698 = invoke class="FilterFlipper" method="SetPosition"(reference=w1728, "position"=u32 1, "waitTimeout"=0) -> ()  [unwired: 2 in, 5 out]
            n699 = invoke class="FilterFlipper" method="SetPosition"(reference=w1729, "position"=u32 1, "waitTimeout"=0) -> ()  [unwired: 2 in, 5 out]
          }
          frame 1 {
            n700 = invoke class="FilterFlipper" method="SetPosition"(reference=w1734, "position"=u32 2, "waitTimeout"=0) -> ()  [unwired: 2 in, 5 out]
            n701 = invoke class="FilterFlipper" method="SetPosition"(reference=w1735, "position"=u32 1, "waitTimeout"=0) -> ()  [unwired: 2 in, 5 out]
          }
          frame 2 {
            n702 = invoke class="FilterFlipper" method="SetPosition"(reference=w1740, "position"=u32 2, "waitTimeout"=0) -> ()  [unwired: 2 in, 5 out]
            n703 = invoke class="FilterFlipper" method="SetPosition"(reference=w1741, "position"=u32 2, "waitTimeout"=0) -> ()  [unwired: 2 in, 5 out]
          }
        }
      }
      event "Filter Configuraton": Value Change {
        # "This NewVal might work might need to be replaced with the miriror configuration variable"
        n704 = event-data() -> ("NewVal"=w1750:u16)  [unwired: 1 in, 5 out]
        n705 = case shown="True" w1748 {
          tunnel: w1751 -> [w1753 w1759]
          tunnel: [w1752 w1758] -> w1746
          tunnel: w1750 -> [_ w1757]
          tunnel: [w1753 w1756] -> w1749
          tunnel: w1747 -> [w1752 w1754]
          frame False {
          }
          frame True {
            n706 = call "FilterWheelMove.vi"("error in (no error)"=w1754, "Filter Configuraton"=w1757, "hdl in"=w1759) -> ("error out"=w1758:errorcluster, "Get Position"=w1755:i32, "hdl out"=w1756:i32)  [unwired: 6 in]
            n707 = local write "Filter wheel position"(w1755) -> ()
          }
        }
      }
      event "Min power": Mouse Down {
        (unwired) 90.0 ("position")
        n708 = event-data() -> ()  [unwired: 1 in, 8 out]
        n709 = invoke class="KCubeDCServo" method="MoveTo"(reference=w1763, "position"=0.0, "waitTimeout"=0) -> ()  [unwired: 2 in, 5 out]
      }
      event "Set power": Mouse Down {
        n710 = event-data() -> ()  [unwired: 1 in, 8 out]
        n711 = invoke class="KCubeDCServo" method="MoveTo"(reference=w1767, "position"="Move to", "waitTimeout"=0) -> ()  [unwired: 2 in, 5 out]
      }
      event "GetNewLoc": Value Change {
        n712 = event-data() -> ("CtlRef"=w1772:refnum<vi>, "NewVal"=w1773:bool)  [unwired: 1 in, 4 out]
        n713 = case shown="True" w1773 {
          tunnel: w1772 -> [w1775 w1787]
          tunnel: [w1775 w1787] -> w1770
          tunnel: w1768 -> [w1774 w1782]
          tunnel: [w1774 w1786] -> w1769
          frame False {
          }
          frame True {
            # "Code rewritten to not use the image processing toolbox 12/30/2025\n\nOld code is below it, commented out"
            n714 = local read "Upper contrast threshold"() -> (w1779:dbl)
            n715 = local read "Lower contrast threshold"() -> (w1778:dbl)
            n716 = disable-structure shown="Disabled" {
              frame Disabled {
                n717 = mathscript code="cent=[];%\n\n%d((d>32.76)&(d<32.80))=0;\n\n%% Level and normalize the map\n\nd = d - min(d(:)) ; \nM = max(d(:));\nd = d / max(d(:)) ;\n\nthres_coeff = thres_coeff/M;\nup_thres_coeff = up_thres_coeff/M;\n\n%% Define smoothing filter for the map\n\nmesh = 0.05;\ndiffracLength = 0.3;\ndiffracPixels = floor(diffracLength/mesh);\n\nsigma = 1; %gaussian low-pass filter\nkernel = zeros(2*diffracPixels + 1, 2*diffracPixels+1);\nW = 0;\nfor i = 1:diffracPixels\n    for j = 1:diffracPixels\n        sq_dist = (i-diffracPixels-1)^2 + (j-diffracPixels-1)^2;\n        kernel(i,j) = exp(-1*(sq_dist)/(2*sigma*sigma));\n        W = W + kernel(i,j);\n    end\nend\nkernel = kernel/W;\n\n%% defaults\n\nif any(any(~floor(d))) %For the case the input image is double, casting to uint16 keeps enough dynamic range while speeds up the code.\n\n    if max(d(:))<=1\n        d =  uint16( d.*2^16./(max(d(:))));\n    else\n        d = uint16(d);\n    end\nend\n\nthres = (max([min(max(d,[],1))  min(max(d,[],2))])) ;\nfilt = kernel; %if needed modify the filter according to the expected peaks sizes\nedg = diffracPixels+1;\nres = 1;\n\n%% Analyze image\n\n\n    \n    % apply threshold\n    if isa(d,'uint8')\n        d=d.*uint8(d>thres);\n    elseif isa(d,'uint16')\n        d=d.*uint16(d>thres);\n    end\n    \n        % smooth image\n        d=conv2(single(d),filt,'same') ;\n        M = max(d(:));\n        thres_coeff = uint16(floor(thres_coeff*M));\n        up_thres_coeff = up_thres_coeff*M;\n        % Apply again threshold (and change if needed according to SNR)\n        d=d.*(d>thres_coeff);\n        bw = (d>thres_coeff);\n        CC = bwconncomp(bw);\n              for i = 1:length(CC.PixelIdxList)\n                      if numel(CC.PixelIdxList{i}) > (2*diffracPixels)^2\n                           d(CC.PixelIdxList{i}) = 0;\n                      end\n               end\n                % switch between local maxima and sub-pixel methods\n            \n                % peak find - using the local maxima approach - 1 pixel resolution\n                \n                % d will be noisy on the edges, and also local maxima looks\n                % for nearest neighbors so edge must be at least 1. We'll skip 'edge' pixels.\n                sd=size(d);\n                [x y]=find(d(edg:sd(1)-edg,edg:sd(2)-edg));\n                \n                % initialize outputs\n \n\n                cent_map=zeros(sd);\n                \n                x=x+edg-1;\n                y=y+edg-1;\n                for j=1:length(y)\n                        if  d(x(j),y(j)) == max(max(d((x(j)- diffracPixels):(x(j)+diffracPixels),(y(j)-diffracPixels):(y(j)+ diffracPixels))))\n\n\n                        if( d(x(j), y(j))< up_thres_coeff)\n                                cent = [cent ;  x(j)  y(j)];\n                        end\n                        %cent_map(x(j),y(j))=cent_map(x(j),y(j))+1; % if a binary matrix output is desired\n                        \n                    end\n                end"() -> ()  [unwired: 4 in, 2 out]
              }
              frame Enabled {
              }
            }
            n718 = local read "Intensity Graph"() -> (w1780:dbl[][])
            n719 = local read "Mesh"() -> (w1776:dbl)
            n720 = script code="cent = [];\n\n%% Level and normalize \nd = d - min(d(:)); \nM = max(d(:));\nd = d / M;\n\nthres_coeff = thres_coeff / M;\nup_thres_coeff = up_thres_coeff / M;\n\n%% Define smoothing filter (Standard MATLAB - No Toolbox)\nmesh = 0.05;\ndiffracLength = 0.3;\ndiffracPixels = floor(diffracLength/mesh);\n\nsigma = 1.50;\n% Create a grid for the Gaussian kernel without loops\n[x_grid, y_grid] = meshgrid(-diffracPixels:diffracPixels, -diffracPixels:diffracPixels);\nkernel = exp(-(x_grid.^2 + y_grid.^2) / (2 * sigma^2));\nkernel = kernel / sum(kernel(:));\n\n%% Image Prep\nif any(any(mod(d, 1) ~= 0)) || max(d(:)) <= 1\n    d = uint16(d .* 65535);\nelse\n    d = uint16(d);\nend\n\n% Base threshold calculation\nthres = max([min(max(d,[],1)) min(max(d,[],2))]);\nedg = diffracPixels + 1;\n\n%% Analyze image\n% Apply initial threshold\nd_filtered = d .* uint16(d > thres);\n\n% Smooth image using standard 2D convolution\nd_smooth = conv2(single(d_filtered), kernel, 'same');\nM_smooth = max(d_smooth(:));\n\n% Adjust thresholds for the smoothed image\nfinal_thres = thres_coeff * M_smooth;\nfinal_up_thres = up_thres_coeff * M_smooth;\n\n% Filter by threshold\nd_smooth = d_smooth .* (d_smooth > final_thres);\n\n%% Local Maxima Search (Toolbox-Free Vectorization)\n% Instead of bwconncomp, we use a sliding window comparison\nsd = size(d_smooth);\n[rows, cols] = find(d_smooth > final_thres);\n\n% Filter coordinates away from edges to prevent indexing errors\nvalid_idx = (rows > edg) & (rows < sd(1)-edg) & (cols > edg) & (cols < sd(2)-edg);\nrows = rows(valid_idx);\ncols = cols(valid_idx);\n\nfor i = 1:length(rows)\n    r = rows(i);\n    c = cols(i);\n    \n    % Extract the local neighborhood\n    local_window = d_smooth(r-diffracPixels:r+diffracPixels, c-diffracPixels:c+diffracPixels);\n    \n    % Check if central pixel is the absolute maximum in its neighborhood\n    if d_smooth(r,c) == max(local_window(:))\n        % Apply the upper intensity bound\n        if d_smooth(r,c) < final_up_thres\n            cent = [cent; r, c];\n        end\n    end\nend\n\n% Remove duplicates (in case of flat-top peaks)\ncent = unique(cent, 'rows');\n\n\n%% OLD CODE BELOW: REQUIRES IMAGE PROCESSING TOOLBOX:\n\n% cent=[];%\n% \n% %d((d>32.76)&(d<32.80))=0;\n% \n% %% Level and normalize the map\n% \n% d = d - min(d(:)) ; \n% M = max(d(:));\n% d = d / max(d(:)) ;\n% \n% thres_coeff = thres_coeff/M;\n% up_thres_coeff = up_thres_coeff/M;\n% \n% %% Define smoothing filter for the map\n% \n% mesh = 0.05;\n% diffracLength = 0.3;\n% diffracPixels = floor(diffracLength/mesh);\n% \n% sigma = 1.50; %gaussian low-pass filter\n% kernel = zeros(2*diffracPixels + 1, 2*diffracPixels+1);\n% W = 0;\n% for i = 1:diffracPixels\n%     for j = 1:diffracPixels\n%         sq_dist = (i-diffracPixels-1)^2 + (j-diffracPixels-1)^2;\n%         kernel(i,j) = exp(-1*(sq_dist)/(2*sigma*sigma));\n%         W = W + kernel(i,j);\n%     end\n% end\n% kernel = kernel/W;\n% \n% %% defaults\n% \n% if any(any(~floor(d))) %For the case the input image is double, casting to uint16 keeps enough dynamic range while speeds up the code.\n% \n%     if max(d(:))<=1\n%         d =  uint16( d.*2^16./(max(d(:))));\n%     else\n%         d = uint16(d);\n%     end\n% end\n% \n% thres = (max([min(max(d,[],1))  min(max(d,[],2))])) ;\n% filt = kernel; %if needed modify the filter according to the expected peaks sizes\n% edg = diffracPixels+1;\n% res = 1;\n% \n% %% Analyze image\n% \n% \n% \n%     % apply threshold\n%     if isa(d,'uint8')\n%         d=d.*uint8(d>thres);\n%     elseif isa(d,'uint16')\n%         d=d.*uint16(d>thres);\n%     end\n% \n%         % smooth image\n%         d=conv2(single(d),filt,'same') ;\n%         M = max(d(:));\n%         thres_coeff = uint16(floor(thres_coeff*M));\n%         up_thres_coeff = up_thres_coeff*M;\n%         % Apply again threshold (and change if needed according to SNR)\n%         d=d.*(d>thres_coeff);\n% \n%          bw1 = (d>thres_coeff);\n%         CC1 = bwconncomp(bw1);\n%               for i = 1:length(CC1.PixelIdxList)\n%                       if numel(CC1.PixelIdxList{i}) > (2.25*diffracPixels)^2\n%                            %d(CC1.PixelIdxList{i}) = 0;\n%                       end\n%                end\n% \n%         bw2 = (d>thres_coeff/2);\n%        CC2 = bwconncomp(bw2);\n%               for i = 1:length(CC2.PixelIdxList)\n%                       if numel(CC2.PixelIdxList{i}) < 2\n%                            %d(CC2.PixelIdxList{i}) = 0;\n%                      end\n% end\n% \n% \n%                 % switch between local maxima and sub-pixel methods\n% \n%                 % peak find - using the local maxima approach - 1 pixel resolution\n% \n%                 % d will be noisy on the edges, and also local maxima looks\n%                 % for nearest neighbors so edge must be at least 1. We'll skip 'edge' pixels.\n%                 sd=size(d);\n%                 [x y]=find(d(edg:sd(1)-edg,edg:sd(2)-edg));\n% \n%                 % initialize outputs\n% \n% \n%                 cent_map=zeros(sd);\n% \n%                 x=x+edg-1;\n%                 y=y+edg-1;\n%                 for j=1:length(y)\n%                         if  d(x(j),y(j)) == max(max(d((x(j)- diffracPixels):(x(j)+diffracPixels),(y(j)-diffracPixels):(y(j)+ diffracPixels))))\n% \n% \n%                         if( d(x(j), y(j))< up_thres_coeff)\n%                                 cent = [cent ;  x(j)  y(j)];\n%                         end\n%                         %cent_map(x(j),y(j))=cent_map(x(j),y(j))+1; % if a binary matrix output is desired\n% \n%                     end\n%                 end"("??"=w1782, "d"=w1780, "up_thres_coeff"=w1779, "thres_coeff"=w1778, "mesh"=w1776) -> ("??"=w1781:errorcluster, "cent"=w1777:dbl[][])
            n721 = local write "cent"(w1777) -> ()
            n722 = flat-sequence {
              tunnel: w1781 -> [w1788]
              tunnel: [w1788] -> w1786
              frame #0 {
                n723 = local write "Emitter #"(0 ("Emitter #")) -> ()
              }
            }
            n724 = Array Size(array=w1777) -> (size(s)=w1785:i32[])
            n725 = Index Array(array=w1785, index=0) -> (element=w1783:i32)
            n726 = local write "# of Emitters"(w1783) -> ()
          }
        }
        n727 = property class="Bool (strict)"(reference=w1770, "Value"=FALSE) -> ()  [unwired: 1 in, 2 out]
      }
      event "Draw emitters": Value Change {
        n728 = event-data() -> ()  [unwired: 1 in, 6 out]
        n729 = local read "X Range"() -> (w1791:dbl)
        n730 = local read "Y Range"() -> (w1790:dbl)
        n731 = local read "Mesh"() -> (w1792:dbl)
        n732 = local read "cent"() -> (w1793:i32[][])
        n733 = call "AUTOFLIM_Draw_emitters.vi"("Y Scan Range"=w1790, "X Scan Range"=w1791, "Mesh"=w1792, "cent"=w1793) -> ("Plot Images:Front"=w1794:picture)  [unwired: 6 in, 1 out]
        n734 = property on="Intensity Graph" class="IntGraph (strict)"("PlotImages.Front"=w1794) -> ()  [unwired: 2 in, 2 out]
      }
      event "Clear emitters": Value Change {
        n735 = event-data() -> ()  [unwired: 1 in, 6 out]
        n736 = property on="Intensity Graph" class="IntGraph (strict)"("PlotImages.Front"=picture data[5B] ("Plot Images:Front")) -> ()  [unwired: 2 in, 2 out]
        n737 = local write "User Selected Measurement Points"(dbl[][] [] ("Autospectra Positions")) -> ()
      }
      event "Intensity Graph": Mouse Down {
        # "Help me find emitters boolean"
        # "If the user clicks on an NV of interest,\nput its coordinates into the position target\ncontrols.  Note this does not start\nthe motion.\n\nAlso, put the current Z position into the\nZ target control, so clicking on the\nGo button doesn't cause any motion\nin Z."
        n738 = event-data() -> ("CtlRef"=w1816:refnum<vi>, "Coords"=w1807:T18)  [unwired: 1 in, 6 out]
        n739 = Index Array(array=w1819, index=2) -> (element=w1817:dbl)
        n740 = local write "Z"(w1817) -> ()
        n741 = local read "Help me find emitters!"() -> (w1799:bool)
        n742 = local read "User Selected Measurement Points"() -> (w1800:dbl[][])
        n743 = local read "Pick candidates"() -> (w1808:bool)
        n744 = property on="Intensity Graph" class="IntGraph (strict)"() -> ("Plot Bounds"=w1812:T19)  [unwired: 2 in, 2 out]
        n745 = Unbundle(w1812) -> ("Left"=w1811:i16, "Top"=w1810:i16)  [unwired: 2 out]
        n746 = invoke class="IntGraph (strict)" method="Map Coords To XY"(reference=w1816, error in=w1814, "Coords"=w1807) -> (error out=w1813:errorcluster, "XY"=w1815:cluster{"X":dbl, "Y":dbl})  [unwired: 4 in, 5 out]
        n747 = Unbundle By Name(w1815) -> ("X"=w1804:dbl, "Y"=w1803:dbl)
        n748 = local write "X"(w1804) -> ()
        n749 = local write "Y"(w1803) -> ()
        n750 = local write "X Center"(w1804) -> ()
        n751 = Build Array(w1804, w1803) -> (w1802:dbl[])
        n752 = Insert Into Array(array=w1800, new element=w1802) -> (→"User Selected Measurement Points":dbl[][])  [unwired: 2 in]
        n753 = local write "Y Center"(w1803) -> ()
        n754 = Bundle("Left"=w1811, "Top"=w1810) -> (w1806:cluster{"Left":i16, "Top":i16})  [unwired: 1 in]
        n755 = case shown="True" w1799 {
          tunnel: w1813 -> [w1830 w1839]
          tunnel: [w1830 w1839] -> w1809
          tunnel: w1807 -> [_ w1833]
          tunnel: w1806 -> [_ w1831]
          frame False {
          }
          frame True {
            n756 = Subtract(x=w1833, y=w1831) -> (x-y=w1832:T18)
            n757 = property on="Intensity Graph" class="IntGraph (strict)"() -> ("PlotImages.Front"=w1838:picture)  [unwired: 2 in, 2 out]
            n758 = call <vilib>:"Draw Circle by Radius.vi"("pen"=T13 {"Width"=1, "Style"=enum."Solid"}, "color(black)"=u32 16716306, "pixel center"=w1832, "radius"=6, "picture"=w1838) -> ("new picture"=w1837:picture)  [unwired: 6 in]
            n759 = property on="Intensity Graph" class="IntGraph (strict)"("PlotImages.Front"=w1837) -> ()  [unwired: 2 in, 2 out]
          }
        }
        n760 = case shown="True" w1808 {
          tunnel: w1809 -> [w1820 w1829]
          tunnel: [w1820 w1829] -> w1805
          tunnel: w1807 -> [_ w1825]
          tunnel: w1806 -> [_ w1823]
          frame False {
          }
          frame True {
            n761 = Subtract(x=w1825, y=w1823) -> (x-y=w1824:T18)
            n762 = property on="Intensity Graph" class="IntGraph (strict)"() -> ("PlotImages.Front"=w1822:picture)  [unwired: 2 in, 2 out]
            n763 = call <vilib>:"Draw Circle by Radius.vi"("pen"=T13 {"Width"=2, "Style"=enum."Solid"}, "color(black)"=u32 4436992, "pixel center"=w1824, "radius"=6, "picture"=w1822) -> ("new picture"=w1821:picture)  [unwired: 6 in]
            n764 = property on="Intensity Graph" class="IntGraph (strict)"("PlotImages.Front"=w1821) -> ()  [unwired: 2 in, 2 out]
          }
        }
      }
      event "Clear auto spectra positions": Value Change {
        n765 = event-data() -> ()  [unwired: 1 in, 6 out]
        n766 = property on="Intensity Graph" class="IntGraph (strict)"("PlotImages.Front"=picture data[5B] ("Plot Images:Front")) -> ()  [unwired: 2 in, 2 out]
        n767 = local write "User Selected Measurement Points"(dbl[][] [] ("Autospectra Positions")) -> ()
      }
      event "Clear Last Select Point": Mouse Down {
        n768 = event-data() -> ()  [unwired: 1 in, 8 out]
        n769 = local read "User Selected Measurement Points"() -> (w1845:dbl[][])
        n770 = disable-structure shown="Disabled" {
          frame Disabled {
            n771 = property on="Intensity Graph" class="IntGraph (strict)"() -> ("PlotImages.Front"=w1847:picture)  [unwired: 2 in, 2 out]
            n772 = call <vilib>:"Draw Circle by Radius.vi"("pen"=T13 {"Width"=1, "Style"=enum."Solid"}, "color(black)"=u32 3684408, "radius"=6, "picture"=w1847) -> ("new picture"=w1851:picture, "pixel center"=w1846:cluster{"horizontal":i16, "vertical":i16})  [unwired: 6 in]
            n773 = property on="Property Node" class="IntGraph (strict)"("PlotImages.Front"=w1851) -> ()  [unwired: 2 in, 2 out]
          }
          frame Enabled {
          }
        }
        n774 = Delete From Array(array=w1845) -> (deleted portion=→"deleted portion":dbl[], array with subset deleted=w1844:dbl[][])  [unwired: 3 in]
        n775 = local write "User Selected Measurement Points"(w1844) -> ()
      }
      event "Clear Last Filter Position": Mouse Down {
        n776 = event-data() -> ()  [unwired: 1 in, 8 out]
        n777 = local read "Filter Positions"() -> (w1853:dbl[])
        n778 = Delete From Array(array=w1853) -> (array with subset deleted=w1852:dbl[])  [unwired: 2 in, 1 out]
        n779 = local write "Filter Positions"(w1852) -> ()
      }
      event "XY Scan": Value Change {
        n780 = event-data() -> ("CtlRef"=w1858:refnum<vi>, "NewVal"=w1855:bool)  [unwired: 1 in, 4 out]
        n781 = case shown="True" w1855 {
          tunnel: w1857 -> [w1861 w1894]
          tunnel: [w1861 w1867] -> w1856
          tunnel: w1858 -> [w1862 w1895]
          tunnel: [w1862 w1895] -> w1860
          tunnel: w1854 -> [_ w1893]
          frame False {
          }
          frame True {
            n782 = flat-sequence {
              tunnel: w1894 -> [w1907]
              tunnel: [w1907] -> w1866
              frame #0 {
                n783 = local write "Emitter #"(0.0 ("Emitter #")) -> ()
                n784 = local write "Motion"(TRUE ("Motion")) -> ()
              }
            }
            n785 = local read "Current Map"() -> (w1891:dbl[][])
            n786 = local read "X-frequency"() -> (w1875:dbl)
            n787 = local read "Table rate"() -> (w1882:i32)
            n788 = local read "Scan Type"() -> (w1880:enum16{"Sinusoidal", "Spiral"})
            n789 = local read "Buffering"() -> (w1892:bool)
            n790 = local read "Y-velocity"() -> (w1874:dbl)
            n791 = local read "X Center"() -> (w1864:dbl)
            n792 = local read "Y Center"() -> (w1863:dbl)
            n793 = local read "Y Range"() -> (w1878:dbl)
            n794 = local read "X Range"() -> (w1877:dbl)
            n795 = local write "Last Scan Y"(w1863) -> ()
            n796 = local write "Last Scan X"(w1864) -> ()
            n797 = Divide(x=w1878, y=2.0) -> (x/y=w1886:dbl)
            n798 = Divide(x=w1877, y=2.0) -> (x/y=w1885:dbl)
            n799 = local read "Scan Termination"() -> (w1872:T6)
            n800 = local read "Buffered Map"() -> (w1889:dbl[][])
            n801 = local read "Analog Input"() -> (w1881:i32)
            n802 = case shown="\"Center of scan\"" w1872 {
              selector: w1872 -> [w1897 w1899 _]
              tunnel: [w1897 w1899 T14."End Position" ("Scan Termination")] -> w1871
              tunnel: [FALSE FALSE TRUE] -> w1870
              frame "Maximum", Default {
              }
              frame "End Position" {
              }
              frame "Center of scan" {
              }
            }
            n803 = Subtract(x=w1863, y=w1886) -> (x-y=w1884:dbl)
            n804 = Subtract(x=w1864, y=w1885) -> (x-y=w1883:dbl)
            n805 = case shown="True" w1892 {
              tunnel: w1891 -> [_ w1905]
              tunnel: [w1903 w1905] -> w1890
              tunnel: w1889 -> [w1903 _]
              tunnel: w1866 -> [w1902 w1904]
              tunnel: [w1902 w1904] -> w1876
              frame False {
              }
              frame True {
              }
            }
            n806 = local write "Buffered Map"(w1890) -> ()
            n807 = local read "Mesh"() -> (w1879:dbl)
            n808 = call "Area_Scan_v12 (SubVI).vi"("Step Axis"="2", "Scan Termination"=w1871, "Center of Scan"=w1870, "Scan Type"=w1880, "Analog Input"=w1881, "Table rate"=w1882, "System no."=w1893, "error in (no error)"=w1876, "Mesh in"=w1879, "X-frequency"=w1875, "X Scan Range"=w1877, "Y-velocity"=w1874, "Y Scan Range"=w1878, "X Scan Center"=w1864, "Y Scan Center"=w1863) -> ("Intensity Graph"=w1865:dbl[][], "Nano AS Data"=w1868:dbl[][], "AS Duration (msec)"=w1869:u32, "error out"=w1867:errorcluster)  [unwired: 8 in, 1 out]
            n809 = local write "Current Map"(w1865) -> ()
            n810 = local write "Intensity Graph"(w1865) -> ()
            n811 = local write "Nano AS Data"(w1868) -> ()
            n812 = local write "AS Duration (msec)"(w1869) -> ()
            n813 = property on="Intensity Graph" class="IntGraph (strict)"(error in=w1867, "XScale.Multiplier"=w1879, "YScale.Multiplier"=w1879, "XScale.Offset"=w1883, "YScale.Offset"=w1884) -> ()  [unwired: 1 in, 2 out]
          }
        }
        n814 = property class="Bool (strict)"(reference=w1860, "Value"=FALSE) -> ()  [unwired: 1 in, 2 out]
      }
      event "Restore center": Mouse Down {
        n815 = event-data() -> ()  [unwired: 1 in, 8 out]
        n816 = local read "Last Scan X"() -> (w1911:dbl)
        n817 = local read "Last Scan Y"() -> (w1910:dbl)
        n818 = local write "X Center"(w1911) -> ()
        n819 = local write "Y Center"(w1910) -> ()
      }
      event "Align Scan": Value Change {
        n820 = event-data() -> ("CtlRef"=w1914:refnum<vi>, "NewVal"=w1913:bool)  [unwired: 1 in, 4 out]
        n821 = case shown="True" w1913 {
          tunnel: w1915 -> [w1920 w1931]
          tunnel: [w1920 w1938] -> w1912
          tunnel: w1914 -> [w1919 w1993]
          tunnel: [w1919 w1993] -> w1918
          tunnel: w1916 -> [_ w1927]
          frame False {
          }
          frame True {
            # "fine XY scan for\naccurate XY alignment"
            # "XZ scan averaged over X\nproduces Z-dependent intensity profile\n\nThen the stage is positioned at Z location\nwith maximum counts"
            # "Gradient search routine\nfor high speed\napproximate XY alignment"
            n822 = flat-sequence {
              tunnel: w1931 -> [w2011]
              tunnel: [w2011] -> w1982
              frame #0 {
                n823 = local write "Emitter #"(0.0 ("Emitter #")) -> ()
                n824 = local write "Motion"(TRUE ("Motion")) -> ()
              }
            }
            n825 = local read "Current Map"() -> (w1991:dbl[][])
            n826 = local read "Speed factor"() -> (w1946:dbl)
            n827 = local read "Z-frequency"() -> (w1954:dbl)
            n828 = local read "Max velocity"() -> (w1947:dbl)
            n829 = local read "A-frequency"() -> (w1961:dbl)
            n830 = local read "Max Radius"() -> (w1950:dbl)
            n831 = local read "Min Radius"() -> (w1949:dbl)
            n832 = local read "Scan Type"() -> (w1978:enum16{"Sinusoidal", "Spiral"})
            n833 = local read "Table rate"() -> (w1976:i32)
            n834 = local read "Scan Type"() -> (w1972:enum16{"Sinusoidal", "Spiral"})
            n835 = local read "Table rate"() -> (w1970:i32)
            n836 = local read "A-velocity"() -> (w1962:dbl)
            n837 = local read "Buffering"() -> (w1992:bool)
            n838 = local read "Z-velocity"() -> (w1955:dbl)
            n839 = local read "ZX range"() -> (w1960:dbl)
            n840 = local read "Tracking"() -> (w1952:bool)
            n841 = local read "Z range"() -> (w1958:dbl)
            n842 = local read "Z range"() -> (w1963:dbl)
            n843 = local read "Z Mesh"() -> (w1959:dbl)
            n844 = local read "Z Mesh"() -> (w1964:dbl)
            n845 = local read "Align XY Mesh"() -> (w1956:dbl)
            n846 = local read "Scan Termination"() -> (w1979:T6)
            n847 = local read "Max. dir. changes"() -> (w1945:i32)
            n848 = local read "Scan Termination"() -> (w1973:T6)
            n849 = local read "Align XY range"() -> (w1935:dbl)
            n850 = local read "Align XY range"() -> (w1968:dbl)
            n851 = local read "Align XY Mesh"() -> (w1942:dbl)
            n852 = local read "GS Frequency"() -> (w1951:dbl)
            n853 = local read "Buffered Map"() -> (w1989:dbl[][])
            n854 = local read "Analog Input"() -> (w1953:i32)
            n855 = local read "Analog Input"() -> (w1977:i32)
            n856 = local read "Analog Input"() -> (w1971:i32)
            n857 = local read "Z"() -> (w1957:dbl)
            n858 = case shown="\"Center of scan\"" w1979 {
              selector: w1979 -> [w2001 w2003 _]
              tunnel: [w2001 w2003 T6."End Position" ("Scan Termination")] -> w1965
              tunnel: [FALSE FALSE TRUE] -> w1981
              frame "Maximum", Default {
              }
              frame "End Position" {
              }
              frame "Center of scan" {
              }
            }
            n859 = case shown="\"Center of scan\"" w1973 {
              selector: w1973 -> [w1995 w1997 _]
              tunnel: [w1995 w1997 T14."End Position" ("Scan Termination")] -> w1975
              tunnel: [FALSE FALSE TRUE] -> w1974
              frame "Maximum", Default {
              }
              frame "End Position" {
              }
              frame "Center of scan" {
              }
            }
            n860 = case shown="False" w1992 {
              tunnel: w1991 -> [_ w2009]
              tunnel: [w2007 w2009] -> w1990
              tunnel: w1989 -> [w2007 _]
              tunnel: w1982 -> [w2006 w2008]
              tunnel: [w2006 w2008] -> w1944
              frame False {
              }
              frame True {
              }
            }
            n861 = Divide(x=w1935, y=2.0) -> (x/y=w1985:dbl)
            n862 = Divide(x=w1935, y=2.0) -> (x/y=w1986:dbl)
            n863 = local write "Buffered Map"(w1990) -> ()
            n864 = local read "ML"() -> (w1948:dbl)
            n865 = call "Gradient_Search_v12 (SubVI).vi"("Speed factor"=w1946, "Max velocity"=w1947, "ML"=w1948, "Min Radius"=w1949, "Max Radius"=w1950, "GS Frequency"=w1951, "Max. dir. changes"=w1945, "error in (no error)"=w1944, "Analog Input"=w1953, "Run?"=TRUE, "System no."=w1927, "Tracking"=w1952) -> ("error out"=w1941:errorcluster)  [unwired: 7 in]
            n866 = call "General wait for movement to stop.vi"("System no."=w1927, "Additional wait time, ms"=3000, "error in"=w1941, "Polling cycle \ntime, ms"=1) -> ("error out"=w1929:errorcluster)  [unwired: 4 in, 11 out]
            n867 = call "POS?.vi"("System no."=w1927, "All axes?"=TRUE, "error in"=w1929) -> ("Position"=w1926:dbl[], "error out"=w1928:errorcluster)  [unwired: 2 in, 13 out]
            n868 = Index Array(array=w1926, index=1) -> (element=w1922:dbl)
            n869 = Index Array(array=w1926, index=0) -> (element=w1921:dbl)
            n870 = Subtract(x=w1922, y=w1986) -> (x-y=w1984:dbl)
            n871 = Subtract(x=w1921, y=w1985) -> (x-y=w1983:dbl)
            n872 = local read "Z"() -> (w1967:dbl)
            n873 = call "Z_Scan_v12 (SubVI).vi"("Scan Axis"="3", "Scan Termination"=w1965, "Center of Scan"=w1981, "Scan Type"=w1978, "Analog Input"=w1977, "Table rate"=w1976, "System no."=w1927, "error in (no error)"=w1928, "Z Mesh"=w1964, "Z-frequency"=w1954, "X Scan Range"=w1960, "Z-velocity"=w1955, "Z Scan Range"=w1963, "X Scan Center"=w1921, "Z Scan Center"=w1967) -> ("Intensity Graph"=w1934:dbl[][], "error out"=w1933:errorcluster)  [unwired: 8 in, 3 out]
            n874 = call "Z_Alignment_v12 (SubVI).vi"("System no."=w1927, "Z range"=w1958, "Intensity Graph"=w1934, "Z Mesh"=w1959, "error in (no error)"=w1933, "Z"=w1957, "Y"=w1922, "X"=w1921) -> ("error out"=w1966:errorcluster, "Zout"=w1923:dbl)  [unwired: 2 in]
            n875 = call "Area_Scan_v12 (SubVI).vi"("Step Axis"="2", "Scan Termination"=w1975, "Center of Scan"=w1974, "Scan Type"=w1972, "Analog Input"=w1971, "Table rate"=w1970, "System no."=w1927, "error in (no error)"=w1966, "Mesh in"=w1942, "X-frequency"=w1961, "X Scan Range"=w1935, "Y-velocity"=w1962, "Y Scan Range"=w1935, "X Scan Center"=w1921, "Y Scan Center"=w1922) -> ("Intensity Graph"=w1936:dbl[][], "error out"=w1932:errorcluster)  [unwired: 8 in, 3 out]
            n876 = property on="Alignment Graph" class="IntGraph (strict)"(error in=w1932, "XScale.Multiplier"=w1942, "YScale.Multiplier"=w1942, "XScale.Offset"=w1983, "YScale.Offset"=w1984) -> ()  [unwired: 1 in, 2 out]
            n877 = call "Smoothing_Alignment_v12 (SubVI).vi"("X center"=w1921, "Intensity Graph"=w1936, "Y center"=w1922, "Mesh"=w1956, "X Scan Range"=w1968, "Y Scan Range"=w1968, "Z"=w1923, "System no."=w1927, "error in (no error)"=w1932) -> ("Alignment Graph"=w1937:dbl[][], "error out"=w1938:errorcluster)  [unwired: 5 in]
            n878 = local write "Alignment Graph"(w1937) -> ()
          }
        }
        n879 = property class="Bool (strict)"(reference=w1918, "Value"=FALSE) -> ()  [unwired: 1 in, 2 out]
      }
      event "Fine Align": Value Change {
        n880 = event-data() -> ("NewVal"=w2016:bool)  [unwired: 1 in, 5 out]
        n881 = case shown="True" w2016 {
          tunnel: w2015 -> [w2018 w2026]
          tunnel: [w2018 w2025] -> w2014
          tunnel: w2013 -> [w2017 w2024]
          tunnel: [w2017 _] -> _
          frame False {
          }
          frame True {
            n882 = local read "Scan Termination"() -> (w2023:T6)
            n883 = call "AUTOFLIM_Fine_Alignment.vi"("System no."=w2024, "Scan Termination"=w2023, "error in"=w2026) -> ("Mesh out"=w2021:dbl, "Numeric 2"=w2020:dbl, "Numeric"=w2019:dbl, "Alignment Array Out"=w2022:dbl[][], "error out"=w2025:errorcluster)  [unwired: 8 in]
            n884 = property on="Alignment Graph" class="IntGraph (strict)"("XScale.Multiplier"=w2021, "YScale.Multiplier"=w2021, "XScale.Offset"=w2020, "YScale.Offset"=w2019) -> ()  [unwired: 2 in, 2 out]
            n885 = local write "Alignment Graph"(w2022) -> ()
          }
        }
      }
      event "Map Switch": Value Change {
        n886 = event-data() -> ("NewVal"=w2027:bool)  [unwired: 1 in, 5 out]
        n887 = case shown="True" w2027 {
          frame False {
            n888 = local read "Buffered Map"() -> (w2029:dbl[][])
            n889 = local write "Intensity Graph"(w2029) -> ()
          }
          frame True {
            n890 = local read "Current Map"() -> (w2030:dbl[][])
            n891 = local write "Intensity Graph"(w2030) -> ()
          }
        }
      }
      event "Write Alignment map to file": Mouse Down {
        n892 = event-data() -> ()  [unwired: 1 in, 8 out]
        n893 = local read "Alignment Graph"() -> (w2032:dbl[][])
        n894 = Multiply(x=w2032, y=1000.0) -> (x*y=w2033:dbl[][])
        n895 = Round To Nearest(number=w2033) -> (nearest integer value=w2036:dbl[][])
        n896 = To Word Integer(number=w2036) -> (16bit integer=w2035:i16[][])
        n897 = call-poly <vilib>:"Write Delimited Spreadsheet.vi"("2D data"=w2035, "append to file? (new file:F)"=FALSE, "transpose? (no:F)"=TRUE, "delimiter (\\t)"="" ("delimiter (\\t)")) -> ()  [unwired: 10 in, 2 out]
      }
      event "String To Send": Value Change {
        # "This frame responds to user inputs in the terminal-- very handy. \n\nNote the terminal can also be used via the parser!  This means you\ncan issue commands and perform sequences even of functionalities\nthat have not been programmed-into this GUI."
        # "is a query"
        n898 = event-data() -> ("CtlRef"=w2043:refnum<vi>, "NewVal"=w2048:string)  [unwired: 1 in, 4 out]
        n899 = Match Pattern(string=w2048, regular expression="[?]") -> (offset past match=w2052:i32)  [unwired: 1 in, 3 out]
        n900 = Concatenate Strings(">>" ("regular expression"), w2048, "\r\n") -> (w2055:string)
        n901 = Not Equal?(x=w2048, y="") -> (x != y?=w2049:bool)
        n902 = local read "Controls"() -> (w2046:enum32{"Operation", "Parameters", "Setup"})
        n903 = Greater Or Equal To 0?(x=w2052) -> (x >= 0?=w2053:bool)
        n904 = Equal?(x=w2046, y=enum32{"Operation", "Parameters", "Setup"}."Setup" ("Controls")) -> (x = y?=w2059:bool)
        n905 = case shown="True" w2049 {
          tunnel: w2040 -> [_ w2072]
          tunnel: w2047 -> [w2063 w2071]
          tunnel: [w2063 w2070] -> w2057
          tunnel: w2053 -> [_ w2069]
          tunnel: [w2060 w2068] -> w2042
          tunnel: [w2062 w2067] -> w2041
          tunnel: w2048 -> [w2062 w2066]
          tunnel: [w2061 w2064] -> w2044
          tunnel: w2055 -> [_ w2065]
          tunnel: w2059 -> [w2061 w2064]
          frame False {
            n906 = local read "Received String"() -> (w2060:string)
          }
          frame True {
            n907 = call "PI Send String.vi"("System no."=w2072, "String to send"=w2066, "error in"=w2071) -> ("error out"=w2073:errorcluster)  [unwired: 16 in]
            n908 = case shown="False" w2069 {
              tunnel: w2073 -> [w2076 w2083]
              tunnel: w2072 -> [_ w2082]
              tunnel: [w2076 w2081] -> w2070
              tunnel: [w2074 w2077] -> w2068
              tunnel: ["" ""] -> w2067
              tunnel: w2065 -> [w2074 w2079]
              frame False {
              }
              frame True {
                # "Receive only if Query button\nwas pressed"
                n909 = call "PI Receive String.vi"("System no."=w2082, "error in"=w2083) -> ("String read"=w2078:string, "error out"=w2081:errorcluster)  [unwired: 15 in, 1 out]
                n910 = Concatenate Strings(w2079, w2078) -> (w2077:string)
              }
            }
          }
        }
        n911 = property class="Str"(reference=w2043, "Key Focus"=w2044) -> ()  [unwired: 1 in, 2 out]
        n912 = local write "Received String"(w2042) -> ()
        n913 = local write "String To Send"(w2041) -> ()
        n914 = call "ERR?.vi"("System no."=w2040, "error in"=w2057) -> ("error out"=w2058:errorcluster)  [unwired: 16 in, 1 out]
        n915 = flat-sequence {
          tunnel: w2058 -> [_]
          frame #0 {
            # "ignore error"
          }
        }
      }
      event "PL scan contrast limits": Value Change {
        n916 = event-data() -> ()  [unwired: 1 in, 6 out]
        n917 = local read "PL scan contrast limits"() -> (w2087:dbl[])
        n918 = Index Array(array=w2087, index=0) -> (element=w2088:dbl)
        n919 = Index Array(array=w2087, index=1) -> (element=w2086:dbl)
        n920 = property on="Intensity Graph" class="IntGraph (strict)"("ZScale.Minimum"=w2088, "ZScale.Maximum"=w2086) -> ()  [unwired: 2 in, 2 out]
      }
      event "Alignment limits": Value Change {
        n921 = event-data() -> ()  [unwired: 1 in, 6 out]
        n922 = local read "Alignment limits"() -> (w2090:dbl[])
        n923 = Index Array(array=w2090, index=0) -> (element=w2091:dbl)
        n924 = Index Array(array=w2090, index=1) -> (element=w2092:dbl)
        n925 = property on="Alignment Graph" class="IntGraph (strict)"("ZScale.Minimum"=w2091, "ZScale.Maximum"=w2092) -> ()  [unwired: 2 in, 2 out]
      }
      event "Correct map": Value Change {
        n926 = event-data() -> ("NewVal"=w2097:bool)  [unwired: 1 in, 5 out]
        n927 = case shown="True" w2097 {
          tunnel: w2098 -> [w2100 w2104]
          tunnel: [w2100 w2103] -> w2096
          frame False {
            n928 = local read "Map Switch"() -> (w2099:bool)
            n929 = case shown="True" w2099 {
              frame False {
                n930 = local read "Buffered Map"() -> (w2101:dbl[][])
                n931 = local write "Intensity Graph"(w2101) -> ()
              }
              frame True {
                n932 = local read "Current Map"() -> (w2102:dbl[][])
                n933 = local write "Intensity Graph"(w2102) -> ()
              }
            }
          }
          frame True {
            n934 = local read "Map Switch"() -> (w2108:bool)
            n935 = case shown="False" w2108 {
              tunnel: [w2111 w2112] -> w2107
              frame False {
                n936 = local read "Buffered Map"() -> (w2111:dbl[][])
              }
              frame True {
                n937 = local read "Current Map"() -> (w2112:dbl[][])
              }
            }
            n938 = local read "Correction type"() -> (w2106:i16)
            n939 = script code="B = A * 0; % Initialize output matrix with zeros\n\n% Replace non-positive values with the overall mean of A\nA(A <= 0) = mean(A(:));\n\nif whichcorrection == 0\n    for i = 1:size(A, 2)\n        line = A(:, i); % Corrected indexing\n        B(:, i) = line - median(line);\n    end\nelseif whichcorrection == 1\n    Xcoord = 1:size(A, 1); % Xcoord should match row dimension\n    for i = 1:size(A, 2)\n        line = A(:, i); % Corrected indexing\n        COEFFS = polyfit(Xcoord', line, 1);\n        B(:, i) = line - (COEFFS(1) * Xcoord' + COEFFS(2));\n    end\nend"("??"=w2104, "A"=w2107, "whichcorrection"=w2106) -> ("??"=w2103:errorcluster, "B"=w2105:cdb[][])
            n940 = local write "Intensity Graph"(w2105) -> ()
            n941 = case shown="True" w2108 {
              tunnel: w2105 -> [w2109 w2110]
              frame False {
                n942 = local write "Buffered MapCorr"(w2109) -> ()
              }
              frame True {
                n943 = local write "Current MapCorr"(w2110) -> ()
              }
            }
          }
        }
      }
      event "Abs. Move": Value Change {
        # "If the Abs. Move button has been pressed, move to the desired XYZ position."
        n944 = event-data() -> ("CtlRef"=w2115:refnum<vi>, "NewVal"=w2119:bool)  [unwired: 1 in, 4 out]
        n945 = case shown="True" w2119 {
          tunnel: w2118 -> [w2121 w2130]
          tunnel: [w2121 w2129] -> w2117
          tunnel: w2116 -> [_ w2128]
          tunnel: w2115 -> [w2120 w2123]
          tunnel: [w2120 w2123] -> w2114
          frame False {
          }
          frame True {
            n946 = local read "X"() -> (w2126:dbl)
            n947 = local read "Y"() -> (w2125:dbl)
            n948 = local read "Z"() -> (w2122:dbl)
            n949 = Build Array(w2126, w2125, w2122) -> (w2124:dbl[])
            n950 = call "MOV.vi"("System no."=w2128, "Axes to move"=string[] ["1", "2", "3"], "Position values"=w2124, "error in"=w2130) -> ("error out"=w2129:errorcluster)  [unwired: 1 in, 14 out]
          }
        }
        n951 = property class="Bool (strict)"(reference=w2114, "Value"=FALSE) -> ()  [unwired: 1 in, 2 out]
      }
      event "HOME": Mouse Down {
        # "If the Abs. Move button has been pressed, move to the desired XYZ position."
        n952 = event-data() -> ("CtlRef"=w2133:refnum<vi>, "Button"=w2137:u16)  [unwired: 1 in, 6 out]
        n953 = case shown="1" w2137 {
          tunnel: w2136 -> [w2139 w2146]
          tunnel: [w2139 w2145] -> w2135
          tunnel: w2134 -> [_ w2144]
          tunnel: w2133 -> [w2138 w2141]
          tunnel: [w2138 w2141] -> w2132
          frame 0, Default {
          }
          frame 1 {
            w2140 = 50.0 ("element")
            n954 = local write "X"(w2140) -> ()
            n955 = local write "Y"(w2140) -> ()
            n956 = local write "Z"(w2140) -> ()
            n957 = local write "X Center"(w2140) -> ()
            n958 = local write "Y Center"(w2140) -> ()
            n959 = Build Array(w2140, w2140, w2140) -> (w2142:dbl[])
            n960 = call "MOV.vi"("System no."=w2144, "Axes to move"=string[] ["1", "2", "3"], "Position values"=w2142, "error in"=w2146) -> ("error out"=w2145:errorcluster)  [unwired: 1 in, 14 out]
          }
        }
        n961 = property class="Bool (strict)"(reference=w2132, "Value"=FALSE) -> ()  [unwired: 1 in, 2 out]
      }
      event "Next emitter": Value Change {
        # "If the Abs. Move button has been pressed, move to the desired XYZ position."
        n962 = event-data() -> ("CtlRef"=w2149:refnum<vi>, "NewVal"=w2153:bool)  [unwired: 1 in, 4 out]
        n963 = case shown="True" w2153 {
          tunnel: w2152 -> [w2155 w2170]
          tunnel: [w2155 w2163] -> w2151
          tunnel: w2150 -> [_ w2169]
          tunnel: w2149 -> [w2154 w2168]
          tunnel: [w2154 w2168] -> w2148
          frame False {
          }
          frame True {
            n964 = property on="Intensity Graph" class="IntGraph (strict)"() -> ("XScale.Offset"=w2166:dbl, "YScale.Offset"=w2165:dbl)  [unwired: 2 in, 2 out]
            n965 = local read "Emitter #"() -> (w2158:i32)
            n966 = Increment(x=w2158) -> (x+1=w2157:i32)
            n967 = local read "Mesh"() -> (w2164:dbl)
            n968 = local read "cent"() -> (w2162:i32[][])
            n969 = local read "Z"() -> (w2167:dbl)
            n970 = call "AUTOFLIM_move_to_emitter.vi"("Mesh"=w2164, "YScale.Offset"=w2165, "XScale.Offset"=w2166, "cent"=w2162, "Drift"=dbl[] [0.0, 0.0], "System no."=w2169, "error in (no error)"=w2170, "Z"=w2167, "Emitter # in"=w2157) -> ("Numeric 2"=w2161:dbl, "Numeric"=w2160:dbl, "Emitter # out"=w2159:i32, "error out"=w2163:errorcluster)  [unwired: 2 in, 1 out]
            n971 = local write "X"(w2161) -> ()
            n972 = local write "Y"(w2160) -> ()
            n973 = local write "Emitter #"(w2159) -> ()
          }
        }
        n974 = property class="Bool (strict)"(reference=w2148, "Value"=FALSE) -> ()  [unwired: 1 in, 2 out]
      }
      event "east", "west", "south", "north", "up", "down": Mouse Down {
        # "If one of the increment buttons has been pressed, increment the XYZ position."
        n975 = event-data() -> ("CtlRef"=w2174:refnum<vi>)  [unwired: 1 in, 7 out]
        n976 = property class="Bool (strict)"(reference=w2174) -> ("Label.Text"=w2171:string)  [unwired: 1 in, 2 out]
        n977 = Equal?(x="east", y=w2171) -> (x = y?=w2183:bool)
        n978 = Equal?(x="west", y=w2171) -> (x = y?=w2180:bool)
        n979 = Equal?(x="north", y=w2171) -> (x = y?=w2178:bool)
        n980 = Equal?(x="south", y=w2171) -> (x = y?=w2179:bool)
        n981 = Equal?(x="down", y=w2171) -> (x = y?=w2182:bool)
        n982 = Equal?(x="up", y=w2171) -> (x = y?=w2181:bool)
        n983 = flat-sequence {
          tunnel: w2183 -> [w2219]
          tunnel: w2182 -> [w2218]
          tunnel: w2181 -> [w2217]
          tunnel: w2180 -> [w2216]
          tunnel: w2179 -> [w2215]
          tunnel: w2178 -> [w2214]
          tunnel: w2177 -> [w2207]
          tunnel: w2176 -> [w2206]
          tunnel: [w2204] -> w2172
          tunnel: w2174 -> [w2203]
          tunnel: [w2203] -> w2173
          frame #0 {
            n984 = case shown="True" w2219 {
              tunnel: [w2260 w2264] -> w2213
              frame False {
                n985 = Build Array(0.0, 0.0, 0.0) -> (w2260:dbl[])
              }
              frame True {
                n986 = Build Array(0.025, 0.0, 0.0) -> (w2264:dbl[])
              }
            }
            n987 = case shown="True" w2216 {
              tunnel: [w2252 w2256] -> w2212
              frame False {
                n988 = Build Array(0.0, 0.0, 0.0) -> (w2252:dbl[])
              }
              frame True {
                n989 = Build Array(-0.025, 0.0, 0.0) -> (w2256:dbl[])
              }
            }
            n990 = case shown="True" w2215 {
              tunnel: [w2244 w2248] -> w2211
              frame False {
                n991 = Build Array(0.0, 0.0, 0.0) -> (w2244:dbl[])
              }
              frame True {
                n992 = Build Array(0.0, -0.025, 0.0) -> (w2248:dbl[])
              }
            }
            n993 = case shown="True" w2214 {
              tunnel: [w2236 w2240] -> w2210
              frame False {
                n994 = Build Array(0.0, 0.0, 0.0) -> (w2236:dbl[])
              }
              frame True {
                n995 = Build Array(0.0, 0.025, 0.0) -> (w2240:dbl[])
              }
            }
            n996 = case shown="True" w2218 {
              tunnel: [w2228 w2232] -> w2209
              frame False {
                n997 = Build Array(0.0, 0.0, 0.0) -> (w2228:dbl[])
              }
              frame True {
                n998 = Build Array(0.0, 0.0, -0.05) -> (w2232:dbl[])
              }
            }
            n999 = case shown="True" w2217 {
              tunnel: [w2220 w2224] -> w2208
              frame False {
                n1000 = Build Array(0.0, 0.0, 0.0) -> (w2220:dbl[])
              }
              frame True {
                n1001 = Build Array(0.0, 0.0, 0.05) -> (w2224:dbl[])
              }
            }
            n1002 = Compound Arithmetic op=ADD(w2213, w2212, w2211, w2210, w2209, w2208) -> (w2202:dbl[])
            n1003 = call "MVR.vi"("System no."=w2207, "Axes to move"=string[] ["1", "2", "3"], "Position values"=w2202, "error in"=w2206) -> ("error out"=w2204:errorcluster)  [unwired: 15 in]
            n1004 = Index Array(array=w2202, index=1) -> (element=w2197:dbl)
            n1005 = Index Array(array=w2202, index=2) -> (element=w2194:dbl)
            n1006 = Index Array(array=w2202, index=0) -> (element=w2198:dbl)
            n1007 = local read "Y"() -> (w2195:dbl)
            n1008 = local read "Z"() -> (w2192:dbl)
            n1009 = local read "X"() -> (w2196:dbl)
            n1010 = Add(x=w2195, y=w2197) -> (x+y=w2191:dbl)
            n1011 = Add(x=w2192, y=w2194) -> (x+y=w2193:dbl)
            n1012 = Add(x=w2196, y=w2198) -> (x+y=w2190:dbl)
            n1013 = local write "Y"(w2191) -> ()
            n1014 = local write "Z"(w2193) -> ()
            n1015 = local write "X"(w2190) -> ()
            n1016 = local write "Y Center"(w2191) -> ()
            n1017 = local write "X Center"(w2190) -> ()
          }
        }
        n1018 = property class="Bool (strict)"(reference=w2173, "Value"=FALSE) -> ()  [unwired: 1 in, 2 out]
      }
      event "stop": Value Change {
        n1019 = event-data() -> ()  [unwired: 1 in, 6 out]
      }
    }
    n1020 = Compound Arithmetic op=OR(w189, w184) -> (w188:bool)
  }
  n1021 = flat-sequence {
    tunnel: [w2285] -> w24
    tunnel: [w2275] -> w23
    tunnel: [w2272] -> w54
    tunnel: [w2271] -> w53
    tunnel: [w2270] -> _
    frame #0 {
      # "Event Loop"
      # "Thorlabs Flipper Motors Initialization (mirrors)"
      n1022 = property class="FilterFlipperControl"(reference="FilterFlipperControl 2", error in=errorcluster {"status"=FALSE, "code"=0, "source"=""} ("error in (no error)"), "SerialNumber"="37001612" ("HWSerialNum")) -> (reference out=w2283:refnum<k24>, error out=w2282:errorcluster)
      n1023 = property class="FilterFlipperControl"(reference="FilterFlipperControl", error in=errorcluster {"status"=FALSE, "code"=0, "source"=""} ("error in (no error)"), "SerialNumber"="37001046" ("HWSerialNum")) -> (reference out=w2278:refnum<k24>, error out=w2279:errorcluster)
      n1024 = invoke class="FilterFlipperControl" method="CreateDevice"(reference=w2283, error in=w2282) -> (reference out=w2280:refnum<k24>, error out=w2281:errorcluster)  [unwired: 1 in, 1 out]
      n1025 = invoke class="FilterFlipperControl" method="CreateDevice"(reference=w2278, error in=w2279) -> (reference out=w2277:refnum<k24>, error out=w2276:errorcluster)  [unwired: 1 in, 1 out]
      n1026 = property class="FilterFlipperControl"(reference=w2280, error in=w2281) -> (reference out=w2285:refnum<k24>, error out=→"Flip Motor (Spectrometer) Initialization Error":errorcluster, "Device"=w2271:refnum<k24>)
      n1027 = property class="FilterFlipperControl"(reference=w2277, error in=w2276) -> (reference out=w2275:refnum<k24>, error out=w2270:errorcluster, "Device"=w2272:refnum<k24>)
      "Flip Motor (Det) Initialization Error" <- w2270
    }
  }
  n1028 = flat-sequence {
    tunnel: [w2293] -> w31
    tunnel: [w2292] -> w8
    tunnel: [w2291] -> w6
    tunnel: [w2290] -> w7
    frame #0 {
      w2297 = u32 0 ("initial count")
      w2298 = 10128 items=["Count Up"=10128, "Count Down"=10124, "Externally Controlled"=10326] ("count direction")
      w2299 = 10280 items=["Rising"=10280, "Falling"=10171] ("edge")
      # "NI DAQ USB-6431 Initalization (Counters)"
      n1029 = call-poly <vilib>:"DAQmx Create Virtual Channel.vi"("initial count"=w2297, "count direction"=w2298, "edge"=w2299, "counter"="ctr0") -> ("task out"=w2307:refnum<k21>, "error out"=w2308:errorcluster)  [unwired: 10 in]
      n1030 = call-poly <vilib>:"DAQmx Create Virtual Channel.vi"("initial count"=w2297, "count direction"=w2298, "edge"=w2299, "counter"="ctr1") -> ("task out"=w2304:refnum<k21>, "error out"=w2305:errorcluster)  [unwired: 10 in]
      n1031 = call-poly <vilib>:"DAQmx Create Virtual Channel.vi"("initial count"=w2297, "count direction"=w2298, "edge"=w2299, "counter"="ctr2") -> ("task out"=w2301:refnum<k21>, "error out"=w2302:errorcluster)  [unwired: 10 in]
      n1032 = call <vilib>:"DAQmx Start Task.vi"("task/channels in"=w2307, "error in"=w2308) -> ("task out"=w2296:refnum<k21>, "error out"=w2292:errorcluster)  [unwired: 12 in]
      "NI USB-6341 ctr0 Initalization Error" <- w2292
      n1033 = call <vilib>:"DAQmx Start Task.vi"("task/channels in"=w2304, "error in"=w2305) -> ("task out"=w2295:refnum<k21>, "error out"=w2291:errorcluster)  [unwired: 12 in]
      "NI USB-6341 ctr1 Initalization Error" <- w2291
      n1034 = call <vilib>:"DAQmx Start Task.vi"("task/channels in"=w2301, "error in"=w2302) -> ("task out"=w2294:refnum<k21>, "error out"=w2290:errorcluster)  [unwired: 12 in]
      "NI USB-6341 ct2 Initalization Error" <- w2290
      n1035 = Bundle("task out"=w2296, "task out"=w2295, "task out"=w2294) -> (w2293:T20)  [unwired: 1 in]
    }
  }
  n1036 = flat-sequence {
    tunnel: [w2310] -> w3
    frame #0 {
      w2316 = u32 0 ("Index (0)")
      # "Thorlabs Power Meter Initalization"
      n1037 = call <instrlib>:"TLPMX Find Resources.vi"("instrument handle"=refnum<visa-resource-name> refnum) -> ("error out"=w2321:errorcluster)  [unwired: 8 in, 2 out]
      n1038 = call <instrlib>:"TLPMX Get Resource Name.vi"("error in (no error)"=w2321, "Index (0)"=w2316) -> ("error out"=w2318:errorcluster, "instrument handle out"=w2315:refnum<visa-resource-name>, "Resource Name"=w2319:string)  [unwired: 7 in]
      "Resource Name" <- w2319
      n1039 = call <instrlib>:"TLPMX Get Resource Information.vi"("error in (no error)"=w2318, "Index (0)"=w2316, "instrument handle"=w2315) -> ("error out"=w2317:errorcluster, "Serial Number"=→"Serial Number":string)  [unwired: 3 in, 4 out]
      n1040 = call <instrlib>:"TLPMX Initialize.vi"("error in (no error)"=w2317, "resource name"=w2319) -> ("error out"=w2312:errorcluster, "instrument handle out"=w2311:refnum<visa-resource-name>)  [unwired: 8 in]
      n1041 = call <instrlib>:"TLPMX Set Wavelength.vi"("error in (no error)"=w2312, "Wavelength (0.0)"="Wavelength", "instrument handle"=w2311) -> ("error out"=→"Power Meter Initalization Error":errorcluster, "instrument handle out"=w2310:refnum<visa-resource-name>)  [unwired: 7 in]
    }
  }
  n1042 = flat-sequence {
    tunnel: [w2333] -> w4
    tunnel: [w2322] -> w16
    frame #0 {
      # "Rotation Stage Initalization (attenuator)"
      n1043 = property class="KCubeDCServoControl"(reference="Rotating Laser Power Filter", "SerialNumber"="27006088") -> (reference out=w2324:refnum<k24>, error out=w2325:errorcluster)  [unwired: 1 in]
      n1044 = invoke class="KCubeDCServoControl" method="CreateDevice"(reference=w2324, error in=w2325) -> (reference out=w2327:refnum<k24>, error out=w2328:errorcluster)  [unwired: 1 in, 1 out]
      n1045 = property class="KCubeDCServoControl"(reference=w2327, error in=w2328) -> (reference out=w2322:refnum<k24>, error out=w2329:errorcluster, "Device"=w2331:refnum<k24>)
      n1046 = invoke class="KCubeDCServo" method="Home"(reference=w2331, error in=w2329, "waitTimeout"=30000) -> (reference out=w2337:refnum<k24>, error out=w2336:errorcluster)  [unwired: 1 in, 2 out]
      n1047 = invoke class="KCubeDCServo" method="SetVelocityParams"(reference=w2337, error in=w2336, "maxVelocity"=25.0, "acceleration"=25.0) -> (reference out=w2333:refnum<k24>, error out=→"Rotation attenuator Initialization Error":errorcluster)  [unwired: 1 in, 3 out]
    }
  }
  n1048 = Merge Errors(w8, w6, w7) -> (w5:errorcluster)
  n1049 = local read "TraceData"() -> (w57:dbl[][])
  n1050 = while {
    shift-right: [w2378] -> _
    shift-left: w57 -> [w2338]
    tunnel: [FALSE] -> w55
    shift-right: [w2363] -> _
    shift-left: _ -> [w2364]
    shift-right: [w2357] -> _
    shift-left: _ -> [w2362]
    shift-right: [w2356] -> _
    shift-left: _ -> [w2361]
    shift-right: [w2349] -> w26
    shift-left: w5 -> [w2348]
    tunnel: w31 -> [w2347]
    tunnel: [w2340] -> w30
    stop <- w2377 stop-if-true
    # "Fast Loop (Read counters)"
    n1051 = Unbundle(w2347) -> ("task out"=w2346:refnum<k21>, "task out"=w2345:refnum<k21>, "task out"=w2344:refnum<k21>)
    n1052 = call-poly <vilib>:"DAQmx Read.vi"("task/channels in"=w2346, "error in"=w2348) -> ("task out"=w2343:refnum<k21>, "data"=w2363:dbl, "error out"=w2352:errorcluster)  [unwired: 11 in]
    n1053 = call-poly <vilib>:"DAQmx Read.vi"("task/channels in"=w2345, "error in"=w2348) -> ("task out"=w2342:refnum<k21>, "data"=w2357:dbl, "error out"=w2351:errorcluster)  [unwired: 11 in]
    n1054 = call-poly <vilib>:"DAQmx Read.vi"("task/channels in"=w2344, "error in"=w2348) -> ("task out"=w2341:refnum<k21>, "data"=w2356:dbl, "error out"=w2350:errorcluster)  [unwired: 11 in]
    n1055 = Unbundle By Name(w2352) -> ("status"=w2354:bool)
    n1056 = Unbundle By Name(w2351) -> ("status"=w2355:bool)
    n1057 = Unbundle By Name(w2350) -> ("status"=w2353:bool)
    n1058 = Subtract(x=w2363, y=w2364) -> (x-y=w2360:dbl)
    n1059 = Subtract(x=w2357, y=w2362) -> (x-y=w2359:dbl)
    n1060 = Subtract(x=w2356, y=w2361) -> (x-y=w2358:dbl)
    n1061 = Bundle("task out"=w2343, "task out"=w2342, "task out"=w2341) -> (w2340:T20)  [unwired: 1 in]
    n1062 = Merge Errors(w2348, w2352, w2351, w2350) -> (w2349:errorcluster)
    n1063 = local read "stop"() -> (w2374:bool)
    n1064 = local read "Laser power (uW)"() -> (w2339:dbl)
    n1065 = Wait (ms)(milliseconds to wait="Counter Int time (ms)") -> ()  [unwired: 1 out]
    n1066 = Compound Arithmetic op=OR(w2354, w2355, w2353, w2374) -> (w2377:bool)
    n1067 = call "Display and Log Count Traces.vi"("Record stab"="Record counts", "Laser power in"=w2339, "TraceData in"=w2338, "Integration time (ms)"="Counter Int time (ms)", "PDM2 ctr in"=w2358, "PDM1 ctr in"=w2359, "SPCM ctr in"=w2360) -> ("PDM2 counts"=→"PDM2 counts":i32, "PDM1 trace"=→"PDM1 trace":dbl, "PDM2 trace"=→"PDM2 trace":dbl, "Trace Data out"=w2376:dbl[][], "All Detector Counts"=→"All Detector Counts":dbl[][], "SPCM trace"=→"SPCM trace":dbl, "SPCM counts"=→"SPCM counts":i32, "PDM1 counts"=→"PDM1 counts":i32)  [unwired: 5 in]
    n1068 = case shown="True" "Write stability to file" {
      tunnel: w2376 -> [w2391 w2399]
      tunnel: [w2391 w2399] -> w2380
      frame False {
      }
      frame True {
        n1069 = local read "Measurement Save Path"() -> (w2400:path)
        n1070 = control-ref of="Laser power (uW)"() -> (w2392:refnum<vi>)
        n1071 = property on="Filter Configuraton" class="Ring (strict)"() -> ("RingText.Text"=w2394:string)  [unwired: 2 in, 2 out]
        n1072 = local read "Filename Note"() -> (w2396:string)
        n1073 = local read "Current Angle"() -> (w2398:sgl)
        n1074 = local read "Position"() -> (w2397:dbl[])
        n1075 = call "Quick Laser Power Log.vi"("Digital in"=w2392) -> ("Numeric"=w2393:dbl)  [unwired: 9 in, 1 out]
        n1076 = call "Save Measurement File.vi"("Measurement Save Path"=w2400, "Measurement Type"=MeasurementType."Stability", "Data in (if 2D)"=w2399, "ND angle"=w2398, "Position"=w2397, "Filename Note"=w2396, "Filter"=w2394, "laser power"=w2393) -> ()  [unwired: 12 in]
      }
    }
    n1077 = case shown="True" "Empty memory" {
      tunnel: w2380 -> [w2382 w2384]
      tunnel: [w2382 w2383] -> w2378
      frame False {
      }
      frame True {
        # "delete all but first row"
        n1078 = Array Size(array=w2384) -> (size(s)=w2390:i32[])
        n1079 = Subtract(x=w2390, y=1) -> (x-y=w2388:i32[])
        n1080 = Index Array(array=w2388, index=0) -> (element=w2386:i32)
        n1081 = Delete From Array(array=w2384, length=w2386, index (row)=1) -> (array with subset deleted=w2383:dbl[][])  [unwired: 1 in, 1 out]
      }
    }
    n1082 = local write "TraceData"(w2378) -> ()
  }
  n1083 = while {
    shift-right: [w2407] -> w39
    shift-left: _ -> [w2406]
    tunnel: w4 -> [w2410]
    stop <- w2409 stop-if-true
    w2403 = 10.0 ("y")
    # "Slow Loop (Read attenuator)"
    n1084 = invoke class="KCubeDCServo" method="GetPositionCounter"(reference=w2410, error in=w2406) -> (error out=w2407:errorcluster, "GetPositionCounter"=w2412:i32)  [unwired: 1 in, 1 out]
    n1085 = Wait (ms)(milliseconds to wait=u32 250) -> ()  [unwired: 1 out]
    n1086 = Divide(x=w2412, y=1920) -> (x/y=w2402:dbl)
    n1087 = Multiply(x=w2402, y=w2403) -> (x*y=w2405:dbl)
    n1088 = Round To Nearest(number=w2405) -> (nearest integer value=w2404:dbl)
    n1089 = Divide(x=w2404, y=w2403) -> (x/y=→"Current Angle":dbl)
    n1090 = local read "stop"() -> (w2409:bool)
  }
  "Attenuator Error Out" <- w39
  n1091 = while {
    shift-right: [w2420] -> w2
    shift-left: _ -> [w2419]
    tunnel: w3 -> [w2418]
    tunnel: [w2417] -> w1
    stop <- w2416 stop-if-true
    n1092 = local read "Record counts"() -> (w2414:bool)
    n1093 = call <instrlib>:"TLPMX Measure Power.vi"("error in (no error)"=w2419, "instrument handle"=w2418) -> ("error out"=w2420:errorcluster, "Power"=w2415:dbl, "instrument handle out"=w2417:refnum<visa-resource-name>)  [unwired: 7 in]
    n1094 = Multiply(x="Multiplier", y=w2415) -> (x*y=w2423:dbl)
    n1095 = case shown="False" w2414 {
      frame False {
        n1096 = Wait (ms)(milliseconds to wait="Power Meter Int Time (ms)") -> ()  [unwired: 1 out]
      }
      frame True {
        n1097 = local read "Counter Int time (ms)"() -> (w2425:T2)
        n1098 = Wait (ms)(milliseconds to wait=w2425) -> ()  [unwired: 1 out]
      }
    }
    n1099 = Multiply(x=w2423, y=1000000) -> (x*y=w2413:dbl)
    n1100 = local write "Laser power (uW)"(w2413) -> ()
    n1101 = local read "stop"() -> (w2416:bool)
  }
  n1102 = case shown="Error .." w2 {
    tunnel: w1 -> [w2428 _]
    tunnel: w2 -> [w2427 w2429]
    tunnel: [w2426 w2429] -> _
    frame No Error {
      n1103 = call <instrlib>:"TLPMX Close.vi"("error in (no error)"=w2427, "instrument handle"=w2428) -> ("error out"=w2426:errorcluster)  [unwired: 9 in]
    }
    frame Error {
    }
  }
  n1104 = local write "SLOC Laser"(w55) -> ()
  n1105 = local write "Laser Shutter"(w55) -> ()
  n1106 = invoke class="KCubeDCServoControl" method="CloseDevice"(reference=w16, error in=w26) -> (error out=w25:errorcluster)  [unwired: 1 in, 2 out]
  n1107 = invoke class="FilterFlipperControl" method="CloseDevice"(reference=w23, error in=w25) -> (error out=w37:errorcluster)  [unwired: 1 in, 2 out]
  n1108 = Unbundle(w30) -> ("task out"=w29:refnum<k21>, "task out"=w28:refnum<k21>, "task out"=w27:refnum<k21>)
  n1109 = call <vilib>:"DAQmx Stop Task.vi"("task/channels in"=w29, "error in"=w37) -> ("task out"=w45:refnum<k21>, "error out"=w46:errorcluster)  [unwired: 12 out]
  n1110 = call <vilib>:"DAQmx Clear Task.vi"("task in"=w45, "error in"=w46) -> ("error out"=w36:errorcluster)  [unwired: 13 in]
  n1111 = call <vilib>:"DAQmx Stop Task.vi"("task/channels in"=w28, "error in"=w36) -> ("task out"=w43:refnum<k21>, "error out"=w44:errorcluster)  [unwired: 12 out]
  n1112 = call <vilib>:"DAQmx Clear Task.vi"("task in"=w43, "error in"=w44) -> ("error out"=w35:errorcluster)  [unwired: 13 in]
  n1113 = call <vilib>:"DAQmx Stop Task.vi"("task/channels in"=w27, "error in"=w35) -> ("task out"=w40:refnum<k21>, "error out"=w41:errorcluster)  [unwired: 12 out]
  n1114 = call <vilib>:"DAQmx Clear Task.vi"("task in"=w40, "error in"=w41) -> ("error out"=w33:errorcluster)  [unwired: 13 in]
  n1115 = invoke class="FilterFlipperControl" method="CloseDevice"(reference=w24, error in=w33) -> (error out=w34:errorcluster)  [unwired: 1 in, 2 out]
  n1116 = feedback-in #1(w34) -> ()
  n1117 = feedback #1() -> (w32:errorcluster)  [unwired: 1 in]
  n1118 = call <vilib>:"Simple Error Handler.vi"("type of dialog (OK msg:1)"=w42, "error in (no error)"=w32) -> ()  [unwired: 3 in, 5 out]
  n1119 = call "Set logging mode.vi"("Logging mode"=FALSE, "error in"=w22) -> ("error out"=w21:errorcluster)  [unwired: 17 in]
  n1120 = call "FRP.vi"("System no."=w56, "Routinename"=string[] ["1", "2", "3\n"], "Option"=i32[] [0, 0], "error in"=w21) -> ("error out"=w62:errorcluster)  [unwired: 15 in]
  n1121 = call "ERR?.vi"("System no."=w56, "error in"=w62) -> ("error out"=w61:errorcluster)  [unwired: 16 in, 1 out]
  n1122 = flat-sequence {
    tunnel: w61 -> [w2430]
    tunnel: [w2430] -> w20
    frame #0 {
    }
  }
  n1123 = Unbundle By Name(w20) -> ("status"=w66:bool)
  n1124 = case shown="False" w66 {
    tunnel: [w2431 w2434] -> w17
    tunnel: w20 -> [w2432 w2434]
    frame False {
      # "No error, write control values\nto disk for retrieval and re-use"
      n1125 = call "Generic LV App Config Save-Retrieve.vi"("error in"=w2432, "Save/Retrieve"="Save") -> ("error out"=w2431:errorcluster)  [unwired: 5 in, 4 out]
    }
    frame True {
      n1126 = local write "Controls"(enum32{"Operation", "Parameters", "Setup"}."Setup" ("Controls")) -> ()
    }
  }
  n1127 = case shown="False" w49 {
    tunnel: w50 -> [_ w2439]
    tunnel: w17 -> [w2436 w2438]
    tunnel: [w2436 w2437] -> w19
    frame False {
    }
    frame True {
      n1128 = call <instrlib>:"Close.vi"("error in (no error)"=w2438, "hdl in"=w2439) -> ("error out"=w2437:errorcluster)  [unwired: 9 in]
    }
  }
  n1129 = call <vilib>:"DAQmx Clear Task.vi"("task in"=w47, "error in"=w19) -> ("error out"=w48:errorcluster)  [unwired: 13 in]
  n1130 = call <vilib>:"Simple Error Handler.vi"("error code (no error:0)"=w60, "error in (no error)"=w48) -> ()  [unwired: 3 in, 5 out]
  "Filter Wheel Init Error" <- w38
